vi "CORE PROGRAMMING TLB FRAME V1.vi"() -> ()   [LabVIEW 2018]
uses:
  TLB Type Definitions/Intruction Type Definitions.ctl
  TLB Type Definitions/State Type Definitions, for 0.26g versions and later 3.ctl
  <vilib>/Studica/Studica Toolkit/NavX/TypeDefs/Flags/Z900_navX_Flags_OpStatusTypeDef.ctl
  <vilib>/Studica/Studica Toolkit/NavX/TypeDefs/Flags/Z900_navX_Flags_CalibrationStatusTypeDef.ctl
  TLB Type Definitions/Vision cluster.ctl
  TLB Type Definitions/PING CLUSTER.ctl
  TLB Type Definitions/Encoder cluster.ctl
  TLB Type Definitions/Stepper cluster.ctl
  TLB Type Definitions/Yaw Cluster.ctl
  TLB Type Definitions/IR Sensor Type Def.ctl
  TLB Type Definitions/Line Sensor Cluster.ctl
  TLB Type Definitions/Time cluster.ctl
  TLB Type Definitions/Box Colour Detection Cluster (0.26d and above).ctl
  Underlying VI's/FGV's/Box FGV/Box Colour FGV Colours.ctl
  <vilib>/Studica/Studica Toolkit/Background/DIO Channel.ctl
  TLB Type Definitions/Y Stepper cluster.ctl
  TLB Type Definitions/Motor Speed Cluster.ctl
  <vilib>/Studica/Studica Toolkit/Background/PWM Channel.ctl
  Underlying VI's/NavX VI/navX type def.ctl
  <vilib>/Studica/Studica Toolkit/Background/I2C Channel.ctl
  Underlying VI's/I2C Master VI/Arduino_Interfacing.ctl
  Labview Training Phase 2/Enum Controls/States for Action Engine.ctl
  Underlying VI's/Motor Control VI with PID/MOTOR CONTROL WITH PID AE DATA MODE TYPE DEF.ctl
  Underlying VI's/Motor Control VI with PID/MOTOR CONTROL WITH PID AE DIRECTION TYPE DEF.ctl
  Experimental VI's/Archived VI's/MOTOR CONTROL NO PID Type Def.ctl
  <vilib>/myRIO/Common/Instrument Driver Framework/myRIO v1.0/AI/typedefs/AI Channels List.ctl
  <vilib>/myRIO/Common/Instrument Driver Framework/myRIO v1.0/AI/typedefs/AI Channels Enum.ctl
  Underlying VI's/Line Sensor AE/Line Sensor AE Type Def.ctl
  Underlying VI's/I2C Master VI/I2C MASTER Type Def.ctl
  Underlying VI's/Elasped Timer/Elapsed timer control.ctl
  Underlying VI's/IMAQ Create Reference AE/IMAQ Reference AE.ctl
  Underlying VI's/FGV's/Box FGV/Box Colour FGV States.ctl
  Underlying VI's/I2C Master VI/I2C_MASTER_WRITE_NEW Type Def.ctl
  Underlying VI's/FGV's/Servo State FGV/Servo States FGV Enum.ctl
  Underlying VI's/Modified webcam FGV/Webcam AE.ctl
  <vilib>/userdefined/High Color/IMAQdx.ctl
  <vilib>/Studica/Studica Toolkit/NavX/NavX.lvlib
panel:
  out "Same colour?":bool
  out "Distance to move":dbl
  out "Box Colour Detection":T1
  out "Errors detected":bool
  out "Robot ready":bool
  out "Time cluster":T3
  out "Table IR obstruct":bool
  out "Front IR obstruct":bool
  out "Line sensors":T4
  out "IR Sensors":T5
  out "NAVX Values":T6
  out "Stepper position values":T7
  out "Encoder values":T8
  out "Ultrasonic sensors":T9
  out "Selected Task":T10=enum."Start Task 9"
  out "Object recognition mode":enum16{"Ball", "Soap", "Gel", "Pipe", "None"}(ring)
  out "Image Processing Error":errorcluster
  out "Object Detection":T11
  out "Status":T14 {"OP Status" items=["INITIALIZING", "SELFTEST_IN_PROGRESS", "ERROR", "IMU_AUTOCAL_IN_PROGRESS", "NORMAL"]; "Calibration Status" items=["IMU_CAL_STATE_MASK"=3, "IMU_CAL_STATE_INPROGRESS"=0, "IMU_CAL_STATE_ACCUMULATE"=1, "IMU_CAL_STATE_COMPLETE"=2]}
  out "General Errors":errorcluster
  in  "Red LED":bool
  out "Front Ultrasonic obstruct":bool
  out "Speed & distance":T15
  out "Task selection":u8
  out "NavX Readings":T16
  out "Arduino Data":T17
  out "TASK ENABLE":bool
  out "Rising Edge":bool
  in  "Green LED":bool
  out "State Logic":T18=enum."Startup"
  out "elements":T10[](array[typedef])
  in  "STOP TASK":bool
  in  "OK Button":bool
  in  "STOP":bool
  out "Queue Errors":errorcluster
  out "Action Queue Items":i32
  out "State Logic Queue Items":i32
  out "Action Queues items":string[](array[string])=["Hardware reset", "Software reset", ""]
  out "Action State":string
  # "TLB FRAMEWORK STATUS"
  # "System Health Status Update"
  # "Test Programme written by Calvin Loke    Dated: 28 Aug 2019\nTest Programme revised by Dr Alex See   Dated 30 Aug 2019\n\nRevision date: 20/03/2020\nProgramme version:   TLB Native Dynamic Events ver 0.19a"
  # "0: Task 1\n1: Task 2\n2: Task 3\n3: Task 4\n4: Task 5\n5: Task 6\n6: Task 7\n7: Task 8 Ball\n8: Task 8 Soap\n9: Task 8 Gel\n10: Task 8 Pipe\n11: Task 9 Blue\n12: Task 9 Black\n13: Task 9 Green\n14: Task 9 Red\n15: Task 9 Yellow"
  # "Ball: Right\nSoap: Left\nGel: Reverse\nPipe: Forward"
  # "VISION"
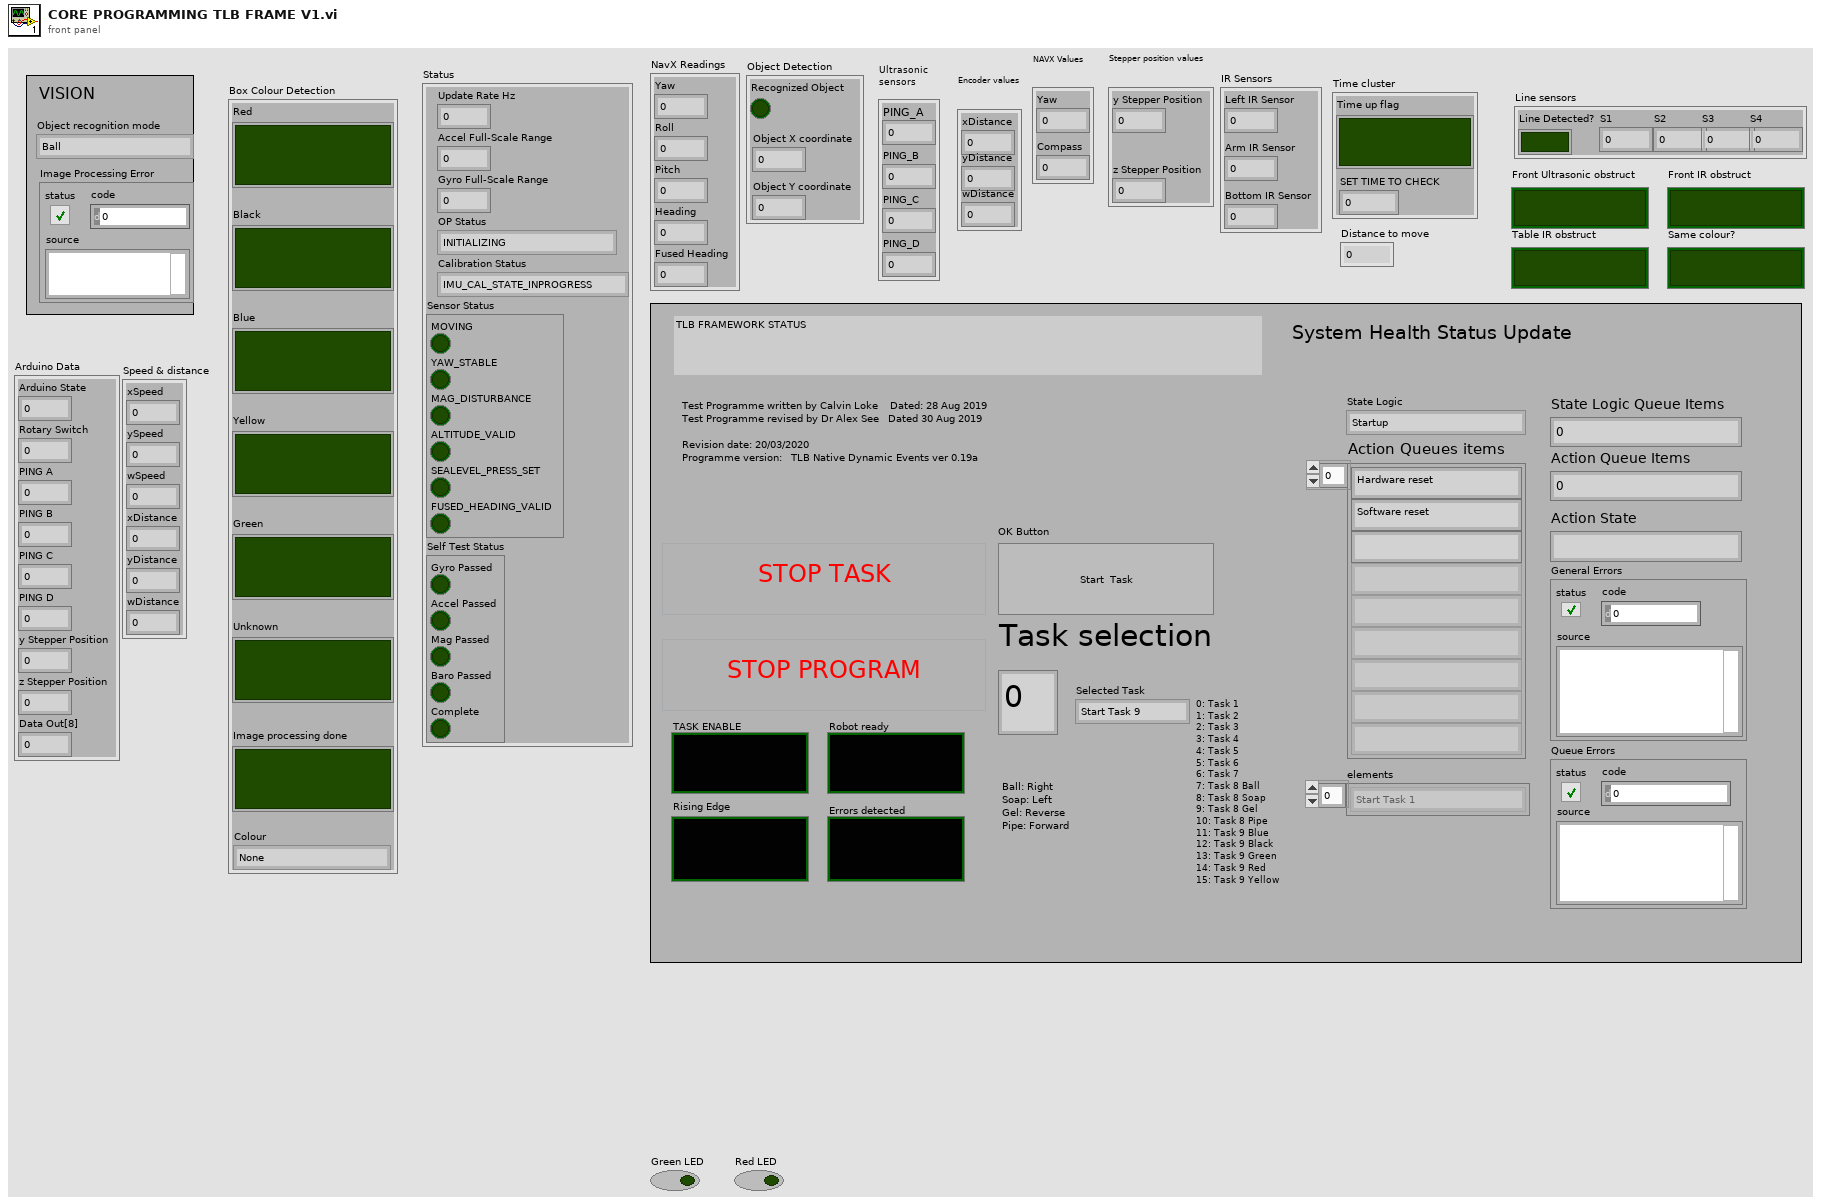
[diagram p1: front panel]
types:
  T1 = typedef "Box Colour Detection Cluster (0.26d and above).ctl" = cluster{"Red":bool, "Black":bool, "Blue":bool, "Yellow":bool, "Green":bool, "Unknown":bool, "Image processing done":bool, "Colour":T2}
  T2 = typedef "Box Colour FGV Colours.ctl" = enum16{"None", "Black", "Blue", "Green", "Red", "Yellow"}
  T3 = typedef "Time cluster.ctl" = cluster{"Time up flag":bool, "SET TIME TO CHECK":dbl}
  T4 = typedef "Line Sensor Cluster.ctl" = cluster{"Line Detected?":bool, "S1":dbl, "S2":dbl, "S3":dbl, "S4":dbl}
  T5 = typedef "IR Sensor Type Def.ctl" = cluster{"Left IR Sensor":dbl, "Arm IR Sensor":dbl, "Bottom IR Sensor":dbl}
  T6 = typedef "Yaw Cluster.ctl" = cluster{"Yaw":dbl, "Compass":dbl}
  T7 = typedef "Stepper cluster.ctl" = cluster{"y Stepper Position":u8, "z Stepper Position":u8}
  T8 = typedef "Encoder cluster.ctl" = cluster{"xDistance":dbl, "yDistance":dbl, "wDistance":dbl}
  T9 = typedef "PING CLUSTER.ctl" = cluster{"PING_A":u8, "PING_B":u8, "PING_C":u8, "PING_D":u8}
  T10 = typedef "Intruction Type Definitions.ctl" = enum16{"None", "Start Task 1", "Start Task 2", "Start Task 3", "Start Task 4", "Start Task 5", "Start Task 6", "Start Task 7", "Start Task 8 - BALL", "Start Task 8 - Gel", "Start Task 8 - Pipe", "Start Task 8 - Soap", "Start Task 9", "Start Task A", "Start Task B", "Exit"}
  T11 = typedef "Vision cluster.ctl" = cluster{"Recognized Object":bool, "Object X coordinate":dbl, "Object Y coordinate":dbl}
  T12 = typedef "NavX.lvlib/Z900_navX_Flags_OpStatusTypeDef.ctl" = u8
  T13 = typedef "NavX.lvlib/Z900_navX_Flags_CalibrationStatusTypeDef.ctl" = u8
  T14 = cluster{"Update Rate Hz":u8, "Accel Full-Scale Range":u8, "Gyro Full-Scale Range":u16, "OP Status":T12, "Calibration Status":T13, "Sensor Status":cluster{"MOVING":bool, "YAW_STABLE":bool, "MAG_DISTURBANCE":bool, "ALTITUDE_VALID":bool, "SEALEVEL_PRESS_SET":bool, "FUSED_HEADING_VALID":bool}, "Self Test Status":cluster{"Gyro Passed":bool, "Accel Passed":bool, "Mag Passed":bool, "Baro Passed":bool, "Complete":bool}}
  T15 = cluster{"xSpeed":dbl, "ySpeed":dbl, "wSpeed":dbl, "xDistance":dbl, "yDistance":dbl, "wDistance":dbl}
  T16 = cluster{"Yaw":dbl, "Roll":dbl, "Pitch":dbl, "Heading":dbl, "Fused Heading":dbl}
  T17 = cluster{"Arduino State":u8, "Rotary Switch":u8, "PING A":u8, "PING B":u8, "PING C":u8, "PING D":u8, "y Stepper Position":u8, "z Stepper Position":u8, "Data Out[8]":u8}
  T18 = typedef "State Type Definitions, for 0.26g versions and later 3.ctl" = enum16{"None", "Startup", "Move to Angle", "True Stop", "Idle", "Shutdown", "Task 1A", "Task 1B", "Task 2:Raise Arm", "Task 2:Sensor Mode", "Task 2:Reverse Mode", "Task 3: Rotate 360", "Task 4_A", "Task 4_B", "Task 4_C", "Task 4_D", "Task 5A: RAISING ARM", "Task 5B: STILL WAITING", "Task 5C: GOING DOWN", "Task 5D: GRAB", "Task 5E: GOING UP", "Task 5F: ARM GRAB HEIGHT", "Task 5G: CLOSE CLAW", "Task 5H: RAISE ARM", "Task 6A: RAISE ARM", "Task 6B: CAM BURST", "Task 6C: PROCESS IMAGE", "Task 6D: BALL BUSTER", "Task 6E: STILL WAITING", "Task 6F: CAM BURST 2", "Task 6G: PROCESS IMAGE 2", "Task 6H: SKADI SOAPS", "Task 6I: STILL WAITING 2", "Task 6J: CAM BURST 3", "Task 6K: PROCESS IMAGE 3", "Task 6L: JAM IT IN", "Task 6M: STILL WAITING 3", "Task 6N: CAM BURST 4", "Task 6O: PROCESS IMAGE 4", "Task 6P: PIPE BOMB", "Task 7", "Task 8A: RAISE ARM", "Task 8B: MOVE TO BOX", "Task 8C: CAM BURST", "Task 8D: PROCESS IMAGE", "Task 8E: ROBOT ADJUST", "Task 8F: CAM BURST 2", "Task 8G: PROCESS IMAGE 2", "Task 8H: ARM ADJUST", "Task 8I: ARM GRAB HEIGHT", "Task 8J: CLOSE CLAW", "Task 8K: RAISE MY SWORD", "Task 8I: STILL WAITING", "Task 8L: Return to position", "Task 9A: Raise Arm", "Task 9B: Rotate to Angle", "Task 9C: Detect Box", "Task 9D: MOVE FORWARD", "Task 9D2: ANGLE CORRECTION", "Task 9E: MOVE LEFT", "Task 9E2: MOVE RIGHT", "Task 9F: SCAN BOX", "Task 9G: MOVE RIGHT", "Task 9H: SCAN BOX 2", "Task 9I: ROTATE 90 CW", "Task 9J: FORWARD", "Task 9J2: ANGLE CORRECTION", "Task 9K: RAM WALL", "Task 9L: MOVE RIGHT", "Task 9M: SCAN BOX 3", "Task 9N: MOVE RIGHT", "Task 9O: SCAN BOX 4", "Task A1: RAISE ARM", "Task A2: ROTATE TO ANGLE", "Task A3: MOVE TO BL BOX", "Task A4: MOVE FORWARD", "Task A5: Stop", "Task A6: ROTATE CW 90", "Task A7: FORWARD", "Task A8: LEFT UNTIL LINE", "Task A9: REVERSE", "Task A10: ROTATE TO ANGLE"}
  T19 = typedef "PWM Channel.ctl" = enum16{"Not Connected", "A/PWM0", "A/PWM1", "A/PWM2", "A/PWM3", "A/PWM4", "B/PWM0", "B/PWM1", "B/PWM2", "B/PWM3", "B/PWM4", "C/PWM0", "C/PWM1"}
  T20 = typedef "Motor Speed Cluster.ctl" = cluster{"ySpeed":dbl, "xSpeed":dbl, "wSpeed":dbl}
  T21 = typedef "Y Stepper cluster.ctl" = cluster{"yStepper desired":u8}
  T22 = typedef "DIO Channel.ctl" = enum16{"Not Connected", "A/DIO1", "A/DIO2", "A/DIO3", "A/DIO4", "A/DIO5", "A/DIO6", "A/DIO7", "A/DIO13", "B/DIO1", "B/DIO2", "B/DIO3", "B/DIO4", "B/DIO5", "B/DIO6", "B/DIO7", "B/DIO13", "C/DIO0", "C/DIO1", "C/DIO2", "C/DIO3", "C/DIO4", "C/DIO5", "C/DIO6", "C/DIO7"}
  T23 = cluster{"PWM Channel":T19, "FPGA VI Reference Out":refnum<k20>}
  T24 = cluster{"DIO Channel":T22, "FPGA VI Reference Out":refnum<k20>}
  T25 = typedef "States for Action Engine.ctl" = enum16{"Initialize", "Write", "Read"}
  T26 = typedef "MOTOR CONTROL WITH PID AE DATA MODE TYPE DEF.ctl" = enum16{"Init AE", "Write to AE", "Read from AE"}
  T27 = typedef "navX type def.ctl" = enum16{"Get i2C reference", "Read Values", "Zero Yaw"}
  T28 = typedef "Arduino_Interfacing.ctl" = enum16{"Initialize", "Write to Arduino", "Read From Arduino"}
  T29 = typedef "I2C Channel.ctl" = enum16{"Not Connected", "A", "B"}
  T30 = cluster{"I2C Ref Out":cluster{"I2C Channel":T29, "FPGA VI Reference Out":refnum<k20>}, "Connected":bool, "Slave Address (7-bit)":u8, "Registry":u8[]}
  T31 = typedef "Box Colour FGV States.ctl" = enum16{"Initialize", "Read", "Write"}
  T32 = typedef "MOTOR CONTROL WITH PID AE DIRECTION TYPE DEF.ctl" = enum16{"y-axis movement", "x-axis movement", "rotation", "stop", "reset encoders"}
  T33 = typedef "Line Sensor AE Type Def.ctl" = enum16{"INIT AE", "READ FROM LINE SENSORS"}
  T34 = typedef "IMAQ Reference AE.ctl" = enum16{"Initialize AE", "Get IMAQ Reference", "Dispose Processing Buffer"}
  T35 = typedef "Elapsed timer control.ctl" = enum16{"Start", "Pause", "Initialize"}
  T36 = typedef "I2C_MASTER_WRITE_NEW Type Def.ctl" = enum16{"Ultrasonic sensors", "Stepper origin", "zStepper 13.3k", "zStepper 13k", "zStepper 12k", "zStepper 11k", "zStepper 10k", "zStepper 9k", "zStepper 8k", "zStepper 7k", "zStepper 6k", "zStepper 5k", "zStepper 4k", "zStepper 3k", "zStepper 2k", "zStepper 1k", "zStepper 900", "zStepper 800", "zStepper 700", "zStepper 600", "zStepper 500", "zStepper 400", "zStepper 300", "zStepper 200", "zStepper 100", "zStepper 0", "yStepper control", "Open Claw", "Close Claw", "Soft Reset"}
  T37 = typedef "Servo States FGV Enum.ctl" = enum16{"Open Claw", "Close claw"}
  T38 = typedef "Webcam AE.ctl" = enum16{"Initialize Camera", "Open Camera", "Continuous Acquisition", "Close Camera", "Retrieve Image", "Dispose Camera Image Buffer"}
  T39 = typedef "IMAQdx.ctl" = refnum<k21>
  T40 = typedef "MOTOR CONTROL NO PID Type Def.ctl" = enum16{"Init", "Front Back", "Left Right", "Rotate", "Stop", "Latch"}
  T41 = typedef "AI Channels List.ctl" = T42[]
  T42 = typedef "AI Channels Enum.ctl" = enum16{"Not Connected", "AudioIn/Left", "AudioIn/Right", "C/AI0", "C/AI1", "A/AI0", "A/AI1", "A/AI2", "A/AI3", "A/AI4", "A/AI5", "A/AI6", "A/AI7", "B/AI0", "B/AI1", "B/AI2", "B/AI3", "B/AI4", "B/AI5", "B/AI6", "B/AI7", "AI/AI0", "AI/AI1", "AI/AI2", "AI/AI3", "A/AI0 (DIFF)", "A/AI1 (DIFF)", "A/AI2 (DIFF)", "A/AI3 (DIFF)", "B/AI0 (DIFF)", "B/AI1 (DIFF)", "B/AI2 (DIFF)", "B/AI3 (DIFF)"}
  T43 = cluster{"S1":dbl, "S2":dbl, "S3":dbl, "S4":dbl, "Array[4]":dbl, "Array[5]":dbl, "Array[6]":dbl, "Array[7]":dbl, "Array[8]":dbl}
  T44 = typedef "I2C MASTER Type Def.ctl" = enum16{"Last State", "Mode 0", "Mode 1", "Mode 2", "Mode 3", "Mode 4", "Mode 5", "Mode 6", "Mode 7", "Mode 8", "Mode 9", "Mode 10"}
  T45 = typedef "IMAQ Image.ctl" = refnum<image>
  T46 = cluster{"Number of Matches":i32, "Object detected?":bool}
  T47 = cluster{"Red":bool, "Black":bool, "Blue":bool, "Yellow":bool, "Green":bool, "No recognizable coolour":bool}
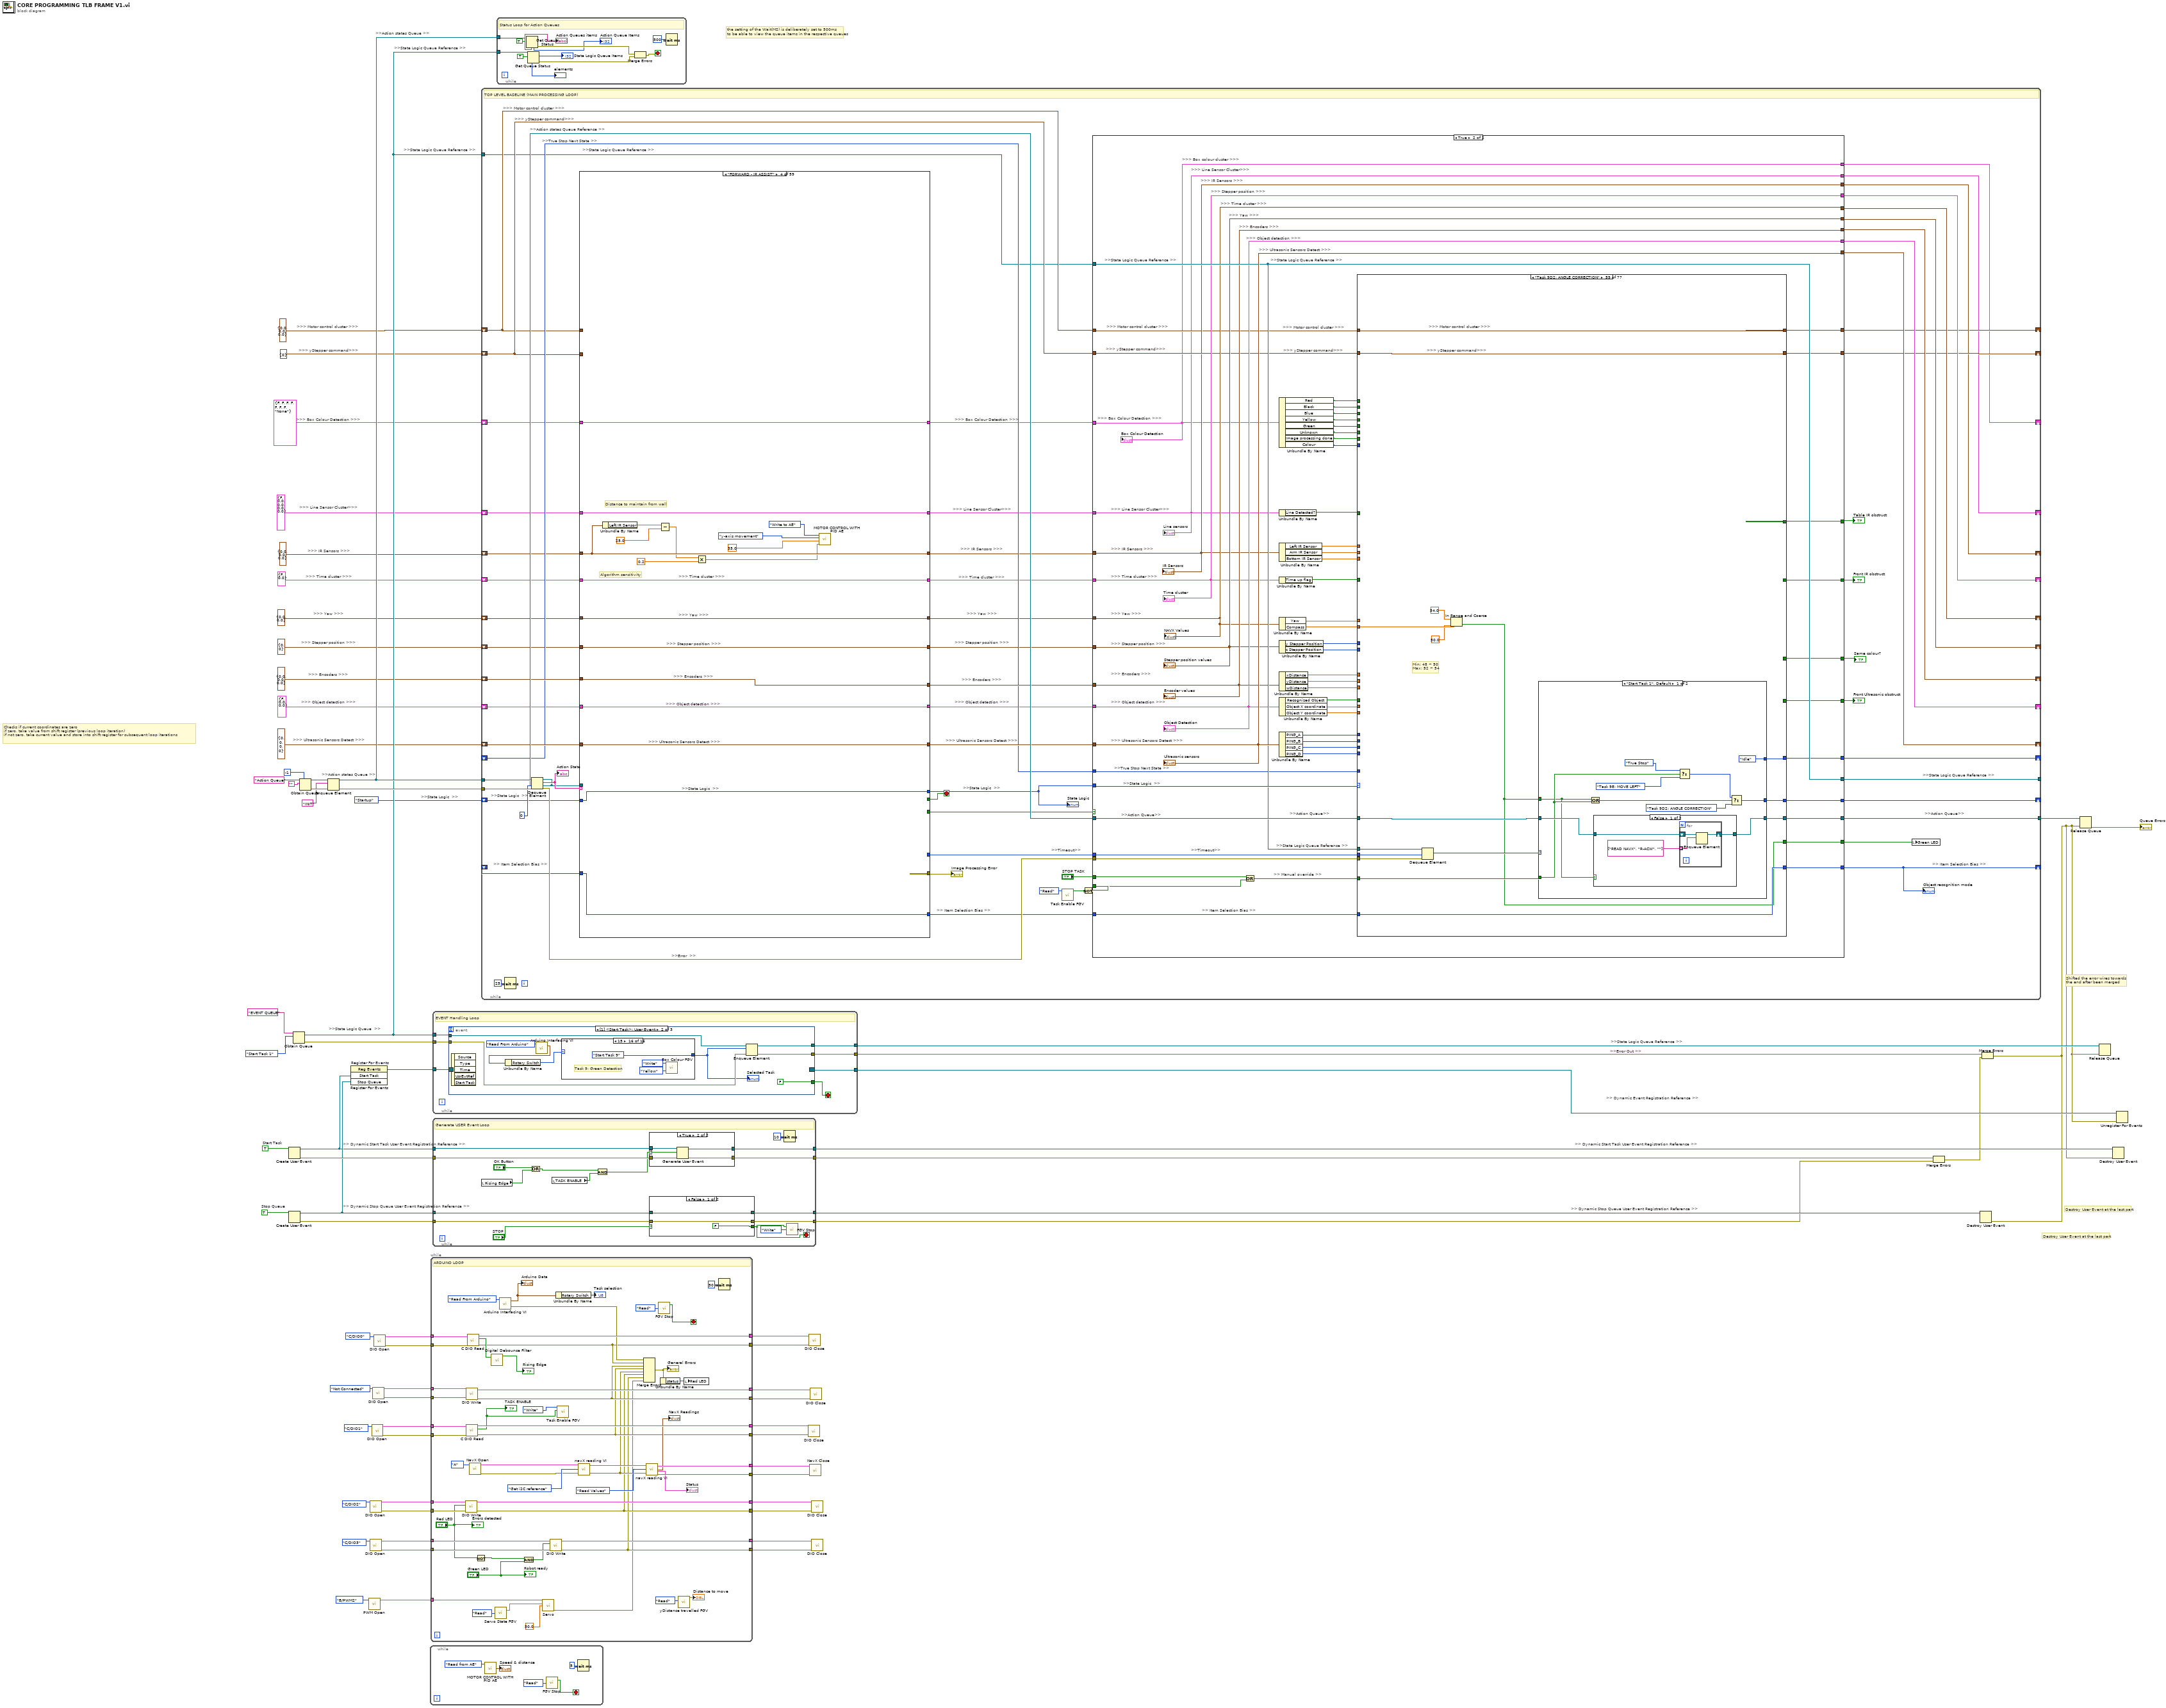
[diagram p0: block diagram]
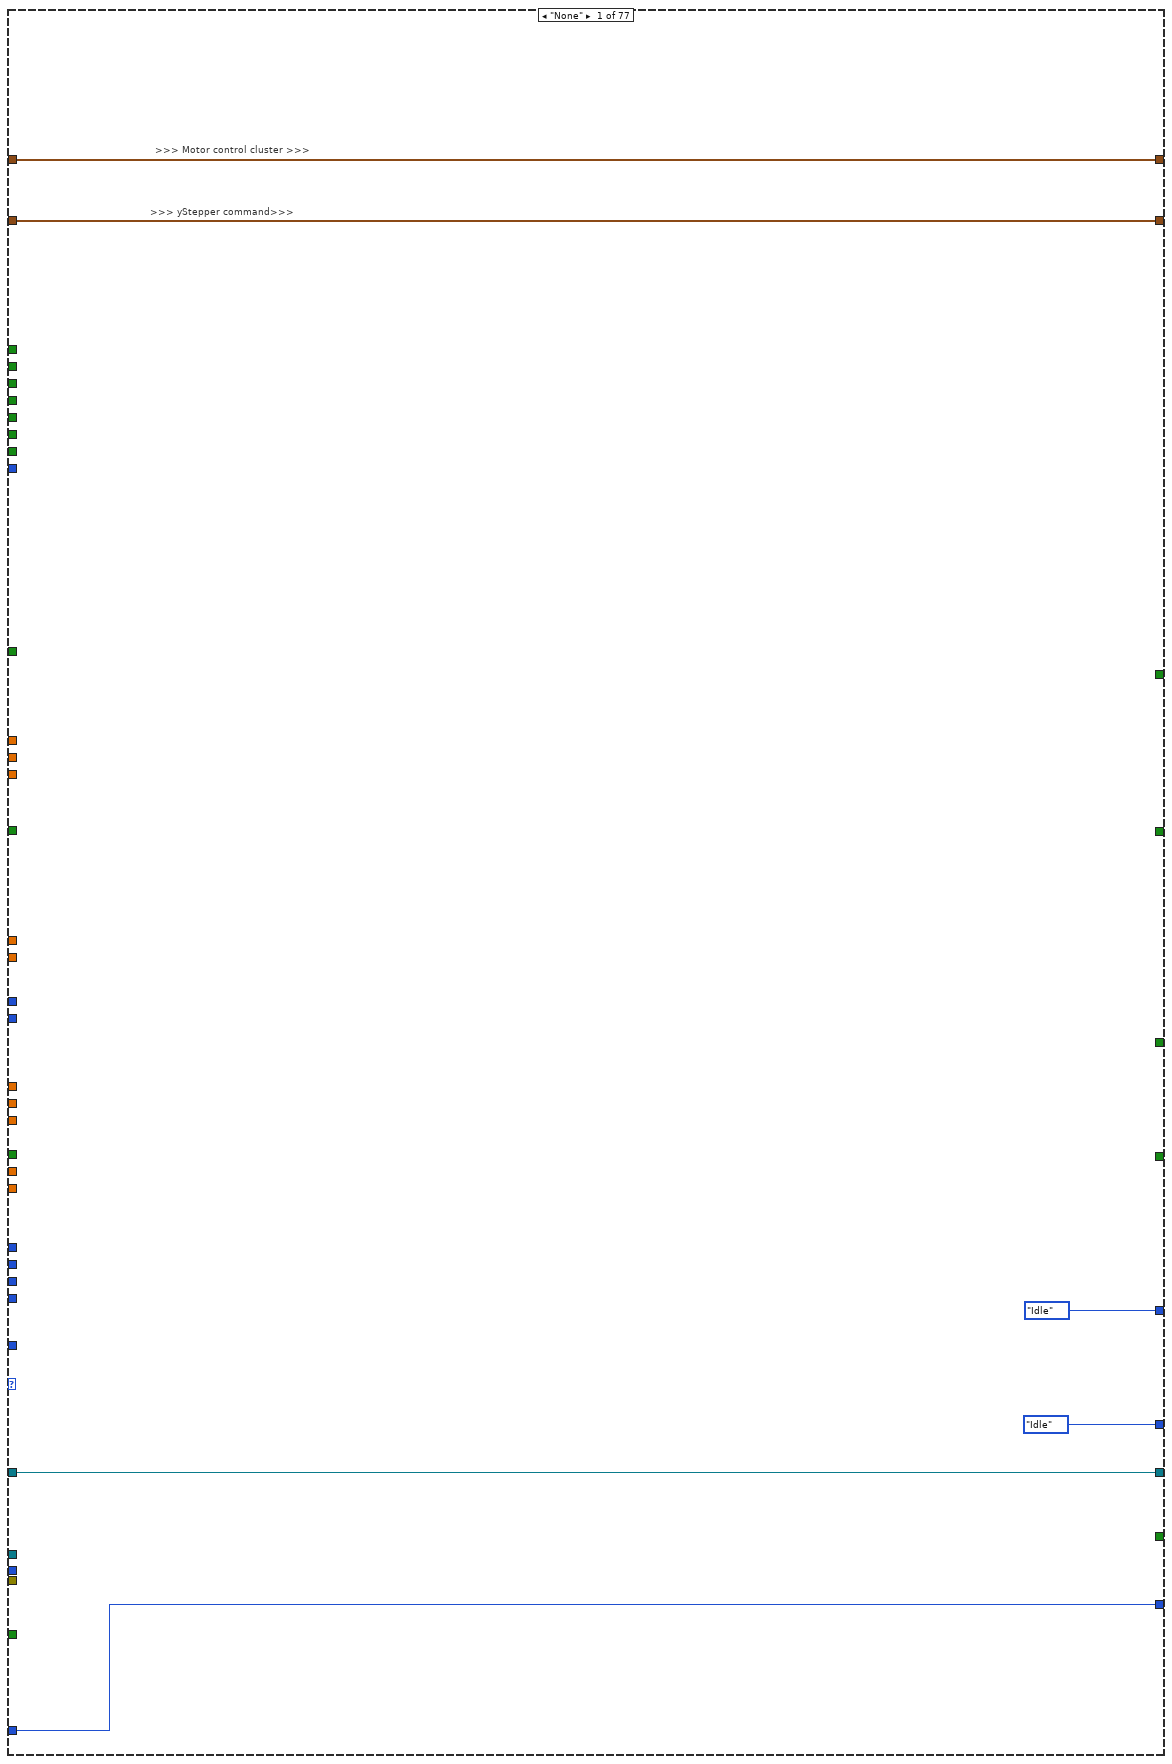
[diagram p3: hidden frame]
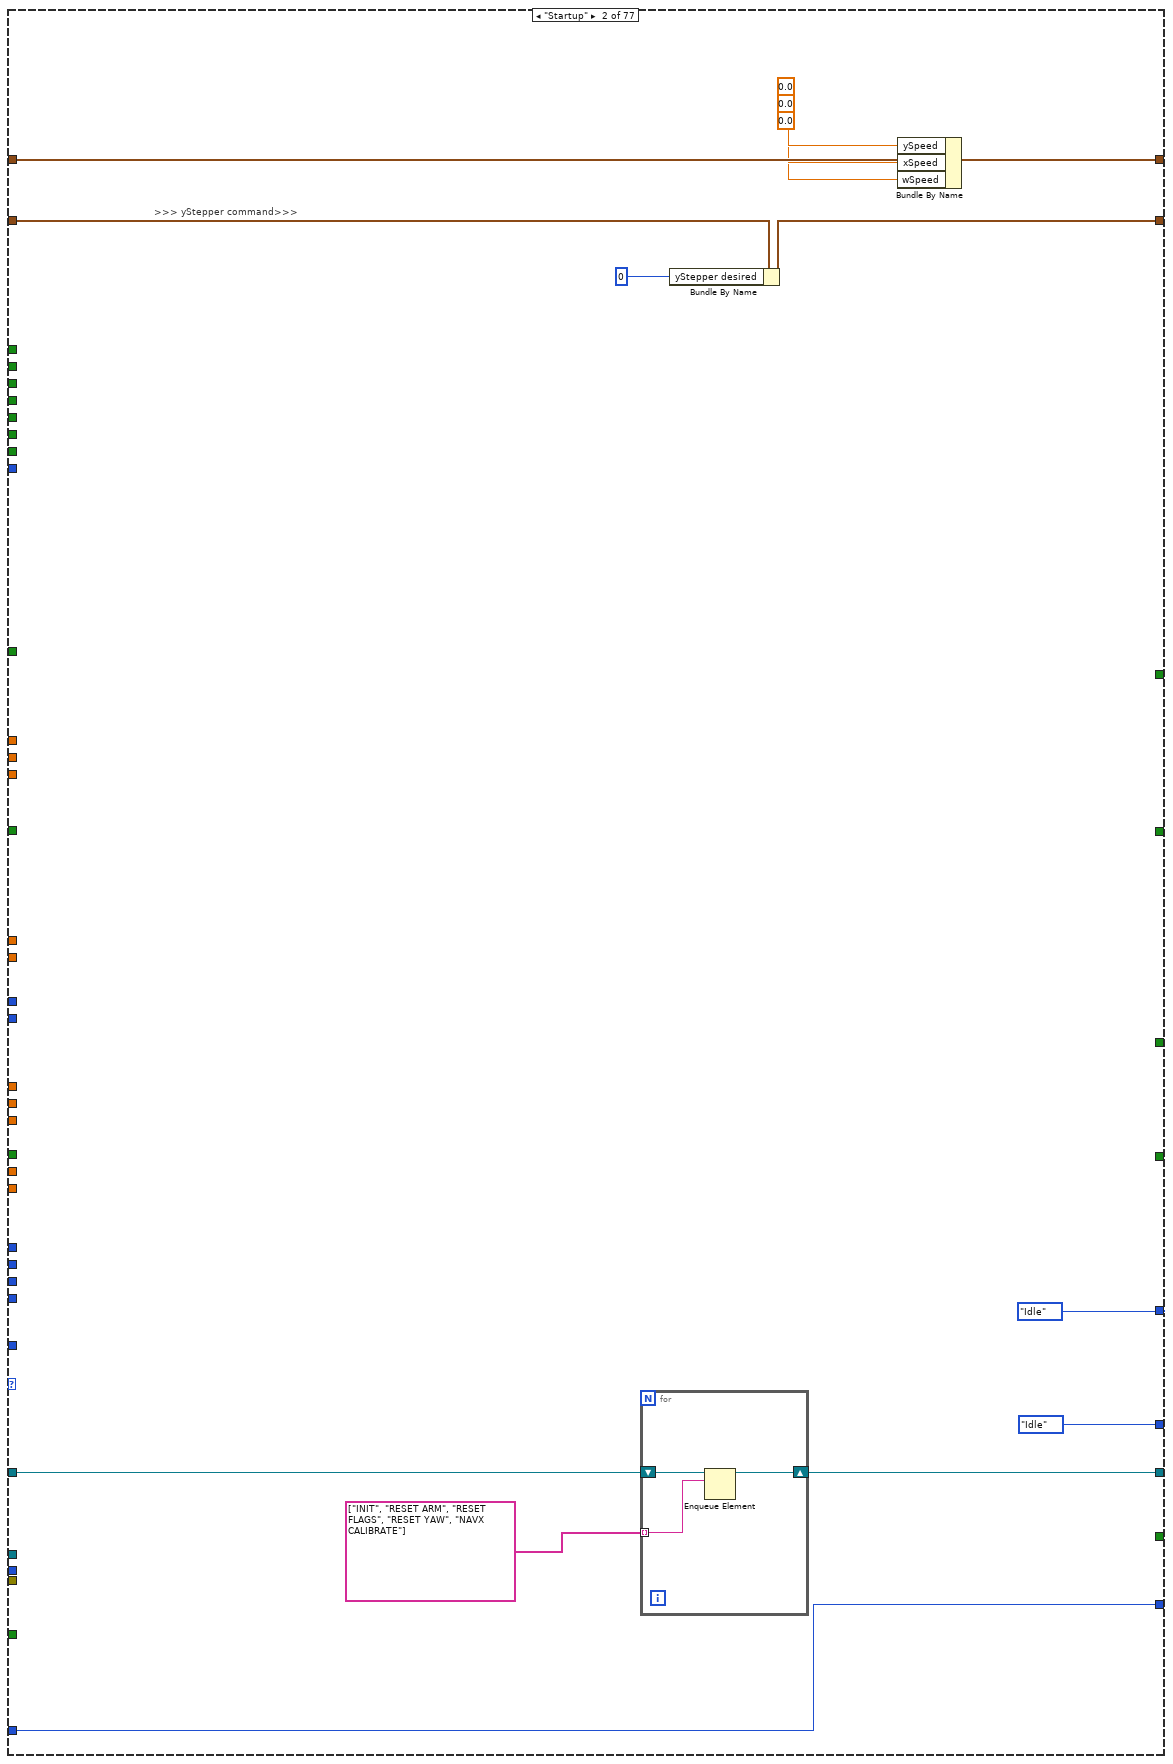
[diagram p4: hidden frame]
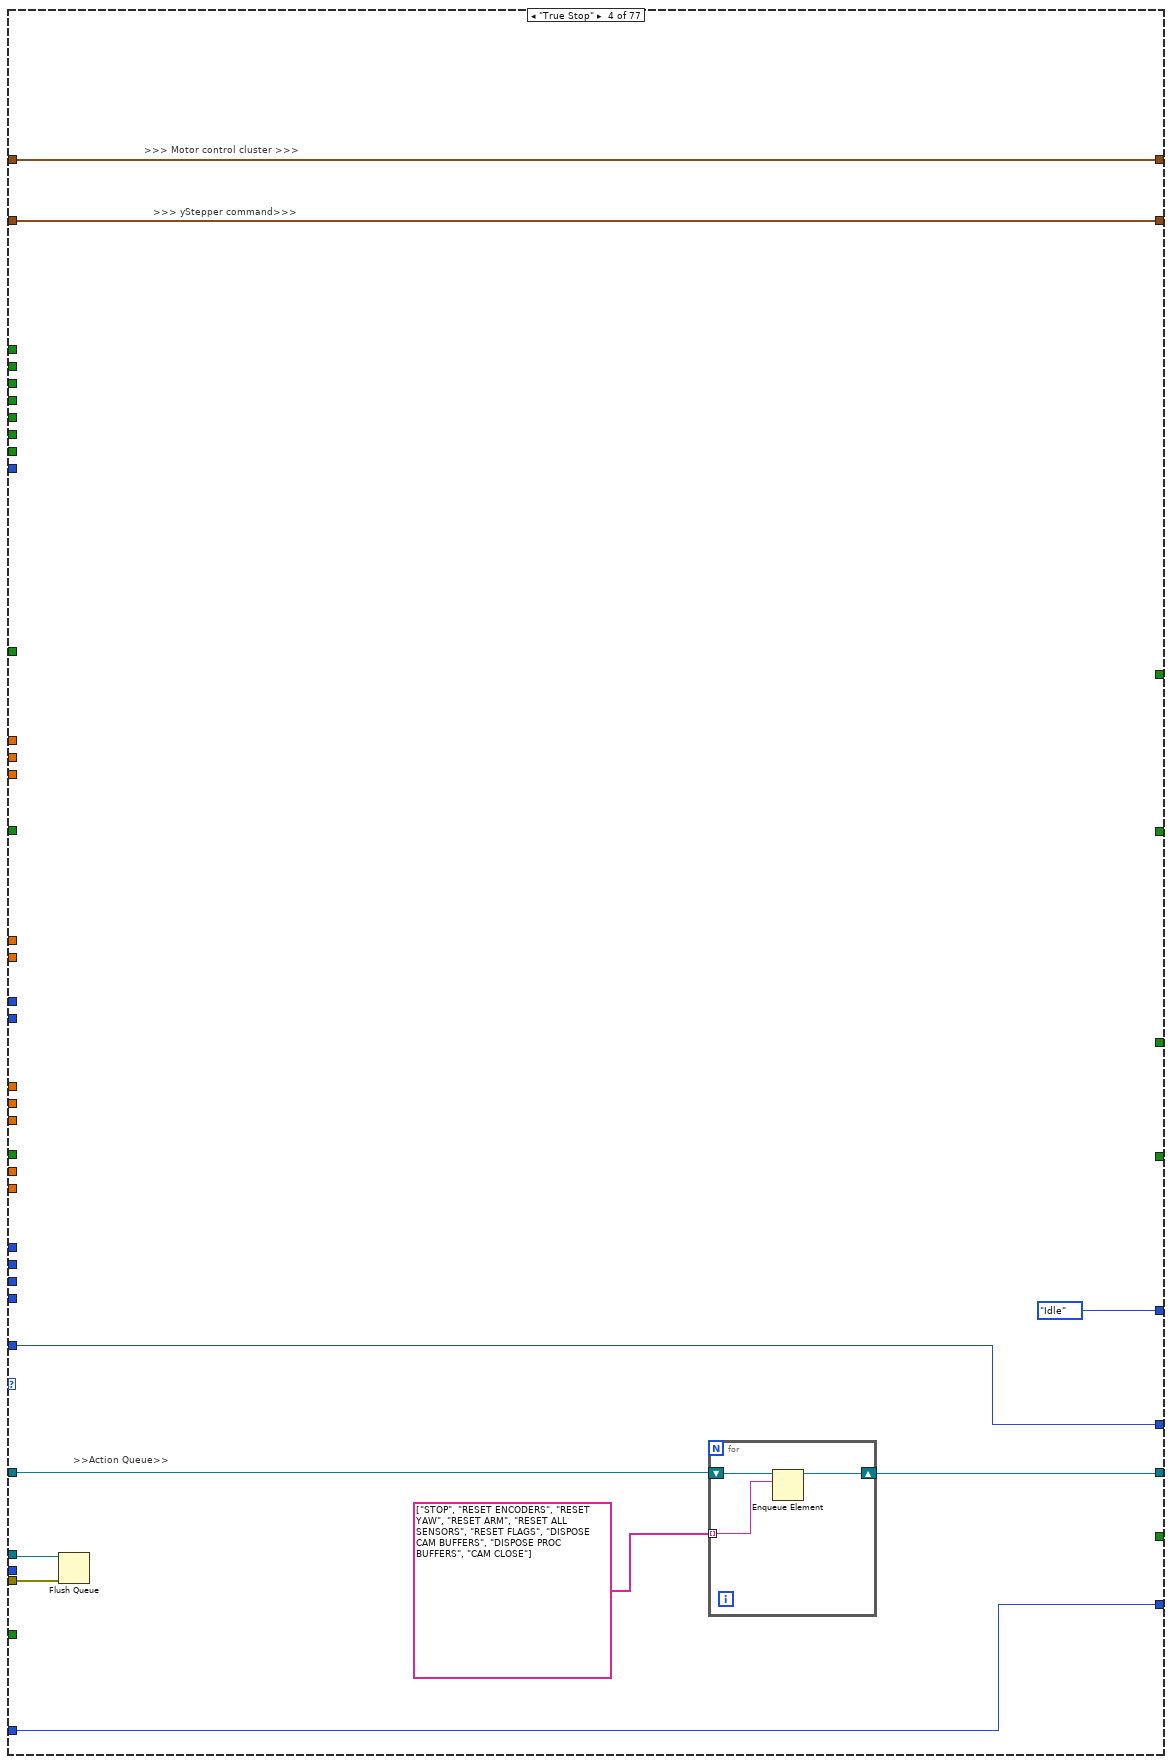
[diagram p6: hidden frame]
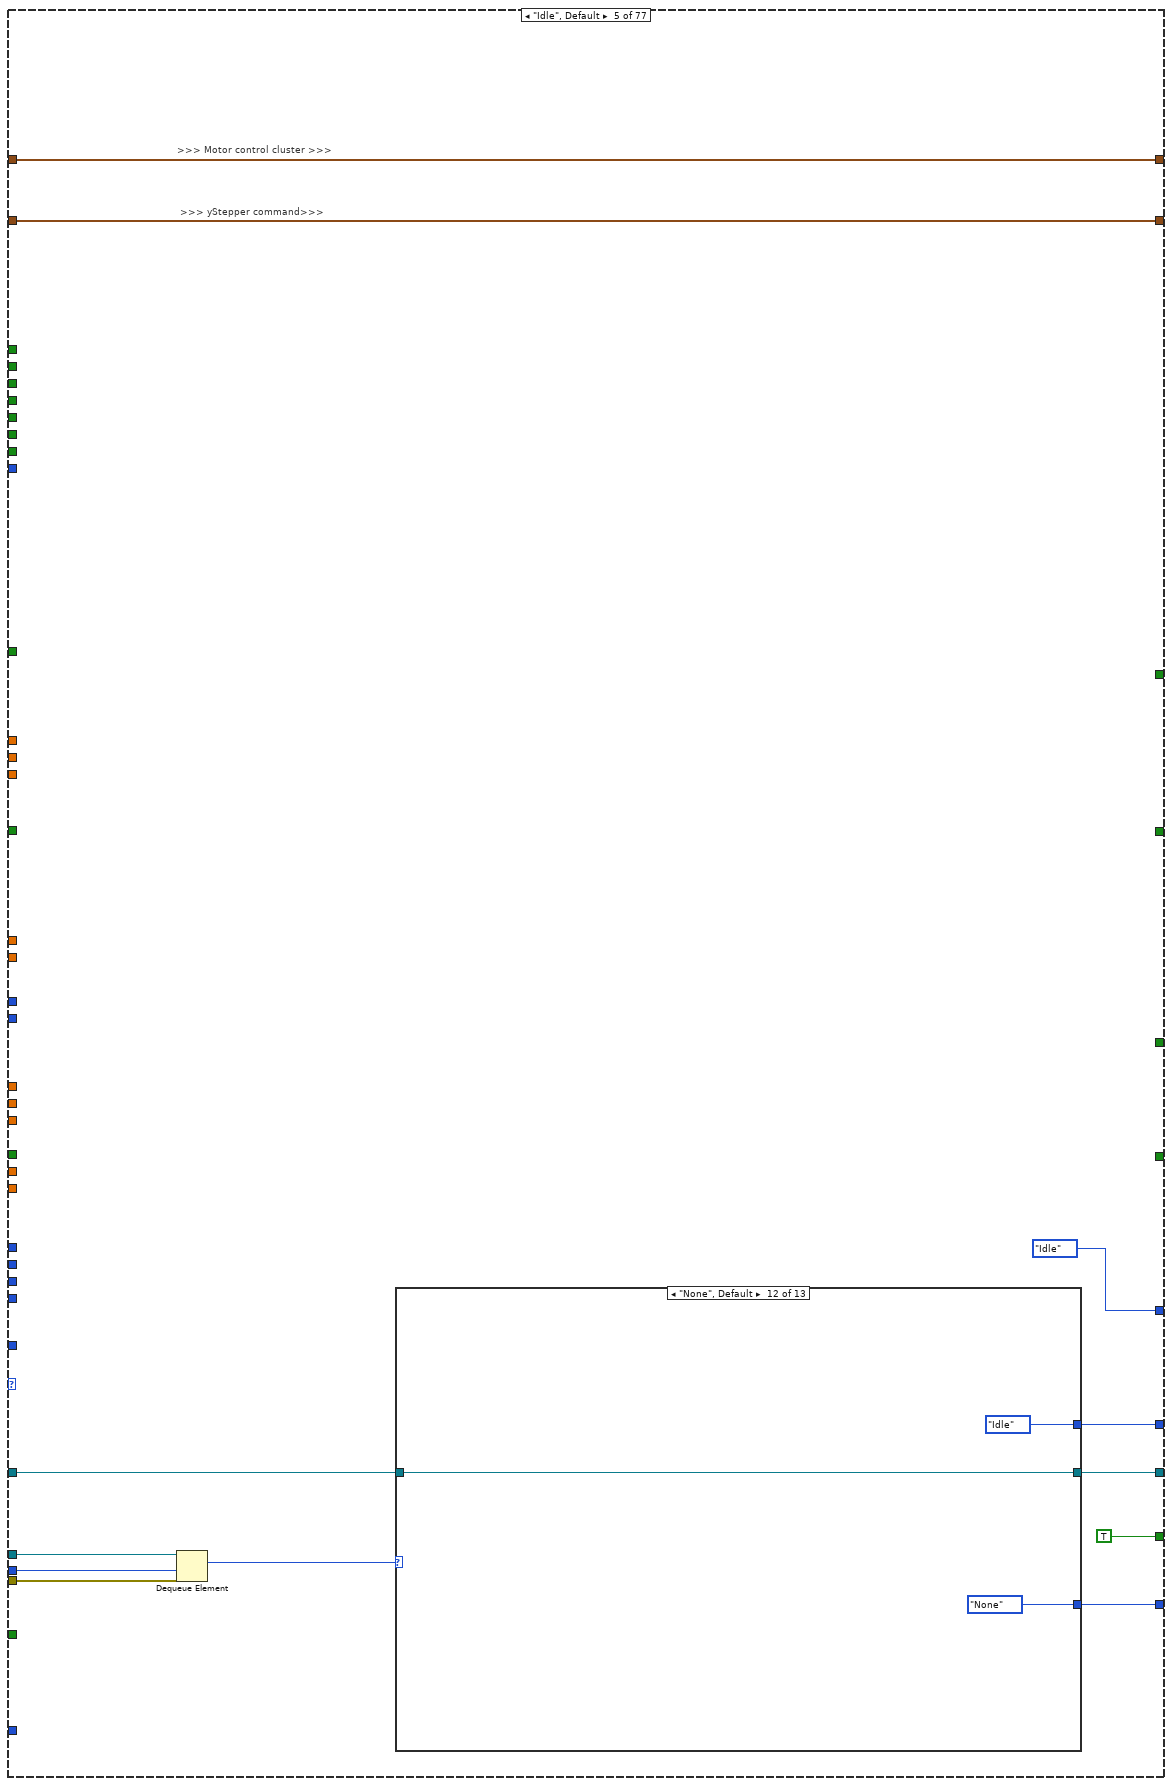
[diagram p7: hidden frame]
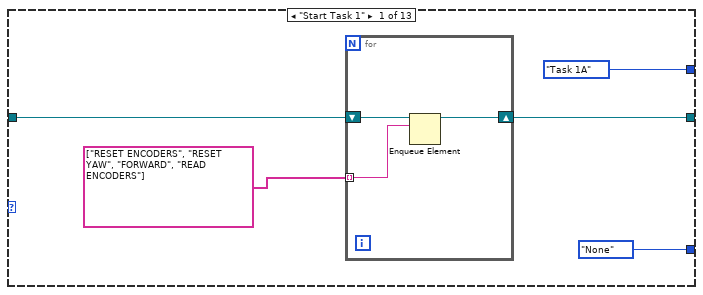
[diagram p8: hidden frame]
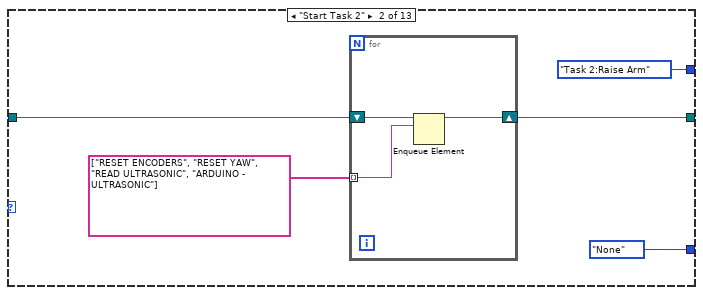
[diagram p9: hidden frame]
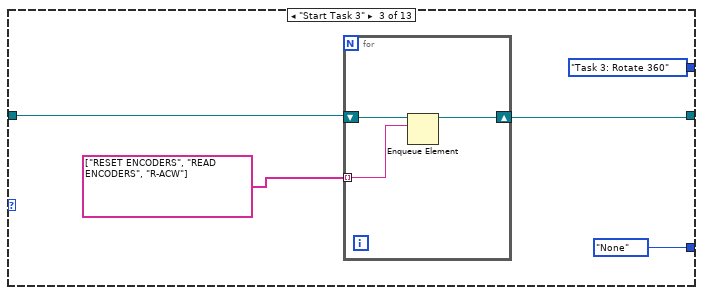
[diagram p10: hidden frame]
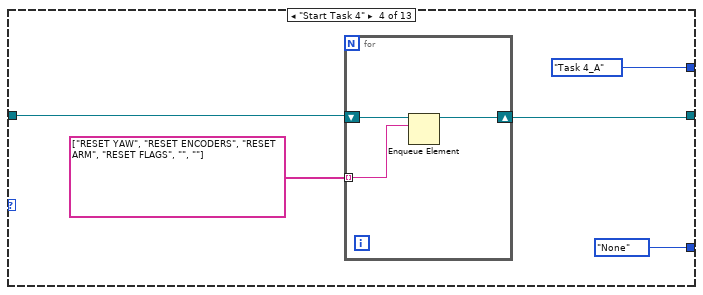
[diagram p11: hidden frame]
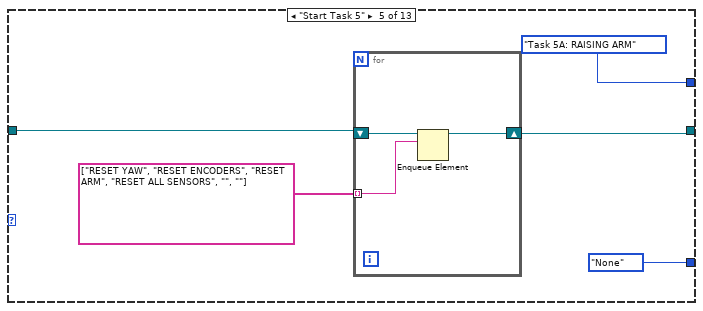
[diagram p12: hidden frame]
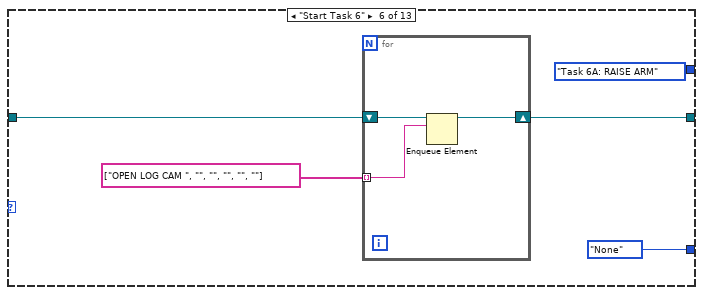
[diagram p13: hidden frame]
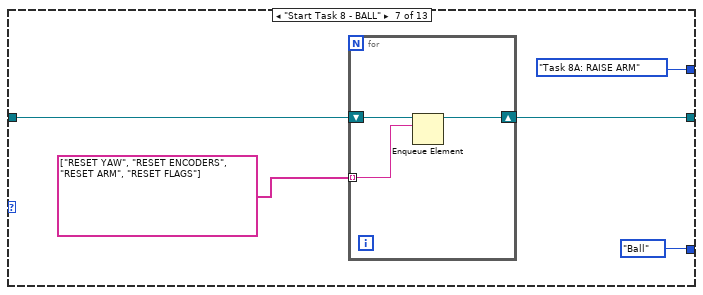
[diagram p14: hidden frame]
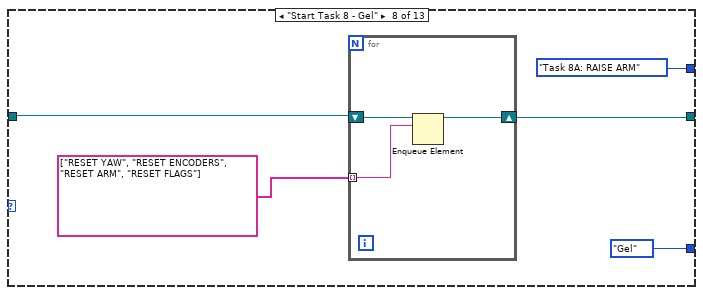
[diagram p15: hidden frame]
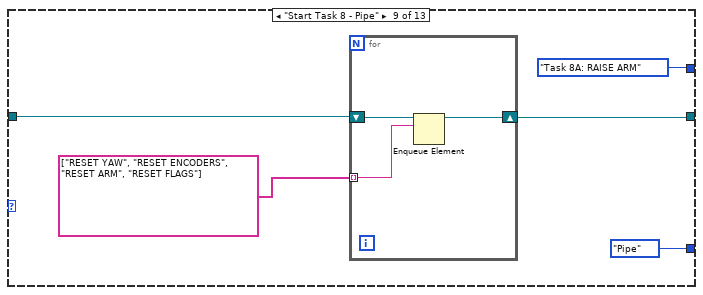
[diagram p16: hidden frame]
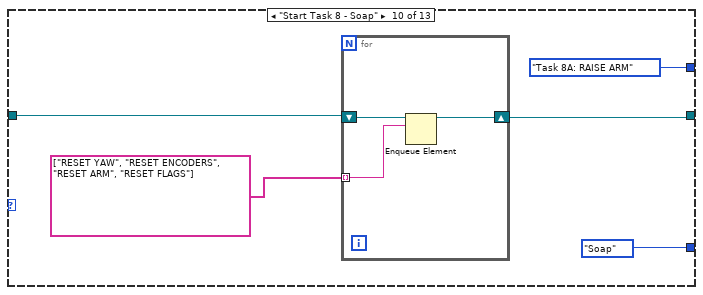
[diagram p17: hidden frame]
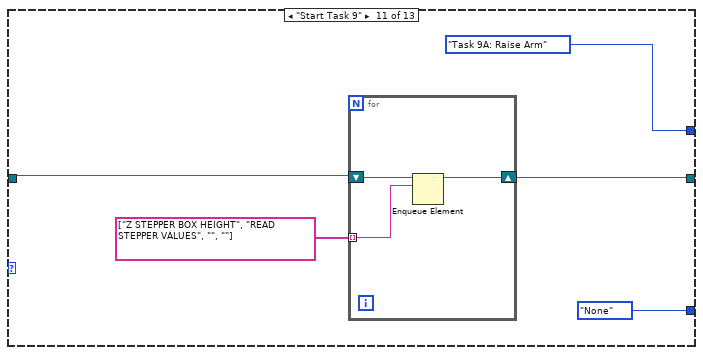
[diagram p18: hidden frame]
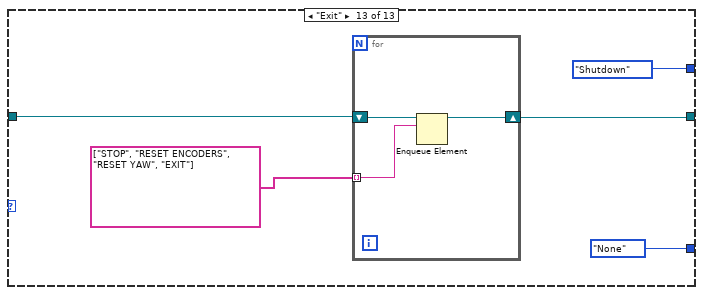
[diagram p19: hidden frame]
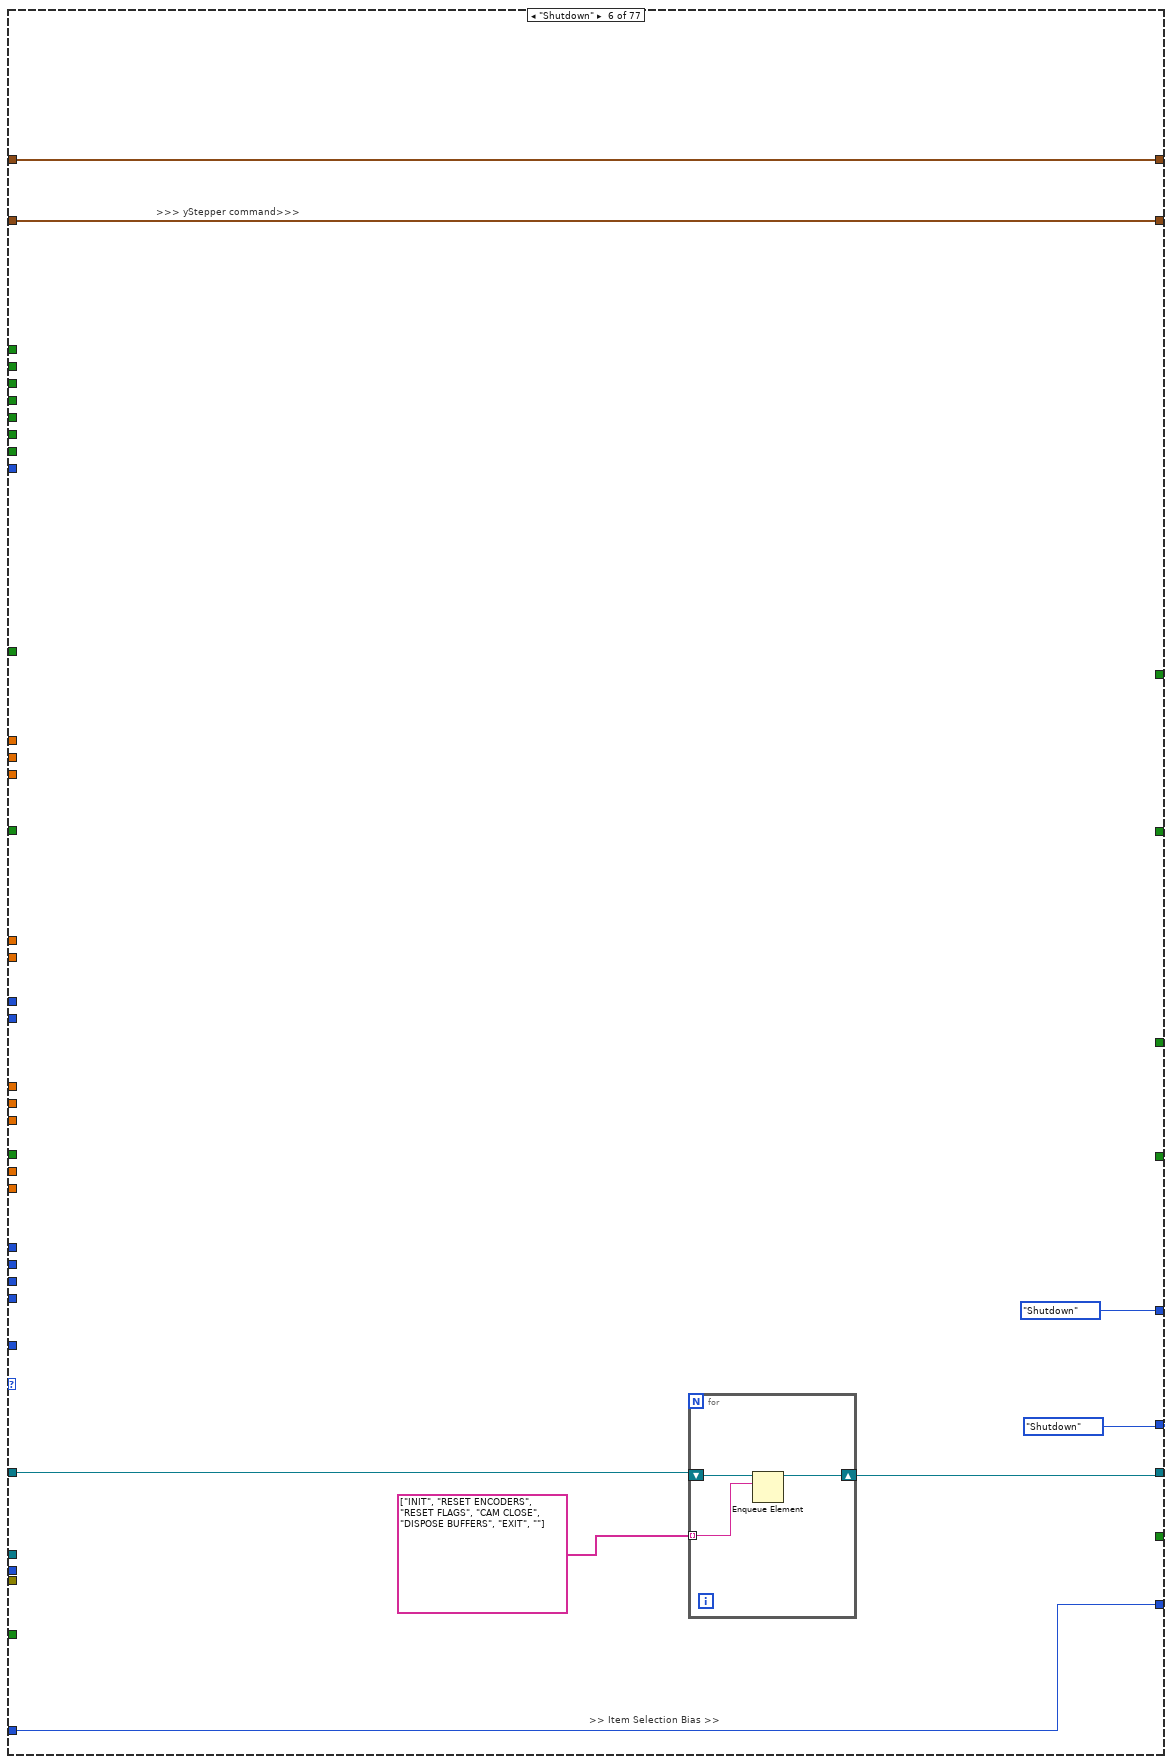
[diagram p20: hidden frame]
diagram:
  w71 = TRUE  # Stop Queue
  w70 = TRUE  # Start Task
  # ">>State Logic Queue Reference >>"
  # ">>Action states Queue >>"
  # ">>> Box Colour Detection >>>"
  # ">>State Logic Queue Reference >>"
  # ">>State Logic  >>"
  # ">>> Line Sensor Cluster>>>"
  # ">>> Motor control cluster >>>"
  # ">>> IR Sensors >>>"
  # "Checks if current coordinates are zero\nif zero, take value from shift register (previous loop iteration)\nif not zero, take current value and store into shift register for subsequent loop iterations"
  # ">>> yStepper command>>>"
  # ">>> Time cluster >>>"
  # ">>> Yaw >>>"
  # ">>> Stepper position >>>"
  # ">>> Encoders >>>"
  # ">>> Object detection >>>"
  # ">>> Ultrasonic Sensors Detect >>>"
  # "the setting of the Wait(MS) is deliberately set to 500ms\nto be able to view the queue items in the respective queues"
  # ">>Error Out >>"
  # ">> Dynamic Stop Queue User Event Registration Reference >>"
  # ">> Dynamic Start Task User Event Registration Reference >>"
  # ">> Dynamic Stop Queue User Event Registration Reference >>"
  # ">> Dynamic Start Task User Event Registration Reference >>"
  # ">> Dynamic Event Registration Reference >>"
  # ">>Action states Queue >>"
  # ">>State Logic Queue  >>"
  # ">>State Logic Queue Reference >>"
  # "Destroy User Event at the last part"
  # "Destroy User Event at the last part"
  # "Shifted the error wires towards\nthe end after been merged"
  n1 = Create User Event(user event datatype=w70) -> (user event=w62:refnum<user-event>, error out=w67:errorcluster)  [unwired: 1 in]
  n2 = Create User Event(user event datatype=w71) -> (user event=w63:refnum<user-event>, error out=w66:errorcluster)  [unwired: 1 in]
  n3 = Obtain Queue(name (unnamed)="EVENT QUEUE", element data type=Intruction_Type_Definitions."Start Task 1" ("Enum")) -> (queue out=w48:refnum<queue>, error out=w54:errorcluster)  [unwired: 3 in, 1 out]
  n4 = Obtain Queue(max queue size (-1, unlimited)=-1, name (unnamed)="Action Queue", element data type="") -> (queue out=w57:refnum<queue>, error out=w53:errorcluster)  [unwired: 2 in, 1 out]
  n5 = Enqueue Element(queue=w57, element="INIT", error in (no error)=w53) -> (queue out=w49:refnum<queue>, error out=w52:errorcluster)  [unwired: 1 in, 1 out]
  n6 = register-events "Register For Events"(w62, w63) -> (reference out=w61:refnum<event-registration>)  [unwired: 2 in, 1 out]
  n7 = call <vilib>:"PWM Open.vi"("PWM Channel"=PWM_Channel."B/PWM2") -> ("PWM Info Out"=w1:T23)  [unwired: 9 in, 1 out]
  n8 = call <vilib>:"DIO Open.vi"("DIO Channel"=DIO_Channel."C/DIO2") -> ("error out"=w21:errorcluster, "DIO Info Out"=w22:T24)  [unwired: 9 in]
  n9 = call <vilib>:"DIO Open.vi"("DIO Channel"=DIO_Channel."C/DIO3") -> ("error out"=w16:errorcluster, "DIO Info Out"=w17:T24)  [unwired: 9 in]
  n10 = call <vilib>:"DIO Open.vi"("DIO Channel"=DIO_Channel."C/DIO1") -> ("error out"=w26:errorcluster, "DIO Info Out"=w27:T24)  [unwired: 9 in]
  n11 = call <vilib>:"DIO Open.vi"("DIO Channel"=DIO_Channel."Not Connected") -> ("error out"=w31:errorcluster, "DIO Info Out"=w33:T24)  [unwired: 9 in]
  n12 = call <vilib>:"DIO Open.vi"("DIO Channel"=DIO_Channel."C/DIO0") -> ("error out"=w36:errorcluster, "DIO Info Out"=w39:T24)  [unwired: 9 in]
  n13 = while {
    stop <- w73 stop-if-true
    n14 = call "MOTOR CONTROL WITH PID AE.vi"("AE Mode"=MOTOR_CONTROL_WITH_PID_AE_DATA_MODE_TYPE_DEF."Read from AE") -> ("Speed & distance"=→"Speed & distance":T15)  [unwired: 3 in]
    n15 = call "FGV Stop.vi"("Init/Read/Write State"=States_for_Action_Engine."Read") -> ("Output node"=w73:bool)  [unwired: 2 in, 1 out]
    n16 = Wait (ms)(milliseconds to wait=u32 5) -> ()  [unwired: 1 out]
  }
  n17 = while {
    tunnel: w39 -> [w128]
    tunnel: [w127] -> w37
    tunnel: w36 -> [w126]
    tunnel: [w98] -> w35
    tunnel: w33 -> [w123]
    tunnel: [w122] -> w32
    tunnel: w31 -> [w121]
    tunnel: [w97] -> w30
    tunnel: [w120] -> w28
    tunnel: w27 -> [w119]
    tunnel: w26 -> [w118]
    tunnel: [w96] -> w25
    tunnel: w22 -> [w113]
    tunnel: w21 -> [w112]
    tunnel: [w111] -> w20
    tunnel: [w94] -> w19
    tunnel: w17 -> [w110]
    tunnel: w16 -> [w109]
    tunnel: [w108] -> w15
    tunnel: [w93] -> w14
    tunnel: [w105] -> w11
    tunnel: [w104] -> w12
    tunnel: w1 -> [w85]
    stop <- w130 stop-if-true
    # "ARDUINO LOOP"
    n18 = call <vilib>:"DIO Write.vi"("error in (no error)"=w112, "Input"="Red LED", "DIO Info In"=w113) -> ("error out"=w94:errorcluster, "DIO Info Out"=w111:T24)  [unwired: 7 in]
    n19 = call <vilib>:"DIO Write.vi"("error in (no error)"=w121, "DIO Info In"=w123) -> ("error out"=w97:errorcluster, "DIO Info Out"=w122:T24)  [unwired: 8 in]
    n20 = call <vilib>:"C DIO Read.vi"("error in (no error)"=w118, "DIO Info In in"=w119) -> ("error out"=w96:errorcluster, "IN"=w77:bool, "DIO Info In out"=w120:T24)  [unwired: 7 in]
    "TASK ENABLE" <- w77
    n21 = call <vilib>:"C DIO Read.vi"("error in (no error)"=w126, "DIO Info In in"=w128) -> ("error out"=w98:errorcluster, "IN"=w125:bool, "DIO Info In out"=w127:T24)  [unwired: 7 in]
    n22 = call <vilib>:"NavX Open.vi"("I2C Channel"=I2C_Channel."A") -> ("error out"=w115:errorcluster, "NavX Info"=w117:T30)  [unwired: 9 in]
    n23 = Not(x="Red LED") -> (.not. x?=w88:bool)
    n24 = call "Digital Debounce Filter.vi"("Boolean input"=w125) -> ("Rising Edge"=→"Rising Edge":bool)  [unwired: 1 in, 2 out]
    n25 = call "Servo State FGV.vi"("Init/Read/Write State"=States_for_Action_Engine."Read") -> ("Output"=w81:dbl)  [unwired: 2 in, 1 out]
    n26 = call "Arduino Interfacing VI.vi"("AE Mode"=Arduino_Interfacing."Read From Arduino") -> ("error out"=w99:errorcluster, "Arduino Data"=w101:T17)  [unwired: 3 in]
    "Arduino Data" <- w101
    n27 = And(x=w88, y="Green LED") -> (x .and. y?=w90:bool)
    n28 = call <vilib>:"Servo.vi"("PWM Info In"=w85, "Position"=w81, "Frequency [Hz]"=50.0) -> ("error out"=w84:errorcluster)  [unwired: 11 in, 1 out]
    n29 = call <vilib>:"DIO Write.vi"("error in (no error)"=w109, "Input"=w90, "DIO Info In"=w110) -> ("error out"=w93:errorcluster, "DIO Info Out"=w108:T24)  [unwired: 7 in]
    n30 = Unbundle By Name(w101) -> ("Rotary Switch"=→"Task selection":u8)
    n31 = call "Task Enable FGV.vi"("Task Enable Input"=w77, "Init/Read/Write State"=States_for_Action_Engine."Write") -> ()  [unwired: 8 in, 2 out]
    n32 = call "navX reading VI.vi"("NavX Info In"=w117, "Mode"=navX_type_def."Get i2C reference", "error in (no error)"=w115) -> ("NavX Info Out"=w106:T30, "Error Out"=w95:errorcluster)  [unwired: 2 out]
    n33 = Merge Errors(w99, w98, w97, w96, w95, w94, w93, w84) -> (w91:errorcluster)
    "General Errors" <- w91
    n34 = call "navX reading VI.vi"("NavX Info In"=w106, "Mode"=navX_type_def."Read Values", "error in (no error)"=w95) -> ("NavX Info Out"=w105:T30, "NavX Readings"=→"NavX Readings":T16, "Status"=→"Status":T14, "Error Out"=w104:errorcluster)
    n35 = call "FGV Stop.vi"("Init/Read/Write State"=States_for_Action_Engine."Read") -> ("Output node"=w130:bool)  [unwired: 2 in, 1 out]
    n36 = Unbundle By Name(w91) -> ("status"=w89:bool)
    n37 = call "yDistance travelled FGV.vi"("Init/Read/Write State"=States_for_Action_Engine."Read") -> ("Output"=→"Distance to move":dbl)  [unwired: 9 in, 1 out]
    n38 = local write "Red LED"(w89) -> ()
    n39 = Wait (ms)(milliseconds to wait=u32 50) -> ()  [unwired: 1 out]
    "Robot ready" <- "Green LED"
    "Errors detected" <- "Red LED"
  }
  n40 = while {
    tunnel: w62 -> [w148]
    tunnel: w63 -> [w147]
    tunnel: [w146] -> w69
    tunnel: [w145] -> w68
    tunnel: w67 -> [w144]
    tunnel: [w143] -> w65
    tunnel: w66 -> [w142]
    tunnel: [w141] -> w64
    stop <- w139 stop-if-true
    # "Generate USER Event Loop"
    n41 = local read "Rising Edge"() -> (w136:bool)
    n42 = Or(x="OK Button", y=w136) -> (x .or. y?=w135:bool)
    n43 = local read "TASK ENABLE"() -> (w134:bool)
    n44 = And(x=w135, y=w134) -> (x .and. y?=w133:bool)
    n45 = case shown="True" w133 {
      selector: w133 -> [_ w159]
      tunnel: w148 -> [w158 w163]
      tunnel: [w158 w162] -> w145
      tunnel: w144 -> [w157 w161]
      tunnel: [w157 w160] -> w143
      frame False {
      }
      frame True {
        n46 = Generate User Event(user event=w163, event data cluster=w159, error in=w161) -> (user event out=w162:refnum<user-event>, error out=w160:errorcluster)  [unwired: 1 in]
      }
    }
    n47 = case shown="False" "STOP" {
      selector: "STOP" -> [_ w152]
      tunnel: w147 -> [w151 w156]
      tunnel: [w151 w155] -> w146
      tunnel: w142 -> [w150 w154]
      tunnel: [w150 w153] -> w141
      tunnel: [FALSE w152] -> w139
      frame False {
      }
      frame True {
        n48 = Generate User Event(user event=w156, event data cluster=w152, error in=w154) -> (user event out=w155:refnum<user-event>, error out=w153:errorcluster)  [unwired: 1 in]
      }
    }
    n49 = Wait (ms)(milliseconds to wait=u32 10) -> ()  [unwired: 1 out]
    n50 = call "FGV Stop.vi"("Init/Read/Write State"=States_for_Action_Engine."Write", "Input Node"=w139) -> ()  [unwired: 1 in, 2 out]
  }
  n51 = while {
    tunnel: w61 -> [w170]
    tunnel: [w169] -> w60
    tunnel: w48 -> [w167]
    tunnel: [w166] -> w59
    tunnel: w54 -> [w165]
    tunnel: [w164] -> w51
    stop <- w168 stop-if-true
    # "EVENT Handling Loop"
    n52 = event shown="[1] <Start Task>: User Event" {
      selector: w170 -> [_ _ _]
      dyn-events: [_ _ _] -> w169
      timeout: _ -> [_ _ _]
      tunnel: [FALSE FALSE w217] -> w168
      tunnel: w167 -> [w175 w184 w215]
      tunnel: [w174 w183 w216] -> w166
      tunnel: w165 -> [w173 w182 w214]
      tunnel: [w172 w181 w213] -> w164
      event Timeout {
        n53 = event-data() -> ()  [unwired: 1 in, 3 out]
        n54 = Enqueue Element(queue=w175, element=Intruction_Type_Definitions."Start Task 1" ("Enum"), error in (no error)=w173) -> (queue out=w174:refnum<queue>, error out=w172:errorcluster)  [unwired: 1 in, 1 out]
      }
      event User Event {
        n55 = event-data() -> ()  [unwired: 1 in, 5 out]
        n56 = call "Arduino Interfacing VI.vi"("AE Mode"=Arduino_Interfacing."Read From Arduino") -> ("Arduino Data"=w178:T17)  [unwired: 3 in, 1 out]
        n57 = Unbundle By Name(w178) -> ("Rotary Switch"=w177:u8)
        n58 = case shown="15" w177 {
          tunnel: [Intruction_Type_Definitions."Start Task 1" ("Enum") Intruction_Type_Definitions."Start Task 2" ("Enum") Intruction_Type_Definitions."Start Task 3" ("Enum") Intruction_Type_Definitions."Start Task 4" ("Enum") Intruction_Type_Definitions."Start Task 5" ("Enum") Intruction_Type_Definitions."Start Task 6" ("Enum") Intruction_Type_Definitions."Start Task 7" ("Enum") Intruction_Type_Definitions."Start Task 8 - BALL" ("Enum") Intruction_Type_Definitions."Start Task 8 - Soap" ("Enum") Intruction_Type_Definitions."Start Task 8 - Gel" ("Enum") Intruction_Type_Definitions."Start Task 8 - Pipe" ("Enum") Intruction_Type_Definitions."Start Task 9" ("Enum") Intruction_Type_Definitions."Start Task 9" ("Enum") Intruction_Type_Definitions."Start Task 9" ("Enum") Intruction_Type_Definitions."Start Task 9" ("Enum") Intruction_Type_Definitions."Start Task 9" ("Enum")] -> w180
          frame 0, Default {
          }
          frame 1 {
          }
          frame 2 {
          }
          frame 3 {
          }
          frame 4 {
          }
          frame 5 {
          }
          frame 6 {
          }
          frame 7 {
          }
          frame 8 {
          }
          frame 9 {
          }
          frame 10 {
          }
          frame 11 {
            # "Task 9: Red Detection"
            n59 = call "Box Colour FGV.vi"("Colour to detect"=Box_Colour_FGV_Colours."Blue", "Init/R/W State"=Box_Colour_FGV_States."Write") -> ()  [unwired: 8 in, 2 out]
          }
          frame 12 {
            # "Task 9: Black Detection"
            n60 = call "Box Colour FGV.vi"("Colour to detect"=Box_Colour_FGV_Colours."Black", "Init/R/W State"=Box_Colour_FGV_States."Write") -> ()  [unwired: 8 in, 2 out]
          }
          frame 13 {
            # "Task 9: Blue Detection"
            n61 = call "Box Colour FGV.vi"("Colour to detect"=Box_Colour_FGV_Colours."Green", "Init/R/W State"=Box_Colour_FGV_States."Write") -> ()  [unwired: 8 in, 2 out]
          }
          frame 14 {
            # "Task 9: Yellow Detection"
            n62 = call "Box Colour FGV.vi"("Colour to detect"=Box_Colour_FGV_Colours."Red", "Init/R/W State"=Box_Colour_FGV_States."Write") -> ()  [unwired: 8 in, 2 out]
          }
          frame 15 {
            # "Task 9: Green Detection"
            n63 = call "Box Colour FGV.vi"("Colour to detect"=Box_Colour_FGV_Colours."Yellow", "Init/R/W State"=Box_Colour_FGV_States."Write") -> ()  [unwired: 8 in, 2 out]
          }
        }
        "Selected Task" <- w180
        n64 = Enqueue Element(queue=w184, element=w180, error in (no error)=w182) -> (queue out=w183:refnum<queue>, error out=w181:errorcluster)  [unwired: 1 in, 1 out]
      }
      event User Event {
        n65 = event-data() -> ("Stop Queue"=w217:bool)  [unwired: 1 in, 4 out]
        n66 = Enqueue Element At Opposite End(queue=w215, element=Intruction_Type_Definitions."Exit" ("Enum"), error in (no error)=w214) -> (queue out=w216:refnum<queue>, error out=w213:errorcluster)  [unwired: 1 in, 1 out]
      }
    }
  }
  n67 = while {
    tunnel: w48 -> [w222]
    tunnel: w49 -> [w279]
    tunnel: w52 -> [w277]
    tunnel: [w276] -> _
    tunnel: [w275] -> w42
    shift-right: [w268] -> _
    shift-left: T9 {"PING_A"=0, "PING_B"=0, "PING_C"=0, "PING_D"=0} -> [w270]
    shift-right: [w262] -> _
    shift-left: State_Type_Definitions,_for_0.26g_versions_and_later_3."Startup" ("Enum") -> [w265]
    shift-right: [w258] -> _
    shift-left: T8 {"xDistance"=0.0, "yDistance"=0.0, "wDistance"=0.0} -> [w260]
    shift-right: [w256] -> _
    shift-left: _ -> [w255]
    shift-right: [w252] -> _
    shift-left: T11 {"Recognized Object"=FALSE, "Object X coordinate"=0.0, "Object Y coordinate"=0.0} -> [w254]
    shift-right: [w249] -> _
    shift-left: T7 {"y Stepper Position"=0, "z Stepper Position"=0} -> [w251]
    shift-right: [w246] -> _
    shift-left: T6 {"Yaw"=0.0, "Compass"=0.0} -> [w248]
    shift-right: [w243] -> _
    shift-left: T3 {"Time up flag"=FALSE, "SET TIME TO CHECK"=0.0} -> [w245]
    shift-right: [w241] -> _
    shift-left: T21 {"yStepper desired"=0} -> [w242]
    shift-right: [w237] -> _
    shift-left: T5 {"Left IR Sensor"=0.0, "Arm IR Sensor"=0.0, "Bottom IR Sensor"=0.0} -> [w239]
    shift-right: [w235] -> _
    shift-left: T20 {"ySpeed"=0.0, "xSpeed"=0.0, "wSpeed"=0.0} -> [w236]
    shift-right: [w232] -> _
    shift-left: T4 {"Line Detected?"=FALSE, "S1"=0.0, "S2"=0.0, "S3"=0.0, "S4"=0.0} -> [w234]
    shift-right: [w230] -> _
    shift-left: _ -> [w229]
    shift-right: [w221] -> _
    shift-left: T1 {"Red"=FALSE, "Black"=FALSE, "Blue"=FALSE, "Yellow"=FALSE, "Green"=FALSE, "Unknown"=FALSE, "Image processing done"=FALSE, "Colour"=enum."None"} -> [w224]
    stop <- w267 stop-if-true
    # ">>> Box Colour Detection >>>"
    # ">>State Logic Queue Reference >>"
    # ">>Action Queue>>"
    # ">>State Logic Queue Reference >>"
    # ">>> Line Sensor Cluster>>>"
    # ">>> IR Sensors >>>"
    # ">>> Time cluster >>>"
    # ">>> Object detection >>>"
    # ">>> Yaw >>>"
    # ">>> Ultrasonic Sensors Detect >>>"
    # ">>> Encoders >>>"
    # ">>> Stepper position >>>"
    # ">>State Logic  >>"
    # ">> Item Selection Bias >>"
    # ">> Item Selection Bias >>"
    # ">> Item Selection Bias >>"
    # ">>State Logic  >>"
    # ">>> Motor control cluster >>>"
    # ">>> yStepper command>>>"
    # ">>True Stop Next State >>"
    # ">>Error  >>"
    # ">>Timeout>>"
    # ">>Action states Queue Reference >>"
    # "TOP LEVEL BASELINE (MAIN PROCESSING LOOP)"
    n68 = Wait (ms)(milliseconds to wait=u32 25) -> ()  [unwired: 1 out]
    n69 = Dequeue Element(queue=w279, timeout in ms (-1)=0, error in (no error)=w277) -> (queue out=w271:refnum<queue>, element=w278:string, error out=w272:errorcluster)  [unwired: 1 out]
    "Action State" <- w278
    n70 = case shown="\"FORWARD - IR ASSIST\"" w278 {
      tunnel: [_ _ _ _ _ _ _ _ _ _ _ _ _ _ _ _ _ _ _ _ _ _ 0 w3975 _ _ _ _ _ _ _ _ _ _ _ _ _ _ _ _ _ _ _ _ _ _ _ _ _ _ _ _ _ _ _ _ _ _ _] -> w274
      tunnel: w271 -> [_ _ _ _ _ _ _ _ _ _ _ _ _ _ _ _ _ _ _ _ _ _ _ _ _ _ _ _ _ _ _ _ _ _ _ _ _ _ _ _ _ _ _ _ _ _ _ _ _ _ _ _ _ _ _ _ _ _ _]
      tunnel: w270 -> [w3616 w3628 w3643 w3657 w3677 w3692 w3706 w3720 w3734 w3748 w3764 w3779 w3793 w3803 w3821 w3838 w3853 w3868 w3892 w3902 w3936 w3949 w3963 w3976 w3988 w4001 w4021 w4056 w4093 w4107 w4120 w4132 w4145 w4160 w4176 w4188 w4200 w4220 w4243 w4254 w4270 w4301 w4311 w4324 w4337 w4350 w4360 w4378 w4388 w4407 w4416 w4432 w4448 w4464 w4480 w4496 w4510 w4525 w4545]
      tunnel: [w3616 w3628 w3643 w3657 w3677 w3692 w3706 w3720 w3734 w3748 w3764 w3779 w3793 w3803 w3821 w3839 w3853 w3868 w3892 w3902 w3937 w3949 w3963 w3976 w3988 w4001 w4021 w4055 w4092 w4107 w4120 w4132 w4145 w4160 w4176 w4188 w4200 w4220 w4243 w4254 w4270 w4301 w4311 w4324 w4337 w4350 w4360 w4378 w4388 w4407 w4416 w4432 w4448 w4464 w4480 w4496 w4510 w4525 w4545] -> w269
      tunnel: [TRUE TRUE _ _ _ _ _ _ _ _ _ _ _ _ _ _ _ _ _ _ _ _ _ _ _ _ _ _ _ _ _ _ _ _ _ _ _ _ _ _ _ _ _ _ _ _ _ _ _ _ _ _ _ _ _ _ _ _ _] -> w267
      tunnel: w265 -> [w3614 w3626 w3642 w3656 w3676 w3691 w3705 w3719 w3733 w3747 w3763 w3778 w3792 w3802 w3820 w3837 w3852 w3866 w3885 w3901 w3935 w3948 w3960 w3973 w3987 w4000 w4020 w4054 w4091 w4106 w4119 w4131 w4137 w4159 w4175 w4187 w4199 w4219 w4242 w4253 w4264 w4295 w4310 w4323 w4336 w4349 w4359 w4369 w4387 w4406 w4415 w4431 w4447 w4463 w4479 w4495 w4509 w4515 w4533]
      tunnel: [_ _ _ _ _ _ _ _ _ _ _ _ _ _ _ _ _ _ _ _ _ _ _ TRUE _ _ _ _ _ _ _ _ _ _ _ _ _ _ _ _ _ _ _ _ _ _ _ _ _ _ _ _ _ _ _ _ _ _ _] -> w264
      tunnel: [w3614 w3626 w3642 w3656 w3676 w3691 w3705 w3719 w3733 w3747 w3763 w3778 w3792 w3802 w3820 w3837 w3852 w3866 w3885 w3901 w3935 w3948 w3960 w3973 w3987 w4000 w4020 w4054 w4091 w4106 w4119 w4131 w4137 w4159 w4175 w4187 w4199 w4219 w4242 w4253 w4264 w4295 w4310 w4323 w4336 w4349 w4359 w4369 w4387 w4406 w4415 w4431 w4447 w4463 w4479 w4495 w4509 w4515 w4533] -> w263
      tunnel: w260 -> [w3613 w3625 w3641 w3659 w3675 w3690 w3704 w3718 w3732 w3746 w3762 w3777 w3791 w3804 w3819 w3836 w3854 w3870 w3887 w3903 w3934 w3950 w3959 w3972 w3989 w4002 w4016 w4045 w4081 w4105 w4122 w4133 w4142 w4161 w4177 w4189 w4201 w4221 w4244 w4256 w4268 w4299 w4313 w4326 w4339 w4352 w4362 w4373 w4390 w4409 w4418 w4434 w4450 w4466 w4482 w4498 w4512 w4517 w4538]
      tunnel: [w3613 w3625 w3641 w3659 w3675 w3690 w3704 w3718 w3732 w3746 w3762 w3777 w3791 w3804 w3818 w3836 w3854 w3870 w3887 w3903 w3933 w3950 w3959 w3972 w3989 w4002 w4016 w4044 w4080 w4105 w4122 w4133 w4142 w4161 w4177 w4189 w4201 w4221 w4244 w4256 w4268 w4299 w4313 w4326 w4339 w4352 w4362 w4373 w4390 w4409 w4418 w4434 w4450 w4466 w4482 w4498 w4512 w4517 w4538] -> w259
      tunnel: w254 -> [w3612 w3624 w3640 w3658 w3674 w3689 w3703 w3717 w3731 w3745 w3761 w3776 w3789 w3801 w3817 w3835 w3847 w3869 w3886 w3900 w3925 w3947 w3958 w3971 w3986 w3999 w4019 w4049 w4086 w4103 w4121 w4130 w4143 w4158 w4174 w4183 w4198 w4217 w4237 w4255 w4269 w4300 w4312 w4325 w4338 w4351 w4361 w4372 w4389 w4408 w4417 w4433 w4449 w4465 w4481 w4497 w4511 w4516 w4537]
      tunnel: [w3612 w3624 w3640 w3658 w3674 w3689 w3703 w3717 w3731 w3745 w3761 w3776 w3789 w3801 w3817 w3835 w3847 w3869 w3886 w3900 w3924 w3947 w3958 w3971 w3986 w3999 w4018 w4048 w4085 w4103 w4121 w4130 w4143 w4158 w4174 w4183 w4198 w4216 w4237 w4255 w4269 w4300 w4312 w4325 w4338 w4351 w4361 w4372 w4389 w4408 w4417 w4433 w4449 w4465 w4481 w4497 w4511 w4516 w4537] -> w253
      tunnel: w251 -> [w3611 w3623 w3639 w3660 w3673 w3688 w3702 w3716 w3730 w3744 w3760 w3775 w3788 w3800 w3816 w3834 w3855 w3871 w3888 w3899 w3930 w3946 w3957 w3970 w3985 w3998 w4015 w4040 w4076 w4102 w4118 w4129 w4141 w4157 w4173 w4186 w4197 w4222 w4245 w4257 w4267 w4298 w4309 w4322 w4335 w4348 w4363 w4374 w4391 w4405 w4419 w4435 w4451 w4467 w4483 w4499 w4513 w4518 w4539]
      tunnel: [w3611 w3623 w3639 w3660 w3673 w3688 w3702 w3716 w3730 w3744 w3760 w3775 w3788 w3800 w3816 w3834 w3855 w3871 w3888 w3899 w3929 w3946 w3957 w3970 w3985 w3998 w4015 w4039 w4075 w4102 w4118 w4129 w4141 w4157 w4173 w4186 w4197 w4222 w4245 w4257 w4267 w4298 w4309 w4322 w4335 w4348 w4363 w4374 w4391 w4404 w4419 w4435 w4451 w4467 w4483 w4499 w4513 w4518 w4539] -> w250
      tunnel: w248 -> [w3610 w3622 w3637 w3661 w3671 w3686 w3700 w3715 w3729 w3743 w3758 w3773 w3787 w3799 w3815 w3827 w3850 w3872 w3889 w3898 w3920 w3945 w3956 w3969 w3984 w3997 w4014 w4036 w4072 w4101 w4115 w4128 w4140 w4156 w4172 w4185 w4196 w4223 w4246 w4258 w4266 w4297 w4308 w4321 w4334 w4345 w4364 w4375 w4392 w4399 w4420 w4436 w4452 w4468 w4484 w4500 w4514 w4519 w4540]
      tunnel: [w3610 w3622 w3637 w3661 w3671 w3686 w3700 w3715 w3729 w3743 w3758 w3773 w3787 w3799 w3815 w3827 w3849 w3872 w3889 w3898 w3919 w3945 w3956 w3969 w3984 w3997 w4014 w4035 w4071 w4101 w4115 w4128 w4140 w4156 w4172 w4185 w4196 w4223 w4246 w4258 w4266 w4297 w4308 w4321 w4334 w4345 w4364 w4375 w4392 w4399 w4420 w4436 w4452 w4468 w4484 w4500 w4514 w4519 w4540] -> w247
      tunnel: w245 -> [w3608 w3621 w3638 w3662 w3672 w3687 w3701 w3714 w3728 w3742 w3759 w3774 w3786 w3798 w3814 w3826 w3846 w3873 w3890 w3897 w3916 w3942 w3955 w3968 w3983 w3996 w4013 w4033 w4069 w4099 w4114 w4127 w4139 w4155 w4171 w4184 w4195 w4224 w4247 w4259 w4265 w4296 w4307 w4320 w4333 w4344 w4365 w4376 w4393 w4398 w4414 w4430 w4446 w4462 w4478 w4494 w4508 w4520 w4541]
      tunnel: [w3608 w3621 w3638 w3662 w3672 w3687 w3701 w3714 w3728 w3742 w3759 w3774 w3786 w3798 w3814 w3826 w3846 w3873 w3890 w3897 w3916 w3942 w3955 w3968 w3983 w3996 w4012 w4032 w4068 w4099 w4114 w4127 w4139 w4155 w4171 w4184 w4195 w4224 w4247 w4259 w4265 w4296 w4307 w4320 w4333 w4344 w4365 w4376 w4393 w4398 w4414 w4428 w4444 w4460 w4476 w4493 w4507 w4520 w4541] -> w244
      tunnel: w242 -> [_ _ _ _ _ _ _ _ _ _ _ _ _ _ _ _ _ _ _ _ _ _ _ _ _ _ _ _ _ _ _ _ _ _ _ _ _ _ _ _ _ _ _ _ _ _ _ _ w4384 _ _ _ _ _ _ _ _ _ _]
      tunnel: [w3607 w3620 w3632 w3652 w3666 w3681 w3696 w3710 w3724 w3738 w3754 w3768 w3783 w3797 w3808 w3825 w3843 w3864 w3891 w3896 w3913 w3941 w3954 w3967 w3982 w3993 w4006 w4026 w4060 w4098 w4113 w4126 w4144 w4149 w4165 w4181 w4193 w4212 w4240 w4251 w4271 w4302 w4306 w4319 w4332 w4343 w4356 w4377 w4382 w4397 w4413 w4426 w4442 w4458 w4474 w4491 w4504 w4524 w4544] -> w238
      tunnel: w239 -> [w3607 w3620 w3632 w3652 w3666 w3681 w3696 w3710 w3724 w3738 w3754 w3768 w3783 w3797 w3808 w3825 w3843 w3865 w3891 w3896 w3913 w3941 w3954 w3967 w3982 w3993 w4006 w4027 w4061 w4098 w4113 w4126 w4144 w4149 w4165 w4181 w4193 w4212 w4240 w4251 w4271 w4302 w4306 w4319 w4332 w4343 w4356 w4377 w4382 w4397 w4413 w4426 w4442 w4458 w4474 w4491 w4504 w4524 w4544]
      tunnel: w236 -> [_ _ _ _ _ _ _ _ _ _ w3753 _ _ _ _ _ _ _ _ _ _ _ _ _ _ _ _ _ _ _ _ _ _ _ _ _ _ _ _ _ _ _ _ _ _ _ _ _ _ _ _ _ _ _ _ _ _ _ _]
      tunnel: w234 -> [w3606 w3619 w3631 w3646 w3665 w3680 w3695 w3709 w3723 w3737 w3751 w3767 w3782 w3796 w3807 w3824 w3842 w3860 w3884 w3895 w3911 w3940 w3953 w3966 w3981 w3992 w4009 w4029 w4064 w4097 w4112 w4125 w4136 w4148 w4164 w4180 w4192 w4210 w4239 w4250 w4262 w4294 w4305 w4318 w4331 w4342 w4355 w4368 w4381 w4396 w4412 w4425 w4441 w4457 w4473 w4490 w4503 w4523 w4543]
      tunnel: [w3606 w3619 w3631 w3646 w3665 w3680 w3695 w3709 w3723 w3737 w3751 w3767 w3782 w3796 w3807 w3824 w3842 w3860 w3883 w3895 w3911 w3940 w3953 w3966 w3981 w3992 w4008 w4028 w4063 w4097 w4112 w4125 w4136 w4148 w4164 w4180 w4192 w4210 w4239 w4250 w4262 w4294 w4305 w4318 w4331 w4342 w4355 w4368 w4381 w4396 w4412 w4425 w4441 w4457 w4473 w4490 w4503 w4523 w4543] -> w233
      tunnel: [_ _ _ _ _ _ _ _ _ _ _ _ _ _ _ _ _ _ _ _ _ _ _ _ _ _ _ _ _ _ _ _ _ _ _ _ _ w4204 w4234 _ _ _ _ _ _ _ _ _ _ _ _ _ _ _ _ _ _ _ _] -> w231
      tunnel: w229 -> [w3605 w3618 w3630 w3645 w3664 w3679 w3694 w3708 w3722 w3736 w3750 w3766 w3781 w3795 w3806 w3823 w3841 w3859 w3875 w3894 w3909 w3939 w3952 w3965 w3980 w3991 w4010 w4030 w4065 w4096 w4111 w4124 w4135 w4147 w4163 w4179 w4191 w4206 w4238 w4249 w4261 w4293 w4304 w4317 w4330 w4341 w4354 w4367 w4380 w4395 w4411 w4424 w4440 w4456 w4472 w4489 w4502 w4522 w4542]
      tunnel: [w3605 w3618 w3630 w3645 w3664 w3679 w3694 w3708 w3722 w3736 w3750 w3766 w3781 w3795 w3806 w3823 w3841 w3859 w3875 w3894 w3909 w3939 w3952 w3965 w3980 w3991 w4010 w4030 w4065 w4096 w4111 w4124 w4135 w4147 w4163 w4179 w4191 w4206 w4238 w4249 w4261 w4293 w4304 w4317 w4330 w4341 w4354 w4367 w4380 w4395 w4411 w4424 w4440 w4456 w4472 w4489 w4502 w4522 w4542] -> w228
      tunnel: w224 -> [w3604 w3617 w3629 w3644 w3663 w3678 w3693 w3707 w3721 w3735 w3749 w3765 w3780 w3794 w3805 w3822 w3840 w3856 w3874 w3893 w3908 w3938 w3951 w3964 w3979 w3990 w4005 w4023 w4059 w4095 w4110 w4123 w4134 w4146 w4162 w4178 w4190 w4209 w4232 w4248 w4260 w4292 w4303 w4316 w4329 w4340 w4353 w4366 w4379 w4394 w4410 w4423 w4439 w4455 w4471 w4488 w4501 w4521 w4536]
      tunnel: [w3604 w3617 w3629 w3644 w3663 w3678 w3693 w3707 w3721 w3735 w3749 w3765 w3780 w3794 w3805 w3822 w3840 w3856 w3874 w3893 w3908 w3938 w3951 w3964 w3979 w3990 w4004 w4023 w4059 w4095 w4110 w4123 w4134 w4146 w4162 w4178 w4190 w4209 w4225 w4248 w4260 w4291 w4303 w4316 w4329 w4340 w4353 w4366 w4379 w4394 w4410 w4423 w4439 w4455 w4471 w4488 w4501 w4521 w4535] -> w223
      frame "Exit" {
        # ">>State Logic  >>"
        # ">>> Time cluster >>>"
        # ">>> Yaw >>>"
        # ">>> Stepper position >>>"
        # ">>> Encoders >>>"
        # ">>> Object detection >>>"
        # ">>> Ultrasonic Sensors Detect >>>"
        n71 = call "Imaq Dispose"("All Images? (No)"=TRUE) -> ()  [unwired: 5 in, 1 out]
      }
      frame "----Movement States----" {
        # ">>State Logic  >>"
        # ">>> Time cluster >>>"
        # ">>> Yaw >>>"
        # ">>> Stepper position >>>"
        # ">>> Encoders >>>"
        # ">>> Object detection >>>"
        # ">>> Ultrasonic Sensors Detect >>>"
      }
      frame "FORWARD" {
        # "High voltage values: 30\nMid voltage values: 40\nLow voltage values: 50"
        # ">>State Logic  >>"
        # ">>> Time cluster >>>"
        # ">>> Yaw >>>"
        # ">>> Stepper position >>>"
        # ">>> Encoders >>>"
        # ">>> Object detection >>>"
        # ">>> Ultrasonic Sensors Detect >>>"
        n72 = Unbundle By Name(w3637) -> ("Yaw"=w3633:dbl)
        n73 = call "MOTOR CONTROL WITH PID AE.vi"("Yaw"=w3633, "Speed"=30.0, "Direction"=MOTOR_CONTROL_WITH_PID_AE_DIRECTION_TYPE_DEF."y-axis movement", "AE Mode"=MOTOR_CONTROL_WITH_PID_AE_DATA_MODE_TYPE_DEF."Write to AE") -> ()  [unwired: 1 out]
      }
      frame "FORWARD - IR ASSIST" {
        # "Algorithm sensitivity"
        # "Distance to maintain from wall"
        # ">>State Logic  >>"
        # ">>> Time cluster >>>"
        # ">>> Yaw >>>"
        # ">>> Stepper position >>>"
        # ">>> Encoders >>>"
        # ">>> Object detection >>>"
        # ">>> Ultrasonic Sensors Detect >>>"
        n74 = Unbundle By Name(w3652) -> ("Left IR Sensor"=w3651:dbl)
        n75 = Subtract(x=w3651, y=25.0) -> (x-y=w3649:dbl)
        n76 = Multiply(x=w3649, y=0.2) -> (x*y=w3647:dbl)
        n77 = call "MOTOR CONTROL WITH PID AE.vi"("Yaw"=w3647, "Speed"=35.0, "Direction"=MOTOR_CONTROL_WITH_PID_AE_DIRECTION_TYPE_DEF."y-axis movement", "AE Mode"=MOTOR_CONTROL_WITH_PID_AE_DATA_MODE_TYPE_DEF."Write to AE") -> ()  [unwired: 1 out]
      }
      frame "LEFT" {
        # ">>State Logic  >>"
        # ">>> Time cluster >>>"
        # ">>> Yaw >>>"
        # ">>> Stepper position >>>"
        # ">>> Encoders >>>"
        # ">>> Object detection >>>"
        # ">>> Ultrasonic Sensors Detect >>>"
        n78 = Unbundle By Name(w3671) -> ("Yaw"=w3668:dbl)
        n79 = call "MOTOR CONTROL WITH PID AE.vi"("Yaw"=w3668, "Speed"=-25.0, "Direction"=MOTOR_CONTROL_WITH_PID_AE_DIRECTION_TYPE_DEF."x-axis movement", "AE Mode"=MOTOR_CONTROL_WITH_PID_AE_DATA_MODE_TYPE_DEF."Write to AE") -> ()  [unwired: 1 out]
      }
      frame "RIGHT" {
        # ">>> Time cluster >>>"
        # ">>> Yaw >>>"
        # ">>> Stepper position >>>"
        # ">>> Encoders >>>"
        # ">>> Object detection >>>"
        # ">>> Ultrasonic Sensors Detect >>>"
        n80 = Unbundle By Name(w3686) -> ("Yaw"=w3682:dbl)
        n81 = call "MOTOR CONTROL WITH PID AE.vi"("Yaw"=w3682, "Speed"=25.0, "Direction"=MOTOR_CONTROL_WITH_PID_AE_DIRECTION_TYPE_DEF."x-axis movement", "AE Mode"=MOTOR_CONTROL_WITH_PID_AE_DATA_MODE_TYPE_DEF."Write to AE") -> ()  [unwired: 1 out]
      }
      frame "R-ACW" {
        # ">>> IR Sensors >>>"
        # ">>> Time cluster >>>"
        # ">>> Yaw >>>"
        # ">>> Stepper position >>>"
        # ">>> Encoders >>>"
        # ">>> Object detection >>>"
        # ">>> Ultrasonic Sensors Detect >>>"
        n82 = call "MOTOR CONTROL WITH PID AE.vi"("Speed"=10.0, "Direction"=MOTOR_CONTROL_WITH_PID_AE_DIRECTION_TYPE_DEF."rotation", "AE Mode"=MOTOR_CONTROL_WITH_PID_AE_DATA_MODE_TYPE_DEF."Write to AE") -> ()  [unwired: 1 in, 1 out]
      }
      frame "R-CW" {
        (unwired) -0.2 ("Speed")
        # ">>> Time cluster >>>"
        # ">>> Yaw >>>"
        # ">>> Stepper position >>>"
        # ">>> Encoders >>>"
        # ">>> Object detection >>>"
        # ">>> Ultrasonic Sensors Detect >>>"
        n83 = call "MOTOR CONTROL WITH PID AE.vi"("Speed"=-8.0, "Direction"=MOTOR_CONTROL_WITH_PID_AE_DIRECTION_TYPE_DEF."rotation", "AE Mode"=MOTOR_CONTROL_WITH_PID_AE_DATA_MODE_TYPE_DEF."Write to AE") -> ()  [unwired: 1 in, 1 out]
      }
      frame "R-ACW SLOW" {
        (unwired) -0.2 ("Speed")
        # ">>> Time cluster >>>"
        # ">>> Yaw >>>"
        # ">>> Stepper position >>>"
        # ">>> Encoders >>>"
        # ">>> Object detection >>>"
        # ">>> Ultrasonic Sensors Detect >>>"
        n84 = call "MOTOR CONTROL WITH PID AE.vi"("Speed"=5.0, "Direction"=MOTOR_CONTROL_WITH_PID_AE_DIRECTION_TYPE_DEF."rotation", "AE Mode"=MOTOR_CONTROL_WITH_PID_AE_DATA_MODE_TYPE_DEF."Write to AE") -> ()  [unwired: 1 in, 1 out]
      }
      frame "R-CW SLOW" {
        (unwired) -0.2 ("Speed")
        # ">>> Time cluster >>>"
        # ">>> Yaw >>>"
        # ">>> Stepper position >>>"
        # ">>> Encoders >>>"
        # ">>> Object detection >>>"
        # ">>> Ultrasonic Sensors Detect >>>"
        n85 = call "MOTOR CONTROL WITH PID AE.vi"("Speed"=-5.0, "Direction"=MOTOR_CONTROL_WITH_PID_AE_DIRECTION_TYPE_DEF."rotation", "AE Mode"=MOTOR_CONTROL_WITH_PID_AE_DATA_MODE_TYPE_DEF."Write to AE") -> ()  [unwired: 1 in, 1 out]
      }
      frame "X AXIS - SLOW" {
        # ">>> Line Sensor Cluster>>>"
        # ">>> IR Sensors >>>"
        # ">>> Time cluster >>>"
        # ">>> Yaw >>>"
        # ">>> Stepper position >>>"
        # ">>> Encoders >>>"
        # ">>> Object detection >>>"
        # ">>> Ultrasonic Sensors Detect >>>"
        n86 = Unbundle By Name(w3753) -> ("xSpeed"=w3752:dbl)
        n87 = Unbundle By Name(w3758) -> ("Yaw"=w3755:dbl)
        n88 = call "MOTOR CONTROL WITH PID AE.vi"("Yaw"=w3755, "Speed"=w3752, "Direction"=MOTOR_CONTROL_WITH_PID_AE_DIRECTION_TYPE_DEF."x-axis movement", "AE Mode"=MOTOR_CONTROL_WITH_PID_AE_DATA_MODE_TYPE_DEF."Write to AE") -> ()  [unwired: 1 out]
      }
      frame "REVERSE" {
        # ">>> Time cluster >>>"
        # ">>> Yaw >>>"
        # ">>> Stepper position >>>"
        # ">>> Encoders >>>"
        # ">>> Object detection >>>"
        # ">>> Ultrasonic Sensors Detect >>>"
        n89 = Unbundle By Name(w3773) -> ("Yaw"=w3769:dbl)
        n90 = call "MOTOR CONTROL WITH PID AE.vi"("Yaw"=w3769, "Speed"=-40.0, "Direction"=MOTOR_CONTROL_WITH_PID_AE_DIRECTION_TYPE_DEF."y-axis movement", "AE Mode"=MOTOR_CONTROL_WITH_PID_AE_DATA_MODE_TYPE_DEF."Write to AE") -> ()  [unwired: 1 out]
      }
      frame "STOP" {
        n91 = Wait (ms)(milliseconds to wait=u32 100) -> ()  [unwired: 1 out]
        n92 = call "MOTOR CONTROL WITH PID AE.vi"("Direction"=MOTOR_CONTROL_WITH_PID_AE_DIRECTION_TYPE_DEF."stop", "AE Mode"=MOTOR_CONTROL_WITH_PID_AE_DATA_MODE_TYPE_DEF."Write to AE") -> ()  [unwired: 2 in, 1 out]
      }
      frame "----SENSOR READING---- " {
      }
      frame "READ ENCODERS" {
        # ">>> Time cluster >>>"
        # ">>> Yaw >>>"
        # ">>> Stepper position >>>"
        # ">>> Object detection >>>"
        # ">>> Current encoder distance >>>"
        # ">>> Ultrasonic Sensors Detect >>>"
        n93 = call "MOTOR CONTROL WITH PID AE.vi"("AE Mode"=MOTOR_CONTROL_WITH_PID_AE_DATA_MODE_TYPE_DEF."Read from AE") -> ("Speed & distance"=w3812:T15)  [unwired: 3 in]
        n94 = Unbundle By Name(w3812) -> ("xDistance"=w3811:dbl, "yDistance"=w3810:dbl, "wDistance"=w3809:dbl)
        n95 = Bundle By Name(cluster=w3819, "xDistance"=w3811, "yDistance"=w3810, "wDistance"=w3809) -> (w3818:T8)
      }
      frame "READ ULTRASONIC" {
        (unwired) navX_type_def."Read Values" ("Mode")
        (unwired) MOTOR_CONTROL_NO_PID_Type_Def."Latch" ("Direction")
        # ">>> Line Sensor Cluster>>>"
        # ">>> IR Sensors >>>"
        # ">>State Logic  >>"
        # ">>> Time cluster >>>"
        # ">>> Ultrasonic Sensors Detect >>>"
        # ">>> Object detection >>>"
        # ">>> Encoders >>>"
        # ">>> Stepper position >>>"
        # ">>> Yaw >>>"
        n96 = call "Arduino Interfacing VI.vi"("AE Mode"=Arduino_Interfacing."Read From Arduino") -> ("Arduino Data"=w3832:T17)  [unwired: 3 in, 1 out]
        n97 = Unbundle By Name(w3832) -> ("PING A"=w3831:u8, "PING B"=w3830:u8, "PING C"=w3829:u8, "PING D"=w3828:u8)
        n98 = Bundle By Name(cluster=w3838, "PING_A"=w3831, "PING_B"=w3830, "PING_C"=w3829, "PING_D"=w3828) -> (w3839:T9)
      }
      frame "READ NAVX" {
        # ">> Item Selection Bias >>"
        # ">>State Logic  >>"
        # ">>> Line Sensor Cluster>>>"
        # ">>> IR Sensors >>>"
        # ">>> Time cluster >>>"
        # ">>> Yaw >>>"
        # ">>> Ultrasonic Sensors Detect >>>"
        # ">>> Object detection >>>"
        # ">>> Encoders >>>"
        # ">>> Stepper position >>>"
        n99 = call "navX reading VI.vi"("Mode"=navX_type_def."Read Values") -> ("NavX Readings"=w3845:T16)  [unwired: 2 in, 3 out]
        n100 = Unbundle By Name(w3845) -> ("Heading"=w3844:dbl)
        n101 = Unbundle By Name(w3845) -> ("Yaw"=w3848:dbl)
        n102 = Bundle By Name(cluster=w3850, "Yaw"=w3848, "Compass"=w3844) -> (w3849:T6)
      }
      frame "READ IR" {
        w3858 = T41 [enum."B/AI2"] items=["Not Connected", "AudioIn/Left", "AudioIn/Right", "C/AI0", "C/AI1", "A/AI0", "A/AI1", "A/AI2", "A/AI3", "A/AI4", "A/AI5", "A/AI6", "A/AI7", "B/AI0", "B/AI1", "B/AI2", "B/AI3", "B/AI4", "B/AI5", "B/AI6", "B/AI7", "AI/AI0", "AI/AI1", "AI/AI2", "AI/AI3", "A/AI0 (DIFF)", "A/AI1 (DIFF)", "A/AI2 (DIFF)", "A/AI3 (DIFF)", "B/AI0 (DIFF)", "B/AI1 (DIFF)", "B/AI2 (DIFF)", "B/AI3 (DIFF)"] ("AI Channel")
        w3862 = T41 [enum."B/AI1"] items=["Not Connected", "AudioIn/Left", "AudioIn/Right", "C/AI0", "C/AI1", "A/AI0", "A/AI1", "A/AI2", "A/AI3", "A/AI4", "A/AI5", "A/AI6", "A/AI7", "B/AI0", "B/AI1", "B/AI2", "B/AI3", "B/AI4", "B/AI5", "B/AI6", "B/AI7", "AI/AI0", "AI/AI1", "AI/AI2", "AI/AI3", "A/AI0 (DIFF)", "A/AI1 (DIFF)", "A/AI2 (DIFF)", "A/AI3 (DIFF)", "B/AI0 (DIFF)", "B/AI1 (DIFF)", "B/AI2 (DIFF)", "B/AI3 (DIFF)"] ("AI Channel")
        w3867 = T41 [enum."B/AI0"] items=["Not Connected", "AudioIn/Left", "AudioIn/Right", "C/AI0", "C/AI1", "A/AI0", "A/AI1", "A/AI2", "A/AI3", "A/AI4", "A/AI5", "A/AI6", "A/AI7", "B/AI0", "B/AI1", "B/AI2", "B/AI3", "B/AI4", "B/AI5", "B/AI6", "B/AI7", "AI/AI0", "AI/AI1", "AI/AI2", "AI/AI3", "A/AI0 (DIFF)", "A/AI1 (DIFF)", "A/AI2 (DIFF)", "A/AI3 (DIFF)", "B/AI0 (DIFF)", "B/AI1 (DIFF)", "B/AI2 (DIFF)", "B/AI3 (DIFF)"] ("AI Channel")
        # ">>> Line Sensor Cluster>>>"
        # ">>> IR Sensors >>>"
        # ">>State Logic  >>"
        # ">>> Time cluster >>>"
        # ">>> Ultrasonic Sensors Detect >>>"
        # ">>> Object detection >>>"
        # ">>> Encoders >>>"
        # ">>> Stepper position >>>"
        # ">>> Yaw >>>"
        n103 = call <vilib>:"Sharp IR.vi"("AI Channel"=w3867) -> ("Sharp IR Distance"=w3863:dbl)  [unwired: 8 in, 2 out]
        n104 = call <vilib>:"Sharp IR.vi"("AI Channel"=w3862) -> ("Sharp IR Distance"=w3861:dbl)  [unwired: 8 in, 2 out]
        n105 = call <vilib>:"Sharp IR.vi"("AI Channel"=w3858) -> ("Sharp IR Distance"=w3857:dbl)  [unwired: 8 in, 2 out]
        n106 = Bundle By Name(cluster=w3865, "Left IR Sensor"=w3863, "Arm IR Sensor"=w3861, "Bottom IR Sensor"=w3857) -> (w3864:T5)
      }
      frame "READ LINE SENSOR" {
        # ">>> IR Sensors >>>"
        # ">>> Line Sensor Cluster>>>"
        # ">>State Logic  >>"
        # ">>> Time cluster >>>"
        # ">>> Object detection >>>"
        # ">>> Yaw >>>"
        # ">>> Ultrasonic Sensors Detect >>>"
        # ">>> Encoders >>>"
        # ">>> Stepper position >>>"
        n107 = call "Line Sensor AE.vi"("AE State"=Line_Sensor_AE_Type_Def."READ FROM LINE SENSORS") -> ("Line Detected?"=w3881:bool, "Line Sensor Raw Values"=w3880:T43)
        n108 = Unbundle By Name(w3880) -> ("S1"=w3879:dbl, "S2"=w3878:dbl, "S3"=w3877:dbl, "S4"=w3876:dbl)
        n109 = Bundle By Name(cluster=w3884, "Line Detected?"=w3881, "S1"=w3879, "S2"=w3878, "S3"=w3877, "S4"=w3876) -> (w3883:T4)
      }
      frame "----SYSTEM MODES----" {
        (unwired) I2C_MASTER_Type_Def."Last State" ("Arduino Mode")
        # ">>> Object detection >>>"
        # ">>> Yaw >>>"
        # ">>> Ultrasonic Sensors Detect >>>"
        # ">>> Encoders >>>"
        # ">>> Stepper position >>>"
      }
      frame "INIT" {
        w3931 = u8 0
        w3932 = 0.0
        # ">>> Box Colour Detection >>>"
        # ">>> IR Sensors >>>"
        # ">>> IR Sensors >>>"
        # ">>> Line Sensor Cluster>>>"
        # ">>> Time cluster >>>"
        # ">>> Object detection >>>"
        # ">>> Yaw >>>"
        # ">>> Ultrasonic Sensors Detect >>>"
        # ">>> Encoders >>>"
        # ">>> Stepper position >>>"
        # ">>State Logic  >>"
        n110 = call "Arduino Interfacing VI.vi"("AE Mode"=Arduino_Interfacing."Initialize") -> ()  [unwired: 3 in, 2 out]
        n111 = call "FGV Stop.vi"("Init/Read/Write State"=States_for_Action_Engine."Initialize") -> ()  [unwired: 2 in, 2 out]
        n112 = call "Elasped Timer.vi"("Action"=Elapsed_timer_control."Initialize") -> ()  [unwired: 7 in, 4 out]
        n113 = call "MOTOR CONTROL WITH PID AE.vi"("AE Mode"=MOTOR_CONTROL_WITH_PID_AE_DATA_MODE_TYPE_DEF."Init AE") -> ()  [unwired: 3 in, 1 out]
        n114 = call "IMAQ Reference AE.vi"("IMAQ AE States"=IMAQ_Reference_AE."Initialize AE") -> ()  [unwired: 1 in, 2 out]
        n115 = call "Line Sensor AE.vi"("AE State"=Line_Sensor_AE_Type_Def."INIT AE") -> ()  [unwired: 2 out]
        n116 = Bundle By Name(cluster=w3925, "Recognized Object"=FALSE, "Object X coordinate"=0.0, "Object Y coordinate"=0.0) -> (w3924:T11)
        n117 = Bundle By Name(cluster=w3930, "y Stepper Position"=u8 0, "z Stepper Position"=u8 0) -> (w3929:T7)
        n118 = Bundle By Name(cluster=w3934, "xDistance"=w3932, "yDistance"=w3932, "wDistance"=w3932) -> (w3933:T8)
        n119 = Bundle By Name(cluster=w3936, "PING_A"=w3931, "PING_B"=w3931, "PING_C"=w3931, "PING_D"=w3931) -> (w3937:T9)
        n120 = invoke class="VI" method="Default Vals.Reinit All"() -> ()  [unwired: 3 in, 3 out]
        n121 = Bundle By Name(cluster=w3920, "Yaw"=0.0) -> (w3919:T6)
        n122 = call "Box Colour FGV.vi"("Init/R/W State"=Box_Colour_FGV_States."Initialize") -> ()  [unwired: 9 in, 2 out]
        n123 = call "Servo State FGV.vi"("Init/Read/Write State"=States_for_Action_Engine."Initialize") -> ()  [unwired: 2 in, 2 out]
        n124 = call "yDistance travelled FGV.vi"("Init/Read/Write State"=States_for_Action_Engine."Initialize") -> ()  [unwired: 9 in, 2 out]
        n125 = call "Task Enable FGV.vi"("Init/Read/Write State"=States_for_Action_Engine."Initialize") -> ()  [unwired: 9 in, 2 out]
      }
      frame "ARDUINO - ULTRASONIC" {
        # ">>> Time cluster >>>"
        # ">>> Line Sensor Cluster>>>"
        # ">>> Object detection >>>"
        # ">>> Yaw >>>"
        # ">>> Ultrasonic Sensors Detect >>>"
        # ">>> Encoders >>>"
        # ">>> Stepper position >>>"
        # ">>State Logic  >>"
        n126 = call "Arduino Interfacing VI.vi"("Data to Write"=I2C_MASTER_WRITE_NEW_Type_Def."Ultrasonic sensors", "AE Mode"=Arduino_Interfacing."Write to Arduino") -> ()  [unwired: 2 in, 2 out]
      }
      frame "NAVX CALIBRATE" {
        # ">>> Object detection >>>"
        # ">>> Yaw >>>"
        # ">>> Ultrasonic Sensors Detect >>>"
        # ">>> Encoders >>>"
        # ">>> Stepper position >>>"
        # ">>State Logic  >>"
        # "Adds a 15 second delay to the startup process \nfor the NavX to calibrate"
        n127 = Wait (ms)(milliseconds to wait=u32 1000) -> ()  [unwired: 1 out]
      }
      frame "NO ACTION", Default {
        (unwired) u8 0 ("y Stepper value")
        (unwired) TRUE ("Latch")
        (unwired) navX_type_def."Read Values" ("Mode")
        (unwired) MOTOR_CONTROL_NO_PID_Type_Def."Latch" ("Direction")
        # ">>> Object detection >>>"
        # ">>> Yaw >>>"
        # ">>> Ultrasonic Sensors Detect >>>"
        # ">>> Encoders >>>"
        # ">>> Stepper position >>>"
        # ">>State Logic  >>"
        n128 = case shown="\"Idle\"" w3973 {
          tunnel: [0 100] -> w3975
          frame "Startup", Default {
          }
          frame "Idle" {
          }
        }
      }
      frame "----RESET CASES----" {
        (unwired) I2C_MASTER_Type_Def."Last State" ("Arduino Mode")
        # ">>> Object detection >>>"
        # ">>> Yaw >>>"
        # ">>> Ultrasonic Sensors Detect >>>"
        # ">>> Encoders >>>"
        # ">>> Stepper position >>>"
        # ">>State Logic  >>"
      }
      frame "RESET ENCODERS" {
        # ">>> Object detection >>>"
        # ">>> Yaw >>>"
        # ">>> Ultrasonic Sensors Detect >>>"
        # ">>> Encoders >>>"
        # ">>> Stepper position >>>"
        # ">>State Logic  >>"
        n129 = call "MOTOR CONTROL WITH PID AE.vi"("Direction"=MOTOR_CONTROL_WITH_PID_AE_DIRECTION_TYPE_DEF."reset encoders", "AE Mode"=MOTOR_CONTROL_WITH_PID_AE_DATA_MODE_TYPE_DEF."Write to AE") -> ()  [unwired: 2 in, 1 out]
      }
      frame "RESET FLAGS" {
        w4003 = FALSE ("Line Detected?")
        # ">>> Line Sensor Cluster>>>"
        # ">>> IR Sensors >>>"
        # ">>> Time cluster >>>"
        # ">>> Object detection >>>"
        # ">>> Yaw >>>"
        # ">>> Ultrasonic Sensors Detect >>>"
        # ">>> Encoders >>>"
        # ">>> Stepper position >>>"
        # ">>> Line Sensor Cluster>>>"
        # ">>> IR Sensors >>>"
        # ">>> Time cluster >>>"
        # ">>> Object detection >>>"
        # ">>> Yaw >>>"
        # ">>> Ultrasonic Sensors Detect >>>"
        # ">>> Encoders >>>"
        # ">>> Stepper position >>>"
        # "Resets BOOLEAN FLAGS only"
        n130 = Wait (ms)(milliseconds to wait=u32 20) -> ()  [unwired: 1 out]
        n131 = Bundle By Name(cluster=w4019, "Recognized Object"=FALSE) -> (w4018:T11)
        n132 = Bundle By Name(cluster=w4009, "Line Detected?"=FALSE) -> (w4008:T4)
        n133 = Bundle By Name(cluster=w4013, "Time up flag"=FALSE) -> (w4012:T3)
        n134 = Bundle By Name(cluster=w4005, "Red"=w4003, "Black"=w4003, "Blue"=w4003, "Yellow"=w4003, "Green"=w4003, "Unknown"=w4003, "Image processing done"=w4003) -> (w4004:T1)
      }
      frame "RESET SENSOR VALUES" {
        w4024 = 0.0 ("S4")
        w4025 = 0.0 ("S4")
        # "Resets SENSOR VALUES only"
        # ">>> Line Sensor Cluster>>>"
        # ">>> IR Sensors >>>"
        # ">>> Time cluster >>>"
        # ">>> Object detection >>>"
        # ">>> Yaw >>>"
        # ">>> Ultrasonic Sensors Detect >>>"
        # ">>> Encoders >>>"
        # ">>> Stepper position >>>"
        # ">>> Line Sensor Cluster>>>"
        # ">>> IR Sensors >>>"
        # ">>> Time cluster >>>"
        # ">>> Object detection >>>"
        # ">>> Yaw >>>"
        # ">>> Ultrasonic Sensors Detect >>>"
        # ">>> Encoders >>>"
        # ">>> Stepper position >>>"
        # "Resets any software variables\nand/or non-critical states"
        n135 = Wait (ms)(milliseconds to wait=u32 20) -> ()  [unwired: 1 out]
        n136 = Bundle By Name(cluster=w4033, "SET TIME TO CHECK"=0.0) -> (w4032:T3)
        n137 = Bundle By Name(cluster=w4049, "Object X coordinate"=0.0, "Object Y coordinate"=0.0) -> (w4048:T11)
        n138 = Bundle By Name(cluster=w4040, "y Stepper Position"=u8 0, "z Stepper Position"=u8 0) -> (w4039:T7)
        n139 = Bundle By Name(cluster=w4027, "Left IR Sensor"=w4024, "Arm IR Sensor"=w4024) -> (w4026:T5)
        n140 = Bundle By Name(cluster=w4045, "xDistance"=0.0, "yDistance"=0.0, "wDistance"=0.0) -> (w4044:T8)
        n141 = Bundle By Name(cluster=w4056, "PING_A"=u8 0, "PING_B"=u8 0, "PING_C"=u8 0, "PING_D"=u8 0) -> (w4055:T9)
        n142 = Bundle By Name(cluster=w4036, "Yaw"=0.0) -> (w4035:T6)
        n143 = Bundle By Name(cluster=w4029, "S1"=w4025, "S2"=w4025, "S3"=w4025, "S4"=w4025) -> (w4028:T4)
      }
      frame "RESET ALL SENSORS" {
        w4058 = 0.0 ("SET TIME TO CHECK")
        # ">>> Line Sensor Cluster>>>"
        # ">>> IR Sensors >>>"
        # ">>> Time cluster >>>"
        # ">>> Object detection >>>"
        # ">>> Yaw >>>"
        # ">>> Ultrasonic Sensors Detect >>>"
        # ">>> Encoders >>>"
        # ">>> Stepper position >>>"
        # ">>> Line Sensor Cluster>>>"
        # ">>> IR Sensors >>>"
        # ">>> Time cluster >>>"
        # ">>> Object detection >>>"
        # ">>> Yaw >>>"
        # ">>> Ultrasonic Sensors Detect >>>"
        # ">>> Encoders >>>"
        # ">>> Stepper position >>>"
        # "Resets ALL SENSOR PARAMTERS"
        n144 = Wait (ms)(milliseconds to wait=u32 20) -> ()  [unwired: 1 out]
        n145 = Bundle By Name(cluster=w4069, "Time up flag"=FALSE, "SET TIME TO CHECK"=0.0) -> (w4068:T3)
        n146 = Bundle By Name(cluster=w4086, "Recognized Object"=FALSE, "Object X coordinate"=0.0, "Object Y coordinate"=0.0) -> (w4085:T11)
        n147 = Bundle By Name(cluster=w4076, "y Stepper Position"=u8 0, "z Stepper Position"=u8 0) -> (w4075:T7)
        n148 = Bundle By Name(cluster=w4061, "Left IR Sensor"=w4058, "Arm IR Sensor"=w4058, "Bottom IR Sensor"=w4058) -> (w4060:T5)
        n149 = Bundle By Name(cluster=w4064, "Line Detected?"=FALSE) -> (w4063:T4)
        n150 = Bundle By Name(cluster=w4081, "xDistance"=0.0, "yDistance"=0.0, "wDistance"=0.0) -> (w4080:T8)
        n151 = Bundle By Name(cluster=w4093, "PING_A"=u8 0, "PING_B"=u8 0, "PING_C"=u8 0, "PING_D"=u8 0) -> (w4092:T9)
        n152 = Bundle By Name(cluster=w4072, "Yaw"=0.0) -> (w4071:T6)
      }
      frame "RESET YAW" {
        n153 = Wait (ms)(milliseconds to wait=u32 100) -> ()  [unwired: 1 out]
        n154 = call "navX reading VI.vi"("Mode"=navX_type_def."Zero Yaw") -> ()  [unwired: 2 in, 4 out]
      }
      frame "RESET ARM" {
        n155 = call "Arduino Interfacing VI.vi"("Data to Write"=I2C_MASTER_WRITE_NEW_Type_Def."Soft Reset", "AE Mode"=Arduino_Interfacing."Write to Arduino") -> ()  [unwired: 2 in, 2 out]
        n156 = call "Servo State FGV.vi"("Init/Read/Write State"=States_for_Action_Engine."Write", "Servo State"=Servo_States_FGV_Enum."Open Claw") -> ()  [unwired: 1 in, 2 out]
      }
      frame "--------CAM STATES-------" {
      }
      frame "OPEN IMAQ REF" {
        # ">>> Line Sensor Cluster>>>"
        # ">>State Logic  >>"
        # ">>> Time cluster >>>"
        # ">>> Object detection >>>"
        # ">>> Yaw >>>"
        # ">>> Ultrasonic Sensors Detect >>>"
        # ">>> Encoders >>>"
        # ">>> Stepper position >>>"
        # ">>> IR Sensors >>>"
        n157 = call "IMAQ Reference AE.vi"("IMAQ AE States"=IMAQ_Reference_AE."Initialize AE") -> ()  [unwired: 1 in, 2 out]
      }
      frame "OPEN LOG CAM" {
        n158 = call "Webcam AE.vi"("Session In"=T39 "cam0", "Camera states"=Webcam_AE."Initialize Camera") -> ("error out"=w4152:errorcluster, "Session Out"=w4151:T39)  [unwired: 1 in, 1 out]
        n159 = call "Webcam AE.vi"("error in (no error)"=w4152, "Session In"=w4151, "Camera states"=Webcam_AE."Open Camera") -> ()  [unwired: 3 out]
      }
      frame "OPEN LIFE CAM" {
        n160 = call "Webcam AE.vi"("Session In"=T39 "cam1", "Camera states"=Webcam_AE."Initialize Camera") -> ("error out"=w4168:errorcluster, "Session Out"=w4167:T39)  [unwired: 1 in, 1 out]
        n161 = call "Webcam AE.vi"("error in (no error)"=w4168, "Session In"=w4167, "Camera states"=Webcam_AE."Open Camera") -> ()  [unwired: 3 out]
      }
      frame "CAM ACQ" {
        # ">>State Logic  >>"
        # ">>> Time cluster >>>"
        # ">>> Yaw >>>"
        # ">>> Stepper position >>>"
        # ">>> Encoders >>>"
        # ">>> Object detection >>>"
        # ">>> Ultrasonic Sensors Detect >>>"
        n162 = call "Webcam AE.vi"("Camera states"=Webcam_AE."Continuous Acquisition") -> ()  [unwired: 2 in, 3 out]
      }
      frame "CAM CLOSE" {
        # ">>> Box Colour Detection >>>"
        # ">>> Line Sensor Cluster>>>"
        # ">>> IR Sensors >>>"
        # ">>State Logic  >>"
        # ">>> Time cluster >>>"
        # ">>> Yaw >>>"
        # ">>> Stepper position >>>"
        # ">>> Encoders >>>"
        # ">>> Object detection >>>"
        # ">>> Ultrasonic Sensors Detect >>>"
        n163 = call "Webcam AE.vi"("Camera states"=Webcam_AE."Close Camera") -> ()  [unwired: 2 in, 3 out]
      }
      frame "PROCESS IMAGE" {
        # ">>> Line Sensor Cluster>>>"
        # ">>> IR Sensors >>>"
        # ">> Item Selection Bias >>"
        # ">> Item Selection Bias >>"
        # ">>State Logic  >>"
        # ">>> Time cluster >>>"
        # ">>> Yaw >>>"
        # ">>> Stepper position >>>"
        # ">>> Encoders >>>"
        # ">>> Object detection >>>"
        # ">>> Ultrasonic Sensors Detect >>>"
        n164 = call "Webcam AE.vi"("Camera states"=Webcam_AE."Retrieve Image") -> ("error out"=w4205:errorcluster, "Image Out"=w4208:T45)  [unwired: 2 in, 1 out]
        n165 = call "IMAQ Reference AE.vi"("IMAQ AE States"=IMAQ_Reference_AE."Get IMAQ Reference") -> ("Image Out"=w4207:T45)  [unwired: 1 in, 1 out]
        n166 = call "Object Detection SubVI v2.vi"("Error In"=w4205, "Mode"=w4206, "Image Dest"=w4207, "Image in"=w4208) -> ("Error out"=w4204:errorcluster, "Object Center Coordinates"=w4203:cluster{"x":sgl, "y":sgl}, "Object detection cluster"=w4202:T46)  [unwired: 1 out]
        n167 = Unbundle By Name(w4202) -> ("Object detected?"=w4213:bool)
        n168 = Unbundle By Name(w4203) -> ("x"=w4215:sgl, "y"=w4214:sgl)
        n169 = Bundle By Name(cluster=w4217, "Recognized Object"=w4213, "Object X coordinate"=w4215, "Object Y coordinate"=w4214) -> (w4216:T11)
      }
      frame "COLOUR PROCESSING" {
        # ">>> Box Colour Detection >>>"
        # ">>> Box Colour Detection >>>"
        # ">>> Line Sensor Cluster>>>"
        # ">>> IR Sensors >>>"
        # ">> Item Selection Bias >>"
        # ">> Item Selection Bias >>"
        # ">>State Logic  >>"
        # ">>> Time cluster >>>"
        # ">>> Yaw >>>"
        # ">>> Stepper position >>>"
        # ">>> Encoders >>>"
        # ">>> Object detection >>>"
        # ">>> Ultrasonic Sensors Detect >>>"
        n170 = call "Webcam AE.vi"("Camera states"=Webcam_AE."Retrieve Image") -> ("error out"=w4235:errorcluster, "Image Out"=w4236:T45)  [unwired: 2 in, 1 out]
        n171 = call "Box Colour Detection SubVI.vi"("Image In"=w4236, "Error In"=w4235) -> ("Colour output boolean cluster"=w4233:T47, "Error out"=w4234:errorcluster)  [unwired: 1 out]
        n172 = Unbundle By Name(w4233) -> ("Red"=w4231:bool, "Black"=w4230:bool, "Blue"=w4229:bool, "Yellow"=w4228:bool, "Green"=w4227:bool, "No recognizable coolour"=w4226:bool)
        n173 = Bundle By Name(cluster=w4232, "Red"=w4231, "Black"=w4230, "Blue"=w4229, "Yellow"=w4228, "Green"=w4227, "Unknown"=w4226) -> (w4225:T1)
      }
      frame "DISPOSE CAM BUFFERS" {
        # ">> Item Selection Bias >>"
        # ">>> Line Sensor Cluster>>>"
        # ">>> IR Sensors >>>"
        # ">>State Logic  >>"
        # ">>> Time cluster >>>"
        # ">>> Yaw >>>"
        # ">>> Stepper position >>>"
        # ">>> Encoders >>>"
        # ">>> Object detection >>>"
        # ">>> Ultrasonic Sensors Detect >>>"
        n174 = call "Webcam AE.vi"("Camera states"=Webcam_AE."Dispose Camera Image Buffer") -> ()  [unwired: 2 in, 3 out]
      }
      frame "DISPOSE PROC BUFFERS" {
        # ">>> Box Colour Detection >>>"
        # ">>> Line Sensor Cluster>>>"
        # ">>State Logic  >>"
        # ">>> IR Sensors >>>"
        # ">>> Time cluster >>>"
        # ">>> Object detection >>>"
        # ">>> Yaw >>>"
        # ">>> Ultrasonic Sensors Detect >>>"
        # ">>> Encoders >>>"
        # ">>> Stepper position >>>"
        n175 = call "IMAQ Reference AE.vi"("IMAQ AE States"=IMAQ_Reference_AE."Dispose Processing Buffer") -> ()  [unwired: 1 in, 2 out]
      }
      frame "BOX COLOUR" {
        # ">>> Box Colour Detection >>>"
        # ">>> Line Sensor Cluster>>>"
        # ">>State Logic  >>"
        # ">>> IR Sensors >>>"
        # ">>> Time cluster >>>"
        # ">>> Object detection >>>"
        # ">>> Yaw >>>"
        # ">>> Ultrasonic Sensors Detect >>>"
        # ">>> Encoders >>>"
        # ">>> Stepper position >>>"
        n176 = call "Box Colour Detection Sequence.vi"() -> ("Colour scan time out?"=w4288:bool, "Colour output boolean cluster"=w4290:T47)  [unwired: 9 in, 1 out]
        n177 = Unbundle By Name(w4290) -> ("Red"=w4287:bool, "Black"=w4283:bool, "Blue"=w4280:bool, "Yellow"=w4279:bool, "Green"=w4276:bool, "No recognizable coolour"=w4289:bool)
        n178 = Select(t=Box_Colour_FGV_Colours."Green" ("Colour"), s=w4276, f=Box_Colour_FGV_Colours."None" ("Colour")) -> (s? t:f=w4274:T2)
        n179 = Select(t=Box_Colour_FGV_Colours."Yellow" ("Colour"), s=w4279, f=w4274) -> (s? t:f=w4273:T2)
        n180 = Select(t=Box_Colour_FGV_Colours."Blue" ("Colour"), s=w4280, f=w4273) -> (s? t:f=w4282:T2)
        n181 = Select(t=Box_Colour_FGV_Colours."Black" ("Colour"), s=w4283, f=w4282) -> (s? t:f=w4285:T2)
        n182 = Select(t=Box_Colour_FGV_Colours."Red" ("Colour"), s=w4287, f=w4285) -> (s? t:f=w4272:T2)
        n183 = Bundle By Name(cluster=w4292, "Red"=w4287, "Black"=w4283, "Blue"=w4280, "Yellow"=w4279, "Green"=w4276, "Unknown"=w4289, "Image processing done"=w4288, "Colour"=w4272) -> (w4291:T1)
      }
      frame "-----ARM ACTIONS-----" {
      }
      frame "CLOSE CLAW" {
        n184 = call "Servo State FGV.vi"("Init/Read/Write State"=States_for_Action_Engine."Write", "Servo State"=Servo_States_FGV_Enum."Close claw") -> ()  [unwired: 1 in, 2 out]
      }
      frame "OPEN CLAW" {
        n185 = call "Servo State FGV.vi"("Init/Read/Write State"=States_for_Action_Engine."Write", "Servo State"=Servo_States_FGV_Enum."Open Claw") -> ()  [unwired: 1 in, 2 out]
      }
      frame "Z STEPPER CAM HEIGHT" {
        n186 = call "Arduino Interfacing VI.vi"("Data to Write"=I2C_MASTER_WRITE_NEW_Type_Def."zStepper 6k", "AE Mode"=Arduino_Interfacing."Write to Arduino") -> ()  [unwired: 2 in, 2 out]
      }
      frame "Z STEPPER GRAB HEIGHT" {
        # ">>State Logic  >>"
        # ">>> Time cluster >>>"
        # ">>> Yaw >>>"
        # ">>> Stepper position >>>"
        # ">>> Encoders >>>"
        # ">>> Object detection >>>"
        # ">>> Ultrasonic Sensors Detect >>>"
        n187 = call "Arduino Interfacing VI.vi"("Data to Write"=I2C_MASTER_WRITE_NEW_Type_Def."zStepper 100", "AE Mode"=Arduino_Interfacing."Write to Arduino") -> ()  [unwired: 2 in, 2 out]
      }
      frame "Z STEPPER BOX HEIGHT" {
        # ">>> IR Sensors >>>"
        # ">>> Time cluster >>>"
        # ">>> Yaw >>>"
        # ">>> Stepper position >>>"
        # ">>> Encoders >>>"
        # ">>> Object detection >>>"
        # ">>> Ultrasonic Sensors Detect >>>"
        n188 = call "Arduino Interfacing VI.vi"("Data to Write"=I2C_MASTER_WRITE_NEW_Type_Def."zStepper 4k", "AE Mode"=Arduino_Interfacing."Write to Arduino") -> ()  [unwired: 2 in, 2 out]
      }
      frame "Y STEPPER CONTROL" {
        # ">>State Logic  >>"
        # ">>> yStepper command>>>"
        # ">>> Time cluster >>>"
        # ">>> Yaw >>>"
        # ">>> Stepper position >>>"
        # ">>> Encoders >>>"
        # ">>> Object detection >>>"
        # ">>> Ultrasonic Sensors Detect >>>"
        n189 = Unbundle By Name(w4384) -> ("yStepper desired"=w4383:u8)
        n190 = call "Arduino Interfacing VI.vi"("y Stepper value"=w4383, "Data to Write"=I2C_MASTER_WRITE_NEW_Type_Def."yStepper control", "AE Mode"=Arduino_Interfacing."Write to Arduino") -> ()  [unwired: 1 in, 2 out]
      }
      frame "READ STEPPER VALUES" {
        # ">>State Logic  >>"
        # ">>> Time cluster >>>"
        # ">>> Yaw >>>"
        # ">>> Stepper position >>>"
        # ">>> Encoders >>>"
        # ">>> Object detection >>>"
        # ">>> Ultrasonic Sensors Detect >>>"
        n191 = call "Arduino Interfacing VI.vi"("AE Mode"=Arduino_Interfacing."Read From Arduino") -> ("Arduino Data"=w4402:T17)  [unwired: 3 in, 1 out]
        n192 = Unbundle By Name(w4402) -> ("y Stepper Position"=w4401:u8, "z Stepper Position"=w4400:u8)
        n193 = Bundle By Name(cluster=w4405, "y Stepper Position"=w4401, "z Stepper Position"=w4400) -> (w4404:T7)
      }
      frame " -----TIMING-----" {
        # ">>State Logic  >>"
        # ">>> Time cluster >>>"
        # ">>> Yaw >>>"
        # ">>> Stepper position >>>"
        # ">>> Encoders >>>"
        # ">>> Object detection >>>"
        # ">>> Ultrasonic Sensors Detect >>>"
      }
      frame "SET TIMER 1" {
        w4421 = 1.0 ("Time Setting")
        # ">>State Logic  >>"
        # ">>> Time cluster >>>"
        # ">>> Yaw >>>"
        # ">>> Stepper position >>>"
        # ">>> Encoders >>>"
        # ">>> Object detection >>>"
        # ">>> Ultrasonic Sensors Detect >>>"
        n194 = Wait (ms)(milliseconds to wait=u32 250) -> ()  [unwired: 1 out]
        n195 = call "Elasped Timer.vi"("Time Setting"=w4421, "Action"=Elapsed_timer_control."Initialize") -> ()  [unwired: 6 in, 4 out]
        n196 = Bundle By Name(cluster=w4430, "Time up flag"=FALSE, "SET TIME TO CHECK"=w4421) -> (w4428:T3)
      }
      frame "SET TIMER 2" {
        w4437 = 2.0 ("Time Setting")
        # ">>State Logic  >>"
        # ">>> Time cluster >>>"
        # ">>> Yaw >>>"
        # ">>> Stepper position >>>"
        # ">>> Encoders >>>"
        # ">>> Object detection >>>"
        # ">>> Ultrasonic Sensors Detect >>>"
        n197 = Wait (ms)(milliseconds to wait=u32 250) -> ()  [unwired: 1 out]
        n198 = call "Elasped Timer.vi"("Time Setting"=w4437, "Action"=Elapsed_timer_control."Initialize") -> ()  [unwired: 6 in, 4 out]
        n199 = Bundle By Name(cluster=w4446, "Time up flag"=FALSE, "SET TIME TO CHECK"=w4437) -> (w4444:T3)
      }
      frame "SET TIMER 3" {
        w4453 = 3.0 ("Time Setting")
        # ">>State Logic  >>"
        # ">>> Time cluster >>>"
        # ">>> Yaw >>>"
        # ">>> Stepper position >>>"
        # ">>> Encoders >>>"
        # ">>> Object detection >>>"
        # ">>> Ultrasonic Sensors Detect >>>"
        n200 = Wait (ms)(milliseconds to wait=u32 250) -> ()  [unwired: 1 out]
        n201 = call "Elasped Timer.vi"("Time Setting"=w4453, "Action"=Elapsed_timer_control."Initialize") -> ()  [unwired: 6 in, 4 out]
        n202 = Bundle By Name(cluster=w4462, "Time up flag"=FALSE, "SET TIME TO CHECK"=w4453) -> (w4460:T3)
      }
      frame "SET TIMER 4" {
        w4469 = 4.0 ("Time Setting")
        # ">>State Logic  >>"
        # ">>> Time cluster >>>"
        # ">>> Yaw >>>"
        # ">>> Stepper position >>>"
        # ">>> Encoders >>>"
        # ">>> Object detection >>>"
        # ">>> Ultrasonic Sensors Detect >>>"
        n203 = call "Elasped Timer.vi"("Time Setting"=w4469, "Action"=Elapsed_timer_control."Initialize") -> ()  [unwired: 6 in, 4 out]
        n204 = Wait (ms)(milliseconds to wait=u32 250) -> ()  [unwired: 1 out]
        n205 = Bundle By Name(cluster=w4478, "Time up flag"=FALSE, "SET TIME TO CHECK"=w4469) -> (w4476:T3)
      }
      frame "SET TIMER 5" {
        w4486 = 5.0 ("Time Setting")
        # ">>State Logic  >>"
        # ">>> Time cluster >>>"
        # ">>> Yaw >>>"
        # ">>> Stepper position >>>"
        # ">>> Encoders >>>"
        # ">>> Object detection >>>"
        # ">>> Ultrasonic Sensors Detect >>>"
        n206 = call "Elasped Timer.vi"("Time Setting"=w4486, "Action"=Elapsed_timer_control."Initialize") -> ("Time Out?!"=w4485:bool)  [unwired: 6 in, 3 out]
        n207 = Wait (ms)(milliseconds to wait=u32 250) -> ()  [unwired: 1 out]
        n208 = Bundle By Name(cluster=w4494, "Time up flag"=w4485, "SET TIME TO CHECK"=w4486) -> (w4493:T3)
      }
      frame "START TIMER" {
        # ">>State Logic  >>"
        # ">>> Time cluster >>>"
        # ">>> Yaw >>>"
        # ">>> Stepper position >>>"
        # ">>> Encoders >>>"
        # ">>> Object detection >>>"
        # ">>> Ultrasonic Sensors Detect >>>"
        n209 = call "Elasped Timer.vi"("Action"=Elapsed_timer_control."Start") -> ("Time Out?!"=w4505:bool)  [unwired: 7 in, 3 out]
        n210 = Bundle By Name(cluster=w4508, "Time up flag"=w4505) -> (w4507:T3)
      }
      frame "-----MISC-----" {
        # ">>> Box Colour Detection >>>"
        # ">>> Line Sensor Cluster>>>"
        # ">>> IR Sensors >>>"
        # ">>> Time cluster >>>"
        # ">>> Object detection >>>"
        # ">>> Yaw >>>"
        # ">>> Ultrasonic Sensors Detect >>>"
        # ">>> Encoders >>>"
        # ">>> Stepper position >>>"
      }
      frame "Task 9" {
        # ">>> Box Colour Detection >>>"
        # ">>> Line Sensor Cluster>>>"
        # ">>> IR Sensors >>>"
        # ">>> Time cluster >>>"
        # ">>> Object detection >>>"
        # ">>> Yaw >>>"
        # ">>> Ultrasonic Sensors Detect >>>"
        # ">>> Encoders >>>"
        # ">>> Stepper position >>>"
        n211 = call "Colour Processing Test Env.vi"() -> ("Colour scan time out?"=w4534:bool, "Colour output boolean cluster"=w4532:T47)  [unwired: 10 in]
        n212 = Unbundle By Name(w4532) -> ("Red"=w4526:bool, "Black"=w4527:bool, "Blue"=w4528:bool, "Yellow"=w4529:bool, "Green"=w4530:bool, "No recognizable coolour"=w4531:bool)
        n213 = Bundle By Name(cluster=w4536, "Red"=w4526, "Black"=w4527, "Blue"=w4528, "Yellow"=w4529, "Green"=w4530, "Unknown"=w4531, "Image processing done"=w4534) -> (w4535:T1)
      }
    }
    "State Logic" <- w263
    "Image Processing Error" <- w231
    n214 = call "Task Enable FGV.vi"("Init/Read/Write State"=States_for_Action_Engine."Read") -> ("Output node"=w219:bool)  [unwired: 9 in, 1 out]
    n215 = Not(x=w219) -> (.not. x?=w257:bool)
    n216 = case shown="True" w264 {
      tunnel: w222 -> [w295 w349]
      tunnel: w271 -> [w291 w351]
      tunnel: [w295 w349] -> w276
      tunnel: [w291 w352] -> w275
      tunnel: w272 -> [_ w347]
      tunnel: w274 -> [_ w348]
      tunnel: w269 -> [w294 w354]
      tunnel: [w294 w354] -> w268
      tunnel: "STOP TASK" -> [_ w337]
      tunnel: w263 -> [w293 w353]
      tunnel: [w293 w350] -> w262
      tunnel: w259 -> [w292 w343]
      tunnel: [w292 w343] -> w258
      tunnel: w257 -> [_ w338]
      tunnel: [w290 w335] -> w256
      tunnel: w255 -> [w290 w334]
      tunnel: w253 -> [w289 w331]
      tunnel: [w289 w331] -> w252
      tunnel: w250 -> [w288 w327]
      tunnel: [w288 w327] -> w249
      tunnel: w247 -> [w287 w325]
      tunnel: [w287 w325] -> w246
      tunnel: w244 -> [w286 w323]
      tunnel: [w286 w323] -> w243
      tunnel: w242 -> [w285 w322]
      tunnel: [w285 w321] -> w241
      tunnel: [_ w319] -> w240
      tunnel: w238 -> [w284 w317]
      tunnel: [w284 w317] -> w237
      tunnel: w236 -> [w283 w316]
      tunnel: [w283 w315] -> w235
      tunnel: w233 -> [w282 w312]
      tunnel: [w282 w312] -> w232
      tunnel: [w281 w311] -> w230
      tunnel: w228 -> [w281 w310]
      tunnel: [_ w308] -> w227
      tunnel: [_ w307] -> w226
      tunnel: [_ w306] -> w225
      tunnel: w223 -> [w280 w305]
      tunnel: [w280 w305] -> w221
      tunnel: [_ w296] -> w218
      frame False {
        # ">>> Box Colour Detection >>>"
        # ">>> Line Sensor Cluster>>>"
        # ">> Item Selection Bias >>"
        # ">>State Logic Queue Reference >>"
        # ">>Action states Queue Reference >>"
        # ">>True Stop Next State >>"
        # ">>State Logic  >>"
        # ">>> IR Sensors >>>"
        # ">>> Line Sensor Cluster>>>"
        # ">>> Line Sensor Cluster>>>"
        # ">>> Motor control cluster >>>"
        # ">>> yStepper command>>>"
        # ">>> Motor control cluster >>>"
        # ">>> yStepper command>>>"
        # ">>> Motor control cluster >>>"
        # ">>> IR Sensors >>>"
        # ">>> IR Sensors >>>"
        # ">>> yStepper command>>>"
        # ">>> Time cluster >>>"
        # ">>> Yaw >>>"
        # ">>> Stepper position >>>"
        # ">>> Encoders >>>"
        # ">>> Object detection >>>"
        # ">>> Ultrasonic Sensors Detect >>>"
        # ">>> Time cluster >>>"
        # ">>> Yaw >>>"
        # ">>> Stepper position >>>"
        # ">>> Encoders >>>"
        # ">>> Object detection >>>"
        # ">>> Ultrasonic Sensors Detect >>>"
      }
      frame True {
        # ">>> Box colour cluster >>>"
        # ">>State Logic Queue Reference >>"
        # ">>> Box Colour Detection >>>"
        # ">> Item Selection Bias >>"
        # ">>> IR Sensors >>>"
        # ">>> Line Sensor Cluster>>>"
        # ">>> Line Sensor Cluster>>>"
        # ">>> Motor control cluster >>>"
        # ">>> yStepper command>>>"
        # ">>> IR Sensors >>>"
        # ">>> Motor control cluster >>>"
        # ">>State Logic Queue Reference >>"
        # ">>Timeout>>"
        # ">>> yStepper command>>>"
        # ">>> Time cluster >>>"
        # ">>> Object detection >>>"
        # ">>> Yaw >>>"
        # ">>> Ultrasonic Sensors Detect >>>"
        # ">>> Encoders >>>"
        # ">>> Stepper position >>>"
        # ">>State Logic  >>"
        # ">>True Stop Next State >>"
        # ">>Action Queue>>"
        # ">> Manual override >>"
        # ">>> Time cluster >>>"
        # ">>> Yaw >>>"
        # ">>> Stepper position >>>"
        # ">>> Encoders >>>"
        # ">>> Object detection >>>"
        # ">>> Ultrasonic Sensors Detect >>>"
        # ">>Action Queue>>"
        # ">>State Logic Queue Reference >>"
        n217 = Or(x=w337, y=w338) -> (x .or. y?=w336:bool)
        n218 = Unbundle By Name(w305) -> ("Red"=w304:bool, "Black"=w303:bool, "Blue"=w302:bool, "Yellow"=w301:bool, "Green"=w300:bool, "Unknown"=w299:bool, "Image processing done"=w298:bool, "Colour"=w297:T2)
        n219 = Unbundle By Name(w312) -> ("Line Detected?"=w313:bool)
        n220 = Unbundle By Name(w317) -> ("Left IR Sensor"=w318:dbl, "Arm IR Sensor"=w314:dbl, "Bottom IR Sensor"=w309:dbl)
        n221 = Unbundle By Name(w323) -> ("Time up flag"=w324:bool)
        n222 = Unbundle By Name(w325) -> ("Yaw"=w326:dbl, "Compass"=w320:dbl)
        n223 = Unbundle By Name(w327) -> ("y Stepper Position"=w329:u8, "z Stepper Position"=w328:u8)
        n224 = Unbundle By Name(w343) -> ("xDistance"=w340:dbl, "yDistance"=w341:dbl, "wDistance"=w342:dbl)
        n225 = Unbundle By Name(w331) -> ("Recognized Object"=w330:bool, "Object X coordinate"=w333:dbl, "Object Y coordinate"=w332:dbl)
        n226 = Unbundle By Name(w354) -> ("PING_A"=w346:u8, "PING_B"=w345:u8, "PING_C"=w344:u8, "PING_D"=w339:u8)
        n227 = case shown="\"Task 9D2: ANGLE CORRECTION\"" w353 {
          tunnel: [w359 w371 w381 w389 w400 w510 w527 w573 w611 w665 w707 w756 w799 w854 w902 w946 w1006 w1047 w1090 w1139 w1179 w1232 w1270 w1322 w1368 w1414 w1455 w1504 w1548 w1594 w1635 w1684 w1728 w1774 w1815 w1864 w1908 w1954 w1995 w2044 w2079 w2097 w2145 w2186 w2236 w2293 w2332 w2381 w2424 w2477 w2515 w2567 w2610 w2655 w2690 w2738 w2781 w2835 w2883 w2926 w2979 w3020 w3076 w3117 w3169 w3217 w3266 w3309 w3353 w3401 w3452 w3495 w3554 w3591 w3595 w3599 w3603] -> w352
          tunnel: w351 -> [w359 w374 w381 w390 w403 w512 w528 w574 w620 w663 w711 w757 w805 w847 w905 w953 w996 w1050 w1096 w1138 w1182 w1222 w1276 w1312 w1363 w1406 w1454 w1503 w1547 w1586 w1634 w1683 w1727 w1766 w1814 w1863 w1907 w1946 w1994 w2043 w2079 w2087 w2148 w2192 w2235 w2292 w2338 w2380 w2427 w2467 w2521 w2557 w2603 w2648 w2694 w2745 w2786 w2840 w2890 w2932 w2977 w3021 w3074 w3118 w3170 w3219 w3273 w3315 w3360 w3406 w3451 w3491 w3552 w3591 w3595 w3599 w3603]
          tunnel: [State_Type_Definitions,_for_0.26g_versions_and_later_3."Idle" ("Enum") State_Type_Definitions,_for_0.26g_versions_and_later_3."Idle" ("Enum") _ w385 w402 State_Type_Definitions,_for_0.26g_versions_and_later_3."Shutdown" ("Enum") w529 w575 w618 w666 w708 w755 w800 w853 w903 w948 w1005 w1048 w1097 w1140 w1181 w1231 w1277 w1321 w1369 w1407 w1456 w1505 w1549 w1587 w1636 w1685 w1729 w1767 w1816 w1865 w1909 w1947 w1996 w2045 State_Type_Definitions,_for_0.26g_versions_and_later_3."Idle" ("Enum") w2096 w2146 w2193 w2237 w2294 w2339 w2382 w2426 w2476 w2522 w2566 w2609 w2654 w2691 w2739 w2782 w2836 w2884 w2925 w2980 w3019 w3077 w3116 w3168 w3218 w3267 w3308 w3355 w3407 w3453 w3494 w3555 _ _ _ _] -> w350
          tunnel: w349 -> [_ _ _ w388 w406 _ w533 w580 w614 w662 w712 w763 w804 w851 w906 w952 w1003 w1045 w1095 w1136 w1183 w1229 w1275 w1319 w1366 w1413 w1452 w1501 w1545 w1593 w1632 w1681 w1725 w1773 w1812 w1861 w1905 w1953 w1992 w2041 _ w2094 w2143 w2191 w2233 w2290 w2337 w2378 w2428 w2474 w2520 w2564 w2607 w2652 w2698 w2744 w2789 w2843 w2889 w2931 w2976 w3029 w3073 w3119 w3163 w3220 w3272 w3314 w3359 w3405 w3450 w3500 w3551 _ _ _ _]
          tunnel: w348 -> [_ _ _ _ w405 _ w532 w579 w613 w661 w713 w762 w803 w850 w899 w951 w1002 w1044 w1094 w1135 w1184 w1228 w1274 w1318 w1365 w1411 w1451 w1500 w1544 w1591 w1631 w1680 w1724 w1771 w1811 w1860 w1904 w1951 w1991 w2040 _ w2093 w2142 w2190 w2232 w2289 w2336 w2377 w2429 w2473 w2519 w2563 w2606 w2651 w2693 w2743 w2788 w2842 w2888 w2930 w2975 w3027 w3072 w3120 w3164 w3221 w3271 w3313 w3358 w3404 w3449 w3499 w3550 _ _ _ _]
          tunnel: w347 -> [_ _ _ w387 w401 _ w531 w578 w612 w660 w714 w761 w802 w849 w898 w950 w1004 w1046 w1093 w1134 w1185 w1230 w1273 w1320 w1364 w1412 w1450 w1499 w1543 w1592 w1630 w1679 w1723 w1772 w1810 w1859 w1903 w1952 w1990 w2039 _ w2095 w2144 w2189 w2231 w2288 w2335 w2376 w2430 w2475 w2518 w2565 w2608 w2653 w2697 w2742 w2787 w2841 w2887 w2929 w2974 w3028 w3071 w3121 w3165 w3222 w3270 w3312 w3357 w3403 w3448 w3498 w3549 _ _ _ _]
          tunnel: w336 -> [_ _ _ _ _ _ w518 w572 w619 w659 w715 w758 w798 w852 w904 w954 w997 w1051 w1091 w1137 w1186 w1223 w1271 w1313 w1367 w1409 w1453 w1502 w1546 w1589 w1633 w1682 w1726 w1769 w1813 w1862 w1906 w1949 w1993 w2042 _ w2088 w2149 w2187 w2234 w2291 w2333 w2379 w2431 w2468 w2516 w2558 w2604 w2649 w2696 w2737 w2785 w2839 w2882 w2928 w2973 w3023 w3070 w3122 w3166 w3223 w3265 w3311 w3356 w3402 w3447 w3497 w3548 _ _ _ _]
          tunnel: w346 -> [_ _ _ _ _ _ _ _ _ _ _ _ _ _ _ _ _ _ _ _ _ _ _ _ _ _ _ _ _ _ _ _ _ _ _ _ _ _ _ _ _ _ _ _ _ _ _ _ _ _ _ _ _ _ _ _ _ _ _ _ _ _ _ _ _ _ _ _ _ _ _ _ _ _ _ _ _]
          tunnel: w345 -> [_ _ _ _ _ _ _ _ _ w658 _ _ _ w843 w887 w944 _ _ _ _ _ _ _ _ _ _ _ _ _ _ _ _ _ _ _ _ _ _ _ _ _ _ w2135 _ _ _ _ _ _ _ _ _ _ _ _ _ _ _ _ _ _ _ _ _ _ _ _ _ _ _ _ _ _ _ _ _ _]
          tunnel: w344 -> [_ _ _ _ _ _ _ _ _ w657 _ _ _ w844 w888 w945 _ _ _ _ _ _ _ _ _ _ _ _ _ _ _ _ _ _ _ _ _ _ _ _ _ _ w2136 _ _ _ _ _ _ _ _ _ _ _ _ _ _ _ _ _ _ _ _ _ _ _ _ _ _ _ _ _ _ _ _ _ _]
          tunnel: w342 -> [_ _ _ _ _ _ _ _ _ _ _ w760 _ _ _ _ _ _ _ _ _ _ _ _ _ _ _ _ _ _ _ _ _ _ _ _ _ _ _ _ _ _ _ _ _ _ _ _ _ _ _ _ _ _ _ _ _ _ _ _ _ _ _ _ w3162 _ _ _ _ _ _ _ _ _ _ _ _]
          tunnel: w341 -> [_ _ _ _ _ _ w526 w571 _ _ w706 _ _ _ _ w949 _ _ _ _ _ _ _ _ _ _ _ _ _ _ _ _ _ _ _ w1852 _ _ _ w2032 _ _ _ _ _ _ _ _ _ _ _ _ _ _ _ _ _ w2826 _ _ _ _ _ _ _ _ _ _ _ _ _ _ _ _ _ _ _]
          tunnel: w340 -> [_ _ _ _ _ _ _ _ _ _ _ _ _ _ w893 _ _ _ _ _ _ _ _ _ _ _ _ w1492 _ _ _ w1672 _ _ _ _ _ _ _ _ _ _ _ _ _ w2279 _ _ _ _ _ _ _ w2641 _ _ _ _ _ _ _ _ w3063 _ _ _ _ _ _ _ _ _ w3541 _ _ _ _]
          tunnel: w339 -> [_ _ _ _ _ _ _ _ _ _ _ _ _ _ _ _ _ _ _ _ _ _ _ _ _ _ _ _ _ _ _ _ _ _ _ _ _ _ _ _ _ _ _ _ _ _ _ _ _ _ _ _ _ _ _ _ _ _ _ _ _ _ _ _ _ _ _ _ _ _ _ _ _ _ _ _ _]
          tunnel: [State_Type_Definitions,_for_0.26g_versions_and_later_3."Idle" ("Enum") State_Type_Definitions,_for_0.26g_versions_and_later_3."Idle" ("Enum") _ State_Type_Definitions,_for_0.26g_versions_and_later_3."Idle" ("Enum") State_Type_Definitions,_for_0.26g_versions_and_later_3."Idle" ("Enum") State_Type_Definitions,_for_0.26g_versions_and_later_3."Shutdown" ("Enum") w524 w569 w617 w664 w709 w752 w797 w846 w901 w947 w1007 w1049 w1089 w1141 w1180 w1233 w1269 w1323 w1370 w1408 w1457 w1506 w1550 w1588 w1637 w1686 w1730 w1768 w1817 w1866 w1910 w1948 w1997 w2046 w2081 w2098 w2147 w2185 w2238 w2295 w2331 w2383 w2425 w2478 w2514 w2568 w2611 w2656 w2692 w2740 w2784 w2838 w2885 w2924 w2978 w3018 w3075 w3115 w3167 w3216 w3268 w3307 w3354 w3408 w3454 w3493 w3553 _ _ _ _] -> w335
          tunnel: w334 -> [_ _ _ w385 _ _ _ _ _ _ _ _ _ _ _ _ _ _ _ _ _ _ _ _ _ _ _ _ _ _ _ _ _ _ _ _ _ _ _ _ w2081 _ _ _ _ _ _ _ _ _ _ _ _ _ _ _ _ _ _ _ _ _ _ _ _ _ _ _ _ _ _ _ _ _ _ _ _]
          tunnel: w330 -> [_ _ _ _ _ _ _ _ _ _ _ _ _ _ _ _ _ _ _ _ _ _ _ _ _ _ w1444 _ _ _ w1624 _ _ _ w1804 _ _ _ w1984 _ _ _ _ _ w2226 _ _ _ _ _ _ _ _ _ _ _ _ _ _ _ _ _ _ _ _ _ _ _ _ _ _ _ _ _ _ _ _]
          tunnel: w333 -> [_ _ _ _ _ _ _ _ _ _ _ _ _ _ _ _ _ _ _ _ _ _ _ _ _ _ _ _ _ _ _ _ _ _ _ _ _ _ _ _ _ _ _ _ _ w2285 _ _ _ _ _ _ _ _ _ _ _ _ _ _ _ _ _ _ _ _ _ _ _ _ _ _ _ _ _ _ _]
          tunnel: w332 -> [_ _ _ _ _ _ _ _ _ _ _ _ _ _ _ _ _ _ _ _ _ _ _ _ _ _ _ _ _ _ _ _ _ _ _ _ _ _ _ _ _ _ _ _ _ _ _ _ w2420 _ _ _ _ _ _ _ _ _ _ _ _ _ _ _ _ _ _ _ _ _ _ _ _ _ _ _ _]
          tunnel: w329 -> [_ _ _ _ _ _ _ _ _ _ _ _ _ _ _ _ _ _ _ _ _ _ _ _ _ _ _ _ _ _ _ _ _ _ _ _ _ _ _ _ _ _ _ _ _ _ _ _ w2419 _ _ _ _ _ _ _ _ _ _ _ _ _ _ _ _ _ _ _ _ _ _ _ _ _ _ _ _]
          tunnel: w328 -> [_ _ _ _ _ _ _ _ w616 _ _ _ w795 _ _ _ w1000 _ w1085 _ w1175 w1226 _ w1316 w1362 _ _ _ _ _ _ _ _ _ _ _ _ _ _ _ _ w2091 _ _ _ _ _ _ _ w2471 _ w2561 _ _ w2695 _ _ _ _ _ _ _ _ _ _ _ _ _ _ _ _ _ _ _ _ _ _]
          tunnel: w326 -> [_ _ _ _ _ _ _ _ _ _ _ _ _ _ _ _ _ _ _ _ _ _ _ _ _ _ _ _ _ _ _ _ _ _ _ _ _ _ _ _ _ _ _ _ _ _ _ _ _ _ _ _ _ _ _ _ _ _ _ _ _ _ _ _ _ _ _ _ _ _ _ _ _ _ _ _ _]
          tunnel: w324 -> [_ _ _ _ _ _ _ _ _ _ _ _ _ _ _ _ _ _ _ w1131 _ _ w1267 _ _ w1402 w1445 _ _ w1582 w1625 _ _ w1762 w1805 _ _ w1942 w1985 _ _ _ _ w2183 w2225 _ w2329 w2373 _ _ w2512 _ _ _ _ _ _ _ _ _ _ _ _ _ _ _ _ _ _ _ _ _ _ _ _ _ _]
          tunnel: w322 -> [w357 w369 w380 w384 w398 w508 w523 w568 w615 w656 w710 w751 w796 w845 w897 w943 w995 w1042 w1088 w1132 w1176 w1221 w1268 w1311 w1360 w1405 w1448 w1497 w1541 w1585 w1628 w1677 w1721 w1765 w1808 w1857 w1901 w1945 w1988 w2037 w2082 w2086 w2140 w2184 w2229 w2286 w2330 w2374 w2422 w2466 w2513 w2556 w2602 w2647 w2689 w2741 w2783 w2837 w2886 w2936 w2972 w3026 w3069 w3124 w3172 w3225 w3269 w3319 w3362 w3410 w3456 w3505 w3547 w3590 w3594 w3598 w3602]
          tunnel: [w357 w368 w380 w384 w398 w508 w523 w568 w615 w656 w710 w751 w796 w845 w897 w943 w995 w1042 w1088 w1132 w1176 w1221 w1268 w1311 w1360 w1405 w1448 w1497 w1541 w1585 w1628 w1677 w1721 w1765 w1808 w1857 w1901 w1945 w1988 w2037 w2082 w2086 w2140 w2184 w2229 w2286 w2330 w2374 w2421 w2466 w2513 w2556 w2602 w2647 w2689 w2741 w2783 w2837 w2886 w2936 w2972 w3026 w3069 w3124 w3172 w3225 w3269 w3319 w3362 w3410 w3456 w3505 w3547 w3590 w3594 w3598 w3602] -> w321
          tunnel: w320 -> [_ _ _ _ _ _ _ _ _ _ _ _ _ _ _ _ _ _ _ _ _ _ _ _ _ _ _ _ _ _ _ _ _ _ _ _ _ _ _ _ _ _ _ _ _ _ _ _ _ _ _ _ _ _ _ w2736 _ _ w2881 _ _ _ _ _ _ _ w3264 _ _ _ _ _ _ _ _ _ _]
          tunnel: [_ _ _ _ TRUE _ w517 w565 w608 w653 w702 w748 w791 _ _ _ _ _ _ _ _ _ _ _ w1356 _ w1445 _ _ _ w1625 _ _ _ w1805 _ _ _ w1985 _ _ _ _ _ w2225 w2275 _ _ _ _ _ _ _ _ w2686 w2731 w2778 w2827 w2876 _ w2969 w3013 w3062 w3110 w3160 w3207 w3259 _ _ _ w3446 w3490 w3540 _ _ _ _] -> w319
          tunnel: w318 -> [_ _ _ _ _ _ _ _ _ _ _ _ _ _ _ _ _ _ _ _ _ _ _ _ _ _ _ _ _ _ _ _ _ _ _ _ _ _ _ _ _ _ _ _ _ _ _ _ _ _ _ _ _ _ _ _ _ _ _ w2923 _ _ _ _ _ _ _ w3306 _ _ _ _ _ _ _ _ _]
          tunnel: w316 -> [w356 w366 w379 w383 w396 w507 w522 w567 w610 w655 w704 w750 w793 w838 w886 w942 w994 w1041 w1087 w1130 w1178 w1220 w1266 w1310 w1359 w1404 w1447 w1496 w1540 w1584 w1627 w1676 w1720 w1764 w1807 w1856 w1900 w1944 w1987 w2036 w2083 w2085 w2134 w2182 w2228 w2282 w2328 w2372 w2416 w2465 w2511 w2555 w2601 w2646 w2688 w2733 w2780 w2834 w2878 w2937 w2971 w3025 w3068 w3126 w3174 w3227 w3261 w3320 w3364 w3412 w3458 w3506 w3546 w3589 w3593 w3597 w3601]
          tunnel: [w356 w365 w379 w383 w396 w507 w522 w567 w610 w655 w704 w750 w793 w838 w886 w942 w994 w1041 w1087 w1130 w1178 w1220 w1266 w1310 w1359 w1404 w1447 w1496 w1540 w1584 w1627 w1676 w1720 w1764 w1807 w1856 w1900 w1944 w1987 w2036 w2083 w2085 w2134 w2182 w2228 w2281 w2328 w2372 w2416 w2465 w2511 w2555 w2601 w2646 w2688 w2733 w2780 w2834 w2878 w2937 w2971 w3025 w3068 w3126 w3174 w3227 w3261 w3320 w3364 w3412 w3458 w3506 w3546 w3589 w3593 w3597 w3601] -> w315
          tunnel: w314 -> [_ _ _ _ _ _ _ _ _ _ _ _ _ _ _ _ _ _ _ _ _ _ _ _ _ _ _ _ _ _ _ _ _ _ _ _ _ _ _ _ _ _ _ _ _ _ _ _ _ _ _ _ _ _ _ _ _ w2832 _ _ _ _ _ _ _ w3214 _ _ _ _ _ _ _ _ _ _ _]
          tunnel: w313 -> [_ _ _ _ _ _ w519 _ _ _ _ _ _ _ _ w940 _ _ _ _ _ _ _ _ _ _ _ _ _ _ _ _ _ _ _ _ _ _ _ _ _ _ _ _ _ _ _ _ _ _ _ _ _ _ _ _ w2778 _ _ _ w2969 _ w3064 _ _ _ _ _ w3352 _ w3446 _ w3542 _ _ _ _]
          tunnel: [w355 w361 w378 w382 w395 w506 w521 w566 w609 w654 w703 w749 w792 w837 w885 w941 w993 w1040 w1086 w1129 w1177 w1219 w1265 w1309 w1358 enum16{"Ball", "Soap", "Gel", "Pipe", "None"}."Ball" ("Object recognition mode") w1446 w1495 enum16{"Ball", "Soap", "Gel", "Pipe", "None"}."Soap" ("Object recognition mode") enum16{"Ball", "Soap", "Gel", "Pipe", "None"}."Soap" ("Object recognition mode") w1626 w1675 enum16{"Ball", "Soap", "Gel", "Pipe", "None"}."Gel" ("Object recognition mode") enum16{"Ball", "Soap", "Gel", "Pipe", "None"}."Gel" ("Object recognition mode") w1806 w1855 enum16{"Ball", "Soap", "Gel", "Pipe", "None"}."Pipe" ("Object recognition mode") enum16{"Ball", "Soap", "Gel", "Pipe", "None"}."Pipe" ("Object recognition mode") w1986 w2035 w2078 w2084 w2133 w2181 w2227 w2276 w2327 w2371 w2415 w2464 w2510 w2554 w2600 w2645 w2687 w2732 w2779 w2831 w2877 w2927 w2970 w3024 w3067 w3125 w3173 w3226 w3260 w3310 w3363 w3411 w3457 w3496 w3545 w3588 w3592 w3596 w3600] -> w311
          tunnel: w310 -> [w355 w361 w378 w382 _ w506 w521 w566 w609 w654 w703 w749 w792 w837 w885 w941 w993 w1040 w1086 w1129 w1177 w1219 w1265 w1309 w1358 _ w1446 w1495 _ _ w1626 w1675 _ _ w1806 w1855 _ _ w1986 w2035 w2078 w2084 w2133 w2181 w2227 w2276 w2327 w2371 w2415 w2464 w2510 w2554 w2600 w2645 w2687 w2732 w2779 w2831 w2877 w2927 w2970 w3024 w3067 w3125 w3173 w3226 w3260 w3310 w3363 w3411 w3457 w3496 w3545 w3588 w3592 w3596 w3600]
          tunnel: w309 -> [_ _ _ _ _ _ _ _ _ _ _ _ _ _ _ _ _ _ _ _ _ _ _ _ _ _ _ _ _ _ _ _ _ _ _ _ _ _ _ _ _ _ w2132 _ _ _ _ _ _ _ _ _ _ _ _ _ _ w2830 _ _ _ _ _ _ _ w3208 _ _ _ _ _ _ _ _ _ _ _]
          tunnel: [_ _ _ _ _ _ _ _ _ w653 _ _ _ _ _ _ _ _ _ _ _ _ _ _ _ _ _ _ _ _ _ _ _ _ _ _ _ _ _ _ _ _ _ _ _ _ _ _ _ _ _ _ _ _ _ _ _ w2827 _ _ _ _ _ _ _ _ _ _ _ _ _ _ _ _ _ _ _] -> w308
          tunnel: [_ _ _ _ _ _ _ _ _ _ _ _ _ _ _ _ _ _ _ _ _ _ _ _ _ _ _ _ _ _ _ _ _ _ _ _ _ _ _ _ _ _ _ _ _ _ _ _ _ _ _ _ _ _ _ _ _ w2824 _ _ _ _ _ _ _ w3206 _ _ _ _ _ _ _ _ _ _ _] -> w307
          tunnel: [_ _ _ _ _ _ _ _ _ _ _ _ _ _ _ _ _ _ _ _ _ _ _ _ _ _ _ _ _ _ _ _ _ _ _ _ _ _ _ _ _ _ _ _ _ _ _ _ _ _ _ _ _ _ _ _ _ w2828 _ _ _ _ _ _ _ w3206 _ _ _ _ _ _ _ _ _ _ _] -> w306
          tunnel: w304 -> [_ _ _ _ _ _ _ _ _ _ _ _ _ _ _ _ _ _ _ _ _ _ _ _ _ _ _ _ _ _ _ _ _ _ _ _ _ _ _ _ _ _ _ _ _ _ _ _ _ _ _ _ _ _ _ _ _ _ _ _ _ _ _ _ _ _ _ _ _ _ _ _ _ _ _ _ _]
          tunnel: w303 -> [_ _ _ _ _ _ _ _ _ _ _ _ _ _ _ _ _ _ _ _ _ _ _ _ _ _ _ _ _ _ _ _ _ _ _ _ _ _ _ _ _ _ _ _ _ _ _ _ _ _ _ _ _ _ _ _ _ _ _ _ _ _ _ _ _ _ _ _ _ _ _ _ _ _ _ _ _]
          tunnel: w302 -> [_ _ _ _ _ _ _ _ _ _ _ _ _ _ _ _ _ _ _ _ _ _ _ _ _ _ _ _ _ _ _ _ _ _ _ _ _ _ _ _ _ _ _ _ _ _ _ _ _ _ _ _ _ _ _ _ _ _ _ _ _ _ _ _ _ _ _ _ _ _ _ _ _ _ _ _ _]
          tunnel: w301 -> [_ _ _ _ _ _ _ _ _ _ _ _ _ _ _ _ _ _ _ _ _ _ _ _ _ _ _ _ _ _ _ _ _ _ _ _ _ _ _ _ _ _ _ _ _ _ _ _ _ _ _ _ _ _ _ _ _ _ _ _ _ _ _ _ _ _ _ _ _ _ _ _ _ _ _ _ _]
          tunnel: w300 -> [_ _ _ _ _ _ _ _ _ _ _ _ _ _ _ _ _ _ _ _ _ _ _ _ _ _ _ _ _ _ _ _ _ _ _ _ _ _ _ _ _ _ _ _ _ _ _ _ _ _ _ _ _ _ _ _ _ _ _ _ _ _ _ _ _ _ _ _ _ _ _ _ _ _ _ _ _]
          tunnel: w299 -> [_ _ _ _ _ _ _ _ _ _ _ _ _ _ _ _ _ _ _ _ _ _ _ _ _ _ _ _ _ _ _ _ _ _ _ _ _ _ _ _ _ _ _ _ _ _ _ _ _ _ _ _ _ _ _ _ _ _ _ _ _ _ _ _ _ _ _ _ _ _ _ _ _ _ _ _ _]
          tunnel: w298 -> [_ _ _ _ _ _ _ _ _ _ _ _ _ _ _ _ _ _ _ _ _ _ _ _ _ _ _ _ _ _ _ _ _ _ _ _ _ _ _ _ _ _ _ _ _ _ _ _ _ _ _ _ _ _ _ _ _ _ _ _ _ w3013 _ w3110 _ _ _ _ _ w3396 _ w3490 _ _ _ _ _]
          tunnel: w297 -> [_ _ _ _ _ _ _ _ _ _ _ _ _ _ _ _ _ _ _ _ _ _ _ _ _ _ _ _ _ _ _ _ _ _ _ _ _ _ _ _ _ _ _ _ _ _ _ _ _ _ _ _ _ _ _ _ _ _ _ _ _ w3016 _ w3112 _ _ _ _ _ w3398 _ w3492 _ _ _ _ _]
          tunnel: [_ _ _ _ _ _ _ _ _ _ _ _ _ _ _ _ _ _ _ _ _ _ _ _ _ _ _ _ _ _ _ _ _ _ _ _ _ _ _ _ _ _ _ _ _ _ _ _ _ _ _ _ _ _ _ _ _ _ _ _ _ w3014 _ w3111 _ _ _ _ _ _ _ _ _ _ _ _ _] -> w296
          frame "None" {
            # ">>> Motor control cluster >>>"
            # ">>> yStepper command>>>"
          }
          frame "Startup" {
            # ">>> yStepper command>>>"
            n228 = for {
              shift-right: [w377] -> w371
              shift-left: w374 -> [w376]
              tunnel: string[] ["INIT", "RESET ARM", "RESET FLAGS", "RESET YAW", "NAVX CALIBRATE"] -> [w375] mode=indexing
              n229 = Enqueue Element(queue=w376, element=w375) -> (queue out=w377:refnum<queue>)  [unwired: 2 in, 2 out]
            }
            n230 = Bundle By Name(cluster=w369, "yStepper desired"=u8 0) -> (w368:T21)
            n231 = Bundle By Name(cluster=w366, "ySpeed"=0.0, "xSpeed"=0.0, "wSpeed"=0.0) -> (w365:T20)
          }
          frame "Move to Angle" {
          }
          frame "True Stop" {
            # ">>Action Queue>>"
            # ">>> Motor control cluster >>>"
            # ">>> yStepper command>>>"
            n232 = Flush Queue(queue=w388, error in (no error)=w387) -> ()  [unwired: 3 out]
            n233 = for {
              shift-right: [w394] -> w389
              shift-left: w390 -> [w393]
              tunnel: string[] ["STOP", "RESET ENCODERS", "RESET YAW", "RESET ARM", "RESET ALL SENSORS", "RESET FLAGS", "DISPOSE CAM BUFFERS", "DISPOSE PROC BUFFERS", "CAM CLOSE"] -> [w392] mode=indexing
              n234 = Enqueue Element(queue=w393, element=w392) -> (queue out=w394:refnum<queue>)  [unwired: 2 in, 2 out]
            }
          }
          frame "Idle", Default {
            # ">>> Motor control cluster >>>"
            # ">>> yStepper command>>>"
            n235 = Dequeue Element(queue=w406, timeout in ms (-1)=w405, error in (no error)=w401) -> (element=w404:T10)  [unwired: 3 out]
            n236 = case shown="\"None\", Default" w404 {
              tunnel: [w409 w417 w425 w433 w441 w449 w457 w465 w473 w480 w490 w497 w500] -> w400
              tunnel: w403 -> [w410 w418 w426 w434 w442 w450 w458 w466 w474 w481 w489 w497 w501]
              tunnel: [State_Type_Definitions,_for_0.26g_versions_and_later_3."Task 1A" ("Enum") State_Type_Definitions,_for_0.26g_versions_and_later_3."Task 2:Raise Arm" ("Enum") State_Type_Definitions,_for_0.26g_versions_and_later_3."Task 3: Rotate 360" ("Enum") State_Type_Definitions,_for_0.26g_versions_and_later_3."Task 4_A" ("Enum") State_Type_Definitions,_for_0.26g_versions_and_later_3."Task 5A: RAISING ARM" ("Enum") State_Type_Definitions,_for_0.26g_versions_and_later_3."Task 6A: RAISE ARM" ("Enum") State_Type_Definitions,_for_0.26g_versions_and_later_3."Task 8A: RAISE ARM" ("Enum") State_Type_Definitions,_for_0.26g_versions_and_later_3."Task 8A: RAISE ARM" ("Enum") State_Type_Definitions,_for_0.26g_versions_and_later_3."Task 8A: RAISE ARM" ("Enum") State_Type_Definitions,_for_0.26g_versions_and_later_3."Task 8A: RAISE ARM" ("Enum") State_Type_Definitions,_for_0.26g_versions_and_later_3."Task 9A: Raise Arm" ("Enum") State_Type_Definitions,_for_0.26g_versions_and_later_3."Idle" ("Enum") State_Type_Definitions,_for_0.26g_versions_and_later_3."Shutdown" ("Enum")] -> w402
              tunnel: [enum16{"Ball", "Soap", "Gel", "Pipe", "None"}."None" ("Object recognition mode") enum16{"Ball", "Soap", "Gel", "Pipe", "None"}."None" ("Object recognition mode") enum16{"Ball", "Soap", "Gel", "Pipe", "None"}."None" ("Object recognition mode") enum16{"Ball", "Soap", "Gel", "Pipe", "None"}."None" ("Object recognition mode") enum16{"Ball", "Soap", "Gel", "Pipe", "None"}."None" ("Object recognition mode") enum16{"Ball", "Soap", "Gel", "Pipe", "None"}."None" ("Object recognition mode") enum16{"Ball", "Soap", "Gel", "Pipe", "None"}."Ball" ("Object recognition mode") enum16{"Ball", "Soap", "Gel", "Pipe", "None"}."Gel" ("Object recognition mode") enum16{"Ball", "Soap", "Gel", "Pipe", "None"}."Pipe" ("Object recognition mode") enum16{"Ball", "Soap", "Gel", "Pipe", "None"}."Soap" ("Object recognition mode") enum16{"Ball", "Soap", "Gel", "Pipe", "None"}."None" ("Object recognition mode") enum16{"Ball", "Soap", "Gel", "Pipe", "None"}."None" ("Object recognition mode") enum16{"Ball", "Soap", "Gel", "Pipe", "None"}."None" ("Object recognition mode")] -> w395
              frame "Start Task 1" {
                n237 = for {
                  shift-right: [w414] -> w409
                  shift-left: w410 -> [w413]
                  tunnel: string[] ["RESET ENCODERS", "RESET YAW", "FORWARD", "READ ENCODERS"] -> [w412] mode=indexing
                  n238 = Enqueue Element(queue=w413, element=w412) -> (queue out=w414:refnum<queue>)  [unwired: 2 in, 2 out]
                }
              }
              frame "Start Task 2" {
                n239 = for {
                  shift-right: [w422] -> w417
                  shift-left: w418 -> [w421]
                  tunnel: string[] ["RESET ENCODERS", "RESET YAW", "READ ULTRASONIC", "ARDUINO - ULTRASONIC"] -> [w420] mode=indexing
                  n240 = Enqueue Element(queue=w421, element=w420) -> (queue out=w422:refnum<queue>)  [unwired: 2 in, 2 out]
                }
              }
              frame "Start Task 3" {
                n241 = for {
                  shift-right: [w430] -> w425
                  shift-left: w426 -> [w429]
                  tunnel: string[] ["RESET ENCODERS", "READ ENCODERS", "R-ACW"] -> [w428] mode=indexing
                  n242 = Enqueue Element(queue=w429, element=w428) -> (queue out=w430:refnum<queue>)  [unwired: 2 in, 2 out]
                }
              }
              frame "Start Task 4" {
                n243 = for {
                  shift-right: [w438] -> w433
                  shift-left: w434 -> [w437]
                  tunnel: string[] ["RESET YAW", "RESET ENCODERS", "RESET ARM", "RESET FLAGS", "", ""] -> [w436] mode=indexing
                  n244 = Enqueue Element(queue=w437, element=w436) -> (queue out=w438:refnum<queue>)  [unwired: 2 in, 2 out]
                }
              }
              frame "Start Task 5" {
                n245 = for {
                  shift-right: [w446] -> w441
                  shift-left: w442 -> [w445]
                  tunnel: string[] ["RESET YAW", "RESET ENCODERS", "RESET ARM", "RESET ALL SENSORS", "", ""] -> [w444] mode=indexing
                  n246 = Enqueue Element(queue=w445, element=w444) -> (queue out=w446:refnum<queue>)  [unwired: 2 in, 2 out]
                }
              }
              frame "Start Task 6" {
                n247 = for {
                  shift-right: [w454] -> w449
                  shift-left: w450 -> [w453]
                  tunnel: string[] ["OPEN LOG CAM ", "", "", "", "", ""] -> [w452] mode=indexing
                  n248 = Enqueue Element(queue=w453, element=w452) -> (queue out=w454:refnum<queue>)  [unwired: 2 in, 2 out]
                }
              }
              frame "Start Task 8 - BALL" {
                n249 = for {
                  shift-right: [w462] -> w457
                  shift-left: w458 -> [w461]
                  tunnel: string[] ["RESET YAW", "RESET ENCODERS", "RESET ARM", "RESET FLAGS"] -> [w460] mode=indexing
                  n250 = Enqueue Element(queue=w461, element=w460) -> (queue out=w462:refnum<queue>)  [unwired: 2 in, 2 out]
                }
              }
              frame "Start Task 8 - Gel" {
                n251 = for {
                  shift-right: [w470] -> w465
                  shift-left: w466 -> [w469]
                  tunnel: string[] ["RESET YAW", "RESET ENCODERS", "RESET ARM", "RESET FLAGS"] -> [w468] mode=indexing
                  n252 = Enqueue Element(queue=w469, element=w468) -> (queue out=w470:refnum<queue>)  [unwired: 2 in, 2 out]
                }
              }
              frame "Start Task 8 - Pipe" {
                n253 = for {
                  shift-right: [w478] -> w473
                  shift-left: w474 -> [w477]
                  tunnel: string[] ["RESET YAW", "RESET ENCODERS", "RESET ARM", "RESET FLAGS"] -> [w476] mode=indexing
                  n254 = Enqueue Element(queue=w477, element=w476) -> (queue out=w478:refnum<queue>)  [unwired: 2 in, 2 out]
                }
              }
              frame "Start Task 8 - Soap" {
                n255 = for {
                  shift-right: [w486] -> w480
                  shift-left: w481 -> [w485]
                  tunnel: string[] ["RESET YAW", "RESET ENCODERS", "RESET ARM", "RESET FLAGS"] -> [w484] mode=indexing
                  n256 = Enqueue Element(queue=w485, element=w484) -> (queue out=w486:refnum<queue>)  [unwired: 2 in, 2 out]
                }
              }
              frame "Start Task 9" {
                n257 = for {
                  shift-right: [w494] -> w490
                  shift-left: w489 -> [w493]
                  tunnel: string[] ["Z STEPPER BOX HEIGHT", "READ STEPPER VALUES", "", ""] -> [w492] mode=indexing
                  n258 = Enqueue Element(queue=w493, element=w492) -> (queue out=w494:refnum<queue>)  [unwired: 2 in, 2 out]
                }
              }
              frame "None", Default {
              }
              frame "Exit" {
                n259 = for {
                  shift-right: [w505] -> w500
                  shift-left: w501 -> [w504]
                  tunnel: string[] ["STOP", "RESET ENCODERS", "RESET YAW", "EXIT"] -> [w503] mode=indexing
                  n260 = Enqueue Element(queue=w504, element=w503) -> (queue out=w505:refnum<queue>)  [unwired: 2 in, 2 out]
                }
              }
            }
          }
          frame "Shutdown" {
            # ">> Item Selection Bias >>"
            # ">>> yStepper command>>>"
            n261 = for {
              shift-right: [w516] -> w510
              shift-left: w512 -> [w515]
              tunnel: string[] ["INIT", "RESET ENCODERS", "RESET FLAGS", "CAM CLOSE", "DISPOSE BUFFERS", "EXIT", ""] -> [w514] mode=indexing
              n262 = Enqueue Element(queue=w515, element=w514) -> (queue out=w516:refnum<queue>)  [unwired: 2 in, 2 out]
            }
          }
          frame "Task 1A" {
            # ">>> Motor control cluster >>>"
            # ">> Line detection >>"
            # ">> Checks if 1 metre moved >>"
            # ">>> yStepper command>>>"
            # "Use 250"
            n263 = Greater?(x=w526, y=265.0) -> (0:w520:bool)
            n264 = Dequeue Element(queue=w533, timeout in ms (-1)=w532, error in (no error)=w531) -> (element=w530:T10)  [unwired: 3 out]
            n265 = And(x=w519, y=w520) -> (x .and. y?=w517:bool)
            n266 = case shown="\"Start Task 1\", Default" w530 {
              tunnel: w518 -> [w534 _]
              tunnel: [w544 State_Type_Definitions,_for_0.26g_versions_and_later_3."True Stop" ("Enum")] -> w529
              tunnel: w528 -> [w542 w559]
              tunnel: [w541 w558] -> w527
              tunnel: [State_Type_Definitions,_for_0.26g_versions_and_later_3."Idle" ("Enum") State_Type_Definitions,_for_0.26g_versions_and_later_3."Shutdown" ("Enum")] -> w524
              tunnel: w517 -> [w535 _]
              frame "Start Task 1", Default {
                n267 = Or(x=w535, y=w534) -> (x .or. y?=w536:bool)
                n268 = case shown="True" w536 {
                  tunnel: w542 -> [w547 w553]
                  tunnel: [w546 w551] -> w541
                  frame False {
                    n269 = for {
                      shift-right: [w549] -> w546
                      shift-left: w547 -> [w550]
                      tunnel: string[] ["READ ENCODERS", "READ NAVX", "FORWARD", "READ LINE SENSOR"] ("element") -> [w548] mode=indexing
                      n270 = Enqueue Element(queue=w550, element=w548) -> (queue out=w549:refnum<queue>)  [unwired: 2 in, 2 out]
                    }
                  }
                  frame True {
                    n271 = for {
                      shift-right: [w555] -> w551
                      shift-left: w553 -> [w556]
                      tunnel: string[] ["RESET YAW", "RESET ENCODERS", "STOP", ""] -> [w554] mode=indexing
                      n272 = Enqueue Element(queue=w556, element=w554) -> (queue out=w555:refnum<queue>)  [unwired: 2 in, 2 out]
                    }
                  }
                }
                n273 = Select(t=State_Type_Definitions,_for_0.26g_versions_and_later_3."True Stop" ("Enum"), s=w534, f=State_Type_Definitions,_for_0.26g_versions_and_later_3."Task 1B" ("Enum")) -> (s? t:f=w539:T18)
                n274 = Select(t=w539, s=w535, f=State_Type_Definitions,_for_0.26g_versions_and_later_3."Task 1A" ("Enum")) -> (s? t:f=w544:T18)
              }
              frame "Exit" {
                n275 = for {
                  shift-right: [w563] -> w558
                  shift-left: w559 -> [w564]
                  tunnel: string[] ["STOP", "RESET ENCODERS", "RESET YAW", ""] -> [w562] mode=indexing
                  n276 = Enqueue Element(queue=w564, element=w562) -> (queue out=w563:refnum<queue>)  [unwired: 2 in, 2 out]
                }
              }
            }
          }
          frame "Task 1B" {
            # ">>> Motor control cluster >>>"
            # ">> Line detection >>"
            # ">> Adds small distance overhead after 1M >>"
            # ">>> yStepper command>>>"
            n277 = Greater?(x=w571, y=50.0) -> (0:w565:bool)
            n278 = Dequeue Element(queue=w580, timeout in ms (-1)=w579, error in (no error)=w578) -> (element=w577:T10)  [unwired: 3 out]
            n279 = Or(x=w565, y=w572) -> (x .or. y?=w576:bool)
            n280 = case shown="\"Start Task 1\", Default" w577 {
              tunnel: w576 -> [w583 _]
              tunnel: [w587 State_Type_Definitions,_for_0.26g_versions_and_later_3."True Stop" ("Enum")] -> w575
              tunnel: w574 -> [w584 w602]
              tunnel: [w582 w601] -> w573
              tunnel: [State_Type_Definitions,_for_0.26g_versions_and_later_3."Idle" ("Enum") State_Type_Definitions,_for_0.26g_versions_and_later_3."Shutdown" ("Enum")] -> w569
              frame "Start Task 1", Default {
                n281 = case shown="True" w583 {
                  tunnel: w584 -> [w590 w596]
                  tunnel: [w589 w594] -> w582
                  frame False {
                    n282 = for {
                      shift-right: [w592] -> w589
                      shift-left: w590 -> [w593]
                      tunnel: string[] ["READ ENCODERS", "READ NAVX", "FORWARD", "READ LINE SENSOR"] ("element") -> [w591] mode=indexing
                      n283 = Enqueue Element(queue=w593, element=w591) -> (queue out=w592:refnum<queue>)  [unwired: 2 in, 2 out]
                    }
                  }
                  frame True {
                    n284 = for {
                      shift-right: [w598] -> w594
                      shift-left: w596 -> [w599]
                      tunnel: string[] ["RESET YAW", "RESET ENCODERS", "STOP", ""] -> [w597] mode=indexing
                      n285 = Enqueue Element(queue=w599, element=w597) -> (queue out=w598:refnum<queue>)  [unwired: 2 in, 2 out]
                    }
                  }
                }
                n286 = Select(t=State_Type_Definitions,_for_0.26g_versions_and_later_3."True Stop" ("Enum"), s=w583, f=State_Type_Definitions,_for_0.26g_versions_and_later_3."Task 1B" ("Enum")) -> (s? t:f=w587:T18)
              }
              frame "Exit" {
                n287 = for {
                  shift-right: [w606] -> w601
                  shift-left: w602 -> [w607]
                  tunnel: string[] ["STOP", "RESET ENCODERS", "RESET YAW", ""] -> [w605] mode=indexing
                  n288 = Enqueue Element(queue=w607, element=w605) -> (queue out=w606:refnum<queue>)  [unwired: 2 in, 2 out]
                }
              }
            }
          }
          frame "Task 2:Raise Arm" {
            # ">>> Motor control cluster >>>"
            # ">> Stepper height reeached >>"
            # ">>> yStepper command>>>"
            # ">> Manual override >>"
            n289 = Dequeue Element(queue=w614, timeout in ms (-1)=w613, error in (no error)=w612) -> (element=w622:T10)  [unwired: 3 out]
            n290 = Equal?(x=w616, y=u8 60) -> (x = y?=w608:bool)
            n291 = case shown="\"Start Task 1\", Default" w622 {
              tunnel: [w633 State_Type_Definitions,_for_0.26g_versions_and_later_3."True Stop" ("Enum")] -> w618
              tunnel: [w631 w648] -> w611
              tunnel: w620 -> [w630 _]
              tunnel: w619 -> [w624 _]
              tunnel: [State_Type_Definitions,_for_0.26g_versions_and_later_3."Idle" ("Enum") State_Type_Definitions,_for_0.26g_versions_and_later_3."Shutdown" ("Enum")] -> w617
              tunnel: w608 -> [w623 _]
              frame "Start Task 1", Default {
                # ">> WIill proceed to part ii if not manual override >>"
                # ">>If ENABLE or Trigger is set to true>>"
                n292 = Or(x=w623, y=w624) -> (x .or. y?=w625:bool)
                n293 = case shown="True" w623 {
                  tunnel: [w636 w642] -> w631
                  tunnel: w630 -> [w635 w641]
                  frame False {
                    n294 = for {
                      shift-right: [w638] -> w636
                      shift-left: w635 -> [w639]
                      tunnel: string[] ["Z STEPPER CAM HEIGHT", "READ STEPPER VALUES"] ("element") -> [w637] mode=indexing
                      n295 = Enqueue Element(queue=w639, element=w637) -> (queue out=w638:refnum<queue>)  [unwired: 2 in, 2 out]
                    }
                  }
                  frame True {
                    n296 = for {
                      shift-right: [w644] -> w642
                      shift-left: w641 -> [w645]
                      tunnel: string[] ["ARDUINO - ULTRASONIC", "READ ULTRASONIC", "", "", "", ""] -> [w643] mode=indexing
                      n297 = Enqueue Element(queue=w645, element=w643) -> (queue out=w644:refnum<queue>)  [unwired: 2 in, 2 out]
                    }
                  }
                }
                n298 = Select(t=State_Type_Definitions,_for_0.26g_versions_and_later_3."True Stop" ("Enum"), s=w624, f=State_Type_Definitions,_for_0.26g_versions_and_later_3."Task 2:Sensor Mode" ("Enum")) -> (s? t:f=w627:T18)
                n299 = Select(t=w627, s=w625, f=State_Type_Definitions,_for_0.26g_versions_and_later_3."Task 2:Raise Arm" ("Enum")) -> (s? t:f=w633:T18)
              }
              frame "Exit" {
                n300 = for {
                  shift-right: [w651] -> w648
                  shift-left: _ -> [w652]
                  tunnel: string[] ["STOP", "RESET ENCODERS", "RESET YAW", ""] -> [w650] mode=indexing
                  n301 = Enqueue Element(queue=w652, element=w650) -> (queue out=w651:refnum<queue>)  [unwired: 2 in, 2 out]
                }
              }
            }
          }
          frame "Task 2:Sensor Mode" {
            w669 = u8 20 ("y")
            # ">>> Motor control cluster >>>"
            # ">>> yStepper command>>>"
            # ">>Object detected>>"
            n302 = Dequeue Element(queue=w662, timeout in ms (-1)=w661, error in (no error)=w660) -> (element=w670:T10)  [unwired: 3 out]
            n303 = Less?(x=w658, y=w669) -> (x < y?=w668:bool)
            n304 = Less?(x=w657, y=w669) -> (x < y?=w667:bool)
            n305 = Or(x=w668, y=w667) -> (x .or. y?=w653:bool)
            n306 = case shown="\"Start Task 1\", Default" w670 {
              tunnel: w653 -> [w673 _]
              tunnel: [w680 State_Type_Definitions,_for_0.26g_versions_and_later_3."True Stop" ("Enum")] -> w666
              tunnel: w659 -> [w672 _]
              tunnel: w663 -> [w679 w696]
              tunnel: [w678 w697] -> w665
              tunnel: [State_Type_Definitions,_for_0.26g_versions_and_later_3."Idle" ("Enum") State_Type_Definitions,_for_0.26g_versions_and_later_3."Shutdown" ("Enum")] -> w664
              frame "Start Task 1", Default {
                n307 = case shown="True" w673 {
                  tunnel: w679 -> [w683 w690]
                  tunnel: [w684 w689] -> w678
                  frame False {
                    n308 = for {
                      tunnel: string[] ["READ ULTRASONIC", "STOP"] ("element") -> [w685] mode=indexing
                      shift-right: [w687] -> w684
                      shift-left: w683 -> [w686]
                      n309 = Enqueue Element(queue=w686, element=w685) -> (queue out=w687:refnum<queue>)  [unwired: 2 in, 2 out]
                    }
                  }
                  frame True {
                    n310 = for {
                      shift-right: [w692] -> w689
                      shift-left: w690 -> [w693]
                      tunnel: string[] ["RESET ENCODERS", "READ NAVX", "READ ENCODERS"] -> [w691] mode=indexing
                      n311 = Enqueue Element(queue=w693, element=w691) -> (queue out=w692:refnum<queue>)  [unwired: 2 in, 2 out]
                    }
                  }
                }
                n312 = Or(x=w673, y=w672) -> (x .or. y?=w671:bool)
                n313 = Select(t=State_Type_Definitions,_for_0.26g_versions_and_later_3."True Stop" ("Enum"), s=w672, f=State_Type_Definitions,_for_0.26g_versions_and_later_3."Task 2:Reverse Mode" ("Enum")) -> (s? t:f=w674:T18)
                n314 = Select(t=w674, s=w671, f=State_Type_Definitions,_for_0.26g_versions_and_later_3."Task 2:Sensor Mode" ("Enum")) -> (s? t:f=w680:T18)
              }
              frame "Exit" {
                n315 = for {
                  shift-right: [w700] -> w697
                  shift-left: w696 -> [w701]
                  tunnel: string[] ["STOP", "RESET ENCODERS", "RESET YAW", "ARDUINO MODE 0"] -> [w699] mode=indexing
                  n316 = Enqueue Element(queue=w701, element=w699) -> (queue out=w700:refnum<queue>)  [unwired: 2 in, 2 out]
                }
              }
            }
          }
          frame "Task 2:Reverse Mode" {
            # ">>> yStepper command>>>"
            n317 = Dequeue Element(queue=w712, timeout in ms (-1)=w713, error in (no error)=w714) -> (element=w716:T10)  [unwired: 3 out]
            n318 = Less?(x=w706, y=-30.0) -> (x < y?=w702:bool)
            n319 = case shown="\"Start Task 1\", Default" w716 {
              tunnel: [w726 State_Type_Definitions,_for_0.26g_versions_and_later_3."True Stop" ("Enum")] -> w708
              tunnel: w715 -> [w719 _]
              tunnel: w711 -> [w725 w742]
              tunnel: [w724 w743] -> w707
              tunnel: [State_Type_Definitions,_for_0.26g_versions_and_later_3."Idle" ("Enum") State_Type_Definitions,_for_0.26g_versions_and_later_3."Shutdown" ("Enum")] -> w709
              tunnel: w702 -> [w717 _]
              frame "Start Task 1", Default {
                n320 = case shown="True" w717 {
                  tunnel: w725 -> [w729 w736]
                  tunnel: [w730 w735] -> w724
                  frame False {
                    n321 = for {
                      tunnel: string[] ["READ ENCODERS", "REVERSE", "READ NAVX"] ("element") -> [w731] mode=indexing
                      shift-right: [w733] -> w730
                      shift-left: w729 -> [w732]
                      n322 = Enqueue Element(queue=w732, element=w731) -> (queue out=w733:refnum<queue>)  [unwired: 2 in, 2 out]
                    }
                  }
                  frame True {
                    n323 = for {
                      shift-right: [w738] -> w735
                      shift-left: w736 -> [w739]
                      tunnel: string[] ["STOP", "ARDUINO - ULTRASONIC", "READ ULTRASONIC", "RESET ENCODERS"] -> [w737] mode=indexing
                      n324 = Enqueue Element(queue=w739, element=w737) -> (queue out=w738:refnum<queue>)  [unwired: 2 in, 2 out]
                    }
                  }
                }
                n325 = Or(x=w717, y=w719) -> (x .or. y?=w718:bool)
                n326 = Select(t=State_Type_Definitions,_for_0.26g_versions_and_later_3."True Stop" ("Enum"), s=w719, f=State_Type_Definitions,_for_0.26g_versions_and_later_3."Task 2:Sensor Mode" ("Enum")) -> (s? t:f=w720:T18)
                n327 = Select(t=w720, s=w718, f=State_Type_Definitions,_for_0.26g_versions_and_later_3."Task 2:Reverse Mode" ("Enum")) -> (s? t:f=w726:T18)
              }
              frame "Exit" {
                n328 = for {
                  shift-right: [w746] -> w743
                  shift-left: w742 -> [w747]
                  tunnel: string[] ["STOP", "RESET ENCODERS", "RESET YAW", "ARDUINO MODE 0"] -> [w745] mode=indexing
                  n329 = Enqueue Element(queue=w747, element=w745) -> (queue out=w746:refnum<queue>)  [unwired: 2 in, 2 out]
                }
              }
            }
          }
          frame "Task 3: Rotate 360" {
            # ">>> Motor control cluster >>>"
            # ">>> yStepper command>>>"
            n330 = Dequeue Element(queue=w763, timeout in ms (-1)=w762, error in (no error)=w761) -> (element=w753:T10)  [unwired: 3 out]
            n331 = Less?(x=w760, y=-160.0) -> (x < y?=w748:bool)
            n332 = Or(x=w748, y=w758) -> (x .or. y?=w754:bool)
            n333 = case shown="\"Start Task 1\", Default" w753 {
              tunnel: w754 -> [w766 _]
              tunnel: [w770 State_Type_Definitions,_for_0.26g_versions_and_later_3."True Stop" ("Enum")] -> w755
              tunnel: w757 -> [w767 w786]
              tunnel: [w765 w785] -> w756
              tunnel: [State_Type_Definitions,_for_0.26g_versions_and_later_3."Idle" ("Enum") State_Type_Definitions,_for_0.26g_versions_and_later_3."Shutdown" ("Enum")] -> w752
              frame "Start Task 1", Default {
                n334 = case shown="False" w766 {
                  tunnel: w767 -> [w773 w779]
                  tunnel: [w772 w777] -> w765
                  frame False {
                    n335 = for {
                      shift-right: [w775] -> w772
                      shift-left: w773 -> [w776]
                      tunnel: string[] ["READ ENCODERS", "R-CW"] ("element") -> [w774] mode=indexing
                      n336 = Enqueue Element(queue=w776, element=w774) -> (queue out=w775:refnum<queue>)  [unwired: 2 in, 2 out]
                    }
                  }
                  frame True {
                    n337 = for {
                      shift-right: [w781] -> w777
                      shift-left: w779 -> [w782]
                      tunnel: string[] ["RESET YAW", "RESET ENCODERS", "STOP", "ARDUINO MODE 0"] -> [w780] mode=indexing
                      n338 = Enqueue Element(queue=w782, element=w780) -> (queue out=w781:refnum<queue>)  [unwired: 2 in, 2 out]
                    }
                  }
                }
                n339 = Select(t=State_Type_Definitions,_for_0.26g_versions_and_later_3."True Stop" ("Enum"), s=w766, f=State_Type_Definitions,_for_0.26g_versions_and_later_3."Task 3: Rotate 360" ("Enum")) -> (s? t:f=w770:T18)
              }
              frame "Exit" {
                n340 = for {
                  shift-right: [w789] -> w785
                  shift-left: w786 -> [w790]
                  tunnel: string[] ["STOP", "RESET ENCODERS", "RESET YAW", ""] -> [w788] mode=indexing
                  n341 = Enqueue Element(queue=w790, element=w788) -> (queue out=w789:refnum<queue>)  [unwired: 2 in, 2 out]
                }
              }
            }
          }
          frame "Task 4_A" {
            # ">> Stepper height reeached >>"
            # ">>> yStepper command>>>"
            # ">> Manual override >>"
            n342 = Dequeue Element(queue=w804, timeout in ms (-1)=w803, error in (no error)=w802) -> (element=w801:T10)  [unwired: 3 out]
            n343 = Equal?(x=w795, y=u8 60) -> (x = y?=w791:bool)
            n344 = case shown="\"Start Task 1\", Default" w801 {
              tunnel: [w816 State_Type_Definitions,_for_0.26g_versions_and_later_3."True Stop" ("Enum")] -> w800
              tunnel: [w814 w832] -> w799
              tunnel: w805 -> [w813 w829]
              tunnel: w798 -> [w807 _]
              tunnel: [State_Type_Definitions,_for_0.26g_versions_and_later_3."Idle" ("Enum") State_Type_Definitions,_for_0.26g_versions_and_later_3."Shutdown" ("Enum")] -> w797
              tunnel: w791 -> [w806 _]
              frame "Start Task 1", Default {
                # ">> WIill proceed to part ii if not manual override >>"
                # ">>If ENABLE or Trigger is set to true>>"
                n345 = Or(x=w806, y=w807) -> (x .or. y?=w808:bool)
                n346 = case shown="False" w806 {
                  tunnel: [w819 w825] -> w814
                  tunnel: w813 -> [w818 w824]
                  frame False {
                    n347 = for {
                      shift-right: [w821] -> w819
                      shift-left: w818 -> [w822]
                      tunnel: string[] ["Z STEPPER CAM HEIGHT", "READ STEPPER VALUES"] ("element") -> [w820] mode=indexing
                      n348 = Enqueue Element(queue=w822, element=w820) -> (queue out=w821:refnum<queue>)  [unwired: 2 in, 2 out]
                    }
                  }
                  frame True {
                    n349 = for {
                      shift-right: [w827] -> w825
                      shift-left: w824 -> [w828]
                      tunnel: string[] ["ARDUINO - ULTRASONIC", "READ ULTRASONIC", "FORWARD", "", "", ""] -> [w826] mode=indexing
                      n350 = Enqueue Element(queue=w828, element=w826) -> (queue out=w827:refnum<queue>)  [unwired: 2 in, 2 out]
                    }
                  }
                }
                n351 = Select(t=State_Type_Definitions,_for_0.26g_versions_and_later_3."True Stop" ("Enum"), s=w807, f=State_Type_Definitions,_for_0.26g_versions_and_later_3."Task 4_B" ("Enum")) -> (s? t:f=w810:T18)
                n352 = Select(t=w810, s=w808, f=State_Type_Definitions,_for_0.26g_versions_and_later_3."Task 4_A" ("Enum")) -> (s? t:f=w816:T18)
              }
              frame "Exit" {
                n353 = for {
                  shift-right: [w835] -> w832
                  shift-left: w829 -> [w836]
                  tunnel: string[] ["STOP", "RESET ENCODERS", "RESET YAW", ""] -> [w834] mode=indexing
                  n354 = Enqueue Element(queue=w836, element=w834) -> (queue out=w835:refnum<queue>)  [unwired: 2 in, 2 out]
                }
              }
            }
          }
          frame "Task 4_B" {
            w842 = u8 20
            # ">> Path blocked >>"
            # ">>> yStepper command>>>"
            # ">> Manual override >>"
            n355 = Dequeue Element(queue=w851, timeout in ms (-1)=w850, error in (no error)=w849) -> (element=w848:T10)  [unwired: 3 out]
            n356 = Less?(x=w844, y=w842) -> (x < y?=w839:bool)
            n357 = Less?(x=w843, y=w842) -> (x < y?=w840:bool)
            n358 = And(x=w840, y=w839) -> (x .and. y?=w841:bool)
            n359 = case shown="\"Start Task 1\", Default" w848 {
              tunnel: [w865 State_Type_Definitions,_for_0.26g_versions_and_later_3."True Stop" ("Enum")] -> w853
              tunnel: [w863 w880] -> w854
              tunnel: w847 -> [w862 _]
              tunnel: w852 -> [w856 _]
              tunnel: [State_Type_Definitions,_for_0.26g_versions_and_later_3."Idle" ("Enum") State_Type_Definitions,_for_0.26g_versions_and_later_3."Shutdown" ("Enum")] -> w846
              tunnel: w841 -> [w855 _]
              frame "Start Task 1", Default {
                # ">> Manual override forces program to true stop >>"
                # ">>If ENABLE or Trigger is set to true>>"
                n360 = Or(x=w855, y=w856) -> (x .or. y?=w861:bool)
                n361 = case shown="False" w855 {
                  tunnel: [w868 w873] -> w863
                  tunnel: w862 -> [w867 w872]
                  frame False {
                    n362 = for {
                      shift-right: [w870] -> w868
                      shift-left: w867 -> [w871]
                      tunnel: string[] ["FORWARD", "READ ULTRASONIC", "READ NAVX"] ("element") -> [w869] mode=indexing
                      n363 = Enqueue Element(queue=w871, element=w869) -> (queue out=w870:refnum<queue>)  [unwired: 2 in, 2 out]
                    }
                  }
                  frame True {
                    n364 = for {
                      shift-right: [w876] -> w873
                      shift-left: w872 -> [w877]
                      tunnel: string[] ["STOP", "RESET YAW", "RESET ENCODERS", "RESET FLAGS"] -> [w875] mode=indexing
                      n365 = Enqueue Element(queue=w877, element=w875) -> (queue out=w876:refnum<queue>)  [unwired: 2 in, 2 out]
                    }
                  }
                }
                n366 = Select(t=State_Type_Definitions,_for_0.26g_versions_and_later_3."True Stop" ("Enum"), s=w856, f=State_Type_Definitions,_for_0.26g_versions_and_later_3."Task 4_C" ("Enum")) -> (s? t:f=w858:T18)
                n367 = Select(t=w858, s=w861, f=State_Type_Definitions,_for_0.26g_versions_and_later_3."Task 4_B" ("Enum")) -> (s? t:f=w865:T18)
              }
              frame "Exit" {
                n368 = for {
                  shift-right: [w883] -> w880
                  shift-left: _ -> [w884]
                  tunnel: string[] ["STOP", "RESET ENCODERS", "RESET YAW", ""] -> [w882] mode=indexing
                  n369 = Enqueue Element(queue=w884, element=w882) -> (queue out=w883:refnum<queue>)  [unwired: 2 in, 2 out]
                }
              }
            }
          }
          frame "Task 4_C" {
            w896 = u8 20
            # ">> xDistance travelled>>"
            # ">> Path NOT blocked >>"
            # ">>> yStepper command>>>"
            # ">> Manual override >>"
            n370 = Dequeue Element(queue=w906, timeout in ms (-1)=w899, error in (no error)=w898) -> (element=w900:T10)  [unwired: 3 out]
            n371 = Greater?(x=w888, y=w896) -> (0:w894:bool)
            n372 = Greater?(x=w893, y=80.0) -> (0:w891:bool)
            n373 = Greater?(x=w887, y=w896) -> (0:w895:bool)
            n374 = And(x=w895, y=w894) -> (x .and. y?=w890:bool)
            n375 = And(x=w891, y=w890) -> (x .and. y?=w889:bool)
            n376 = case shown="\"Start Task 1\", Default" w900 {
              tunnel: [w917 State_Type_Definitions,_for_0.26g_versions_and_later_3."True Stop" ("Enum")] -> w903
              tunnel: [w915 w933] -> w902
              tunnel: w905 -> [w914 w930]
              tunnel: w904 -> [w908 _]
              tunnel: [State_Type_Definitions,_for_0.26g_versions_and_later_3."Idle" ("t") State_Type_Definitions,_for_0.26g_versions_and_later_3."Shutdown" ("Enum")] -> w901
              tunnel: w889 -> [w907 _]
              frame "Start Task 1", Default {
                # ">> Manual override forces program to true stop >>"
                # ">>If ENABLE or Trigger is set to true>>"
                n377 = Or(x=w907, y=w908) -> (x .or. y?=w913:bool)
                n378 = case shown="False" w907 {
                  tunnel: [w920 w925] -> w915
                  tunnel: w914 -> [w918 w924]
                  frame False {
                    n379 = for {
                      shift-right: [w922] -> w920
                      shift-left: w918 -> [w923]
                      tunnel: string[] ["RIGHT", "READ NAVX", "READ ENCODERS", "READ ULTRASONIC"] ("element") -> [w921] mode=indexing
                      n380 = Enqueue Element(queue=w923, element=w921) -> (queue out=w922:refnum<queue>)  [unwired: 2 in, 2 out]
                    }
                  }
                  frame True {
                    n381 = for {
                      shift-right: [w928] -> w925
                      shift-left: w924 -> [w929]
                      tunnel: string[] ["STOP", "RESET YAW", "RESET ENCODERS", "ARDUINO - ULTRASONIC"] -> [w927] mode=indexing
                      n382 = Enqueue Element(queue=w929, element=w927) -> (queue out=w928:refnum<queue>)  [unwired: 2 in, 2 out]
                    }
                  }
                }
                n383 = Select(t=State_Type_Definitions,_for_0.26g_versions_and_later_3."True Stop" ("Enum"), s=w908, f=State_Type_Definitions,_for_0.26g_versions_and_later_3."Task 4_D" ("Enum")) -> (s? t:f=w909:T18)
                n384 = Select(t=w909, s=w913, f=State_Type_Definitions,_for_0.26g_versions_and_later_3."Task 4_C" ("Enum")) -> (s? t:f=w917:T18)
              }
              frame "Exit" {
                n385 = for {
                  shift-right: [w936] -> w933
                  shift-left: w930 -> [w937]
                  tunnel: string[] ["STOP", "RESET ENCODERS", "RESET YAW", ""] -> [w935] mode=indexing
                  n386 = Enqueue Element(queue=w937, element=w935) -> (queue out=w936:refnum<queue>)  [unwired: 2 in, 2 out]
                }
              }
            }
          }
          frame "Task 4_D" {
            w960 = u8 20
            # ">>> Motor control cluster >>>"
            # ">> Line detected >>"
            # ">> yDistance travelled>>"
            # ">> Path blocked >>"
            # ">>> yStepper command>>>"
            # ">> Manual override >>"
            n387 = Less?(x=w945, y=w960) -> (x < y?=w958:bool)
            n388 = Greater?(x=w949, y=200.0) -> (0:w956:bool)
            n389 = Less?(x=w944, y=w960) -> (x < y?=w959:bool)
            n390 = And(x=w959, y=w958) -> (x .and. y?=w955:bool)
            n391 = Dequeue Element(queue=w952, timeout in ms (-1)=w951, error in (no error)=w950) -> (element=w961:T10)  [unwired: 3 out]
            n392 = Or(x=w956, y=w955) -> (x .or. y?=w939:bool)
            n393 = And(x=w940, y=w939) -> (x .and. y?=w938:bool)
            n394 = case shown="\"Start Task 1\", Default" w961 {
              tunnel: [w972 State_Type_Definitions,_for_0.26g_versions_and_later_3."True Stop" ("Enum")] -> w948
              tunnel: [w970 w988] -> w946
              tunnel: w953 -> [w969 w985]
              tunnel: w954 -> [w963 _]
              tunnel: [State_Type_Definitions,_for_0.26g_versions_and_later_3."Idle" ("t") State_Type_Definitions,_for_0.26g_versions_and_later_3."Shutdown" ("Enum")] -> w947
              tunnel: w938 -> [w962 _]
              frame "Start Task 1", Default {
                # ">> Manual override forces program to true stop >>"
                # ">>If ENABLE or Trigger is set to true>>"
                n395 = Or(x=w962, y=w963) -> (x .or. y?=w968:bool)
                n396 = case shown="False" w962 {
                  tunnel: [w975 w980] -> w970
                  tunnel: w969 -> [w973 w979]
                  frame False {
                    n397 = for {
                      shift-right: [w977] -> w975
                      shift-left: w973 -> [w978]
                      tunnel: string[] ["FORWARD", "READ NAVX", "READ ENCODERS", "READ ULTRASONIC", "READ LINE SENSOR"] ("element") -> [w976] mode=indexing
                      n398 = Enqueue Element(queue=w978, element=w976) -> (queue out=w977:refnum<queue>)  [unwired: 2 in, 2 out]
                    }
                  }
                  frame True {
                    n399 = for {
                      shift-right: [w983] -> w980
                      shift-left: w979 -> [w984]
                      tunnel: string[] ["STOP", "RESET YAW", "RESET ENCODERS", "RESET FLAGS"] -> [w982] mode=indexing
                      n400 = Enqueue Element(queue=w984, element=w982) -> (queue out=w983:refnum<queue>)  [unwired: 2 in, 2 out]
                    }
                  }
                }
                n401 = Select(t=State_Type_Definitions,_for_0.26g_versions_and_later_3."True Stop" ("Enum"), s=w963, f=State_Type_Definitions,_for_0.26g_versions_and_later_3."True Stop" ("Enum")) -> (s? t:f=w964:T18)
                n402 = Select(t=w964, s=w968, f=State_Type_Definitions,_for_0.26g_versions_and_later_3."Task 4_D" ("Enum")) -> (s? t:f=w972:T18)
              }
              frame "Exit" {
                n403 = for {
                  shift-right: [w991] -> w988
                  shift-left: w985 -> [w992]
                  tunnel: string[] ["STOP", "RESET ENCODERS", "RESET YAW", ""] -> [w990] mode=indexing
                  n404 = Enqueue Element(queue=w992, element=w990) -> (queue out=w991:refnum<queue>)  [unwired: 2 in, 2 out]
                }
              }
            }
          }
          frame "Task 5A: RAISING ARM" {
            # "Stays in Task 5_A until stepper reaches desired \nheight"
            # ">>> Motor control cluster >>>"
            # ">>> yStepper command>>>"
            # ">> Manual override >>"
            n405 = Dequeue Element(queue=w1003, timeout in ms (-1)=w1002, error in (no error)=w1004) -> (element=w1001:T10)  [unwired: 3 out]
            n406 = Equal?(x=w1000, y=u8 60) -> (x = y?=w998:bool)
            n407 = case shown="\"Start Task 1\", Default" w1001 {
              tunnel: [w1014 State_Type_Definitions,_for_0.26g_versions_and_later_3."True Stop" ("Enum")] -> w1005
              tunnel: [w1017 w1034] -> w1006
              tunnel: [State_Type_Definitions,_for_0.26g_versions_and_later_3."Idle" ("Enum") State_Type_Definitions,_for_0.26g_versions_and_later_3."Shutdown" ("Enum")] -> w1007
              tunnel: w998 -> [w1013 _]
              tunnel: w997 -> [w1012 _]
              tunnel: w996 -> [w1008 w1031]
              frame "Start Task 1", Default {
                # "T: Go back to idle, F: Continue with task\""
                # ">> Manual override >>"
                n408 = case shown="False" w1013 {
                  tunnel: [w1021 w1027] -> w1017
                  tunnel: w1008 -> [w1019 w1025]
                  frame False {
                    n409 = for {
                      tunnel: string[] ["Z STEPPER CAM HEIGHT", "READ STEPPER VALUES"] ("element") -> [w1022] mode=indexing
                      shift-right: [w1024] -> w1021
                      shift-left: w1019 -> [w1023]
                      n410 = Enqueue Element(queue=w1023, element=w1022) -> (queue out=w1024:refnum<queue>)  [unwired: 2 in, 2 out]
                    }
                  }
                  frame True {
                    n411 = for {
                      shift-right: [w1029] -> w1027
                      shift-left: w1025 -> [w1030]
                      tunnel: string[] ["RESET FLAGS", "RESET YAW", "RESET ENCODERS"] -> [w1028] mode=indexing
                      n412 = Enqueue Element(queue=w1030, element=w1028) -> (queue out=w1029:refnum<queue>)  [unwired: 2 in, 2 out]
                    }
                  }
                }
                n413 = Or(x=w1013, y=w1012) -> (x .or. y?=w1015:bool)
                n414 = Select(t=State_Type_Definitions,_for_0.26g_versions_and_later_3."True Stop" ("Enum"), s=w1012, f=State_Type_Definitions,_for_0.26g_versions_and_later_3."Task 5B: STILL WAITING" ("Enum")) -> (s? t:f=w1009:T18)
                n415 = Select(t=w1009, s=w1015, f=State_Type_Definitions,_for_0.26g_versions_and_later_3."Task 5A: RAISING ARM" ("Enum")) -> (s? t:f=w1014:T18)
              }
              frame "Exit" {
                n416 = for {
                  shift-right: [w1037] -> w1034
                  shift-left: w1031 -> [w1038]
                  tunnel: string[] ["STOP", "RESET ENCODERS", "RESET YAW", "ARDUINO MODE 0"] -> [w1036] mode=indexing
                  n417 = Enqueue Element(queue=w1038, element=w1036) -> (queue out=w1037:refnum<queue>)  [unwired: 2 in, 2 out]
                }
              }
            }
          }
          frame "Task 5B: STILL WAITING" {
            # ">>> yStepper command>>>"
            n418 = Dequeue Element(queue=w1045, timeout in ms (-1)=w1044, error in (no error)=w1046) -> (element=w1043:T10)  [unwired: 3 out]
            n419 = local read "Rising Edge"() -> (w1039:bool)
            n420 = case shown="\"Start Task 1\", Default" w1043 {
              tunnel: [w1058 State_Type_Definitions,_for_0.26g_versions_and_later_3."True Stop" ("Enum")] -> w1048
              tunnel: [w1061 w1078] -> w1047
              tunnel: [State_Type_Definitions,_for_0.26g_versions_and_later_3."Idle" ("Enum") State_Type_Definitions,_for_0.26g_versions_and_later_3."Shutdown" ("Enum")] -> w1049
              tunnel: w1051 -> [w1057 _]
              tunnel: w1050 -> [w1053 w1075]
              tunnel: w1039 -> [w1052 _]
              frame "Start Task 1", Default {
                # "T: Go back to idle, F: Continue with task\""
                # ">> Manual override >>"
                n421 = case shown="False" w1052 {
                  tunnel: [w1065 w1071] -> w1061
                  tunnel: w1053 -> [w1063 w1069]
                  frame False {
                    n422 = for {
                      tunnel: string[] ["READ IR", "READ NAVX", ""] ("element") -> [w1066] mode=indexing
                      shift-right: [w1068] -> w1065
                      shift-left: w1063 -> [w1067]
                      n423 = Enqueue Element(queue=w1067, element=w1066) -> (queue out=w1068:refnum<queue>)  [unwired: 2 in, 2 out]
                    }
                  }
                  frame True {
                    n424 = for {
                      shift-right: [w1073] -> w1071
                      shift-left: w1069 -> [w1074]
                      tunnel: string[] ["Z STEPPER GRAB HEIGHT", "READ STEPPER VALUES", "", ""] -> [w1072] mode=indexing
                      n425 = Enqueue Element(queue=w1074, element=w1072) -> (queue out=w1073:refnum<queue>)  [unwired: 2 in, 2 out]
                    }
                  }
                }
                n426 = Or(x=w1052, y=w1057) -> (x .or. y?=w1059:bool)
                n427 = Select(t=State_Type_Definitions,_for_0.26g_versions_and_later_3."True Stop" ("Enum"), s=w1057, f=State_Type_Definitions,_for_0.26g_versions_and_later_3."Task 5C: GOING DOWN" ("Enum")) -> (s? t:f=w1054:T18)
                n428 = Select(t=w1054, s=w1059, f=State_Type_Definitions,_for_0.26g_versions_and_later_3."Task 5B: STILL WAITING" ("Enum")) -> (s? t:f=w1058:T18)
              }
              frame "Exit" {
                n429 = for {
                  shift-right: [w1081] -> w1078
                  shift-left: w1075 -> [w1082]
                  tunnel: string[] ["STOP", "RESET ENCODERS", "RESET YAW", "ARDUINO MODE 0"] -> [w1080] mode=indexing
                  n430 = Enqueue Element(queue=w1082, element=w1080) -> (queue out=w1081:refnum<queue>)  [unwired: 2 in, 2 out]
                }
              }
            }
          }
          frame "Task 5C: GOING DOWN" {
            # ">>> Motor control cluster >>>"
            # ">>> yStepper command>>>"
            # ">> Manual override >>"
            n431 = Equal?(x=w1085, y=u8 1) -> (x = y?=w1083:bool)
            n432 = Dequeue Element(queue=w1095, timeout in ms (-1)=w1094, error in (no error)=w1093) -> (element=w1092:T10)  [unwired: 3 out]
            n433 = case shown="\"Start Task 1\", Default" w1092 {
              tunnel: [w1104 State_Type_Definitions,_for_0.26g_versions_and_later_3."True Stop" ("Enum")] -> w1097
              tunnel: [w1107 w1124] -> w1090
              tunnel: [State_Type_Definitions,_for_0.26g_versions_and_later_3."Idle" ("Enum") State_Type_Definitions,_for_0.26g_versions_and_later_3."Shutdown" ("Enum")] -> w1089
              tunnel: w1091 -> [w1098 _]
              tunnel: w1096 -> [w1103 w1121]
              tunnel: w1083 -> [w1102 _]
              frame "Start Task 1", Default {
                # ">> Is time up? >>"
                # "Determines if object is in range to pick up"
                # ">> Manual override >>"
                n434 = case shown="False" w1102 {
                  tunnel: [w1111 w1117] -> w1107
                  tunnel: w1103 -> [w1110 w1115]
                  frame False {
                    n435 = for {
                      tunnel: string[] ["READ STEPPER VALUES", "Z STEPPER GRAB HEIGHT", "", ""] -> [w1112] mode=indexing
                      shift-right: [w1114] -> w1111
                      shift-left: w1110 -> [w1113]
                      n436 = Enqueue Element(queue=w1113, element=w1112) -> (queue out=w1114:refnum<queue>)  [unwired: 2 in, 2 out]
                    }
                  }
                  frame True {
                    n437 = for {
                      shift-right: [w1119] -> w1117
                      shift-left: w1115 -> [w1120]
                      tunnel: string[] ["RESET FLAGS", "RESET YAW", "SET TIMER 5"] -> [w1118] mode=indexing
                      n438 = Enqueue Element(queue=w1120, element=w1118) -> (queue out=w1119:refnum<queue>)  [unwired: 2 in, 2 out]
                    }
                  }
                }
                n439 = Or(x=w1102, y=w1098) -> (x .or. y?=w1105:bool)
                n440 = Select(t=State_Type_Definitions,_for_0.26g_versions_and_later_3."True Stop" ("Enum"), s=w1098, f=State_Type_Definitions,_for_0.26g_versions_and_later_3."Task 5D: GRAB" ("Enum")) -> (s? t:f=w1100:T18)
                n441 = Select(t=w1100, s=w1105, f=State_Type_Definitions,_for_0.26g_versions_and_later_3."Task 5C: GOING DOWN" ("Enum")) -> (s? t:f=w1104:T18)
              }
              frame "Exit" {
                n442 = for {
                  shift-right: [w1127] -> w1124
                  shift-left: w1121 -> [w1128]
                  tunnel: string[] ["STOP", "RESET ENCODERS", "RESET YAW", "ARDUINO MODE 0"] -> [w1126] mode=indexing
                  n443 = Enqueue Element(queue=w1128, element=w1126) -> (queue out=w1127:refnum<queue>)  [unwired: 2 in, 2 out]
                }
              }
            }
          }
          frame "Task 5D: GRAB" {
            # ">>> Motor control cluster >>>"
            # ">>> yStepper command>>>"
            n444 = Dequeue Element(queue=w1136, timeout in ms (-1)=w1135, error in (no error)=w1134) -> (element=w1133:T10)  [unwired: 3 out]
            n445 = case shown="\"Start Task 1\", Default" w1133 {
              tunnel: [w1148 State_Type_Definitions,_for_0.26g_versions_and_later_3."True Stop" ("Enum")] -> w1140
              tunnel: [w1151 w1168] -> w1139
              tunnel: [State_Type_Definitions,_for_0.26g_versions_and_later_3."Idle" ("Enum") State_Type_Definitions,_for_0.26g_versions_and_later_3."Shutdown" ("Enum")] -> w1141
              tunnel: w1137 -> [w1147 _]
              tunnel: w1138 -> [w1143 w1165]
              tunnel: w1131 -> [w1142 _]
              frame "Start Task 1", Default {
                # ">> T: Breaks out of state loop; F: Stays in loop>>"
                # ">> Manual override >>"
                # ">> Checks if time is up>>"
                # "Stays in Task 5D until the object is detected"
                # "T: Go back to idle, F: Continue with task\""
                # ">> Manual override >>"
                n446 = case shown="True" w1142 {
                  tunnel: [w1155 w1161] -> w1151
                  tunnel: w1143 -> [w1153 w1159]
                  frame False {
                    n447 = for {
                      tunnel: string[] ["START TIMER", "CLOSE CLAW", ""] ("element") -> [w1156] mode=indexing
                      shift-right: [w1158] -> w1155
                      shift-left: w1153 -> [w1157]
                      n448 = Enqueue Element(queue=w1157, element=w1156) -> (queue out=w1158:refnum<queue>)  [unwired: 2 in, 2 out]
                    }
                  }
                  frame True {
                    n449 = for {
                      shift-right: [w1163] -> w1161
                      shift-left: w1159 -> [w1164]
                      tunnel: string[] ["READ STEPPER VALUES", "ZSTEPPER BOX HEIGHT", ""] -> [w1162] mode=indexing
                      n450 = Enqueue Element(queue=w1164, element=w1162) -> (queue out=w1163:refnum<queue>)  [unwired: 2 in, 2 out]
                    }
                  }
                }
                n451 = Or(x=w1142, y=w1147) -> (x .or. y?=w1149:bool)
                n452 = Select(t=State_Type_Definitions,_for_0.26g_versions_and_later_3."True Stop" ("Enum"), s=w1147, f=State_Type_Definitions,_for_0.26g_versions_and_later_3."Task 5E: GOING UP" ("Enum")) -> (s? t:f=w1144:T18)
                n453 = Select(t=w1144, s=w1149, f=State_Type_Definitions,_for_0.26g_versions_and_later_3."Task 5D: GRAB" ("Enum")) -> (s? t:f=w1148:T18)
              }
              frame "Exit" {
                n454 = for {
                  shift-right: [w1171] -> w1168
                  shift-left: w1165 -> [w1172]
                  tunnel: string[] ["STOP", "RESET ENCODERS", "RESET YAW", "ARDUINO MODE 0"] -> [w1170] mode=indexing
                  n455 = Enqueue Element(queue=w1172, element=w1170) -> (queue out=w1171:refnum<queue>)  [unwired: 2 in, 2 out]
                }
              }
            }
          }
          frame "Task 5E: GOING UP" {
            # ">>> Motor control cluster >>>"
            # ">>> yStepper command>>>"
            n456 = Equal?(x=w1175, y=u8 50) -> (x = y?=w1173:bool)
            n457 = Dequeue Element(queue=w1183, timeout in ms (-1)=w1184, error in (no error)=w1185) -> (element=w1187:T10)  [unwired: 3 out]
            n458 = case shown="\"Start Task 1\", Default" w1187 {
              tunnel: [w1195 State_Type_Definitions,_for_0.26g_versions_and_later_3."True Stop" ("Enum")] -> w1181
              tunnel: [w1197 w1214] -> w1179
              tunnel: [State_Type_Definitions,_for_0.26g_versions_and_later_3."Idle" ("Enum") State_Type_Definitions,_for_0.26g_versions_and_later_3."Shutdown" ("Enum")] -> w1180
              tunnel: w1186 -> [w1194 _]
              tunnel: w1182 -> [w1190 w1211]
              tunnel: w1173 -> [w1189 _]
              frame "Start Task 1", Default {
                # ">> T: Breaks out of state loop; F: Stays in loop>>"
                # ">> Manual override >>"
                # ">> Checks if time is up>>"
                # "Stays in Task 5D until the object is detected"
                # "T: Go back to idle, F: Continue with task\""
                # ">> Manual override >>"
                n459 = Or(x=w1189, y=w1194) -> (x .or. y?=w1188:bool)
                n460 = case shown="False" w1188 {
                  tunnel: [w1201 w1207] -> w1197
                  tunnel: w1190 -> [w1199 w1205]
                  frame False {
                    n461 = for {
                      tunnel: string[] ["READ STEPPER VALUES", "ZSTEPPER BOX HEIGHT", ""] ("element") -> [w1202] mode=indexing
                      shift-right: [w1204] -> w1201
                      shift-left: w1199 -> [w1203]
                      n462 = Enqueue Element(queue=w1203, element=w1202) -> (queue out=w1204:refnum<queue>)  [unwired: 2 in, 2 out]
                    }
                  }
                  frame True {
                    n463 = for {
                      shift-right: [w1209] -> w1207
                      shift-left: w1205 -> [w1210]
                      tunnel: string[] ["CAM CLOSE", "DISPOSE BUFFERS", ""] -> [w1208] mode=indexing
                      n464 = Enqueue Element(queue=w1210, element=w1208) -> (queue out=w1209:refnum<queue>)  [unwired: 2 in, 2 out]
                    }
                  }
                }
                n465 = Select(t=State_Type_Definitions,_for_0.26g_versions_and_later_3."True Stop" ("Enum"), s=w1194, f=State_Type_Definitions,_for_0.26g_versions_and_later_3."True Stop" ("Enum")) -> (s? t:f=w1191:T18)
                n466 = Select(t=w1191, s=w1188, f=State_Type_Definitions,_for_0.26g_versions_and_later_3."Task 5E: GOING UP" ("Enum")) -> (s? t:f=w1195:T18)
              }
              frame "Exit" {
                n467 = for {
                  shift-right: [w1217] -> w1214
                  shift-left: w1211 -> [w1218]
                  tunnel: string[] ["STOP", "RESET ENCODERS", "RESET YAW", "ARDUINO MODE 0"] -> [w1216] mode=indexing
                  n468 = Enqueue Element(queue=w1218, element=w1216) -> (queue out=w1217:refnum<queue>)  [unwired: 2 in, 2 out]
                }
              }
            }
          }
          frame "Task 5F: ARM GRAB HEIGHT" {
            # ">>> Motor control cluster >>>"
            # ">>> yStepper command>>>"
            # ">> Manual override >>"
            n469 = Dequeue Element(queue=w1229, timeout in ms (-1)=w1228, error in (no error)=w1230) -> (element=w1227:T10)  [unwired: 3 out]
            n470 = Equal?(x=w1226, y=u8 1) -> (x = y?=w1224:bool)
            n471 = case shown="\"Start Task 1\", Default" w1227 {
              tunnel: [w1240 State_Type_Definitions,_for_0.26g_versions_and_later_3."True Stop" ("Enum")] -> w1231
              tunnel: [w1243 w1260] -> w1232
              tunnel: [State_Type_Definitions,_for_0.26g_versions_and_later_3."Idle" ("Enum") State_Type_Definitions,_for_0.26g_versions_and_later_3."Shutdown" ("Enum")] -> w1233
              tunnel: w1224 -> [w1239 _]
              tunnel: w1223 -> [w1238 _]
              tunnel: w1222 -> [w1234 w1257]
              frame "Start Task 1", Default {
                # "Stays in Task 5F until stepper reaches desired \nheight"
                # "T: Go back to idle, F: Continue with task\""
                # ">> Manual override >>"
                n472 = case shown="True" w1239 {
                  tunnel: [w1247 w1253] -> w1243
                  tunnel: w1234 -> [w1245 w1251]
                  frame False {
                    n473 = for {
                      tunnel: string[] ["Z STEPPER GRAB HEIGHT", "READ STEPPER VALUES"] ("element") -> [w1248] mode=indexing
                      shift-right: [w1250] -> w1247
                      shift-left: w1245 -> [w1249]
                      n474 = Enqueue Element(queue=w1249, element=w1248) -> (queue out=w1250:refnum<queue>)  [unwired: 2 in, 2 out]
                    }
                  }
                  frame True {
                    n475 = for {
                      shift-right: [w1255] -> w1253
                      shift-left: w1251 -> [w1256]
                      tunnel: string[] ["RESET YAW", "RESET ENCODERS", "RESET FLAGS"] -> [w1254] mode=indexing
                      n476 = Enqueue Element(queue=w1256, element=w1254) -> (queue out=w1255:refnum<queue>)  [unwired: 2 in, 2 out]
                    }
                  }
                }
                n477 = Or(x=w1239, y=w1238) -> (x .or. y?=w1241:bool)
                n478 = Select(t=State_Type_Definitions,_for_0.26g_versions_and_later_3."True Stop" ("Enum"), s=w1238, f=State_Type_Definitions,_for_0.26g_versions_and_later_3."True Stop" ("Enum")) -> (s? t:f=w1235:T18)
                n479 = Select(t=w1235, s=w1241, f=State_Type_Definitions,_for_0.26g_versions_and_later_3."Task 5F: ARM GRAB HEIGHT" ("Enum")) -> (s? t:f=w1240:T18)
              }
              frame "Exit" {
                n480 = for {
                  shift-right: [w1263] -> w1260
                  shift-left: w1257 -> [w1264]
                  tunnel: string[] ["STOP", "RESET ENCODERS", "RESET YAW", "ARDUINO MODE 0"] -> [w1262] mode=indexing
                  n481 = Enqueue Element(queue=w1264, element=w1262) -> (queue out=w1263:refnum<queue>)  [unwired: 2 in, 2 out]
                }
              }
            }
          }
          frame "Task 5G: CLOSE CLAW" {
            # ">>> yStepper command>>>"
            # ">> Manual override >>"
            n482 = Dequeue Element(queue=w1275, timeout in ms (-1)=w1274, error in (no error)=w1273) -> (element=w1272:T10)  [unwired: 3 out]
            n483 = case shown="\"Start Task 1\", Default" w1272 {
              tunnel: [w1284 State_Type_Definitions,_for_0.26g_versions_and_later_3."True Stop" ("Enum")] -> w1277
              tunnel: [w1287 w1304] -> w1270
              tunnel: [State_Type_Definitions,_for_0.26g_versions_and_later_3."Idle" ("Enum") State_Type_Definitions,_for_0.26g_versions_and_later_3."Shutdown" ("Enum")] -> w1269
              tunnel: w1271 -> [w1278 _]
              tunnel: w1276 -> [w1283 w1301]
              tunnel: w1267 -> [w1282 _]
              frame "Start Task 1", Default {
                # ">> Is time up? >>"
                # "Determines if object is in range to pick up"
                # ">> Manual override >>"
                n484 = case shown="True" w1282 {
                  tunnel: [w1291 w1297] -> w1287
                  tunnel: w1283 -> [w1289 w1295]
                  frame False {
                    n485 = for {
                      tunnel: string[] ["CLOSE CLAW", "START TIMER"] ("element") -> [w1292] mode=indexing
                      shift-right: [w1294] -> w1291
                      shift-left: w1289 -> [w1293]
                      n486 = Enqueue Element(queue=w1293, element=w1292) -> (queue out=w1294:refnum<queue>)  [unwired: 2 in, 2 out]
                    }
                  }
                  frame True {
                    n487 = for {
                      shift-right: [w1299] -> w1297
                      shift-left: w1295 -> [w1300]
                      tunnel: string[] ["READ STEPPER VALUES", "", ""] -> [w1298] mode=indexing
                      n488 = Enqueue Element(queue=w1300, element=w1298) -> (queue out=w1299:refnum<queue>)  [unwired: 2 in, 2 out]
                    }
                  }
                }
                n489 = Or(x=w1282, y=w1278) -> (x .or. y?=w1285:bool)
                n490 = Select(t=State_Type_Definitions,_for_0.26g_versions_and_later_3."True Stop" ("Enum"), s=w1278, f=State_Type_Definitions,_for_0.26g_versions_and_later_3."Task 5H: RAISE ARM" ("Enum")) -> (s? t:f=w1280:T18)
                n491 = Select(t=w1280, s=w1285, f=State_Type_Definitions,_for_0.26g_versions_and_later_3."Task 5G: CLOSE CLAW" ("Enum")) -> (s? t:f=w1284:T18)
              }
              frame "Exit" {
                n492 = for {
                  shift-right: [w1307] -> w1304
                  shift-left: w1301 -> [w1308]
                  tunnel: string[] ["STOP", "RESET ENCODERS", "RESET YAW", "ARDUINO MODE 0"] -> [w1306] mode=indexing
                  n493 = Enqueue Element(queue=w1308, element=w1306) -> (queue out=w1307:refnum<queue>)  [unwired: 2 in, 2 out]
                }
              }
            }
          }
          frame "Task 5H: RAISE ARM" {
            # ">>> yStepper command>>>"
            # ">> Manual override >>"
            n494 = Dequeue Element(queue=w1319, timeout in ms (-1)=w1318, error in (no error)=w1320) -> (element=w1317:T10)  [unwired: 3 out]
            n495 = Equal?(x=w1316, y=u8 60) -> (x = y?=w1314:bool)
            n496 = case shown="\"Start Task 1\", Default" w1317 {
              tunnel: [w1330 State_Type_Definitions,_for_0.26g_versions_and_later_3."True Stop" ("Enum")] -> w1321
              tunnel: [w1333 w1350] -> w1322
              tunnel: [State_Type_Definitions,_for_0.26g_versions_and_later_3."Idle" ("Enum") State_Type_Definitions,_for_0.26g_versions_and_later_3."Shutdown" ("Enum")] -> w1323
              tunnel: w1314 -> [w1329 _]
              tunnel: w1313 -> [w1328 _]
              tunnel: w1312 -> [w1324 w1347]
              frame "Start Task 1", Default {
                # "Stays in Task 5_A until stepper reaches desired \nheight"
                # "T: Go back to idle, F: Continue with task\""
                # ">> Manual override >>"
                n497 = case shown="False" w1329 {
                  tunnel: [w1337 w1343] -> w1333
                  tunnel: w1324 -> [w1335 w1341]
                  frame False {
                    n498 = for {
                      tunnel: string[] ["Z STEPPER CAM HEIGHT", "READ STEPPER VALUES"] ("element") -> [w1338] mode=indexing
                      shift-right: [w1340] -> w1337
                      shift-left: w1335 -> [w1339]
                      n499 = Enqueue Element(queue=w1339, element=w1338) -> (queue out=w1340:refnum<queue>)  [unwired: 2 in, 2 out]
                    }
                  }
                  frame True {
                    n500 = for {
                      shift-right: [w1345] -> w1343
                      shift-left: w1341 -> [w1346]
                      tunnel: string[] ["ARDUINO - ULTRASONIC", "READ ULTRASONIC", ""] -> [w1344] mode=indexing
                      n501 = Enqueue Element(queue=w1346, element=w1344) -> (queue out=w1345:refnum<queue>)  [unwired: 2 in, 2 out]
                    }
                  }
                }
                n502 = Or(x=w1329, y=w1328) -> (x .or. y?=w1331:bool)
                n503 = Select(t=State_Type_Definitions,_for_0.26g_versions_and_later_3."True Stop" ("Enum"), s=w1328, f=State_Type_Definitions,_for_0.26g_versions_and_later_3."True Stop" ("Enum")) -> (s? t:f=w1325:T18)
                n504 = Select(t=w1325, s=w1331, f=State_Type_Definitions,_for_0.26g_versions_and_later_3."Task 5H: RAISE ARM" ("Enum")) -> (s? t:f=w1330:T18)
              }
              frame "Exit" {
                n505 = for {
                  shift-right: [w1353] -> w1350
                  shift-left: w1347 -> [w1354]
                  tunnel: string[] ["STOP", "RESET ENCODERS", "RESET YAW", "ARDUINO MODE 0"] -> [w1352] mode=indexing
                  n506 = Enqueue Element(queue=w1354, element=w1352) -> (queue out=w1353:refnum<queue>)  [unwired: 2 in, 2 out]
                }
              }
            }
          }
          frame "Task 6A: RAISE ARM" {
            # ">>> Motor control cluster >>>"
            # ">>> yStepper command>>>"
            n507 = Equal?(x=w1362, y=u8 60) -> (x = y?=w1356:bool)
            n508 = Dequeue Element(queue=w1366, timeout in ms (-1)=w1365, error in (no error)=w1364) -> (element=w1371:T10)  [unwired: 3 out]
            n509 = local read "Rising Edge"() -> (w1357:bool)
            n510 = And(x=w1357, y=w1356) -> (x .and. y?=w1355:bool)
            n511 = case shown="\"Start Task 1\", Default" w1371 {
              tunnel: [w1381 State_Type_Definitions,_for_0.26g_versions_and_later_3."True Stop" ("Enum")] -> w1369
              tunnel: [w1380 w1397] -> w1368
              tunnel: [State_Type_Definitions,_for_0.26g_versions_and_later_3."Idle" ("Enum") State_Type_Definitions,_for_0.26g_versions_and_later_3."Shutdown" ("Enum")] -> w1370
              tunnel: w1367 -> [w1377 _]
              tunnel: w1363 -> [w1378 _]
              tunnel: w1355 -> [w1375 _]
              frame "Start Task 1", Default {
                n512 = Or(x=w1375, y=w1377) -> (x .or. y?=w1372:bool)
                n513 = case shown="False" w1372 {
                  tunnel: [w1385 w1391] -> w1380
                  tunnel: w1378 -> [w1383 w1390]
                  frame False {
                    n514 = for {
                      tunnel: string[] ["Z STEPPER CAM HEIGHT", "READ STEPPER VALUES"] ("element") -> [w1386] mode=indexing
                      shift-right: [w1388] -> w1385
                      shift-left: w1383 -> [w1387]
                      n515 = Enqueue Element(queue=w1387, element=w1386) -> (queue out=w1388:refnum<queue>)  [unwired: 2 in, 2 out]
                    }
                  }
                  frame True {
                    n516 = for {
                      shift-right: [w1393] -> w1391
                      shift-left: w1390 -> [w1394]
                      tunnel: string[] ["OPEN LOG CAM", "SET TIMER 2", "OPEN IMAQ REF", "", ""] -> [w1392] mode=indexing
                      n517 = Enqueue Element(queue=w1394, element=w1392) -> (queue out=w1393:refnum<queue>)  [unwired: 2 in, 2 out]
                    }
                  }
                }
                n518 = Select(t=State_Type_Definitions,_for_0.26g_versions_and_later_3."Task 6B: CAM BURST" ("Enum"), s=w1375, f=State_Type_Definitions,_for_0.26g_versions_and_later_3."True Stop" ("Enum")) -> (s? t:f=w1373:T18)
                n519 = Select(t=w1373, s=w1372, f=State_Type_Definitions,_for_0.26g_versions_and_later_3."Task 6A: RAISE ARM" ("Enum")) -> (s? t:f=w1381:T18)
              }
              frame "Exit" {
                n520 = for {
                  shift-right: [w1400] -> w1397
                  shift-left: _ -> [w1401]
                  tunnel: string[] ["STOP", "RESET ENCODERS", "RESET YAW", "ARDUINO MODE 0"] -> [w1399] mode=indexing
                  n521 = Enqueue Element(queue=w1401, element=w1399) -> (queue out=w1400:refnum<queue>)  [unwired: 2 in, 2 out]
                }
              }
            }
          }
          frame "Task 6B: CAM BURST" {
            # ">> Manual override >>"
            # ">>> Motor control cluster >>>"
            # ">>> yStepper command>>>"
            n522 = Dequeue Element(queue=w1413, timeout in ms (-1)=w1411, error in (no error)=w1412) -> (element=w1410:T10)  [unwired: 3 out]
            n523 = case shown="\"Start Task 1\", Default" w1410 {
              tunnel: [w1421 State_Type_Definitions,_for_0.26g_versions_and_later_3."True Stop" ("Enum")] -> w1407
              tunnel: [w1419 w1439] -> w1414
              tunnel: [State_Type_Definitions,_for_0.26g_versions_and_later_3."Idle" ("Enum") State_Type_Definitions,_for_0.26g_versions_and_later_3."Shutdown" ("Enum")] -> w1408
              tunnel: w1409 -> [w1417 _]
              tunnel: w1406 -> [w1418 w1436]
              tunnel: w1402 -> [w1415 _]
              frame "Start Task 1", Default {
                n524 = Or(x=w1415, y=w1417) -> (x .or. y?=w1416:bool)
                n525 = case shown="True" w1416 {
                  tunnel: [w1426 w1432] -> w1419
                  tunnel: w1418 -> [w1424 w1430]
                  frame False {
                    n526 = for {
                      tunnel: string[] ["CAM ACQ", "START TIMER"] ("element") -> [w1427] mode=indexing
                      shift-right: [w1429] -> w1426
                      shift-left: w1424 -> [w1428]
                      n527 = Enqueue Element(queue=w1428, element=w1427) -> (queue out=w1429:refnum<queue>)  [unwired: 2 in, 2 out]
                    }
                  }
                  frame True {
                    n528 = for {
                      shift-right: [w1434] -> w1432
                      shift-left: w1430 -> [w1435]
                      tunnel: string[] ["CAM CLOSE", "PROCESS IMAGE", "SET TIMER 2", "RESET ENCODERS"] -> [w1433] mode=indexing
                      n529 = Enqueue Element(queue=w1435, element=w1433) -> (queue out=w1434:refnum<queue>)  [unwired: 2 in, 2 out]
                    }
                  }
                }
                n530 = Select(t=State_Type_Definitions,_for_0.26g_versions_and_later_3."Task 6C: PROCESS IMAGE" ("Enum"), s=w1416, f=State_Type_Definitions,_for_0.26g_versions_and_later_3."Task 6B: CAM BURST" ("Enum")) -> (s? t:f=w1421:T18)
              }
              frame "Exit" {
                # ">> State after true stop >>"
                # ">> Goes to true stop >>"
                n531 = for {
                  shift-right: [w1442] -> w1439
                  shift-left: w1436 -> [w1443]
                  tunnel: string[] ["STOP", "RESET ENCODERS", "RESET YAW", ""] -> [w1441] mode=indexing
                  n532 = Enqueue Element(queue=w1443, element=w1441) -> (queue out=w1442:refnum<queue>)  [unwired: 2 in, 2 out]
                }
              }
            }
          }
          frame "Task 6C: PROCESS IMAGE" {
            # "Ball > Soap > Gel > Pipe"
            # ">>> Motor control cluster >>>"
            # ">>> yStepper command>>>"
            n533 = Dequeue Element(queue=w1452, timeout in ms (-1)=w1451, error in (no error)=w1450) -> (element=w1449:T10)  [unwired: 3 out]
            n534 = case shown="\"Start Task 1\", Default" w1449 {
              tunnel: [w1468 State_Type_Definitions,_for_0.26g_versions_and_later_3."True Stop" ("Enum")] -> w1456
              tunnel: [w1470 w1487] -> w1455
              tunnel: [State_Type_Definitions,_for_0.26g_versions_and_later_3."Idle" ("Enum") State_Type_Definitions,_for_0.26g_versions_and_later_3."Shutdown" ("Enum")] -> w1457
              tunnel: w1453 -> [w1459 _]
              tunnel: w1454 -> [w1465 w1484]
              tunnel: w1445 -> [w1463 _]
              tunnel: w1444 -> [w1464 _]
              frame "Start Task 1", Default {
                # "Stays in Task 5D until the object is detected"
                n535 = Or(x=w1463, y=w1459) -> (x .or. y?=w1462:bool)
                n536 = case shown="True" w1462 {
                  tunnel: [w1474 w1480] -> w1470
                  tunnel: w1465 -> [w1472 w1478]
                  frame False {
                    n537 = for {
                      tunnel: string[] ["START TIMER", "PROCESS IMAGE", ""] ("element") -> [w1475] mode=indexing
                      shift-right: [w1477] -> w1474
                      shift-left: w1472 -> [w1476]
                      n538 = Enqueue Element(queue=w1476, element=w1475) -> (queue out=w1477:refnum<queue>)  [unwired: 2 in, 2 out]
                    }
                  }
                  frame True {
                    n539 = for {
                      shift-right: [w1482] -> w1480
                      shift-left: w1478 -> [w1483]
                      tunnel: string[] ["RESET ENCODERS", "RESET YAW", ""] -> [w1481] mode=indexing
                      n540 = Enqueue Element(queue=w1483, element=w1481) -> (queue out=w1482:refnum<queue>)  [unwired: 2 in, 2 out]
                    }
                  }
                }
                n541 = Select(t=State_Type_Definitions,_for_0.26g_versions_and_later_3."Task 6D: BALL BUSTER" ("Enum"), s=w1464, f=State_Type_Definitions,_for_0.26g_versions_and_later_3."Task 6F: CAM BURST 2" ("Enum")) -> (s? t:f=w1460:T18)
                n542 = Select(t=State_Type_Definitions,_for_0.26g_versions_and_later_3."True Stop" ("Enum"), s=w1459, f=w1460) -> (s? t:f=w1466:T18)
                n543 = Select(t=w1466, s=w1462, f=State_Type_Definitions,_for_0.26g_versions_and_later_3."Task 6C: PROCESS IMAGE" ("Enum")) -> (s? t:f=w1468:T18)
              }
              frame "Exit" {
                n544 = for {
                  shift-right: [w1490] -> w1487
                  shift-left: w1484 -> [w1491]
                  tunnel: string[] ["STOP", "RESET ENCODERS", "RESET YAW", "ARDUINO MODE 0"] -> [w1489] mode=indexing
                  n545 = Enqueue Element(queue=w1491, element=w1489) -> (queue out=w1490:refnum<queue>)  [unwired: 2 in, 2 out]
                }
              }
            }
          }
          frame "Task 6D: BALL BUSTER" {
            # "Ball > Soap > Gel > Pipe"
            # ">>> Motor control cluster >>>"
            # ">>> yStepper command>>>"
            n546 = Greater Or Equal?(x=w1492, y=20.0) -> (x >= y?=w1493:bool)
            n547 = Dequeue Element(queue=w1501, timeout in ms (-1)=w1500, error in (no error)=w1499) -> (element=w1498:T10)  [unwired: 3 out]
            n548 = case shown="\"Start Task 1\", Default" w1498 {
              tunnel: [w1514 State_Type_Definitions,_for_0.26g_versions_and_later_3."True Stop" ("Enum")] -> w1505
              tunnel: [w1516 w1533] -> w1504
              tunnel: [State_Type_Definitions,_for_0.26g_versions_and_later_3."Idle" ("Enum") State_Type_Definitions,_for_0.26g_versions_and_later_3."Shutdown" ("Enum")] -> w1506
              tunnel: w1502 -> [w1509 _]
              tunnel: w1503 -> [w1511 w1530]
              tunnel: w1493 -> [w1508 _]
              frame "Start Task 1", Default {
                # "Stays in Task 5D until the object is detected"
                n549 = Or(x=w1508, y=w1509) -> (x .or. y?=w1510:bool)
                n550 = case shown="False" w1510 {
                  tunnel: [w1520 w1526] -> w1516
                  tunnel: w1511 -> [w1518 w1524]
                  frame False {
                    n551 = for {
                      tunnel: string[] ["RIGHT", "READ NAVX", "READ ENCODERS"] ("element") -> [w1521] mode=indexing
                      shift-right: [w1523] -> w1520
                      shift-left: w1518 -> [w1522]
                      n552 = Enqueue Element(queue=w1522, element=w1521) -> (queue out=w1523:refnum<queue>)  [unwired: 2 in, 2 out]
                    }
                  }
                  frame True {
                    n553 = for {
                      shift-right: [w1528] -> w1526
                      shift-left: w1524 -> [w1529]
                      tunnel: string[] ["RESET ENCODERS", "RESET YAW", "RESET FLAGS"] -> [w1527] mode=indexing
                      n554 = Enqueue Element(queue=w1529, element=w1527) -> (queue out=w1528:refnum<queue>)  [unwired: 2 in, 2 out]
                    }
                  }
                }
                n555 = Select(t=State_Type_Definitions,_for_0.26g_versions_and_later_3."True Stop" ("Enum"), s=w1509, f=State_Type_Definitions,_for_0.26g_versions_and_later_3."Task 6E: STILL WAITING" ("Enum")) -> (s? t:f=w1512:T18)
                n556 = Select(t=w1512, s=w1510, f=State_Type_Definitions,_for_0.26g_versions_and_later_3."Task 6D: BALL BUSTER" ("Enum")) -> (s? t:f=w1514:T18)
              }
              frame "Exit" {
                n557 = for {
                  shift-right: [w1536] -> w1533
                  shift-left: w1530 -> [w1537]
                  tunnel: string[] ["STOP", "RESET ENCODERS", "RESET YAW", "ARDUINO MODE 0"] -> [w1535] mode=indexing
                  n558 = Enqueue Element(queue=w1537, element=w1535) -> (queue out=w1536:refnum<queue>)  [unwired: 2 in, 2 out]
                }
              }
            }
          }
          frame "Task 6E: STILL WAITING" {
            # "Ball > Soap > Gel > Pipe"
            # ">>> Motor control cluster >>>"
            # ">>> yStepper command>>>"
            n559 = local read "Rising Edge"() -> (w1539:bool)
            n560 = Dequeue Element(queue=w1545, timeout in ms (-1)=w1544, error in (no error)=w1543) -> (element=w1542:T10)  [unwired: 3 out]
            n561 = case shown="\"Start Task 1\", Default" w1542 {
              tunnel: [w1559 State_Type_Definitions,_for_0.26g_versions_and_later_3."True Stop" ("Enum")] -> w1549
              tunnel: [w1552 w1577] -> w1548
              tunnel: [State_Type_Definitions,_for_0.26g_versions_and_later_3."Idle" ("Enum") State_Type_Definitions,_for_0.26g_versions_and_later_3."Shutdown" ("Enum")] -> w1550
              tunnel: w1546 -> [w1556 _]
              tunnel: w1547 -> [w1553 w1574]
              tunnel: w1539 -> [w1554 _]
              frame "Start Task 1", Default {
                # "Stays in Task 5D until the object is detected"
                n562 = Or(x=w1554, y=w1556) -> (x .or. y?=w1551:bool)
                n563 = case shown="False" w1551 {
                  tunnel: [w1564 w1570] -> w1552
                  tunnel: w1553 -> [w1562 w1569]
                  frame False {
                    n564 = for {
                      tunnel: string[] ["Z STEPPER CAM HEIGHT", "READ STEPPER VALUES"] ("element") -> [w1565] mode=indexing
                      shift-right: [w1567] -> w1564
                      shift-left: w1562 -> [w1566]
                      n565 = Enqueue Element(queue=w1566, element=w1565) -> (queue out=w1567:refnum<queue>)  [unwired: 2 in, 2 out]
                    }
                  }
                  frame True {
                    n566 = for {
                      shift-right: [w1572] -> w1570
                      shift-left: w1569 -> [w1573]
                      tunnel: string[] ["OPEN LOG CAM", "SET TIMER 2", "OPEN IMAQ REF", "", ""] -> [w1571] mode=indexing
                      n567 = Enqueue Element(queue=w1573, element=w1571) -> (queue out=w1572:refnum<queue>)  [unwired: 2 in, 2 out]
                    }
                  }
                }
                n568 = Select(t=State_Type_Definitions,_for_0.26g_versions_and_later_3."True Stop" ("Enum"), s=w1556, f=State_Type_Definitions,_for_0.26g_versions_and_later_3."Task 6F: CAM BURST 2" ("Enum")) -> (s? t:f=w1557:T18)
                n569 = Select(t=w1557, s=w1551, f=State_Type_Definitions,_for_0.26g_versions_and_later_3."Task 6E: STILL WAITING" ("Enum")) -> (s? t:f=w1559:T18)
              }
              frame "Exit" {
                n570 = for {
                  shift-right: [w1580] -> w1577
                  shift-left: w1574 -> [w1581]
                  tunnel: string[] ["STOP", "RESET ENCODERS", "RESET YAW", "ARDUINO MODE 0"] -> [w1579] mode=indexing
                  n571 = Enqueue Element(queue=w1581, element=w1579) -> (queue out=w1580:refnum<queue>)  [unwired: 2 in, 2 out]
                }
              }
            }
          }
          frame "Task 6F: CAM BURST 2" {
            # ">> Manual override >>"
            # ">>> Motor control cluster >>>"
            # ">>> yStepper command>>>"
            n572 = Dequeue Element(queue=w1593, timeout in ms (-1)=w1591, error in (no error)=w1592) -> (element=w1590:T10)  [unwired: 3 out]
            n573 = case shown="\"Start Task 1\", Default" w1590 {
              tunnel: [w1601 State_Type_Definitions,_for_0.26g_versions_and_later_3."True Stop" ("Enum")] -> w1587
              tunnel: [w1599 w1619] -> w1594
              tunnel: [State_Type_Definitions,_for_0.26g_versions_and_later_3."Idle" ("Enum") State_Type_Definitions,_for_0.26g_versions_and_later_3."Shutdown" ("Enum")] -> w1588
              tunnel: w1589 -> [w1597 _]
              tunnel: w1586 -> [w1598 w1616]
              tunnel: w1582 -> [w1595 _]
              frame "Start Task 1", Default {
                n574 = Or(x=w1595, y=w1597) -> (x .or. y?=w1596:bool)
                n575 = case shown="True" w1596 {
                  tunnel: [w1606 w1612] -> w1599
                  tunnel: w1598 -> [w1604 w1610]
                  frame False {
                    n576 = for {
                      tunnel: string[] ["CAM ACQ", "START TIMER"] ("element") -> [w1607] mode=indexing
                      shift-right: [w1609] -> w1606
                      shift-left: w1604 -> [w1608]
                      n577 = Enqueue Element(queue=w1608, element=w1607) -> (queue out=w1609:refnum<queue>)  [unwired: 2 in, 2 out]
                    }
                  }
                  frame True {
                    n578 = for {
                      shift-right: [w1614] -> w1612
                      shift-left: w1610 -> [w1615]
                      tunnel: string[] ["CAM CLOSE", "PROCESS IMAGE", "SET TIMER 2", "RESET ENCODERS"] -> [w1613] mode=indexing
                      n579 = Enqueue Element(queue=w1615, element=w1613) -> (queue out=w1614:refnum<queue>)  [unwired: 2 in, 2 out]
                    }
                  }
                }
                n580 = Select(t=State_Type_Definitions,_for_0.26g_versions_and_later_3."Task 6G: PROCESS IMAGE 2" ("Enum"), s=w1596, f=State_Type_Definitions,_for_0.26g_versions_and_later_3."Task 6F: CAM BURST 2" ("Enum")) -> (s? t:f=w1601:T18)
              }
              frame "Exit" {
                # ">> State after true stop >>"
                # ">> Goes to true stop >>"
                n581 = for {
                  shift-right: [w1622] -> w1619
                  shift-left: w1616 -> [w1623]
                  tunnel: string[] ["STOP", "RESET ENCODERS", "RESET YAW", ""] -> [w1621] mode=indexing
                  n582 = Enqueue Element(queue=w1623, element=w1621) -> (queue out=w1622:refnum<queue>)  [unwired: 2 in, 2 out]
                }
              }
            }
          }
          frame "Task 6G: PROCESS IMAGE 2" {
            # "Ball > Soap > Gel > Pipe"
            # ">>> Motor control cluster >>>"
            # ">>> yStepper command>>>"
            n583 = Dequeue Element(queue=w1632, timeout in ms (-1)=w1631, error in (no error)=w1630) -> (element=w1629:T10)  [unwired: 3 out]
            n584 = case shown="\"Start Task 1\", Default" w1629 {
              tunnel: [w1648 State_Type_Definitions,_for_0.26g_versions_and_later_3."True Stop" ("Enum")] -> w1636
              tunnel: [w1650 w1667] -> w1635
              tunnel: [State_Type_Definitions,_for_0.26g_versions_and_later_3."Idle" ("Enum") State_Type_Definitions,_for_0.26g_versions_and_later_3."Shutdown" ("Enum")] -> w1637
              tunnel: w1633 -> [w1639 _]
              tunnel: w1634 -> [w1645 w1664]
              tunnel: w1625 -> [w1643 _]
              tunnel: w1624 -> [w1644 _]
              frame "Start Task 1", Default {
                # "Stays in Task 5D until the object is detected"
                n585 = Or(x=w1643, y=w1639) -> (x .or. y?=w1642:bool)
                n586 = case shown="True" w1642 {
                  tunnel: [w1654 w1660] -> w1650
                  tunnel: w1645 -> [w1652 w1658]
                  frame False {
                    n587 = for {
                      tunnel: string[] ["START TIMER", "PROCESS IMAGE", ""] ("element") -> [w1655] mode=indexing
                      shift-right: [w1657] -> w1654
                      shift-left: w1652 -> [w1656]
                      n588 = Enqueue Element(queue=w1656, element=w1655) -> (queue out=w1657:refnum<queue>)  [unwired: 2 in, 2 out]
                    }
                  }
                  frame True {
                    n589 = for {
                      shift-right: [w1662] -> w1660
                      shift-left: w1658 -> [w1663]
                      tunnel: string[] ["RESET ENCODERS", "RESET YAW", ""] -> [w1661] mode=indexing
                      n590 = Enqueue Element(queue=w1663, element=w1661) -> (queue out=w1662:refnum<queue>)  [unwired: 2 in, 2 out]
                    }
                  }
                }
                n591 = Select(t=State_Type_Definitions,_for_0.26g_versions_and_later_3."Task 6H: SKADI SOAPS" ("Enum"), s=w1644, f=State_Type_Definitions,_for_0.26g_versions_and_later_3."Task 6J: CAM BURST 3" ("Enum")) -> (s? t:f=w1640:T18)
                n592 = Select(t=State_Type_Definitions,_for_0.26g_versions_and_later_3."True Stop" ("Enum"), s=w1639, f=w1640) -> (s? t:f=w1646:T18)
                n593 = Select(t=w1646, s=w1642, f=State_Type_Definitions,_for_0.26g_versions_and_later_3."Task 6G: PROCESS IMAGE 2" ("Enum")) -> (s? t:f=w1648:T18)
              }
              frame "Exit" {
                n594 = for {
                  shift-right: [w1670] -> w1667
                  shift-left: w1664 -> [w1671]
                  tunnel: string[] ["STOP", "RESET ENCODERS", "RESET YAW", "ARDUINO MODE 0"] -> [w1669] mode=indexing
                  n595 = Enqueue Element(queue=w1671, element=w1669) -> (queue out=w1670:refnum<queue>)  [unwired: 2 in, 2 out]
                }
              }
            }
          }
          frame "Task 6H: SKADI SOAPS" {
            # "Ball > Soap > Gel > Pipe"
            # ">>> Motor control cluster >>>"
            # ">>> yStepper command>>>"
            n596 = Less Or Equal?(x=w1672, y=-20.0) -> (x <= y?=w1673:bool)
            n597 = Dequeue Element(queue=w1681, timeout in ms (-1)=w1680, error in (no error)=w1679) -> (element=w1678:T10)  [unwired: 3 out]
            n598 = case shown="\"Start Task 1\", Default" w1678 {
              tunnel: [w1694 State_Type_Definitions,_for_0.26g_versions_and_later_3."True Stop" ("Enum")] -> w1685
              tunnel: [w1696 w1713] -> w1684
              tunnel: [State_Type_Definitions,_for_0.26g_versions_and_later_3."Idle" ("Enum") State_Type_Definitions,_for_0.26g_versions_and_later_3."Shutdown" ("Enum")] -> w1686
              tunnel: w1682 -> [w1689 _]
              tunnel: w1683 -> [w1691 w1710]
              tunnel: w1673 -> [w1688 _]
              frame "Start Task 1", Default {
                # "Stays in Task 5D until the object is detected"
                n599 = Or(x=w1688, y=w1689) -> (x .or. y?=w1690:bool)
                n600 = case shown="False" w1690 {
                  tunnel: [w1700 w1706] -> w1696
                  tunnel: w1691 -> [w1698 w1704]
                  frame False {
                    n601 = for {
                      tunnel: string[] ["LEFT", "READ NAVX", "READ ENCODERS"] ("element") -> [w1701] mode=indexing
                      shift-right: [w1703] -> w1700
                      shift-left: w1698 -> [w1702]
                      n602 = Enqueue Element(queue=w1702, element=w1701) -> (queue out=w1703:refnum<queue>)  [unwired: 2 in, 2 out]
                    }
                  }
                  frame True {
                    n603 = for {
                      shift-right: [w1708] -> w1706
                      shift-left: w1704 -> [w1709]
                      tunnel: string[] ["RESET ENCODERS", "RESET YAW", "RESET FLAGS"] -> [w1707] mode=indexing
                      n604 = Enqueue Element(queue=w1709, element=w1707) -> (queue out=w1708:refnum<queue>)  [unwired: 2 in, 2 out]
                    }
                  }
                }
                n605 = Select(t=State_Type_Definitions,_for_0.26g_versions_and_later_3."True Stop" ("Enum"), s=w1689, f=State_Type_Definitions,_for_0.26g_versions_and_later_3."Task 6I: STILL WAITING 2" ("Enum")) -> (s? t:f=w1692:T18)
                n606 = Select(t=w1692, s=w1690, f=State_Type_Definitions,_for_0.26g_versions_and_later_3."Task 6H: SKADI SOAPS" ("Enum")) -> (s? t:f=w1694:T18)
              }
              frame "Exit" {
                n607 = for {
                  shift-right: [w1716] -> w1713
                  shift-left: w1710 -> [w1717]
                  tunnel: string[] ["STOP", "RESET ENCODERS", "RESET YAW", "ARDUINO MODE 0"] -> [w1715] mode=indexing
                  n608 = Enqueue Element(queue=w1717, element=w1715) -> (queue out=w1716:refnum<queue>)  [unwired: 2 in, 2 out]
                }
              }
            }
          }
          frame "Task 6I: STILL WAITING 2" {
            # "Ball > Soap > Gel > Pipe"
            # ">>> Motor control cluster >>>"
            # ">>> yStepper command>>>"
            n609 = local read "Rising Edge"() -> (w1719:bool)
            n610 = Dequeue Element(queue=w1725, timeout in ms (-1)=w1724, error in (no error)=w1723) -> (element=w1722:T10)  [unwired: 3 out]
            n611 = case shown="\"Start Task 1\", Default" w1722 {
              tunnel: [w1739 State_Type_Definitions,_for_0.26g_versions_and_later_3."True Stop" ("Enum")] -> w1729
              tunnel: [w1732 w1757] -> w1728
              tunnel: [State_Type_Definitions,_for_0.26g_versions_and_later_3."Idle" ("Enum") State_Type_Definitions,_for_0.26g_versions_and_later_3."Shutdown" ("Enum")] -> w1730
              tunnel: w1726 -> [w1736 _]
              tunnel: w1727 -> [w1733 w1754]
              tunnel: w1719 -> [w1734 _]
              frame "Start Task 1", Default {
                # "Stays in Task 5D until the object is detected"
                n612 = Or(x=w1734, y=w1736) -> (x .or. y?=w1731:bool)
                n613 = case shown="False" w1731 {
                  tunnel: [w1744 w1750] -> w1732
                  tunnel: w1733 -> [w1742 w1749]
                  frame False {
                    n614 = for {
                      tunnel: string[] ["Z STEPPER CAM HEIGHT", "READ STEPPER VALUES"] ("element") -> [w1745] mode=indexing
                      shift-right: [w1747] -> w1744
                      shift-left: w1742 -> [w1746]
                      n615 = Enqueue Element(queue=w1746, element=w1745) -> (queue out=w1747:refnum<queue>)  [unwired: 2 in, 2 out]
                    }
                  }
                  frame True {
                    n616 = for {
                      shift-right: [w1752] -> w1750
                      shift-left: w1749 -> [w1753]
                      tunnel: string[] ["OPEN LOG CAM", "SET TIMER 2", "OPEN IMAQ REF", "", ""] -> [w1751] mode=indexing
                      n617 = Enqueue Element(queue=w1753, element=w1751) -> (queue out=w1752:refnum<queue>)  [unwired: 2 in, 2 out]
                    }
                  }
                }
                n618 = Select(t=State_Type_Definitions,_for_0.26g_versions_and_later_3."True Stop" ("Enum"), s=w1736, f=State_Type_Definitions,_for_0.26g_versions_and_later_3."Task 6J: CAM BURST 3" ("Enum")) -> (s? t:f=w1737:T18)
                n619 = Select(t=w1737, s=w1731, f=State_Type_Definitions,_for_0.26g_versions_and_later_3."Task 6I: STILL WAITING 2" ("Enum")) -> (s? t:f=w1739:T18)
              }
              frame "Exit" {
                n620 = for {
                  shift-right: [w1760] -> w1757
                  shift-left: w1754 -> [w1761]
                  tunnel: string[] ["STOP", "RESET ENCODERS", "RESET YAW", "ARDUINO MODE 0"] -> [w1759] mode=indexing
                  n621 = Enqueue Element(queue=w1761, element=w1759) -> (queue out=w1760:refnum<queue>)  [unwired: 2 in, 2 out]
                }
              }
            }
          }
          frame "Task 6J: CAM BURST 3" {
            # ">> Manual override >>"
            # ">>> Motor control cluster >>>"
            # ">>> yStepper command>>>"
            n622 = Dequeue Element(queue=w1773, timeout in ms (-1)=w1771, error in (no error)=w1772) -> (element=w1770:T10)  [unwired: 3 out]
            n623 = case shown="\"Start Task 1\", Default" w1770 {
              tunnel: [w1781 State_Type_Definitions,_for_0.26g_versions_and_later_3."True Stop" ("Enum")] -> w1767
              tunnel: [w1779 w1799] -> w1774
              tunnel: [State_Type_Definitions,_for_0.26g_versions_and_later_3."Idle" ("Enum") State_Type_Definitions,_for_0.26g_versions_and_later_3."Shutdown" ("Enum")] -> w1768
              tunnel: w1769 -> [w1777 _]
              tunnel: w1766 -> [w1778 w1796]
              tunnel: w1762 -> [w1775 _]
              frame "Start Task 1", Default {
                n624 = Or(x=w1775, y=w1777) -> (x .or. y?=w1776:bool)
                n625 = case shown="True" w1776 {
                  tunnel: [w1786 w1792] -> w1779
                  tunnel: w1778 -> [w1784 w1790]
                  frame False {
                    n626 = for {
                      tunnel: string[] ["CAM ACQ", "START TIMER"] ("element") -> [w1787] mode=indexing
                      shift-right: [w1789] -> w1786
                      shift-left: w1784 -> [w1788]
                      n627 = Enqueue Element(queue=w1788, element=w1787) -> (queue out=w1789:refnum<queue>)  [unwired: 2 in, 2 out]
                    }
                  }
                  frame True {
                    n628 = for {
                      shift-right: [w1794] -> w1792
                      shift-left: w1790 -> [w1795]
                      tunnel: string[] ["CAM CLOSE", "PROCESS IMAGE", "SET TIMER 2", "RESET ENCODERS"] -> [w1793] mode=indexing
                      n629 = Enqueue Element(queue=w1795, element=w1793) -> (queue out=w1794:refnum<queue>)  [unwired: 2 in, 2 out]
                    }
                  }
                }
                n630 = Select(t=State_Type_Definitions,_for_0.26g_versions_and_later_3."Task 6K: PROCESS IMAGE 3" ("Enum"), s=w1776, f=State_Type_Definitions,_for_0.26g_versions_and_later_3."Task 6J: CAM BURST 3" ("Enum")) -> (s? t:f=w1781:T18)
              }
              frame "Exit" {
                # ">> State after true stop >>"
                # ">> Goes to true stop >>"
                n631 = for {
                  shift-right: [w1802] -> w1799
                  shift-left: w1796 -> [w1803]
                  tunnel: string[] ["STOP", "RESET ENCODERS", "RESET YAW", ""] -> [w1801] mode=indexing
                  n632 = Enqueue Element(queue=w1803, element=w1801) -> (queue out=w1802:refnum<queue>)  [unwired: 2 in, 2 out]
                }
              }
            }
          }
          frame "Task 6K: PROCESS IMAGE 3" {
            # "Ball > Soap > Gel > Pipe"
            # ">>> Motor control cluster >>>"
            # ">>> yStepper command>>>"
            n633 = Dequeue Element(queue=w1812, timeout in ms (-1)=w1811, error in (no error)=w1810) -> (element=w1809:T10)  [unwired: 3 out]
            n634 = case shown="\"Start Task 1\", Default" w1809 {
              tunnel: [w1828 State_Type_Definitions,_for_0.26g_versions_and_later_3."True Stop" ("Enum")] -> w1816
              tunnel: [w1830 w1847] -> w1815
              tunnel: [State_Type_Definitions,_for_0.26g_versions_and_later_3."Idle" ("Enum") State_Type_Definitions,_for_0.26g_versions_and_later_3."Shutdown" ("Enum")] -> w1817
              tunnel: w1813 -> [w1819 _]
              tunnel: w1814 -> [w1825 w1844]
              tunnel: w1805 -> [w1823 _]
              tunnel: w1804 -> [w1824 _]
              frame "Start Task 1", Default {
                # "Stays in Task 5D until the object is detected"
                n635 = Or(x=w1823, y=w1819) -> (x .or. y?=w1822:bool)
                n636 = case shown="True" w1822 {
                  tunnel: [w1834 w1840] -> w1830
                  tunnel: w1825 -> [w1832 w1838]
                  frame False {
                    n637 = for {
                      tunnel: string[] ["START TIMER", "PROCESS IMAGE", ""] ("element") -> [w1835] mode=indexing
                      shift-right: [w1837] -> w1834
                      shift-left: w1832 -> [w1836]
                      n638 = Enqueue Element(queue=w1836, element=w1835) -> (queue out=w1837:refnum<queue>)  [unwired: 2 in, 2 out]
                    }
                  }
                  frame True {
                    n639 = for {
                      shift-right: [w1842] -> w1840
                      shift-left: w1838 -> [w1843]
                      tunnel: string[] ["RESET ENCODERS", "RESET YAW", ""] -> [w1841] mode=indexing
                      n640 = Enqueue Element(queue=w1843, element=w1841) -> (queue out=w1842:refnum<queue>)  [unwired: 2 in, 2 out]
                    }
                  }
                }
                n641 = Select(t=State_Type_Definitions,_for_0.26g_versions_and_later_3."Task 6L: JAM IT IN" ("Enum"), s=w1824, f=State_Type_Definitions,_for_0.26g_versions_and_later_3."Task 6N: CAM BURST 4" ("Enum")) -> (s? t:f=w1820:T18)
                n642 = Select(t=State_Type_Definitions,_for_0.26g_versions_and_later_3."True Stop" ("Enum"), s=w1819, f=w1820) -> (s? t:f=w1826:T18)
                n643 = Select(t=w1826, s=w1822, f=State_Type_Definitions,_for_0.26g_versions_and_later_3."Task 6K: PROCESS IMAGE 3" ("Enum")) -> (s? t:f=w1828:T18)
              }
              frame "Exit" {
                n644 = for {
                  shift-right: [w1850] -> w1847
                  shift-left: w1844 -> [w1851]
                  tunnel: string[] ["STOP", "RESET ENCODERS", "RESET YAW", "ARDUINO MODE 0"] -> [w1849] mode=indexing
                  n645 = Enqueue Element(queue=w1851, element=w1849) -> (queue out=w1850:refnum<queue>)  [unwired: 2 in, 2 out]
                }
              }
            }
          }
          frame "Task 6L: JAM IT IN" {
            # "Ball > Soap > Gel > Pipe"
            # ">>> Motor control cluster >>>"
            # ">>> yStepper command>>>"
            n646 = Less Or Equal?(x=w1852, y=-20.0) -> (x <= y?=w1853:bool)
            n647 = Dequeue Element(queue=w1861, timeout in ms (-1)=w1860, error in (no error)=w1859) -> (element=w1858:T10)  [unwired: 3 out]
            n648 = case shown="\"Start Task 1\", Default" w1858 {
              tunnel: [w1874 State_Type_Definitions,_for_0.26g_versions_and_later_3."True Stop" ("Enum")] -> w1865
              tunnel: [w1876 w1893] -> w1864
              tunnel: [State_Type_Definitions,_for_0.26g_versions_and_later_3."Idle" ("Enum") State_Type_Definitions,_for_0.26g_versions_and_later_3."Shutdown" ("Enum")] -> w1866
              tunnel: w1862 -> [w1869 _]
              tunnel: w1863 -> [w1871 w1890]
              tunnel: w1853 -> [w1868 _]
              frame "Start Task 1", Default {
                # "Stays in Task 5D until the object is detected"
                n649 = Or(x=w1868, y=w1869) -> (x .or. y?=w1870:bool)
                n650 = case shown="False" w1870 {
                  tunnel: [w1880 w1886] -> w1876
                  tunnel: w1871 -> [w1878 w1884]
                  frame False {
                    n651 = for {
                      tunnel: string[] ["REVERSE", "READ NAVX", "READ ENCODERS"] ("element") -> [w1881] mode=indexing
                      shift-right: [w1883] -> w1880
                      shift-left: w1878 -> [w1882]
                      n652 = Enqueue Element(queue=w1882, element=w1881) -> (queue out=w1883:refnum<queue>)  [unwired: 2 in, 2 out]
                    }
                  }
                  frame True {
                    n653 = for {
                      shift-right: [w1888] -> w1886
                      shift-left: w1884 -> [w1889]
                      tunnel: string[] ["RESET ENCODERS", "RESET YAW", "RESET FLAGS"] -> [w1887] mode=indexing
                      n654 = Enqueue Element(queue=w1889, element=w1887) -> (queue out=w1888:refnum<queue>)  [unwired: 2 in, 2 out]
                    }
                  }
                }
                n655 = Select(t=State_Type_Definitions,_for_0.26g_versions_and_later_3."True Stop" ("Enum"), s=w1869, f=State_Type_Definitions,_for_0.26g_versions_and_later_3."Task 6M: STILL WAITING 3" ("Enum")) -> (s? t:f=w1872:T18)
                n656 = Select(t=w1872, s=w1870, f=State_Type_Definitions,_for_0.26g_versions_and_later_3."Task 6L: JAM IT IN" ("Enum")) -> (s? t:f=w1874:T18)
              }
              frame "Exit" {
                n657 = for {
                  shift-right: [w1896] -> w1893
                  shift-left: w1890 -> [w1897]
                  tunnel: string[] ["STOP", "RESET ENCODERS", "RESET YAW", "ARDUINO MODE 0"] -> [w1895] mode=indexing
                  n658 = Enqueue Element(queue=w1897, element=w1895) -> (queue out=w1896:refnum<queue>)  [unwired: 2 in, 2 out]
                }
              }
            }
          }
          frame "Task 6M: STILL WAITING 3" {
            # "Ball > Soap > Gel > Pipe"
            # ">>> Motor control cluster >>>"
            # ">>> yStepper command>>>"
            n659 = local read "Rising Edge"() -> (w1899:bool)
            n660 = Dequeue Element(queue=w1905, timeout in ms (-1)=w1904, error in (no error)=w1903) -> (element=w1902:T10)  [unwired: 3 out]
            n661 = case shown="\"Start Task 1\", Default" w1902 {
              tunnel: [w1919 State_Type_Definitions,_for_0.26g_versions_and_later_3."True Stop" ("Enum")] -> w1909
              tunnel: [w1912 w1937] -> w1908
              tunnel: [State_Type_Definitions,_for_0.26g_versions_and_later_3."Idle" ("Enum") State_Type_Definitions,_for_0.26g_versions_and_later_3."Shutdown" ("Enum")] -> w1910
              tunnel: w1906 -> [w1916 _]
              tunnel: w1907 -> [w1913 w1934]
              tunnel: w1899 -> [w1914 _]
              frame "Start Task 1", Default {
                # "Stays in Task 5D until the object is detected"
                n662 = Or(x=w1914, y=w1916) -> (x .or. y?=w1911:bool)
                n663 = case shown="False" w1911 {
                  tunnel: [w1924 w1930] -> w1912
                  tunnel: w1913 -> [w1922 w1929]
                  frame False {
                    n664 = for {
                      tunnel: string[] ["Z STEPPER CAM HEIGHT", "READ STEPPER VALUES"] ("element") -> [w1925] mode=indexing
                      shift-right: [w1927] -> w1924
                      shift-left: w1922 -> [w1926]
                      n665 = Enqueue Element(queue=w1926, element=w1925) -> (queue out=w1927:refnum<queue>)  [unwired: 2 in, 2 out]
                    }
                  }
                  frame True {
                    n666 = for {
                      shift-right: [w1932] -> w1930
                      shift-left: w1929 -> [w1933]
                      tunnel: string[] ["OPEN LOG CAM", "SET TIMER 2", "OPEN IMAQ REF", "", ""] -> [w1931] mode=indexing
                      n667 = Enqueue Element(queue=w1933, element=w1931) -> (queue out=w1932:refnum<queue>)  [unwired: 2 in, 2 out]
                    }
                  }
                }
                n668 = Select(t=State_Type_Definitions,_for_0.26g_versions_and_later_3."True Stop" ("Enum"), s=w1916, f=State_Type_Definitions,_for_0.26g_versions_and_later_3."Task 6N: CAM BURST 4" ("Enum")) -> (s? t:f=w1917:T18)
                n669 = Select(t=w1917, s=w1911, f=State_Type_Definitions,_for_0.26g_versions_and_later_3."Task 6M: STILL WAITING 3" ("Enum")) -> (s? t:f=w1919:T18)
              }
              frame "Exit" {
                n670 = for {
                  shift-right: [w1940] -> w1937
                  shift-left: w1934 -> [w1941]
                  tunnel: string[] ["STOP", "RESET ENCODERS", "RESET YAW", "ARDUINO MODE 0"] -> [w1939] mode=indexing
                  n671 = Enqueue Element(queue=w1941, element=w1939) -> (queue out=w1940:refnum<queue>)  [unwired: 2 in, 2 out]
                }
              }
            }
          }
          frame "Task 6N: CAM BURST 4" {
            # ">> Manual override >>"
            # ">>> Motor control cluster >>>"
            # ">>> yStepper command>>>"
            n672 = Dequeue Element(queue=w1953, timeout in ms (-1)=w1951, error in (no error)=w1952) -> (element=w1950:T10)  [unwired: 3 out]
            n673 = case shown="\"Start Task 1\", Default" w1950 {
              tunnel: [w1961 State_Type_Definitions,_for_0.26g_versions_and_later_3."True Stop" ("Enum")] -> w1947
              tunnel: [w1959 w1979] -> w1954
              tunnel: [State_Type_Definitions,_for_0.26g_versions_and_later_3."Idle" ("Enum") State_Type_Definitions,_for_0.26g_versions_and_later_3."Shutdown" ("Enum")] -> w1948
              tunnel: w1949 -> [w1957 _]
              tunnel: w1946 -> [w1958 w1976]
              tunnel: w1942 -> [w1955 _]
              frame "Start Task 1", Default {
                n674 = Or(x=w1955, y=w1957) -> (x .or. y?=w1956:bool)
                n675 = case shown="True" w1956 {
                  tunnel: [w1966 w1972] -> w1959
                  tunnel: w1958 -> [w1964 w1970]
                  frame False {
                    n676 = for {
                      tunnel: string[] ["CAM ACQ", "START TIMER"] ("element") -> [w1967] mode=indexing
                      shift-right: [w1969] -> w1966
                      shift-left: w1964 -> [w1968]
                      n677 = Enqueue Element(queue=w1968, element=w1967) -> (queue out=w1969:refnum<queue>)  [unwired: 2 in, 2 out]
                    }
                  }
                  frame True {
                    n678 = for {
                      shift-right: [w1974] -> w1972
                      shift-left: w1970 -> [w1975]
                      tunnel: string[] ["CAM CLOSE", "PROCESS IMAGE", "SET TIMER 2", "RESET ENCODERS"] -> [w1973] mode=indexing
                      n679 = Enqueue Element(queue=w1975, element=w1973) -> (queue out=w1974:refnum<queue>)  [unwired: 2 in, 2 out]
                    }
                  }
                }
                n680 = Select(t=State_Type_Definitions,_for_0.26g_versions_and_later_3."Task 6O: PROCESS IMAGE 4" ("Enum"), s=w1956, f=State_Type_Definitions,_for_0.26g_versions_and_later_3."Task 6N: CAM BURST 4" ("Enum")) -> (s? t:f=w1961:T18)
              }
              frame "Exit" {
                # ">> State after true stop >>"
                # ">> Goes to true stop >>"
                n681 = for {
                  shift-right: [w1982] -> w1979
                  shift-left: w1976 -> [w1983]
                  tunnel: string[] ["STOP", "RESET ENCODERS", "RESET YAW", ""] -> [w1981] mode=indexing
                  n682 = Enqueue Element(queue=w1983, element=w1981) -> (queue out=w1982:refnum<queue>)  [unwired: 2 in, 2 out]
                }
              }
            }
          }
          frame "Task 6O: PROCESS IMAGE 4" {
            # "Ball > Soap > Gel > Pipe"
            # ">>> Motor control cluster >>>"
            # ">>> yStepper command>>>"
            n683 = Dequeue Element(queue=w1992, timeout in ms (-1)=w1991, error in (no error)=w1990) -> (element=w1989:T10)  [unwired: 3 out]
            n684 = case shown="\"Start Task 1\", Default" w1989 {
              tunnel: [w2008 State_Type_Definitions,_for_0.26g_versions_and_later_3."True Stop" ("Enum")] -> w1996
              tunnel: [w2010 w2027] -> w1995
              tunnel: [State_Type_Definitions,_for_0.26g_versions_and_later_3."Idle" ("Enum") State_Type_Definitions,_for_0.26g_versions_and_later_3."Shutdown" ("Enum")] -> w1997
              tunnel: w1993 -> [w1999 _]
              tunnel: w1994 -> [w2005 w2024]
              tunnel: w1985 -> [w2003 _]
              tunnel: w1984 -> [w2004 _]
              frame "Start Task 1", Default {
                # "Stays in Task 5D until the object is detected"
                n685 = Or(x=w2003, y=w1999) -> (x .or. y?=w2002:bool)
                n686 = case shown="True" w2002 {
                  tunnel: [w2014 w2020] -> w2010
                  tunnel: w2005 -> [w2012 w2018]
                  frame False {
                    n687 = for {
                      tunnel: string[] ["START TIMER", "PROCESS IMAGE", ""] ("element") -> [w2015] mode=indexing
                      shift-right: [w2017] -> w2014
                      shift-left: w2012 -> [w2016]
                      n688 = Enqueue Element(queue=w2016, element=w2015) -> (queue out=w2017:refnum<queue>)  [unwired: 2 in, 2 out]
                    }
                  }
                  frame True {
                    n689 = for {
                      shift-right: [w2022] -> w2020
                      shift-left: w2018 -> [w2023]
                      tunnel: string[] ["RESET ENCODERS", "RESET YAW", ""] -> [w2021] mode=indexing
                      n690 = Enqueue Element(queue=w2023, element=w2021) -> (queue out=w2022:refnum<queue>)  [unwired: 2 in, 2 out]
                    }
                  }
                }
                n691 = Select(t=State_Type_Definitions,_for_0.26g_versions_and_later_3."Task 6P: PIPE BOMB" ("Enum"), s=w2004, f=State_Type_Definitions,_for_0.26g_versions_and_later_3."Task 6B: CAM BURST" ("Enum")) -> (s? t:f=w2000:T18)
                n692 = Select(t=State_Type_Definitions,_for_0.26g_versions_and_later_3."True Stop" ("Enum"), s=w1999, f=w2000) -> (s? t:f=w2006:T18)
                n693 = Select(t=w2006, s=w2002, f=State_Type_Definitions,_for_0.26g_versions_and_later_3."Task 6O: PROCESS IMAGE 4" ("Enum")) -> (s? t:f=w2008:T18)
              }
              frame "Exit" {
                n694 = for {
                  shift-right: [w2030] -> w2027
                  shift-left: w2024 -> [w2031]
                  tunnel: string[] ["STOP", "RESET ENCODERS", "RESET YAW", "ARDUINO MODE 0"] -> [w2029] mode=indexing
                  n695 = Enqueue Element(queue=w2031, element=w2029) -> (queue out=w2030:refnum<queue>)  [unwired: 2 in, 2 out]
                }
              }
            }
          }
          frame "Task 6P: PIPE BOMB" {
            # "Ball > Soap > Gel > Pipe"
            # ">>> Motor control cluster >>>"
            # ">>> yStepper command>>>"
            n696 = Greater Or Equal?(x=w2032, y=20.0) -> (x >= y?=w2033:bool)
            n697 = Dequeue Element(queue=w2041, timeout in ms (-1)=w2040, error in (no error)=w2039) -> (element=w2038:T10)  [unwired: 3 out]
            n698 = case shown="\"Start Task 1\", Default" w2038 {
              tunnel: [w2054 State_Type_Definitions,_for_0.26g_versions_and_later_3."True Stop" ("Enum")] -> w2045
              tunnel: [w2056 w2073] -> w2044
              tunnel: [State_Type_Definitions,_for_0.26g_versions_and_later_3."Idle" ("Enum") State_Type_Definitions,_for_0.26g_versions_and_later_3."Shutdown" ("Enum")] -> w2046
              tunnel: w2042 -> [w2049 _]
              tunnel: w2043 -> [w2051 w2070]
              tunnel: w2033 -> [w2048 _]
              frame "Start Task 1", Default {
                # "Stays in Task 5D until the object is detected"
                n699 = Or(x=w2048, y=w2049) -> (x .or. y?=w2050:bool)
                n700 = case shown="False" w2050 {
                  tunnel: [w2060 w2066] -> w2056
                  tunnel: w2051 -> [w2058 w2064]
                  frame False {
                    n701 = for {
                      tunnel: string[] ["FORWARD", "READ NAVX", "READ ENCODERS"] ("element") -> [w2061] mode=indexing
                      shift-right: [w2063] -> w2060
                      shift-left: w2058 -> [w2062]
                      n702 = Enqueue Element(queue=w2062, element=w2061) -> (queue out=w2063:refnum<queue>)  [unwired: 2 in, 2 out]
                    }
                  }
                  frame True {
                    n703 = for {
                      shift-right: [w2068] -> w2066
                      shift-left: w2064 -> [w2069]
                      tunnel: string[] ["RESET ENCODERS", "RESET YAW", "RESET FLAGS"] -> [w2067] mode=indexing
                      n704 = Enqueue Element(queue=w2069, element=w2067) -> (queue out=w2068:refnum<queue>)  [unwired: 2 in, 2 out]
                    }
                  }
                }
                n705 = Select(t=State_Type_Definitions,_for_0.26g_versions_and_later_3."True Stop" ("Enum"), s=w2049, f=State_Type_Definitions,_for_0.26g_versions_and_later_3."Task 5F: ARM GRAB HEIGHT" ("Enum")) -> (s? t:f=w2052:T18)
                n706 = Select(t=w2052, s=w2050, f=State_Type_Definitions,_for_0.26g_versions_and_later_3."Task 6P: PIPE BOMB" ("Enum")) -> (s? t:f=w2054:T18)
              }
              frame "Exit" {
                n707 = for {
                  shift-right: [w2076] -> w2073
                  shift-left: w2070 -> [w2077]
                  tunnel: string[] ["STOP", "RESET ENCODERS", "RESET YAW", "ARDUINO MODE 0"] -> [w2075] mode=indexing
                  n708 = Enqueue Element(queue=w2077, element=w2075) -> (queue out=w2076:refnum<queue>)  [unwired: 2 in, 2 out]
                }
              }
            }
          }
          frame "Task 7" {
          }
          frame "Task 8A: RAISE ARM" {
            # ">>> Motor control cluster >>>"
            # ">>> yStepper command>>>"
            # ">> Manual override >>"
            n709 = Dequeue Element(queue=w2094, timeout in ms (-1)=w2093, error in (no error)=w2095) -> (element=w2092:T10)  [unwired: 3 out]
            n710 = Equal?(x=w2091, y=u8 60) -> (x = y?=w2089:bool)
            n711 = case shown="\"Start Task 1\", Default" w2092 {
              tunnel: [w2105 State_Type_Definitions,_for_0.26g_versions_and_later_3."True Stop" ("Enum")] -> w2096
              tunnel: [w2108 w2125] -> w2097
              tunnel: [State_Type_Definitions,_for_0.26g_versions_and_later_3."Idle" ("Enum") State_Type_Definitions,_for_0.26g_versions_and_later_3."Shutdown" ("Enum")] -> w2098
              tunnel: w2089 -> [w2104 _]
              tunnel: w2088 -> [w2103 _]
              tunnel: w2087 -> [w2099 w2122]
              frame "Start Task 1", Default {
                # "Stays in Task 5_A until stepper reaches desired \nheight"
                # "T: Go back to idle, F: Continue with task\""
                # ">> Manual override >>"
                n712 = case shown="False" w2104 {
                  tunnel: [w2112 w2118] -> w2108
                  tunnel: w2099 -> [w2110 w2116]
                  frame False {
                    n713 = for {
                      tunnel: string[] ["Z STEPPER CAM HEIGHT", "READ STEPPER VALUES", "READ IR"] ("element") -> [w2113] mode=indexing
                      shift-right: [w2115] -> w2112
                      shift-left: w2110 -> [w2114]
                      n714 = Enqueue Element(queue=w2114, element=w2113) -> (queue out=w2115:refnum<queue>)  [unwired: 2 in, 2 out]
                    }
                  }
                  frame True {
                    n715 = for {
                      shift-right: [w2120] -> w2118
                      shift-left: w2116 -> [w2121]
                      tunnel: string[] ["RESET YAW", "RESET ENCODERS", "READ IR"] -> [w2119] mode=indexing
                      n716 = Enqueue Element(queue=w2121, element=w2119) -> (queue out=w2120:refnum<queue>)  [unwired: 2 in, 2 out]
                    }
                  }
                }
                n717 = Or(x=w2104, y=w2103) -> (x .or. y?=w2106:bool)
                n718 = Select(t=State_Type_Definitions,_for_0.26g_versions_and_later_3."True Stop" ("Enum"), s=w2103, f=State_Type_Definitions,_for_0.26g_versions_and_later_3."Task 8B: MOVE TO BOX" ("Enum")) -> (s? t:f=w2100:T18)
                n719 = Select(t=w2100, s=w2106, f=State_Type_Definitions,_for_0.26g_versions_and_later_3."Task 8A: RAISE ARM" ("Enum")) -> (s? t:f=w2105:T18)
              }
              frame "Exit" {
                n720 = for {
                  shift-right: [w2128] -> w2125
                  shift-left: w2122 -> [w2129]
                  tunnel: string[] ["STOP", "RESET ENCODERS", "RESET YAW", "ARDUINO MODE 0"] -> [w2127] mode=indexing
                  n721 = Enqueue Element(queue=w2129, element=w2127) -> (queue out=w2128:refnum<queue>)  [unwired: 2 in, 2 out]
                }
              }
            }
          }
          frame "Task 8B: MOVE TO BOX" {
            w2139 = u8 15 ("y")
            # "High voltage: 70"
            # ">>> yStepper command>>>"
            n722 = Less?(x=w2136, y=w2139) -> (x < y?=w2137:bool)
            n723 = Less?(x=w2135, y=w2139) -> (x < y?=w2138:bool)
            n724 = And(x=w2138, y=w2137) -> ()  [unwired: 1 out]
            n725 = Dequeue Element(queue=w2143, timeout in ms (-1)=w2142, error in (no error)=w2144) -> (element=w2141:T10)  [unwired: 3 out]
            n726 = Less?(x=w2132, y=40.0) -> (x < y?=w2130:bool)
            n727 = case shown="\"Start Task 1\", Default" w2141 {
              tunnel: [w2156 State_Type_Definitions,_for_0.26g_versions_and_later_3."True Stop" ("Enum")] -> w2146
              tunnel: [w2159 w2176] -> w2145
              tunnel: [State_Type_Definitions,_for_0.26g_versions_and_later_3."Idle" ("Enum") State_Type_Definitions,_for_0.26g_versions_and_later_3."Shutdown" ("Enum")] -> w2147
              tunnel: w2149 -> [w2155 _]
              tunnel: w2148 -> [w2151 w2173]
              tunnel: w2130 -> [w2150 _]
              frame "Start Task 1", Default {
                # "Stays in Task 5_B to capture image over 5 seconds"
                # "T: Go back to idle, F: Continue with task\""
                # ">> Manual override >>"
                n728 = case shown="True" w2150 {
                  tunnel: [w2163 w2169] -> w2159
                  tunnel: w2151 -> [w2161 w2167]
                  frame False {
                    n729 = for {
                      tunnel: string[] ["FORWARD", "READ IR", "READ NAVX"] ("element") -> [w2164] mode=indexing
                      shift-right: [w2166] -> w2163
                      shift-left: w2161 -> [w2165]
                      n730 = Enqueue Element(queue=w2165, element=w2164) -> (queue out=w2166:refnum<queue>)  [unwired: 2 in, 2 out]
                    }
                  }
                  frame True {
                    n731 = for {
                      shift-right: [w2171] -> w2169
                      shift-left: w2167 -> [w2172]
                      tunnel: string[] ["STOP", "RESET ENCODERS", "OPEN LOG CAM", "SET TIMER 2", "OPEN IMAQ REF"] -> [w2170] mode=indexing
                      n732 = Enqueue Element(queue=w2172, element=w2170) -> (queue out=w2171:refnum<queue>)  [unwired: 2 in, 2 out]
                    }
                  }
                }
                n733 = Or(x=w2150, y=w2155) -> (x .or. y?=w2157:bool)
                n734 = Select(t=State_Type_Definitions,_for_0.26g_versions_and_later_3."True Stop" ("Enum"), s=w2155, f=State_Type_Definitions,_for_0.26g_versions_and_later_3."Task 8C: CAM BURST" ("Enum")) -> (s? t:f=w2152:T18)
                n735 = Select(t=w2152, s=w2157, f=State_Type_Definitions,_for_0.26g_versions_and_later_3."Task 8B: MOVE TO BOX" ("Enum")) -> (s? t:f=w2156:T18)
              }
              frame "Exit" {
                n736 = for {
                  shift-right: [w2179] -> w2176
                  shift-left: w2173 -> [w2180]
                  tunnel: string[] ["STOP", "RESET ENCODERS", "RESET YAW", "ARDUINO MODE 0"] -> [w2178] mode=indexing
                  n737 = Enqueue Element(queue=w2180, element=w2178) -> (queue out=w2179:refnum<queue>)  [unwired: 2 in, 2 out]
                }
              }
            }
          }
          frame "Task 8C: CAM BURST" {
            # ">>> Motor control cluster >>>"
            # ">>> yStepper command>>>"
            # ">> Manual override >>"
            n738 = Dequeue Element(queue=w2191, timeout in ms (-1)=w2190, error in (no error)=w2189) -> (element=w2188:T10)  [unwired: 3 out]
            n739 = case shown="\"Start Task 1\", Default" w2188 {
              tunnel: [w2200 State_Type_Definitions,_for_0.26g_versions_and_later_3."True Stop" ("Enum")] -> w2193
              tunnel: [w2203 w2220] -> w2186
              tunnel: [State_Type_Definitions,_for_0.26g_versions_and_later_3."Idle" ("Enum") State_Type_Definitions,_for_0.26g_versions_and_later_3."Shutdown" ("Enum")] -> w2185
              tunnel: w2187 -> [w2194 _]
              tunnel: w2192 -> [w2199 w2217]
              tunnel: w2183 -> [w2198 _]
              frame "Start Task 1", Default {
                # ">> Is time up? >>"
                # "Determines if object is in range to pick up"
                # ">> Manual override >>"
                n740 = case shown="True" w2198 {
                  tunnel: [w2207 w2213] -> w2203
                  tunnel: w2199 -> [w2205 w2211]
                  frame False {
                    n741 = for {
                      tunnel: string[] ["CAM ACQ", "START TIMER"] ("element") -> [w2208] mode=indexing
                      shift-right: [w2210] -> w2207
                      shift-left: w2205 -> [w2209]
                      n742 = Enqueue Element(queue=w2209, element=w2208) -> (queue out=w2210:refnum<queue>)  [unwired: 2 in, 2 out]
                    }
                  }
                  frame True {
                    n743 = for {
                      shift-right: [w2215] -> w2213
                      shift-left: w2211 -> [w2216]
                      tunnel: string[] ["CAM CLOSE", "PROCESS IMAGE", "SET TIMER 2"] -> [w2214] mode=indexing
                      n744 = Enqueue Element(queue=w2216, element=w2214) -> (queue out=w2215:refnum<queue>)  [unwired: 2 in, 2 out]
                    }
                  }
                }
                n745 = Or(x=w2198, y=w2194) -> (x .or. y?=w2201:bool)
                n746 = Select(t=State_Type_Definitions,_for_0.26g_versions_and_later_3."True Stop" ("Enum"), s=w2194, f=State_Type_Definitions,_for_0.26g_versions_and_later_3."Task 8D: PROCESS IMAGE" ("Enum")) -> (s? t:f=w2196:T18)
                n747 = Select(t=w2196, s=w2201, f=State_Type_Definitions,_for_0.26g_versions_and_later_3."Task 8C: CAM BURST" ("Enum")) -> (s? t:f=w2200:T18)
              }
              frame "Exit" {
                n748 = for {
                  shift-right: [w2223] -> w2220
                  shift-left: w2217 -> [w2224]
                  tunnel: string[] ["STOP", "RESET ENCODERS", "RESET YAW", "ARDUINO MODE 0"] -> [w2222] mode=indexing
                  n749 = Enqueue Element(queue=w2224, element=w2222) -> (queue out=w2223:refnum<queue>)  [unwired: 2 in, 2 out]
                }
              }
            }
          }
          frame "Task 8D: PROCESS IMAGE" {
            # ">>> Motor control cluster >>>"
            # ">>> yStepper command>>>"
            n750 = Dequeue Element(queue=w2233, timeout in ms (-1)=w2232, error in (no error)=w2231) -> (element=w2230:T10)  [unwired: 3 out]
            n751 = case shown="\"Start Task 1\", Default" w2230 {
              tunnel: [w2248 State_Type_Definitions,_for_0.26g_versions_and_later_3."True Stop" ("Enum")] -> w2237
              tunnel: [w2251 w2268] -> w2236
              tunnel: [State_Type_Definitions,_for_0.26g_versions_and_later_3."Idle" ("Enum") State_Type_Definitions,_for_0.26g_versions_and_later_3."Shutdown" ("Enum")] -> w2238
              tunnel: w2234 -> [w2247 _]
              tunnel: w2235 -> [w2244 w2265]
              tunnel: w2225 -> [w2243 _]
              tunnel: w2226 -> [w2242 _]
              frame "Start Task 1", Default {
                # ">> T: Breaks out of state loop; F: Stays in loop>>"
                # ">> Manual override >>"
                # ">> Checks if time is up>>"
                # "Stays in Task 5D until the object is detected"
                # "T: Go back to idle, F: Continue with task\""
                # ">> Manual override >>"
                n752 = case shown="False" w2243 {
                  tunnel: [w2255 w2261] -> w2251
                  tunnel: w2244 -> [w2253 w2259]
                  frame False {
                    n753 = for {
                      tunnel: string[] ["START TIMER", "PROCESS IMAGE", ""] ("element") -> [w2256] mode=indexing
                      shift-right: [w2258] -> w2255
                      shift-left: w2253 -> [w2257]
                      n754 = Enqueue Element(queue=w2257, element=w2256) -> (queue out=w2258:refnum<queue>)  [unwired: 2 in, 2 out]
                    }
                  }
                  frame True {
                    n755 = for {
                      shift-right: [w2263] -> w2261
                      shift-left: w2259 -> [w2264]
                      tunnel: string[] ["RESET ENCODERS", "", ""] -> [w2262] mode=indexing
                      n756 = Enqueue Element(queue=w2264, element=w2262) -> (queue out=w2263:refnum<queue>)  [unwired: 2 in, 2 out]
                    }
                  }
                }
                n757 = Or(x=w2243, y=w2247) -> (x .or. y?=w2249:bool)
                n758 = Select(t=State_Type_Definitions,_for_0.26g_versions_and_later_3."Task 8E: ROBOT ADJUST" ("Enum"), s=w2242, f=State_Type_Definitions,_for_0.26g_versions_and_later_3."True Stop" ("Enum")) -> (s? t:f=w2239:T18)
                n759 = Select(t=State_Type_Definitions,_for_0.26g_versions_and_later_3."True Stop" ("Enum"), s=w2247, f=w2239) -> (s? t:f=w2245:T18)
                n760 = Select(t=w2245, s=w2249, f=State_Type_Definitions,_for_0.26g_versions_and_later_3."Task 8D: PROCESS IMAGE" ("Enum")) -> (s? t:f=w2248:T18)
              }
              frame "Exit" {
                n761 = for {
                  shift-right: [w2271] -> w2268
                  shift-left: w2265 -> [w2272]
                  tunnel: string[] ["STOP", "RESET ENCODERS", "RESET YAW", "ARDUINO MODE 0"] -> [w2270] mode=indexing
                  n762 = Enqueue Element(queue=w2272, element=w2270) -> (queue out=w2271:refnum<queue>)  [unwired: 2 in, 2 out]
                }
              }
            }
          }
          frame "Task 8E: ROBOT ADJUST" {
            # ">>> Motor control cluster >>>"
            # ">>> yStepper command>>>"
            n763 = Dequeue Element(queue=w2290, timeout in ms (-1)=w2289, error in (no error)=w2288) -> (element=w2287:T10)  [unwired: 3 out]
            n764 = Subtract(x=w2285, y=150.0) -> (x-y=w2283:dbl)
            n765 = formula code="if (error <= -100 && error < -80){\n    distance = -20;\n    xSpeed = -30;\n}\n\nelse if (error <= -80 && error < -60){\n    distance = -18;\n    xSpeed = -30;\n}\n\nelse if (error <= -60 && error < -40){\n    distance = -15;\n    xSpeed = -30;\n}\n\nelse if (error <= -40 && error < -20){\n    distance = -10;\n    xSpeed = -30;\n}\n\nelse if (error <= -20 && error < -10){\n    distance = 5;\n    xSpeed = -30;\n}\n\nelse if (error <= -10 && error <= 10){\n    distance = 0;\n    xSpeed = 0;\n}\n\nelse if (error <= 20 && error < 40){\n    distance = 5;\n    xSpeed = 30;\n}\n\nelse if (error <= 40 && error < 60){\n    distance = 10;\n    xSpeed = 30;\n}\n\nelse if (error <= 60 && error < 80){\n    distance = 15;\n    xSpeed = 30;\n}\n\nelse if (error <= 80 && error < 100){\n    distance = 18;\n    xSpeed = 30;\n}\n\nelse if (error <= 100){\n    distance = 20;\n    xSpeed = 30;\n}\n\nelse {\n    distance = 0;\n    xSpeed = 0;\n}"("error"=w2283) -> ("distance"=w2273:dbl, "xSpeed"=w2280:dbl)
            n766 = formula code="if (target > 0){\nif (current  >= target)\noutput = 1;\n\nelse if (current != target)\noutput = 0;\n}\n\nelse if (target == 0){\nif (current == target)\noutput = 1;\n\nelse if (current != target)\noutput = 0;\n}\n\nelse if (target < 0){\nif (current <= target)\noutput = 1;\n\nelse if (current != target)\noutput = 0;\n}\n\nelse if (current != target)\noutput = 0;"("target"=w2273, "current"=w2279) -> ("output"=w2278:dbl)
            n767 = call "yDistance travelled FGV.vi"("Init/Read/Write State"=States_for_Action_Engine."Write", "yDistance travelled"=w2273) -> ()  [unwired: 8 in, 2 out]
            n768 = Bundle By Name(cluster=w2282, "xSpeed"=w2280) -> (w2281:T20)
            n769 = Equal?(x=w2278, y=1.0) -> (x = y?=w2275:bool)
            n770 = case shown="\"Start Task 1\", Default" w2287 {
              tunnel: [w2302 State_Type_Definitions,_for_0.26g_versions_and_later_3."True Stop" ("Enum")] -> w2294
              tunnel: [w2305 w2322] -> w2293
              tunnel: [State_Type_Definitions,_for_0.26g_versions_and_later_3."Idle" ("Enum") State_Type_Definitions,_for_0.26g_versions_and_later_3."Shutdown" ("Enum")] -> w2295
              tunnel: w2291 -> [w2301 _]
              tunnel: w2292 -> [w2297 w2319]
              tunnel: w2275 -> [w2296 _]
              frame "Start Task 1", Default {
                # ">> T: Breaks out of state loop; F: Stays in loop>>"
                # ">> Manual override >>"
                # ">> Checks if time is up>>"
                # "Stays in Task 5D until the object is detected"
                # "T: Go back to idle, F: Continue with task\""
                # ">> Manual override >>"
                n771 = case shown="True" w2296 {
                  tunnel: [w2309 w2315] -> w2305
                  tunnel: w2297 -> [w2307 w2313]
                  frame False {
                    n772 = for {
                      tunnel: string[] ["X AXIS - SLOW", "READ ENCODERS", "READ NAVX"] ("element") -> [w2310] mode=indexing
                      shift-right: [w2312] -> w2309
                      shift-left: w2307 -> [w2311]
                      n773 = Enqueue Element(queue=w2311, element=w2310) -> (queue out=w2312:refnum<queue>)  [unwired: 2 in, 2 out]
                    }
                  }
                  frame True {
                    n774 = for {
                      shift-right: [w2317] -> w2315
                      shift-left: w2313 -> [w2318]
                      tunnel: string[] ["SET TIMER 2", "STOP", "READ STEPPER VALUES", ""] -> [w2316] mode=indexing
                      n775 = Enqueue Element(queue=w2318, element=w2316) -> (queue out=w2317:refnum<queue>)  [unwired: 2 in, 2 out]
                    }
                  }
                }
                n776 = Or(x=w2296, y=w2301) -> (x .or. y?=w2303:bool)
                n777 = Select(t=State_Type_Definitions,_for_0.26g_versions_and_later_3."True Stop" ("Enum"), s=w2301, f=State_Type_Definitions,_for_0.26g_versions_and_later_3."Task 8H: ARM ADJUST" ("Enum")) -> (s? t:f=w2298:T18)
                n778 = Select(t=w2298, s=w2303, f=State_Type_Definitions,_for_0.26g_versions_and_later_3."Task 8E: ROBOT ADJUST" ("Enum")) -> (s? t:f=w2302:T18)
              }
              frame "Exit" {
                n779 = for {
                  shift-right: [w2325] -> w2322
                  shift-left: w2319 -> [w2326]
                  tunnel: string[] ["STOP", "RESET ENCODERS", "RESET YAW", "ARDUINO MODE 0"] -> [w2324] mode=indexing
                  n780 = Enqueue Element(queue=w2326, element=w2324) -> (queue out=w2325:refnum<queue>)  [unwired: 2 in, 2 out]
                }
              }
            }
          }
          frame "Task 8F: CAM BURST 2" {
            # ">>> Motor control cluster >>>"
            # ">>> yStepper command>>>"
            # ">> Manual override >>"
            n781 = Dequeue Element(queue=w2337, timeout in ms (-1)=w2336, error in (no error)=w2335) -> (element=w2334:T10)  [unwired: 3 out]
            n782 = case shown="\"Start Task 1\", Default" w2334 {
              tunnel: [w2346 State_Type_Definitions,_for_0.26g_versions_and_later_3."True Stop" ("Enum")] -> w2339
              tunnel: [w2349 w2366] -> w2332
              tunnel: [State_Type_Definitions,_for_0.26g_versions_and_later_3."Idle" ("Enum") State_Type_Definitions,_for_0.26g_versions_and_later_3."Shutdown" ("Enum")] -> w2331
              tunnel: w2333 -> [w2340 _]
              tunnel: w2338 -> [w2345 w2363]
              tunnel: w2329 -> [w2344 _]
              frame "Start Task 1", Default {
                # ">> Is time up? >>"
                # "Determines if object is in range to pick up"
                # ">> Manual override >>"
                n783 = case shown="False" w2344 {
                  tunnel: [w2353 w2359] -> w2349
                  tunnel: w2345 -> [w2351 w2357]
                  frame False {
                    n784 = for {
                      tunnel: string[] ["CAM ACQ", "START TIMER"] ("element") -> [w2354] mode=indexing
                      shift-right: [w2356] -> w2353
                      shift-left: w2351 -> [w2355]
                      n785 = Enqueue Element(queue=w2355, element=w2354) -> (queue out=w2356:refnum<queue>)  [unwired: 2 in, 2 out]
                    }
                  }
                  frame True {
                    n786 = for {
                      shift-right: [w2361] -> w2359
                      shift-left: w2357 -> [w2362]
                      tunnel: string[] ["CAM CLOSE", "PROCESS IMAGE", "SET TIMER 3"] -> [w2360] mode=indexing
                      n787 = Enqueue Element(queue=w2362, element=w2360) -> (queue out=w2361:refnum<queue>)  [unwired: 2 in, 2 out]
                    }
                  }
                }
                n788 = Or(x=w2344, y=w2340) -> (x .or. y?=w2347:bool)
                n789 = Select(t=State_Type_Definitions,_for_0.26g_versions_and_later_3."True Stop" ("Enum"), s=w2340, f=State_Type_Definitions,_for_0.26g_versions_and_later_3."Task 8G: PROCESS IMAGE 2" ("Enum")) -> (s? t:f=w2342:T18)
                n790 = Select(t=w2342, s=w2347, f=State_Type_Definitions,_for_0.26g_versions_and_later_3."Task 8F: CAM BURST 2" ("Enum")) -> (s? t:f=w2346:T18)
              }
              frame "Exit" {
                n791 = for {
                  shift-right: [w2369] -> w2366
                  shift-left: w2363 -> [w2370]
                  tunnel: string[] ["STOP", "RESET ENCODERS", "RESET YAW", "ARDUINO MODE 0"] -> [w2368] mode=indexing
                  n792 = Enqueue Element(queue=w2370, element=w2368) -> (queue out=w2369:refnum<queue>)  [unwired: 2 in, 2 out]
                }
              }
            }
          }
          frame "Task 8G: PROCESS IMAGE 2" {
            # ">>> yStepper command>>>"
            n793 = Dequeue Element(queue=w2378, timeout in ms (-1)=w2377, error in (no error)=w2376) -> (element=w2375:T10)  [unwired: 3 out]
            n794 = case shown="\"Start Task 1\", Default" w2375 {
              tunnel: [w2390 State_Type_Definitions,_for_0.26g_versions_and_later_3."True Stop" ("Enum")] -> w2382
              tunnel: [w2393 w2410] -> w2381
              tunnel: [State_Type_Definitions,_for_0.26g_versions_and_later_3."Idle" ("Enum") State_Type_Definitions,_for_0.26g_versions_and_later_3."Shutdown" ("Enum")] -> w2383
              tunnel: w2379 -> [w2389 _]
              tunnel: w2380 -> [w2385 w2407]
              tunnel: w2373 -> [w2384 _]
              frame "Start Task 1", Default {
                # ">> T: Breaks out of state loop; F: Stays in loop>>"
                # ">> Manual override >>"
                # ">> Checks if time is up>>"
                # "Stays in Task 5D until the object is detected"
                # "T: Go back to idle, F: Continue with task\""
                # ">> Manual override >>"
                n795 = case shown="False" w2384 {
                  tunnel: [w2397 w2403] -> w2393
                  tunnel: w2385 -> [w2395 w2401]
                  frame False {
                    n796 = for {
                      tunnel: string[] ["START TIMER", "PROCESS IMAGE", ""] ("element") -> [w2398] mode=indexing
                      shift-right: [w2400] -> w2397
                      shift-left: w2395 -> [w2399]
                      n797 = Enqueue Element(queue=w2399, element=w2398) -> (queue out=w2400:refnum<queue>)  [unwired: 2 in, 2 out]
                    }
                  }
                  frame True {
                    n798 = for {
                      shift-right: [w2405] -> w2403
                      shift-left: w2401 -> [w2406]
                      tunnel: string[] ["READ STEPPER VALUES", "Y STEPPER CONTROL", ""] -> [w2404] mode=indexing
                      n799 = Enqueue Element(queue=w2406, element=w2404) -> (queue out=w2405:refnum<queue>)  [unwired: 2 in, 2 out]
                    }
                  }
                }
                n800 = Or(x=w2384, y=w2389) -> (x .or. y?=w2391:bool)
                n801 = Select(t=State_Type_Definitions,_for_0.26g_versions_and_later_3."True Stop" ("Enum"), s=w2389, f=State_Type_Definitions,_for_0.26g_versions_and_later_3."Task 8H: ARM ADJUST" ("Enum")) -> (s? t:f=w2386:T18)
                n802 = Select(t=w2386, s=w2391, f=State_Type_Definitions,_for_0.26g_versions_and_later_3."Task 8G: PROCESS IMAGE 2" ("Enum")) -> (s? t:f=w2390:T18)
              }
              frame "Exit" {
                n803 = for {
                  shift-right: [w2413] -> w2410
                  shift-left: w2407 -> [w2414]
                  tunnel: string[] ["STOP", "RESET ENCODERS", "RESET YAW", "ARDUINO MODE 0"] -> [w2412] mode=indexing
                  n804 = Enqueue Element(queue=w2414, element=w2412) -> (queue out=w2413:refnum<queue>)  [unwired: 2 in, 2 out]
                }
              }
            }
          }
          frame "Task 8H: ARM ADJUST" {
            # ">>> yStepper command>>>"
            n805 = Dequeue Element(queue=w2428, timeout in ms (-1)=w2429, error in (no error)=w2430) -> (element=w2432:T10)  [unwired: 3 out]
            n806 = formula code="if (pos >= 40 && pos < 80)\ny = 40;\n\nelse if (pos >= 80 && pos < 100)\ny = 35;\n\nelse if (pos >= 100 && pos < 120)\ny = 20;\n\nelse if (pos >= 120 && pos < 140)\ny = 15;\n\nelse if (pos >= 140 && pos < 150)\ny = 10;\n\nelse if (pos >= 150 && 170)\ny = 5;\n\nelse \ny = 0;"("pos"=w2420) -> ("y"=w2423:dbl)
            n807 = To Unsigned Byte Integer(number=w2423) -> (unsigned 8bit integer=w2418:u8)
            n808 = Equal?(x=w2419, y=w2418) -> (x = y?=w2417:bool)
            n809 = case shown="\"Start Task 1\", Default" w2432 {
              tunnel: [w2439 State_Type_Definitions,_for_0.26g_versions_and_later_3."True Stop" ("Enum")] -> w2426
              tunnel: [w2442 w2459] -> w2424
              tunnel: [State_Type_Definitions,_for_0.26g_versions_and_later_3."Idle" ("Enum") State_Type_Definitions,_for_0.26g_versions_and_later_3."Shutdown" ("Enum")] -> w2425
              tunnel: w2431 -> [w2433 _]
              tunnel: w2427 -> [w2435 w2456]
              tunnel: w2417 -> [w2434 _]
              frame "Start Task 1", Default {
                # ">> T: Breaks out of state loop; F: Stays in loop>>"
                # ">> Manual override >>"
                # ">> Checks if time is up>>"
                # "Stays in Task 5D until the object is detected"
                # "T: Go back to idle, F: Continue with task\""
                # ">> Manual override >>"
                n810 = case shown="False" w2434 {
                  tunnel: [w2446 w2452] -> w2442
                  tunnel: w2435 -> [w2444 w2450]
                  frame False {
                    n811 = for {
                      tunnel: string[] ["READ STEPPER VALUES", "Y STEPPER CONTROL", ""] ("element") -> [w2447] mode=indexing
                      shift-right: [w2449] -> w2446
                      shift-left: w2444 -> [w2448]
                      n812 = Enqueue Element(queue=w2448, element=w2447) -> (queue out=w2449:refnum<queue>)  [unwired: 2 in, 2 out]
                    }
                  }
                  frame True {
                    n813 = for {
                      shift-right: [w2454] -> w2452
                      shift-left: w2450 -> [w2455]
                      tunnel: string[] ["DISPOSE BUFFERS", "READ STEPPER VALUES", ""] -> [w2453] mode=indexing
                      n814 = Enqueue Element(queue=w2455, element=w2453) -> (queue out=w2454:refnum<queue>)  [unwired: 2 in, 2 out]
                    }
                  }
                }
                n815 = Or(x=w2434, y=w2433) -> (x .or. y?=w2440:bool)
                n816 = Select(t=State_Type_Definitions,_for_0.26g_versions_and_later_3."True Stop" ("Enum"), s=w2433, f=State_Type_Definitions,_for_0.26g_versions_and_later_3."Task 8I: ARM GRAB HEIGHT" ("Enum")) -> (s? t:f=w2436:T18)
                n817 = Select(t=w2436, s=w2440, f=State_Type_Definitions,_for_0.26g_versions_and_later_3."Task 8H: ARM ADJUST" ("Enum")) -> (s? t:f=w2439:T18)
              }
              frame "Exit" {
                n818 = for {
                  shift-right: [w2462] -> w2459
                  shift-left: w2456 -> [w2463]
                  tunnel: string[] ["STOP", "RESET ENCODERS", "RESET YAW", "ARDUINO MODE 0"] -> [w2461] mode=indexing
                  n819 = Enqueue Element(queue=w2463, element=w2461) -> (queue out=w2462:refnum<queue>)  [unwired: 2 in, 2 out]
                }
              }
            }
            n820 = Bundle By Name(cluster=w2422, "yStepper desired"=w2418) -> (w2421:T21)
          }
          frame "Task 8I: ARM GRAB HEIGHT" {
            # ">>> Motor control cluster >>>"
            # ">>> yStepper command>>>"
            # ">> Manual override >>"
            n821 = Dequeue Element(queue=w2474, timeout in ms (-1)=w2473, error in (no error)=w2475) -> (element=w2472:T10)  [unwired: 3 out]
            n822 = Equal?(x=w2471, y=u8 1) -> (x = y?=w2469:bool)
            n823 = case shown="\"Start Task 1\", Default" w2472 {
              tunnel: [w2485 State_Type_Definitions,_for_0.26g_versions_and_later_3."True Stop" ("Enum")] -> w2476
              tunnel: [w2488 w2505] -> w2477
              tunnel: [State_Type_Definitions,_for_0.26g_versions_and_later_3."Idle" ("Enum") State_Type_Definitions,_for_0.26g_versions_and_later_3."Shutdown" ("Enum")] -> w2478
              tunnel: w2469 -> [w2484 _]
              tunnel: w2468 -> [w2483 _]
              tunnel: w2467 -> [w2479 w2502]
              frame "Start Task 1", Default {
                # "Stays in Task 5F until stepper reaches desired \nheight"
                # "T: Go back to idle, F: Continue with task\""
                # ">> Manual override >>"
                n824 = case shown="True" w2484 {
                  tunnel: [w2492 w2498] -> w2488
                  tunnel: w2479 -> [w2490 w2496]
                  frame False {
                    n825 = for {
                      tunnel: string[] ["Z STEPPER GRAB HEIGHT", "READ STEPPER VALUES"] ("element") -> [w2493] mode=indexing
                      shift-right: [w2495] -> w2492
                      shift-left: w2490 -> [w2494]
                      n826 = Enqueue Element(queue=w2494, element=w2493) -> (queue out=w2495:refnum<queue>)  [unwired: 2 in, 2 out]
                    }
                  }
                  frame True {
                    n827 = for {
                      shift-right: [w2500] -> w2498
                      shift-left: w2496 -> [w2501]
                      tunnel: string[] ["SET TIMER 2", "CLOSE CLAW", ""] -> [w2499] mode=indexing
                      n828 = Enqueue Element(queue=w2501, element=w2499) -> (queue out=w2500:refnum<queue>)  [unwired: 2 in, 2 out]
                    }
                  }
                }
                n829 = Or(x=w2484, y=w2483) -> (x .or. y?=w2486:bool)
                n830 = Select(t=State_Type_Definitions,_for_0.26g_versions_and_later_3."True Stop" ("Enum"), s=w2483, f=State_Type_Definitions,_for_0.26g_versions_and_later_3."Task 8J: CLOSE CLAW" ("Enum")) -> (s? t:f=w2480:T18)
                n831 = Select(t=w2480, s=w2486, f=State_Type_Definitions,_for_0.26g_versions_and_later_3."Task 8I: ARM GRAB HEIGHT" ("Enum")) -> (s? t:f=w2485:T18)
              }
              frame "Exit" {
                n832 = for {
                  shift-right: [w2508] -> w2505
                  shift-left: w2502 -> [w2509]
                  tunnel: string[] ["STOP", "RESET ENCODERS", "RESET YAW", "ARDUINO MODE 0"] -> [w2507] mode=indexing
                  n833 = Enqueue Element(queue=w2509, element=w2507) -> (queue out=w2508:refnum<queue>)  [unwired: 2 in, 2 out]
                }
              }
            }
          }
          frame "Task 8J: CLOSE CLAW" {
            # ">>> yStepper command>>>"
            # ">> Manual override >>"
            n834 = Dequeue Element(queue=w2520, timeout in ms (-1)=w2519, error in (no error)=w2518) -> (element=w2517:T10)  [unwired: 3 out]
            n835 = case shown="\"Start Task 1\", Default" w2517 {
              tunnel: [w2529 State_Type_Definitions,_for_0.26g_versions_and_later_3."True Stop" ("Enum")] -> w2522
              tunnel: [w2532 w2549] -> w2515
              tunnel: [State_Type_Definitions,_for_0.26g_versions_and_later_3."Idle" ("Enum") State_Type_Definitions,_for_0.26g_versions_and_later_3."Shutdown" ("Enum")] -> w2514
              tunnel: w2516 -> [w2523 _]
              tunnel: w2521 -> [w2528 w2546]
              tunnel: w2512 -> [w2527 _]
              frame "Start Task 1", Default {
                # ">> Is time up? >>"
                # "Determines if object is in range to pick up"
                # ">> Manual override >>"
                n836 = case shown="True" w2527 {
                  tunnel: [w2536 w2542] -> w2532
                  tunnel: w2528 -> [w2534 w2540]
                  frame False {
                    n837 = for {
                      tunnel: string[] ["CLOSE CLAW", "START TIMER"] ("element") -> [w2537] mode=indexing
                      shift-right: [w2539] -> w2536
                      shift-left: w2534 -> [w2538]
                      n838 = Enqueue Element(queue=w2538, element=w2537) -> (queue out=w2539:refnum<queue>)  [unwired: 2 in, 2 out]
                    }
                  }
                  frame True {
                    n839 = for {
                      shift-right: [w2544] -> w2542
                      shift-left: w2540 -> [w2545]
                      tunnel: string[] ["READ STEPPER VALUES", "", ""] -> [w2543] mode=indexing
                      n840 = Enqueue Element(queue=w2545, element=w2543) -> (queue out=w2544:refnum<queue>)  [unwired: 2 in, 2 out]
                    }
                  }
                }
                n841 = Or(x=w2527, y=w2523) -> (x .or. y?=w2530:bool)
                n842 = Select(t=State_Type_Definitions,_for_0.26g_versions_and_later_3."True Stop" ("Enum"), s=w2523, f=State_Type_Definitions,_for_0.26g_versions_and_later_3."Task 8K: RAISE MY SWORD" ("Enum")) -> (s? t:f=w2525:T18)
                n843 = Select(t=w2525, s=w2530, f=State_Type_Definitions,_for_0.26g_versions_and_later_3."Task 8J: CLOSE CLAW" ("Enum")) -> (s? t:f=w2529:T18)
              }
              frame "Exit" {
                n844 = for {
                  shift-right: [w2552] -> w2549
                  shift-left: w2546 -> [w2553]
                  tunnel: string[] ["STOP", "RESET ENCODERS", "RESET YAW", "ARDUINO MODE 0"] -> [w2551] mode=indexing
                  n845 = Enqueue Element(queue=w2553, element=w2551) -> (queue out=w2552:refnum<queue>)  [unwired: 2 in, 2 out]
                }
              }
            }
          }
          frame "Task 8K: RAISE MY SWORD" {
            # ">>> Motor control cluster >>>"
            # ">>> yStepper command>>>"
            # ">> Manual override >>"
            n846 = Dequeue Element(queue=w2564, timeout in ms (-1)=w2563, error in (no error)=w2565) -> (element=w2562:T10)  [unwired: 3 out]
            n847 = Equal?(x=w2561, y=u8 60) -> (x = y?=w2559:bool)
            n848 = case shown="\"Start Task 1\", Default" w2562 {
              tunnel: [w2575 State_Type_Definitions,_for_0.26g_versions_and_later_3."True Stop" ("Enum")] -> w2566
              tunnel: [w2578 w2595] -> w2567
              tunnel: [State_Type_Definitions,_for_0.26g_versions_and_later_3."Idle" ("Enum") State_Type_Definitions,_for_0.26g_versions_and_later_3."Shutdown" ("Enum")] -> w2568
              tunnel: w2559 -> [w2574 _]
              tunnel: w2558 -> [w2573 _]
              tunnel: w2557 -> [w2569 w2592]
              frame "Start Task 1", Default {
                # "Stays in Task 5_A until stepper reaches desired \nheight"
                # "T: Go back to idle, F: Continue with task\""
                # ">> Manual override >>"
                n849 = case shown="True" w2574 {
                  tunnel: [w2582 w2588] -> w2578
                  tunnel: w2569 -> [w2580 w2586]
                  frame False {
                    n850 = for {
                      tunnel: string[] ["Z STEPPER CAM HEIGHT", "READ STEPPER VALUES"] ("element") -> [w2583] mode=indexing
                      shift-right: [w2585] -> w2582
                      shift-left: w2580 -> [w2584]
                      n851 = Enqueue Element(queue=w2584, element=w2583) -> (queue out=w2585:refnum<queue>)  [unwired: 2 in, 2 out]
                    }
                  }
                  frame True {
                    n852 = for {
                      shift-right: [w2590] -> w2588
                      shift-left: w2586 -> [w2591]
                      tunnel: string[] ["CAM CLOSE", "DISPOSE CAM BUFFERS", "DISPOSE PROC BUFFERS", "RESET FLAGS"] -> [w2589] mode=indexing
                      n853 = Enqueue Element(queue=w2591, element=w2589) -> (queue out=w2590:refnum<queue>)  [unwired: 2 in, 2 out]
                    }
                  }
                }
                n854 = Or(x=w2574, y=w2573) -> (x .or. y?=w2576:bool)
                n855 = Select(t=State_Type_Definitions,_for_0.26g_versions_and_later_3."True Stop" ("Enum"), s=w2573, f=State_Type_Definitions,_for_0.26g_versions_and_later_3."Task 8I: STILL WAITING" ("Enum")) -> (s? t:f=w2570:T18)
                n856 = Select(t=w2570, s=w2576, f=State_Type_Definitions,_for_0.26g_versions_and_later_3."Task 8K: RAISE MY SWORD" ("Enum")) -> (s? t:f=w2575:T18)
              }
              frame "Exit" {
                n857 = for {
                  shift-right: [w2598] -> w2595
                  shift-left: w2592 -> [w2599]
                  tunnel: string[] ["STOP", "RESET ENCODERS", "RESET YAW", "ARDUINO MODE 0"] -> [w2597] mode=indexing
                  n858 = Enqueue Element(queue=w2599, element=w2597) -> (queue out=w2598:refnum<queue>)  [unwired: 2 in, 2 out]
                }
              }
            }
          }
          frame "Task 8I: STILL WAITING" {
            # ">>> Motor control cluster >>>"
            # ">>> yStepper command>>>"
            # ">> Manual override >>"
            n859 = Dequeue Element(queue=w2607, timeout in ms (-1)=w2606, error in (no error)=w2608) -> (element=w2605:T10)  [unwired: 3 out]
            n860 = case shown="\"Start Task 1\", Default" w2605 {
              tunnel: [w2615 State_Type_Definitions,_for_0.26g_versions_and_later_3."True Stop" ("Enum")] -> w2609
              tunnel: [w2617 w2634] -> w2610
              tunnel: [State_Type_Definitions,_for_0.26g_versions_and_later_3."Idle" ("Enum") State_Type_Definitions,_for_0.26g_versions_and_later_3."Shutdown" ("Enum")] -> w2611
              tunnel: w2604 -> [w2612 _]
              tunnel: w2603 -> [w2613 w2631]
              frame "Start Task 1", Default {
                # "Stays in Task 5_A until stepper reaches desired \nheight"
                # "T: Go back to idle, F: Continue with task\""
                # ">> Manual override >>"
                n861 = case shown="True" w2612 {
                  tunnel: [w2621 w2627] -> w2617
                  tunnel: w2613 -> [w2619 w2625]
                  frame False {
                    n862 = for {
                      tunnel: string[] ["READ NAVX", "READ IR"] ("element") -> [w2622] mode=indexing
                      shift-right: [w2624] -> w2621
                      shift-left: w2619 -> [w2623]
                      n863 = Enqueue Element(queue=w2623, element=w2622) -> (queue out=w2624:refnum<queue>)  [unwired: 2 in, 2 out]
                    }
                  }
                  frame True {
                    n864 = for {
                      shift-right: [w2629] -> w2627
                      shift-left: w2625 -> [w2630]
                      tunnel: string[] ["RESET ENCODERS", "RESET YAW", "RESET FLAGS", ""] -> [w2628] mode=indexing
                      n865 = Enqueue Element(queue=w2630, element=w2628) -> (queue out=w2629:refnum<queue>)  [unwired: 2 in, 2 out]
                    }
                  }
                }
                n866 = Select(t=State_Type_Definitions,_for_0.26g_versions_and_later_3."True Stop" ("Enum"), s=w2612, f=State_Type_Definitions,_for_0.26g_versions_and_later_3."Task 8I: STILL WAITING" ("Enum")) -> (s? t:f=w2615:T18)
              }
              frame "Exit" {
                n867 = for {
                  shift-right: [w2637] -> w2634
                  shift-left: w2631 -> [w2638]
                  tunnel: string[] ["STOP", "RESET ENCODERS", "RESET YAW", "ARDUINO MODE 0"] -> [w2636] mode=indexing
                  n868 = Enqueue Element(queue=w2638, element=w2636) -> (queue out=w2637:refnum<queue>)  [unwired: 2 in, 2 out]
                }
              }
            }
          }
          frame "Task 8L: Return to position" {
            # ">>> Motor control cluster >>>"
            # ">>> yStepper command>>>"
            # ">> Manual override >>"
            n869 = call "yDistance travelled FGV.vi"("Init/Read/Write State"=States_for_Action_Engine."Read") -> ("Output"=w2643:dbl)  [unwired: 9 in, 1 out]
            n870 = Dequeue Element(queue=w2652, timeout in ms (-1)=w2651, error in (no error)=w2653) -> (element=w2650:T10)  [unwired: 3 out]
            n871 = Multiply(x=w2643, y=-1.0) -> (x*y=w2640:dbl)
            n872 = Less Or Equal?(x=w2641, y=w2640) -> (x <= y?=w2639:bool)
            n873 = case shown="\"Start Task 1\", Default" w2650 {
              tunnel: [w2662 State_Type_Definitions,_for_0.26g_versions_and_later_3."True Stop" ("Enum")] -> w2654
              tunnel: [w2664 w2681] -> w2655
              tunnel: [State_Type_Definitions,_for_0.26g_versions_and_later_3."Idle" ("Enum") State_Type_Definitions,_for_0.26g_versions_and_later_3."Shutdown" ("Enum")] -> w2656
              tunnel: w2649 -> [w2658 _]
              tunnel: w2648 -> [w2660 w2678]
              tunnel: w2639 -> [w2659 _]
              frame "Start Task 1", Default {
                # "Stays in Task 5_A until stepper reaches desired \nheight"
                # "T: Go back to idle, F: Continue with task\""
                # ">> Manual override >>"
                n874 = Or(x=w2659, y=w2658) -> (x .or. y?=w2657:bool)
                n875 = case shown="False" w2657 {
                  tunnel: [w2668 w2674] -> w2664
                  tunnel: w2660 -> [w2666 w2672]
                  frame False {
                    n876 = for {
                      tunnel: string[] ["READ NAVX", "LEFT"] ("element") -> [w2669] mode=indexing
                      shift-right: [w2671] -> w2668
                      shift-left: w2666 -> [w2670]
                      n877 = Enqueue Element(queue=w2670, element=w2669) -> (queue out=w2671:refnum<queue>)  [unwired: 2 in, 2 out]
                    }
                  }
                  frame True {
                    n878 = for {
                      shift-right: [w2676] -> w2674
                      shift-left: w2672 -> [w2677]
                      tunnel: string[] ["RESET ENCODERS", "RESET YAW", "RESET FLAGS", ""] -> [w2675] mode=indexing
                      n879 = Enqueue Element(queue=w2677, element=w2675) -> (queue out=w2676:refnum<queue>)  [unwired: 2 in, 2 out]
                    }
                  }
                }
                n880 = Select(t=State_Type_Definitions,_for_0.26g_versions_and_later_3."True Stop" ("Enum"), s=w2657, f=State_Type_Definitions,_for_0.26g_versions_and_later_3."Task 8L: Return to position" ("Enum")) -> (s? t:f=w2662:T18)
              }
              frame "Exit" {
                n881 = for {
                  shift-right: [w2684] -> w2681
                  shift-left: w2678 -> [w2685]
                  tunnel: string[] ["STOP", "RESET ENCODERS", "RESET YAW", "ARDUINO MODE 0"] -> [w2683] mode=indexing
                  n882 = Enqueue Element(queue=w2685, element=w2683) -> (queue out=w2684:refnum<queue>)  [unwired: 2 in, 2 out]
                }
              }
            }
          }
          frame "Task 9A: Raise Arm" {
            # ">>> Motor control cluster >>>"
            # ">> Stepper height reeached >>"
            # ">>> yStepper command>>>"
            # ">> Manual override >>"
            n883 = Dequeue Element(queue=w2698, timeout in ms (-1)=w2693, error in (no error)=w2697) -> (element=w2700:T10)  [unwired: 3 out]
            n884 = Equal?(x=w2695, y=u8 40) -> (x = y?=w2686:bool)
            n885 = case shown="\"Start Task 1\", Default" w2700 {
              tunnel: [w2711 State_Type_Definitions,_for_0.26g_versions_and_later_3."True Stop" ("Enum")] -> w2691
              tunnel: [w2709 w2726] -> w2690
              tunnel: w2694 -> [w2708 _]
              tunnel: w2696 -> [w2702 _]
              tunnel: [State_Type_Definitions,_for_0.26g_versions_and_later_3."Idle" ("Enum") State_Type_Definitions,_for_0.26g_versions_and_later_3."Shutdown" ("Enum")] -> w2692
              tunnel: w2686 -> [w2701 _]
              frame "Start Task 1", Default {
                # ">> WIill proceed to part ii if not manual override >>"
                # ">>If ENABLE or Trigger is set to true>>"
                n886 = Or(x=w2701, y=w2702) -> (x .or. y?=w2703:bool)
                n887 = case shown="False" w2701 {
                  tunnel: [w2714 w2720] -> w2709
                  tunnel: w2708 -> [w2713 w2719]
                  frame False {
                    n888 = for {
                      shift-right: [w2716] -> w2714
                      shift-left: w2713 -> [w2717]
                      tunnel: string[] ["Z STEPPER BOX HEIGHT", "READ STEPPER VALUES"] ("element") -> [w2715] mode=indexing
                      n889 = Enqueue Element(queue=w2717, element=w2715) -> (queue out=w2716:refnum<queue>)  [unwired: 2 in, 2 out]
                    }
                  }
                  frame True {
                    n890 = for {
                      shift-right: [w2722] -> w2720
                      shift-left: w2719 -> [w2723]
                      tunnel: string[] ["READ NAVX", "RESET FLAGS", "RESET YAW", "", "", ""] -> [w2721] mode=indexing
                      n891 = Enqueue Element(queue=w2723, element=w2721) -> (queue out=w2722:refnum<queue>)  [unwired: 2 in, 2 out]
                    }
                  }
                }
                n892 = Select(t=State_Type_Definitions,_for_0.26g_versions_and_later_3."True Stop" ("Enum"), s=w2702, f=State_Type_Definitions,_for_0.26g_versions_and_later_3."Task 9B: Rotate to Angle" ("Enum")) -> (s? t:f=w2705:T18)
                n893 = Select(t=w2705, s=w2703, f=State_Type_Definitions,_for_0.26g_versions_and_later_3."Task 9A: Raise Arm" ("Enum")) -> (s? t:f=w2711:T18)
              }
              frame "Exit" {
                n894 = for {
                  shift-right: [w2729] -> w2726
                  shift-left: _ -> [w2730]
                  tunnel: string[] ["STOP", "RESET ENCODERS", "RESET YAW", ""] -> [w2728] mode=indexing
                  n895 = Enqueue Element(queue=w2730, element=w2728) -> (queue out=w2729:refnum<queue>)  [unwired: 2 in, 2 out]
                }
              }
            }
          }
          frame "Task 9B: Rotate to Angle" {
            # ">>> Motor control cluster >>>"
            # ">>> yStepper command>>>"
            n896 = Dequeue Element(queue=w2744, timeout in ms (-1)=w2743, error in (no error)=w2742) -> (element=w2746:T10)  [unwired: 3 out]
            n897 = In Range and Coerce(upper limit=65.0, x=w2736, lower limit=60.0) -> (In Range?=w2731:bool)  [unwired: 1 out]
            n898 = case shown="\"Start Task 1\", Default" w2746 {
              tunnel: w2737 -> [w2749 _]
              tunnel: [w2757 State_Type_Definitions,_for_0.26g_versions_and_later_3."True Stop" ("Enum")] -> w2739
              tunnel: w2745 -> [w2755 w2773]
              tunnel: [w2754 w2772] -> w2738
              tunnel: [State_Type_Definitions,_for_0.26g_versions_and_later_3."Idle" ("Enum") State_Type_Definitions,_for_0.26g_versions_and_later_3."Shutdown" ("Enum")] -> w2740
              tunnel: w2731 -> [w2747 _]
              frame "Start Task 1", Default {
                n899 = Or(x=w2747, y=w2749) -> (x .or. y?=w2748:bool)
                n900 = case shown="False" w2747 {
                  tunnel: w2755 -> [w2760 w2766]
                  tunnel: [w2759 w2764] -> w2754
                  frame False {
                    n901 = for {
                      shift-right: [w2762] -> w2759
                      shift-left: w2760 -> [w2763]
                      tunnel: string[] ["READ NAVX", "R-CW", ""] ("element") -> [w2761] mode=indexing
                      n902 = Enqueue Element(queue=w2763, element=w2761) -> (queue out=w2762:refnum<queue>)  [unwired: 2 in, 2 out]
                    }
                  }
                  frame True {
                    n903 = for {
                      shift-right: [w2768] -> w2764
                      shift-left: w2766 -> [w2769]
                      tunnel: string[] ["STOP", "RESET ENCODERS", "RESET YAW", "RESET FLAGS", ""] -> [w2767] mode=indexing
                      n904 = Enqueue Element(queue=w2769, element=w2767) -> (queue out=w2768:refnum<queue>)  [unwired: 2 in, 2 out]
                    }
                  }
                }
                n905 = Select(t=State_Type_Definitions,_for_0.26g_versions_and_later_3."True Stop" ("Enum"), s=w2749, f=State_Type_Definitions,_for_0.26g_versions_and_later_3."Task 9C: Detect Box") -> (s? t:f=w2751:T18)
                n906 = Select(t=w2751, s=w2748, f=State_Type_Definitions,_for_0.26g_versions_and_later_3."Task 9B: Rotate to Angle" ("Enum")) -> (s? t:f=w2757:T18)
              }
              frame "Exit" {
                n907 = for {
                  shift-right: [w2776] -> w2772
                  shift-left: w2773 -> [w2777]
                  tunnel: string[] ["STOP", "RESET ENCODERS", "RESET YAW", ""] -> [w2775] mode=indexing
                  n908 = Enqueue Element(queue=w2777, element=w2775) -> (queue out=w2776:refnum<queue>)  [unwired: 2 in, 2 out]
                }
              }
            }
          }
          frame "Task 9C: Detect Box" {
            # ">>> Motor control cluster >>>"
            # ">>Line Detected>>"
            # ">>Action Queue>>"
            # ">>> yStepper command>>>"
            n909 = Dequeue Element(queue=w2789, timeout in ms (-1)=w2788, error in (no error)=w2787) -> (element=w2790:T10)  [unwired: 3 out]
            n910 = case shown="\"Start Task 1\", Default" w2790 {
              tunnel: w2785 -> [w2791 _]
              tunnel: [w2801 State_Type_Definitions,_for_0.26g_versions_and_later_3."True Stop" ("Enum")] -> w2782
              tunnel: w2786 -> [w2799 w2817]
              tunnel: [w2798 w2816] -> w2781
              tunnel: [State_Type_Definitions,_for_0.26g_versions_and_later_3."Idle" ("Enum") State_Type_Definitions,_for_0.26g_versions_and_later_3."Shutdown" ("Enum")] -> w2784
              tunnel: w2778 -> [w2792 _]
              frame "Start Task 1", Default {
                n911 = Or(x=w2791, y=w2792) -> (x .or. y?=w2793:bool)
                n912 = case shown="False" w2792 {
                  tunnel: w2799 -> [w2804 w2810]
                  tunnel: [w2803 w2808] -> w2798
                  frame False {
                    n913 = for {
                      shift-right: [w2806] -> w2803
                      shift-left: w2804 -> [w2807]
                      tunnel: string[] ["READ IR", "READ LINE SENSOR", "FORWARD - IR ASSIST", "READ NAVX"] ("element") -> [w2805] mode=indexing
                      n914 = Enqueue Element(queue=w2807, element=w2805) -> (queue out=w2806:refnum<queue>)  [unwired: 2 in, 2 out]
                    }
                  }
                  frame True {
                    n915 = for {
                      shift-right: [w2812] -> w2808
                      shift-left: w2810 -> [w2813]
                      tunnel: string[] ["STOP", "RESET ENCODERS", "RESET YAW", "RESET FLAGS", "ARDUINO - ULTRASONIC"] -> [w2811] mode=indexing
                      n916 = Enqueue Element(queue=w2813, element=w2811) -> (queue out=w2812:refnum<queue>)  [unwired: 2 in, 2 out]
                    }
                  }
                }
                n917 = Select(t=State_Type_Definitions,_for_0.26g_versions_and_later_3."True Stop" ("Enum"), s=w2791, f=State_Type_Definitions,_for_0.26g_versions_and_later_3."Task 9D: MOVE FORWARD") -> (s? t:f=w2795:T18)
                n918 = Select(t=w2795, s=w2793, f=State_Type_Definitions,_for_0.26g_versions_and_later_3."Task 9C: Detect Box" ("Enum")) -> (s? t:f=w2801:T18)
              }
              frame "Exit" {
                n919 = for {
                  shift-right: [w2820] -> w2816
                  shift-left: w2817 -> [w2821]
                  tunnel: string[] ["STOP", "RESET ENCODERS", "RESET YAW", ""] -> [w2819] mode=indexing
                  n920 = Enqueue Element(queue=w2821, element=w2819) -> (queue out=w2820:refnum<queue>)  [unwired: 2 in, 2 out]
                }
              }
            }
          }
          frame "Task 9D: MOVE FORWARD" {
            (unwired) u8 50 ("y")
            # "Use 20 low voltage\nUse 25 high voltage"
            # ">> Item Selection Bias >>"
            # ">> Wall detected >>"
            # ">> Manual override >>"
            # ">>Table Detected>>"
            # ">>> Motor control cluster >>>"
            # ">>Table or wall detectected>>"
            # ">>Action Queue>>"
            # ">>> yStepper command>>>"
            n921 = Dequeue Element(queue=w2843, timeout in ms (-1)=w2842, error in (no error)=w2841) -> (element=w2844:T10)  [unwired: 3 out]
            n922 = Less Or Equal?(x=w2832, y=25.0) -> (x <= y?=w2828:bool)
            n923 = Less?(x=w2830, y=625.0) -> (x < y?=w2824:bool)
            n924 = Greater Or Equal?(x=w2826, y=620.0) -> (x >= y?=w2825:bool)
            n925 = And(x=w2824, y=w2825) -> (x .and. y?=w2823:bool)
            n926 = Or(x=w2828, y=w2823) -> (x .or. y?=w2827:bool)
            n927 = case shown="\"Start Task 1\", Default" w2844 {
              tunnel: w2839 -> [w2845 _]
              tunnel: [w2855 State_Type_Definitions,_for_0.26g_versions_and_later_3."True Stop" ("Enum")] -> w2836
              tunnel: w2840 -> [w2853 w2871]
              tunnel: [w2852 w2870] -> w2835
              tunnel: [State_Type_Definitions,_for_0.26g_versions_and_later_3."Idle" ("Enum") State_Type_Definitions,_for_0.26g_versions_and_later_3."Shutdown" ("Enum")] -> w2838
              tunnel: w2827 -> [w2846 _]
              frame "Start Task 1", Default {
                n928 = Or(x=w2845, y=w2846) -> (x .or. y?=w2847:bool)
                n929 = case shown="True" w2846 {
                  tunnel: w2853 -> [w2858 w2864]
                  tunnel: [w2857 w2862] -> w2852
                  frame False {
                    n930 = for {
                      shift-right: [w2860] -> w2857
                      shift-left: w2858 -> [w2861]
                      tunnel: string[] ["READ IR", "FORWARD - IR ASSIST", "READ ENCODERS", "READ NAVX"] ("element") -> [w2859] mode=indexing
                      n931 = Enqueue Element(queue=w2861, element=w2859) -> (queue out=w2860:refnum<queue>)  [unwired: 2 in, 2 out]
                    }
                  }
                  frame True {
                    n932 = for {
                      shift-right: [w2866] -> w2862
                      shift-left: w2864 -> [w2867]
                      tunnel: string[] ["STOP", "RESET ENCODERS", "RESET YAW", "RESET FLAGS"] -> [w2865] mode=indexing
                      n933 = Enqueue Element(queue=w2867, element=w2865) -> (queue out=w2866:refnum<queue>)  [unwired: 2 in, 2 out]
                    }
                  }
                }
                n934 = Select(t=State_Type_Definitions,_for_0.26g_versions_and_later_3."True Stop" ("Enum"), s=w2845, f=State_Type_Definitions,_for_0.26g_versions_and_later_3."Task 9D2: ANGLE CORRECTION") -> (s? t:f=w2849:T18)
                n935 = Select(t=w2849, s=w2847, f=State_Type_Definitions,_for_0.26g_versions_and_later_3."Task 9D: MOVE FORWARD" ("Enum")) -> (s? t:f=w2855:T18)
              }
              frame "Exit" {
                n936 = for {
                  shift-right: [w2874] -> w2870
                  shift-left: w2871 -> [w2875]
                  tunnel: string[] ["STOP", "RESET ENCODERS", "RESET YAW", ""] -> [w2873] mode=indexing
                  n937 = Enqueue Element(queue=w2875, element=w2873) -> (queue out=w2874:refnum<queue>)  [unwired: 2 in, 2 out]
                }
              }
            }
          }
          frame "Task 9D2: ANGLE CORRECTION" {
            # "Min: 48 ~ 50\nMax: 52 ~ 54"
            # ">>> Motor control cluster >>>"
            # ">>> yStepper command>>>"
            n938 = Dequeue Element(queue=w2889, timeout in ms (-1)=w2888, error in (no error)=w2887) -> (element=w2891:T10)  [unwired: 3 out]
            n939 = In Range and Coerce(upper limit=54.0, x=w2881, lower limit=50.0) -> (In Range?=w2876:bool)  [unwired: 1 out]
            n940 = case shown="\"Start Task 1\", Default" w2891 {
              tunnel: w2882 -> [w2894 _]
              tunnel: [w2902 State_Type_Definitions,_for_0.26g_versions_and_later_3."True Stop" ("Enum")] -> w2884
              tunnel: w2890 -> [w2900 w2918]
              tunnel: [w2899 w2917] -> w2883
              tunnel: [State_Type_Definitions,_for_0.26g_versions_and_later_3."Idle" ("Enum") State_Type_Definitions,_for_0.26g_versions_and_later_3."Shutdown" ("Enum")] -> w2885
              tunnel: w2876 -> [w2892 _]
              frame "Start Task 1", Default {
                n941 = Or(x=w2892, y=w2894) -> (x .or. y?=w2893:bool)
                n942 = case shown="False" w2892 {
                  tunnel: w2900 -> [w2905 w2911]
                  tunnel: [w2904 w2909] -> w2899
                  frame False {
                    n943 = for {
                      shift-right: [w2907] -> w2904
                      shift-left: w2905 -> [w2908]
                      tunnel: string[] ["READ NAVX", "R-ACW", ""] ("element") -> [w2906] mode=indexing
                      n944 = Enqueue Element(queue=w2908, element=w2906) -> (queue out=w2907:refnum<queue>)  [unwired: 2 in, 2 out]
                    }
                  }
                  frame True {
                    n945 = for {
                      shift-right: [w2913] -> w2909
                      shift-left: w2911 -> [w2914]
                      tunnel: string[] ["STOP", "RESET ENCODERS", "RESET YAW", "", ""] -> [w2912] mode=indexing
                      n946 = Enqueue Element(queue=w2914, element=w2912) -> (queue out=w2913:refnum<queue>)  [unwired: 2 in, 2 out]
                    }
                  }
                }
                n947 = Select(t=State_Type_Definitions,_for_0.26g_versions_and_later_3."True Stop" ("Enum"), s=w2894, f=State_Type_Definitions,_for_0.26g_versions_and_later_3."Task 9E: MOVE LEFT") -> (s? t:f=w2896:T18)
                n948 = Select(t=w2896, s=w2893, f=State_Type_Definitions,_for_0.26g_versions_and_later_3."Task 9D2: ANGLE CORRECTION" ("Enum")) -> (s? t:f=w2902:T18)
              }
              frame "Exit" {
                n949 = for {
                  shift-right: [w2921] -> w2917
                  shift-left: w2918 -> [w2922]
                  tunnel: string[] ["STOP", "RESET ENCODERS", "RESET YAW", ""] -> [w2920] mode=indexing
                  n950 = Enqueue Element(queue=w2922, element=w2920) -> (queue out=w2921:refnum<queue>)  [unwired: 2 in, 2 out]
                }
              }
            }
          }
          frame "Task 9E: MOVE LEFT" {
            # "High battery voltage: 15"
            # ">> Item Selection Bias >>"
            # ">>Stops if either table or wall is obstructing >>"
            n951 = Less?(x=w2923, y=15.0) -> (x < y?=w2933:bool)
            n952 = Dequeue Element(queue=w2931, timeout in ms (-1)=w2930, error in (no error)=w2929) -> (element=w2935:T10)  [unwired: 3 out]
            n953 = case shown="\"Start Task 1\", Default" w2935 {
              tunnel: w2933 -> [w2940 _]
              tunnel: [w2947 State_Type_Definitions,_for_0.26g_versions_and_later_3."True Stop" ("Enum")] -> w2925
              tunnel: w2928 -> [w2939 _]
              tunnel: w2932 -> [w2946 w2963]
              tunnel: [w2945 w2964] -> w2926
              tunnel: [State_Type_Definitions,_for_0.26g_versions_and_later_3."Idle" ("Enum") State_Type_Definitions,_for_0.26g_versions_and_later_3."Shutdown" ("Enum")] -> w2924
              frame "Start Task 1", Default {
                n954 = case shown="False" w2940 {
                  tunnel: w2946 -> [w2950 w2957]
                  tunnel: [w2951 w2956] -> w2945
                  frame False {
                    n955 = for {
                      tunnel: string[] ["LEFT", "READ NAVX", "READ IR", ""] ("element") -> [w2952] mode=indexing
                      shift-right: [w2954] -> w2951
                      shift-left: w2950 -> [w2953]
                      n956 = Enqueue Element(queue=w2953, element=w2952) -> (queue out=w2954:refnum<queue>)  [unwired: 2 in, 2 out]
                    }
                  }
                  frame True {
                    n957 = for {
                      shift-right: [w2959] -> w2956
                      shift-left: w2957 -> [w2960]
                      tunnel: string[] ["STOP", "RESET ENCODERS", "RESET FLAGS", "RESET YAW", "READ IR", ""] -> [w2958] mode=indexing
                      n958 = Enqueue Element(queue=w2960, element=w2958) -> (queue out=w2959:refnum<queue>)  [unwired: 2 in, 2 out]
                    }
                  }
                }
                n959 = Or(x=w2940, y=w2939) -> (x .or. y?=w2938:bool)
                n960 = Select(t=State_Type_Definitions,_for_0.26g_versions_and_later_3."True Stop" ("Enum"), s=w2939, f=State_Type_Definitions,_for_0.26g_versions_and_later_3."Task 9E2: MOVE RIGHT" ("Enum")) -> (s? t:f=w2941:T18)
                n961 = Select(t=w2941, s=w2938, f=State_Type_Definitions,_for_0.26g_versions_and_later_3."Task 9E: MOVE LEFT" ("Enum")) -> (s? t:f=w2947:T18)
              }
              frame "Exit" {
                n962 = for {
                  shift-right: [w2967] -> w2964
                  shift-left: w2963 -> [w2968]
                  tunnel: string[] ["STOP", "RESET ENCODERS", "RESET YAW", "ARDUINO MODE 0"] -> [w2966] mode=indexing
                  n963 = Enqueue Element(queue=w2968, element=w2966) -> (queue out=w2967:refnum<queue>)  [unwired: 2 in, 2 out]
                }
              }
            }
          }
          frame "Task 9E2: MOVE RIGHT" {
            # ">>> Motor control cluster >>>"
            # ">>> yStepper command>>>"
            n964 = Dequeue Element(queue=w2976, timeout in ms (-1)=w2975, error in (no error)=w2974) -> (element=w2981:T10)  [unwired: 3 out]
            n965 = case shown="\"Start Task 1\", Default" w2981 {
              tunnel: w2969 -> [w2984 _]
              tunnel: [w2991 State_Type_Definitions,_for_0.26g_versions_and_later_3."True Stop" ("Enum")] -> w2980
              tunnel: w2973 -> [w2983 _]
              tunnel: w2977 -> [w2990 w3007]
              tunnel: [w2989 w3008] -> w2979
              tunnel: [State_Type_Definitions,_for_0.26g_versions_and_later_3."Idle" ("Enum") State_Type_Definitions,_for_0.26g_versions_and_later_3."Shutdown" ("Enum")] -> w2978
              frame "Start Task 1", Default {
                n966 = case shown="True" w2984 {
                  tunnel: w2990 -> [w2994 w3001]
                  tunnel: [w2995 w3000] -> w2989
                  frame False {
                    n967 = for {
                      tunnel: string[] ["READ LINE SENSOR", "READ NAVX", "RIGHT", "READ ENCODERS"] ("element") -> [w2996] mode=indexing
                      shift-right: [w2998] -> w2995
                      shift-left: w2994 -> [w2997]
                      n968 = Enqueue Element(queue=w2997, element=w2996) -> (queue out=w2998:refnum<queue>)  [unwired: 2 in, 2 out]
                    }
                  }
                  frame True {
                    n969 = for {
                      shift-right: [w3003] -> w3000
                      shift-left: w3001 -> [w3004]
                      tunnel: string[] ["RESET ENCODERS", "RESET YAW", "RESET FLAGS", "STOP", "BOX COLOUR"] -> [w3002] mode=indexing
                      n970 = Enqueue Element(queue=w3004, element=w3002) -> (queue out=w3003:refnum<queue>)  [unwired: 2 in, 2 out]
                    }
                  }
                }
                n971 = Or(x=w2984, y=w2983) -> (x .or. y?=w2982:bool)
                n972 = Select(t=State_Type_Definitions,_for_0.26g_versions_and_later_3."True Stop" ("Enum"), s=w2983, f=State_Type_Definitions,_for_0.26g_versions_and_later_3."Task 9F: SCAN BOX" ("Enum")) -> (s? t:f=w2985:T18)
                n973 = Select(t=w2985, s=w2982, f=State_Type_Definitions,_for_0.26g_versions_and_later_3."Task 9E2: MOVE RIGHT" ("Enum")) -> (s? t:f=w2991:T18)
              }
              frame "Exit" {
                n974 = for {
                  shift-right: [w3011] -> w3008
                  shift-left: w3007 -> [w3012]
                  tunnel: string[] ["STOP", "RESET ENCODERS", "RESET YAW", "ARDUINO MODE 0"] -> [w3010] mode=indexing
                  n975 = Enqueue Element(queue=w3012, element=w3010) -> (queue out=w3011:refnum<queue>)  [unwired: 2 in, 2 out]
                }
              }
            }
          }
          frame "Task 9F: SCAN BOX" {
            # ">>> Motor control cluster >>>"
            # ">>Colour detection >>"
            # ">>> yStepper command>>>"
            # ">> Manual override >>"
            n976 = Dequeue Element(queue=w3029, timeout in ms (-1)=w3027, error in (no error)=w3028) -> (element=w3022:T10)  [unwired: 3 out]
            n977 = call "Box Colour FGV.vi"("Init/R/W State"=Box_Colour_FGV_States."Read") -> ("Colour to detect (output)"=w3015:T2)  [unwired: 9 in, 1 out]
            n978 = Equal?(x=w3016, y=w3015) -> (x = y?=w3014:bool)
            n979 = case shown="\"Start Task 1\", Default" w3022 {
              tunnel: [w3042 State_Type_Definitions,_for_0.26g_versions_and_later_3."True Stop" ("Enum")] -> w3019
              tunnel: [w3040 w3057] -> w3020
              tunnel: w3021 -> [w3039 _]
              tunnel: w3023 -> [w3032 _]
              tunnel: [State_Type_Definitions,_for_0.26g_versions_and_later_3."Idle" ("Enum") State_Type_Definitions,_for_0.26g_versions_and_later_3."Shutdown" ("Enum")] -> w3018
              tunnel: w3013 -> [w3033 _]
              tunnel: w3014 -> [w3031 _]
              frame "Start Task 1", Default {
                # ">> Will stop either due to manual override or is same box colour >>"
                # ">> WIill proceed to part ii if not manual override >>"
                # ">>If ENABLE or Trigger is set to true>>"
                n980 = Or(x=w3033, y=w3032) -> (x .or. y?=w3034:bool)
                n981 = case shown="True" w3033 {
                  tunnel: [w3045 w3051] -> w3040
                  tunnel: w3039 -> [w3044 w3050]
                  frame False {
                    n982 = for {
                      shift-right: [w3047] -> w3045
                      shift-left: w3044 -> [w3048]
                      tunnel: string[] ["", ""] ("element") -> [w3046] mode=indexing
                      n983 = Enqueue Element(queue=w3048, element=w3046) -> (queue out=w3047:refnum<queue>)  [unwired: 2 in, 2 out]
                    }
                  }
                  frame True {
                    n984 = for {
                      shift-right: [w3053] -> w3051
                      shift-left: w3050 -> [w3054]
                      tunnel: string[] ["RESET ENCODER", "RESET FLAGS", "RESET YAW", "", "", ""] -> [w3052] mode=indexing
                      n985 = Enqueue Element(queue=w3054, element=w3052) -> (queue out=w3053:refnum<queue>)  [unwired: 2 in, 2 out]
                    }
                  }
                }
                n986 = Or(x=w3032, y=w3031) -> (x .or. y?=w3030:bool)
                n987 = Select(t=State_Type_Definitions,_for_0.26g_versions_and_later_3."True Stop" ("Enum"), s=w3030, f=State_Type_Definitions,_for_0.26g_versions_and_later_3."Task 9G: MOVE RIGHT" ("Enum")) -> (s? t:f=w3036:T18)
                n988 = Select(t=w3036, s=w3034, f=State_Type_Definitions,_for_0.26g_versions_and_later_3."Task 9F: SCAN BOX" ("Enum")) -> (s? t:f=w3042:T18)
              }
              frame "Exit" {
                n989 = for {
                  shift-right: [w3060] -> w3057
                  shift-left: _ -> [w3061]
                  tunnel: string[] ["STOP", "RESET ENCODERS", "RESET YAW", ""] -> [w3059] mode=indexing
                  n990 = Enqueue Element(queue=w3061, element=w3059) -> (queue out=w3060:refnum<queue>)  [unwired: 2 in, 2 out]
                }
              }
            }
          }
          frame "Task 9G: MOVE RIGHT" {
            # ">>> Motor control cluster >>>"
            # ">>> yStepper command>>>"
            n991 = Dequeue Element(queue=w3073, timeout in ms (-1)=w3072, error in (no error)=w3071) -> (element=w3078:T10)  [unwired: 3 out]
            n992 = Greater?(x=w3063, y=50.0) -> (0:w3066:bool)
            n993 = And(x=w3064, y=w3066) -> (x .and. y?=w3062:bool)
            n994 = case shown="\"Start Task 1\", Default" w3078 {
              tunnel: w3062 -> [w3081 _]
              tunnel: [w3088 State_Type_Definitions,_for_0.26g_versions_and_later_3."True Stop" ("Enum")] -> w3077
              tunnel: w3070 -> [w3080 _]
              tunnel: w3074 -> [w3087 w3104]
              tunnel: [w3086 w3105] -> w3076
              tunnel: [State_Type_Definitions,_for_0.26g_versions_and_later_3."Idle" ("Enum") State_Type_Definitions,_for_0.26g_versions_and_later_3."Shutdown" ("Enum")] -> w3075
              frame "Start Task 1", Default {
                n995 = case shown="True" w3081 {
                  tunnel: w3087 -> [w3091 w3098]
                  tunnel: [w3092 w3097] -> w3086
                  frame False {
                    n996 = for {
                      tunnel: string[] ["READ LINE SENSOR", "READ NAVX", "RIGHT", "READ ENCODERS"] ("element") -> [w3093] mode=indexing
                      shift-right: [w3095] -> w3092
                      shift-left: w3091 -> [w3094]
                      n997 = Enqueue Element(queue=w3094, element=w3093) -> (queue out=w3095:refnum<queue>)  [unwired: 2 in, 2 out]
                    }
                  }
                  frame True {
                    n998 = for {
                      shift-right: [w3100] -> w3097
                      shift-left: w3098 -> [w3101]
                      tunnel: string[] ["RESET ENCODERS", "RESET YAW", "RESET FLAGS", "STOP", "BOX COLOUR"] -> [w3099] mode=indexing
                      n999 = Enqueue Element(queue=w3101, element=w3099) -> (queue out=w3100:refnum<queue>)  [unwired: 2 in, 2 out]
                    }
                  }
                }
                n1000 = Or(x=w3081, y=w3080) -> (x .or. y?=w3079:bool)
                n1001 = Select(t=State_Type_Definitions,_for_0.26g_versions_and_later_3."True Stop" ("Enum"), s=w3080, f=State_Type_Definitions,_for_0.26g_versions_and_later_3."Task 9H: SCAN BOX 2" ("Enum")) -> (s? t:f=w3082:T18)
                n1002 = Select(t=w3082, s=w3079, f=State_Type_Definitions,_for_0.26g_versions_and_later_3."Task 9G: MOVE RIGHT" ("Enum")) -> (s? t:f=w3088:T18)
              }
              frame "Exit" {
                n1003 = for {
                  shift-right: [w3108] -> w3105
                  shift-left: w3104 -> [w3109]
                  tunnel: string[] ["STOP", "RESET ENCODERS", "RESET YAW", "ARDUINO MODE 0"] -> [w3107] mode=indexing
                  n1004 = Enqueue Element(queue=w3109, element=w3107) -> (queue out=w3108:refnum<queue>)  [unwired: 2 in, 2 out]
                }
              }
            }
          }
          frame "Task 9H: SCAN BOX 2" {
            # ">> Item Selection Bias >>"
            # ">>> Motor control cluster >>>"
            # ">>> yStepper command>>>"
            n1005 = Dequeue Element(queue=w3119, timeout in ms (-1)=w3120, error in (no error)=w3121) -> (element=w3123:T10)  [unwired: 3 out]
            n1006 = call "Box Colour FGV.vi"("Init/R/W State"=Box_Colour_FGV_States."Read") -> ("Colour to detect (output)"=w3113:T2)  [unwired: 9 in, 1 out]
            n1007 = Equal?(x=w3112, y=w3113) -> (x = y?=w3111:bool)
            n1008 = case shown="\"Start Task 1\", Default" w3123 {
              tunnel: w3110 -> [w3131 _]
              tunnel: [w3138 State_Type_Definitions,_for_0.26g_versions_and_later_3."True Stop" ("Enum")] -> w3116
              tunnel: w3122 -> [w3128 _]
              tunnel: w3118 -> [w3137 w3154]
              tunnel: [w3136 w3155] -> w3117
              tunnel: [State_Type_Definitions,_for_0.26g_versions_and_later_3."Idle" ("Enum") State_Type_Definitions,_for_0.26g_versions_and_later_3."Shutdown" ("Enum")] -> w3115
              tunnel: w3111 -> [w3129 _]
              frame "Start Task 1", Default {
                n1009 = Or(x=w3131, y=w3128) -> (x .or. y?=w3130:bool)
                n1010 = Or(x=w3129, y=w3128) -> (x .or. y?=w3127:bool)
                n1011 = case shown="True" w3131 {
                  tunnel: w3137 -> [w3141 w3148]
                  tunnel: [w3142 w3147] -> w3136
                  frame False {
                    n1012 = for {
                      tunnel: string[] ["", "", "", ""] ("element") -> [w3143] mode=indexing
                      shift-right: [w3145] -> w3142
                      shift-left: w3141 -> [w3144]
                      n1013 = Enqueue Element(queue=w3144, element=w3143) -> (queue out=w3145:refnum<queue>)  [unwired: 2 in, 2 out]
                    }
                  }
                  frame True {
                    n1014 = for {
                      shift-right: [w3150] -> w3147
                      shift-left: w3148 -> [w3151]
                      tunnel: string[] ["READ NAVX", "RESET FLAGS", "RESET ENCODERS", "", "", ""] -> [w3149] mode=indexing
                      n1015 = Enqueue Element(queue=w3151, element=w3149) -> (queue out=w3150:refnum<queue>)  [unwired: 2 in, 2 out]
                    }
                  }
                }
                n1016 = Select(t=State_Type_Definitions,_for_0.26g_versions_and_later_3."True Stop" ("Enum"), s=w3127, f=State_Type_Definitions,_for_0.26g_versions_and_later_3."Task 9I: ROTATE 90 CW" ("Enum")) -> (s? t:f=w3132:T18)
                n1017 = Select(t=w3132, s=w3130, f=State_Type_Definitions,_for_0.26g_versions_and_later_3."Task 9H: SCAN BOX 2" ("Enum")) -> (s? t:f=w3138:T18)
              }
              frame "Exit" {
                n1018 = for {
                  shift-right: [w3158] -> w3155
                  shift-left: w3154 -> [w3159]
                  tunnel: string[] ["STOP", "RESET ENCODERS", "RESET YAW", "ARDUINO MODE 0"] -> [w3157] mode=indexing
                  n1019 = Enqueue Element(queue=w3159, element=w3157) -> (queue out=w3158:refnum<queue>)  [unwired: 2 in, 2 out]
                }
              }
            }
          }
          frame "Task 9I: ROTATE 90 CW" {
            # "High battery voltage: -36\nMid voltage: -38 \nLow voltage: -40"
            # ">> Item Selection Bias >>"
            n1020 = Less Or Equal?(x=w3162, y=-38.0) -> (x <= y?=w3160:bool)
            n1021 = Dequeue Element(queue=w3163, timeout in ms (-1)=w3164, error in (no error)=w3165) -> (element=w3171:T10)  [unwired: 3 out]
            n1022 = case shown="\"Start Task 1\", Default" w3171 {
              tunnel: w3160 -> [w3177 _]
              tunnel: [w3184 State_Type_Definitions,_for_0.26g_versions_and_later_3."True Stop" ("Enum")] -> w3168
              tunnel: w3166 -> [w3176 _]
              tunnel: w3170 -> [w3183 w3200]
              tunnel: [w3182 w3201] -> w3169
              tunnel: [State_Type_Definitions,_for_0.26g_versions_and_later_3."Idle" ("Enum") State_Type_Definitions,_for_0.26g_versions_and_later_3."Shutdown" ("Enum")] -> w3167
              frame "Start Task 1", Default {
                n1023 = case shown="False" w3177 {
                  tunnel: w3183 -> [w3187 w3194]
                  tunnel: [w3188 w3193] -> w3182
                  frame False {
                    n1024 = for {
                      tunnel: string[] ["R-CW", "READ ENCODERS", "READ IR", "READ NAVX"] ("element") -> [w3189] mode=indexing
                      shift-right: [w3191] -> w3188
                      shift-left: w3187 -> [w3190]
                      n1025 = Enqueue Element(queue=w3190, element=w3189) -> (queue out=w3191:refnum<queue>)  [unwired: 2 in, 2 out]
                    }
                  }
                  frame True {
                    n1026 = for {
                      shift-right: [w3196] -> w3193
                      shift-left: w3194 -> [w3197]
                      tunnel: string[] ["STOP", "RESET ENCODERS", "RESET YAW", "RESET FLAGS", "READ IR", ""] -> [w3195] mode=indexing
                      n1027 = Enqueue Element(queue=w3197, element=w3195) -> (queue out=w3196:refnum<queue>)  [unwired: 2 in, 2 out]
                    }
                  }
                }
                n1028 = Or(x=w3177, y=w3176) -> (x .or. y?=w3175:bool)
                n1029 = Select(t=State_Type_Definitions,_for_0.26g_versions_and_later_3."True Stop" ("Enum"), s=w3176, f=State_Type_Definitions,_for_0.26g_versions_and_later_3."Task 9J: FORWARD" ("Enum")) -> (s? t:f=w3178:T18)
                n1030 = Select(t=w3178, s=w3175, f=State_Type_Definitions,_for_0.26g_versions_and_later_3."Task 9I: ROTATE 90 CW" ("Enum")) -> (s? t:f=w3184:T18)
              }
              frame "Exit" {
                n1031 = for {
                  shift-right: [w3204] -> w3201
                  shift-left: w3200 -> [w3205]
                  tunnel: string[] ["STOP", "RESET ENCODERS", "RESET YAW", "ARDUINO MODE 0"] -> [w3203] mode=indexing
                  n1032 = Enqueue Element(queue=w3205, element=w3203) -> (queue out=w3204:refnum<queue>)  [unwired: 2 in, 2 out]
                }
              }
            }
          }
          frame "Task 9J: FORWARD" {
            # "Max: 25\nMin: 18"
            # "Tried values: 70, 150"
            # ">>Stops if either table or wall is obstructing >>"
            # ">> Item Selection Bias >>"
            n1033 = Less?(x=w3208, y=150.0) -> (x < y?=w3211:bool)
            n1034 = Greater Than 0?(x=w3208) -> (x > 0?=w3210:bool)
            n1035 = Less Or Equal?(x=w3214, y=25.0) -> (x <= y?=w3212:bool)
            n1036 = Greater Than 0?(x=w3214) -> (x > 0?=w3213:bool)
            n1037 = And(x=w3210, y=w3211) -> ()  [unwired: 1 out]
            n1038 = Dequeue Element(queue=w3220, timeout in ms (-1)=w3221, error in (no error)=w3222) -> (element=w3224:T10)  [unwired: 3 out]
            n1039 = And(x=w3213, y=w3212) -> (x .and. y?=w3206:bool)
            n1040 = Or(x=w3206, y=w3206) -> (x .or. y?=w3207:bool)
            n1041 = case shown="\"Start Task 1\", Default" w3224 {
              tunnel: w3207 -> [w3230 _]
              tunnel: [w3237 State_Type_Definitions,_for_0.26g_versions_and_later_3."True Stop" ("Enum")] -> w3218
              tunnel: w3223 -> [w3229 _]
              tunnel: w3219 -> [w3236 w3253]
              tunnel: [w3235 w3254] -> w3217
              tunnel: [State_Type_Definitions,_for_0.26g_versions_and_later_3."Idle" ("Enum") State_Type_Definitions,_for_0.26g_versions_and_later_3."Shutdown" ("Enum")] -> w3216
              frame "Start Task 1", Default {
                n1042 = case shown="True" w3230 {
                  tunnel: w3236 -> [w3240 w3247]
                  tunnel: [w3241 w3246] -> w3235
                  frame False {
                    n1043 = for {
                      tunnel: string[] ["READ IR", "READ NAVX", "FORWARD"] ("element") -> [w3242] mode=indexing
                      shift-right: [w3244] -> w3241
                      shift-left: w3240 -> [w3243]
                      n1044 = Enqueue Element(queue=w3243, element=w3242) -> (queue out=w3244:refnum<queue>)  [unwired: 2 in, 2 out]
                    }
                  }
                  frame True {
                    n1045 = for {
                      shift-right: [w3249] -> w3246
                      shift-left: w3247 -> [w3250]
                      tunnel: string[] ["STOP", "RESET ENCODERS", "RESET YAW", "RESET FLAGS", "READ IR", ""] -> [w3248] mode=indexing
                      n1046 = Enqueue Element(queue=w3250, element=w3248) -> (queue out=w3249:refnum<queue>)  [unwired: 2 in, 2 out]
                    }
                  }
                }
                n1047 = Or(x=w3230, y=w3229) -> (x .or. y?=w3228:bool)
                n1048 = Select(t=State_Type_Definitions,_for_0.26g_versions_and_later_3."True Stop" ("Enum"), s=w3229, f=State_Type_Definitions,_for_0.26g_versions_and_later_3."Task 9J2: ANGLE CORRECTION" ("Enum")) -> (s? t:f=w3231:T18)
                n1049 = Select(t=w3231, s=w3228, f=State_Type_Definitions,_for_0.26g_versions_and_later_3."Task 9J: FORWARD" ("Enum")) -> (s? t:f=w3237:T18)
              }
              frame "Exit" {
                n1050 = for {
                  shift-right: [w3257] -> w3254
                  shift-left: w3253 -> [w3258]
                  tunnel: string[] ["STOP", "RESET ENCODERS", "RESET YAW", "ARDUINO MODE 0"] -> [w3256] mode=indexing
                  n1051 = Enqueue Element(queue=w3258, element=w3256) -> (queue out=w3257:refnum<queue>)  [unwired: 2 in, 2 out]
                }
              }
            }
          }
          frame "Task 9J2: ANGLE CORRECTION" {
            # "Ngee Ann Values: Min 100, Max 110"
            # ">>> Motor control cluster >>>"
            # ">>> yStepper command>>>"
            n1052 = Dequeue Element(queue=w3272, timeout in ms (-1)=w3271, error in (no error)=w3270) -> (element=w3274:T10)  [unwired: 3 out]
            n1053 = In Range and Coerce(upper limit=110.0, x=w3264, lower limit=100.0) -> (In Range?=w3259:bool)  [unwired: 1 out]
            n1054 = case shown="\"Start Task 1\", Default" w3274 {
              tunnel: w3265 -> [w3277 _]
              tunnel: [w3285 State_Type_Definitions,_for_0.26g_versions_and_later_3."True Stop" ("Enum")] -> w3267
              tunnel: w3273 -> [w3283 w3301]
              tunnel: [w3282 w3300] -> w3266
              tunnel: [State_Type_Definitions,_for_0.26g_versions_and_later_3."Idle" ("Enum") State_Type_Definitions,_for_0.26g_versions_and_later_3."Shutdown" ("Enum")] -> w3268
              tunnel: w3259 -> [w3275 _]
              frame "Start Task 1", Default {
                n1055 = Or(x=w3275, y=w3277) -> (x .or. y?=w3276:bool)
                n1056 = case shown="False" w3275 {
                  tunnel: w3283 -> [w3288 w3294]
                  tunnel: [w3287 w3292] -> w3282
                  frame False {
                    n1057 = for {
                      shift-right: [w3290] -> w3287
                      shift-left: w3288 -> [w3291]
                      tunnel: string[] ["READ NAVX", "R-ACW", ""] ("element") -> [w3289] mode=indexing
                      n1058 = Enqueue Element(queue=w3291, element=w3289) -> (queue out=w3290:refnum<queue>)  [unwired: 2 in, 2 out]
                    }
                  }
                  frame True {
                    n1059 = for {
                      shift-right: [w3296] -> w3292
                      shift-left: w3294 -> [w3297]
                      tunnel: string[] ["STOP", "RESET ENCODERS", "RESET YAW", "", ""] -> [w3295] mode=indexing
                      n1060 = Enqueue Element(queue=w3297, element=w3295) -> (queue out=w3296:refnum<queue>)  [unwired: 2 in, 2 out]
                    }
                  }
                }
                n1061 = Select(t=State_Type_Definitions,_for_0.26g_versions_and_later_3."True Stop" ("Enum"), s=w3277, f=State_Type_Definitions,_for_0.26g_versions_and_later_3."Task 9K: RAM WALL") -> (s? t:f=w3279:T18)
                n1062 = Select(t=w3279, s=w3276, f=State_Type_Definitions,_for_0.26g_versions_and_later_3."Task 9J2: ANGLE CORRECTION" ("Enum")) -> (s? t:f=w3285:T18)
              }
              frame "Exit" {
                n1063 = for {
                  shift-right: [w3304] -> w3300
                  shift-left: w3301 -> [w3305]
                  tunnel: string[] ["STOP", "RESET ENCODERS", "RESET YAW", ""] -> [w3303] mode=indexing
                  n1064 = Enqueue Element(queue=w3305, element=w3303) -> (queue out=w3304:refnum<queue>)  [unwired: 2 in, 2 out]
                }
              }
            }
          }
          frame "Task 9K: RAM WALL" {
            # "High battery voltage: 15"
            # ">> Item Selection Bias >>"
            # ">>Stops if either table or wall is obstructing >>"
            n1065 = Less?(x=w3306, y=15.0) -> (x < y?=w3316:bool)
            n1066 = Dequeue Element(queue=w3314, timeout in ms (-1)=w3313, error in (no error)=w3312) -> (element=w3318:T10)  [unwired: 3 out]
            n1067 = case shown="\"Start Task 1\", Default" w3318 {
              tunnel: w3316 -> [w3323 _]
              tunnel: [w3330 State_Type_Definitions,_for_0.26g_versions_and_later_3."True Stop" ("Enum")] -> w3308
              tunnel: w3311 -> [w3322 _]
              tunnel: w3315 -> [w3329 w3346]
              tunnel: [w3328 w3347] -> w3309
              tunnel: [State_Type_Definitions,_for_0.26g_versions_and_later_3."Idle" ("Enum") State_Type_Definitions,_for_0.26g_versions_and_later_3."Shutdown" ("Enum")] -> w3307
              frame "Start Task 1", Default {
                n1068 = case shown="True" w3323 {
                  tunnel: w3329 -> [w3333 w3340]
                  tunnel: [w3334 w3339] -> w3328
                  frame False {
                    n1069 = for {
                      tunnel: string[] ["LEFT", "READ NAVX", "READ IR", ""] ("element") -> [w3335] mode=indexing
                      shift-right: [w3337] -> w3334
                      shift-left: w3333 -> [w3336]
                      n1070 = Enqueue Element(queue=w3336, element=w3335) -> (queue out=w3337:refnum<queue>)  [unwired: 2 in, 2 out]
                    }
                  }
                  frame True {
                    n1071 = for {
                      shift-right: [w3342] -> w3339
                      shift-left: w3340 -> [w3343]
                      tunnel: string[] ["STOP", "RESET ENCODERS", "RESET FLAGS", "RESET YAW", "READ IR", ""] -> [w3341] mode=indexing
                      n1072 = Enqueue Element(queue=w3343, element=w3341) -> (queue out=w3342:refnum<queue>)  [unwired: 2 in, 2 out]
                    }
                  }
                }
                n1073 = Or(x=w3323, y=w3322) -> (x .or. y?=w3321:bool)
                n1074 = Select(t=State_Type_Definitions,_for_0.26g_versions_and_later_3."True Stop" ("Enum"), s=w3322, f=State_Type_Definitions,_for_0.26g_versions_and_later_3."Task 9L: MOVE RIGHT" ("Enum")) -> (s? t:f=w3324:T18)
                n1075 = Select(t=w3324, s=w3321, f=State_Type_Definitions,_for_0.26g_versions_and_later_3."Task 9K: RAM WALL" ("Enum")) -> (s? t:f=w3330:T18)
              }
              frame "Exit" {
                n1076 = for {
                  shift-right: [w3350] -> w3347
                  shift-left: w3346 -> [w3351]
                  tunnel: string[] ["STOP", "RESET ENCODERS", "RESET YAW", "ARDUINO MODE 0"] -> [w3349] mode=indexing
                  n1077 = Enqueue Element(queue=w3351, element=w3349) -> (queue out=w3350:refnum<queue>)  [unwired: 2 in, 2 out]
                }
              }
            }
          }
          frame "Task 9L: MOVE RIGHT" {
            # "High battery voltage: 15"
            # ">>> Motor control cluster >>>"
            # ">>> yStepper command>>>"
            # ">> Item Selection Bias >>"
            n1078 = Dequeue Element(queue=w3359, timeout in ms (-1)=w3358, error in (no error)=w3357) -> (element=w3361:T10)  [unwired: 3 out]
            n1079 = case shown="\"Start Task 1\", Default" w3361 {
              tunnel: w3352 -> [w3367 _]
              tunnel: [w3374 State_Type_Definitions,_for_0.26g_versions_and_later_3."True Stop" ("Enum")] -> w3355
              tunnel: w3356 -> [w3366 _]
              tunnel: w3360 -> [w3373 w3390]
              tunnel: [w3372 w3391] -> w3353
              tunnel: [State_Type_Definitions,_for_0.26g_versions_and_later_3."Idle" ("Enum") State_Type_Definitions,_for_0.26g_versions_and_later_3."Shutdown" ("Enum")] -> w3354
              frame "Start Task 1", Default {
                n1080 = case shown="True" w3367 {
                  tunnel: w3373 -> [w3377 w3384]
                  tunnel: [w3378 w3383] -> w3372
                  frame False {
                    n1081 = for {
                      tunnel: string[] ["RIGHT", "READ NAVX", "READ LINE SENSOR", ""] ("element") -> [w3379] mode=indexing
                      shift-right: [w3381] -> w3378
                      shift-left: w3377 -> [w3380]
                      n1082 = Enqueue Element(queue=w3380, element=w3379) -> (queue out=w3381:refnum<queue>)  [unwired: 2 in, 2 out]
                    }
                  }
                  frame True {
                    n1083 = for {
                      shift-right: [w3386] -> w3383
                      shift-left: w3384 -> [w3387]
                      tunnel: string[] ["STOP", "RESET ENCODERS", "RESET FLAGS", "RESET YAW", "BOX COLOUR", ""] -> [w3385] mode=indexing
                      n1084 = Enqueue Element(queue=w3387, element=w3385) -> (queue out=w3386:refnum<queue>)  [unwired: 2 in, 2 out]
                    }
                  }
                }
                n1085 = Or(x=w3367, y=w3366) -> (x .or. y?=w3365:bool)
                n1086 = Select(t=State_Type_Definitions,_for_0.26g_versions_and_later_3."True Stop" ("Enum"), s=w3366, f=State_Type_Definitions,_for_0.26g_versions_and_later_3."Task 9M: SCAN BOX 3" ("Enum")) -> (s? t:f=w3368:T18)
                n1087 = Select(t=w3368, s=w3365, f=State_Type_Definitions,_for_0.26g_versions_and_later_3."Task 9L: MOVE RIGHT" ("Enum")) -> (s? t:f=w3374:T18)
              }
              frame "Exit" {
                n1088 = for {
                  shift-right: [w3394] -> w3391
                  shift-left: w3390 -> [w3395]
                  tunnel: string[] ["STOP", "RESET ENCODERS", "RESET YAW", "ARDUINO MODE 0"] -> [w3393] mode=indexing
                  n1089 = Enqueue Element(queue=w3395, element=w3393) -> (queue out=w3394:refnum<queue>)  [unwired: 2 in, 2 out]
                }
              }
            }
          }
          frame "Task 9M: SCAN BOX 3" {
            # ">>> Motor control cluster >>>"
            # ">>> yStepper command>>>"
            # ">> Item Selection Bias >>"
            n1090 = Dequeue Element(queue=w3405, timeout in ms (-1)=w3404, error in (no error)=w3403) -> (element=w3409:T10)  [unwired: 3 out]
            n1091 = call "Box Colour FGV.vi"("Init/R/W State"=Box_Colour_FGV_States."Read") -> ("Colour to detect (output)"=w3399:T2)  [unwired: 9 in, 1 out]
            n1092 = Equal?(x=w3398, y=w3399) -> (x = y?=w3397:bool)
            n1093 = case shown="\"Start Task 1\", Default" w3409 {
              tunnel: w3396 -> [w3417 _]
              tunnel: [w3424 State_Type_Definitions,_for_0.26g_versions_and_later_3."True Stop" ("Enum")] -> w3407
              tunnel: w3402 -> [w3413 _]
              tunnel: w3406 -> [w3423 w3440]
              tunnel: [w3422 w3441] -> w3401
              tunnel: [State_Type_Definitions,_for_0.26g_versions_and_later_3."Idle" ("Enum") State_Type_Definitions,_for_0.26g_versions_and_later_3."Shutdown" ("Enum")] -> w3408
              tunnel: w3397 -> [w3415 _]
              frame "Start Task 1", Default {
                n1094 = case shown="True" w3417 {
                  tunnel: w3423 -> [w3427 w3434]
                  tunnel: [w3428 w3433] -> w3422
                  frame False {
                    n1095 = for {
                      tunnel: string[] ["", "", "", ""] ("element") -> [w3429] mode=indexing
                      shift-right: [w3431] -> w3428
                      shift-left: w3427 -> [w3430]
                      n1096 = Enqueue Element(queue=w3430, element=w3429) -> (queue out=w3431:refnum<queue>)  [unwired: 2 in, 2 out]
                    }
                  }
                  frame True {
                    n1097 = for {
                      shift-right: [w3436] -> w3433
                      shift-left: w3434 -> [w3437]
                      tunnel: string[] ["STOP", "RESET ENCODERS", "RESET FLAGS", "RESET YAW", "", ""] -> [w3435] mode=indexing
                      n1098 = Enqueue Element(queue=w3437, element=w3435) -> (queue out=w3436:refnum<queue>)  [unwired: 2 in, 2 out]
                    }
                  }
                }
                n1099 = Or(x=w3417, y=w3413) -> (x .or. y?=w3416:bool)
                n1100 = Or(x=w3415, y=w3413) -> (x .or. y?=w3414:bool)
                n1101 = Select(t=State_Type_Definitions,_for_0.26g_versions_and_later_3."True Stop" ("Enum"), s=w3414, f=State_Type_Definitions,_for_0.26g_versions_and_later_3."Task 9N: MOVE RIGHT" ("Enum")) -> (s? t:f=w3418:T18)
                n1102 = Select(t=w3418, s=w3416, f=State_Type_Definitions,_for_0.26g_versions_and_later_3."Task 9M: SCAN BOX 3" ("Enum")) -> (s? t:f=w3424:T18)
              }
              frame "Exit" {
                n1103 = for {
                  shift-right: [w3444] -> w3441
                  shift-left: w3440 -> [w3445]
                  tunnel: string[] ["STOP", "RESET ENCODERS", "RESET YAW", "ARDUINO MODE 0"] -> [w3443] mode=indexing
                  n1104 = Enqueue Element(queue=w3445, element=w3443) -> (queue out=w3444:refnum<queue>)  [unwired: 2 in, 2 out]
                }
              }
            }
          }
          frame "Task 9N: MOVE RIGHT" {
            # ">> Item Selection Bias >>"
            n1105 = Dequeue Element(queue=w3450, timeout in ms (-1)=w3449, error in (no error)=w3448) -> (element=w3455:T10)  [unwired: 3 out]
            n1106 = case shown="\"Start Task 1\", Default" w3455 {
              tunnel: w3446 -> [w3461 _]
              tunnel: [w3468 State_Type_Definitions,_for_0.26g_versions_and_later_3."True Stop" ("Enum")] -> w3453
              tunnel: w3447 -> [w3460 _]
              tunnel: w3451 -> [w3467 w3484]
              tunnel: [w3466 w3485] -> w3452
              tunnel: [State_Type_Definitions,_for_0.26g_versions_and_later_3."Idle" ("Enum") State_Type_Definitions,_for_0.26g_versions_and_later_3."Shutdown" ("Enum")] -> w3454
              frame "Start Task 1", Default {
                n1107 = case shown="True" w3461 {
                  tunnel: w3467 -> [w3471 w3478]
                  tunnel: [w3472 w3477] -> w3466
                  frame False {
                    n1108 = for {
                      tunnel: string[] ["READ LINE SENSOR", "READ NAVX", "RIGHT", "READ ENCODERS"] ("element") -> [w3473] mode=indexing
                      shift-right: [w3475] -> w3472
                      shift-left: w3471 -> [w3474]
                      n1109 = Enqueue Element(queue=w3474, element=w3473) -> (queue out=w3475:refnum<queue>)  [unwired: 2 in, 2 out]
                    }
                  }
                  frame True {
                    n1110 = for {
                      shift-right: [w3480] -> w3477
                      shift-left: w3478 -> [w3481]
                      tunnel: string[] ["STOP", "RESET ENCODERS", "RESET YAW", "RESET FLAGS", "BOX COLOUR", ""] -> [w3479] mode=indexing
                      n1111 = Enqueue Element(queue=w3481, element=w3479) -> (queue out=w3480:refnum<queue>)  [unwired: 2 in, 2 out]
                    }
                  }
                }
                n1112 = Or(x=w3461, y=w3460) -> (x .or. y?=w3459:bool)
                n1113 = Select(t=State_Type_Definitions,_for_0.26g_versions_and_later_3."True Stop" ("Enum"), s=w3460, f=State_Type_Definitions,_for_0.26g_versions_and_later_3."Task 9O: SCAN BOX 4" ("Enum")) -> (s? t:f=w3462:T18)
                n1114 = Select(t=w3462, s=w3459, f=State_Type_Definitions,_for_0.26g_versions_and_later_3."Task 9N: MOVE RIGHT" ("Enum")) -> (s? t:f=w3468:T18)
              }
              frame "Exit" {
                n1115 = for {
                  shift-right: [w3488] -> w3485
                  shift-left: w3484 -> [w3489]
                  tunnel: string[] ["STOP", "RESET ENCODERS", "RESET YAW", "ARDUINO MODE 0"] -> [w3487] mode=indexing
                  n1116 = Enqueue Element(queue=w3489, element=w3487) -> (queue out=w3488:refnum<queue>)  [unwired: 2 in, 2 out]
                }
              }
            }
          }
          frame "Task 9O: SCAN BOX 4" {
            # ">>> Motor control cluster >>>"
            # ">>> yStepper command>>>"
            # ">> Item Selection Bias >>"
            n1117 = Dequeue Element(queue=w3500, timeout in ms (-1)=w3499, error in (no error)=w3498) -> (element=w3504:T10)  [unwired: 3 out]
            n1118 = call "Box Colour FGV.vi"("Init/R/W State"=Box_Colour_FGV_States."Read") -> ("Colour to detect (output)"=w3502:T2)  [unwired: 9 in, 1 out]
            n1119 = Equal?(x=w3492, y=w3502) -> (x = y?=w3501:bool)
            n1120 = case shown="\"Start Task 1\", Default" w3504 {
              tunnel: w3490 -> [w3511 _]
              tunnel: [w3518 State_Type_Definitions,_for_0.26g_versions_and_later_3."True Stop" ("Enum")] -> w3494
              tunnel: w3497 -> [w3507 _]
              tunnel: w3491 -> [w3517 w3534]
              tunnel: [w3516 w3535] -> w3495
              tunnel: [State_Type_Definitions,_for_0.26g_versions_and_later_3."Idle" ("Enum") State_Type_Definitions,_for_0.26g_versions_and_later_3."Shutdown" ("Enum")] -> w3493
              tunnel: w3501 -> [w3509 _]
              frame "Start Task 1", Default {
                n1121 = case shown="True" w3511 {
                  tunnel: w3517 -> [w3521 w3528]
                  tunnel: [w3522 w3527] -> w3516
                  frame False {
                    n1122 = for {
                      tunnel: string[] ["", "", "", ""] ("element") -> [w3523] mode=indexing
                      shift-right: [w3525] -> w3522
                      shift-left: w3521 -> [w3524]
                      n1123 = Enqueue Element(queue=w3524, element=w3523) -> (queue out=w3525:refnum<queue>)  [unwired: 2 in, 2 out]
                    }
                  }
                  frame True {
                    n1124 = for {
                      shift-right: [w3530] -> w3527
                      shift-left: w3528 -> [w3531]
                      tunnel: string[] ["STOP", "RESET ENCODERS", "RESET FLAGS", "RESET YAW", "", ""] -> [w3529] mode=indexing
                      n1125 = Enqueue Element(queue=w3531, element=w3529) -> (queue out=w3530:refnum<queue>)  [unwired: 2 in, 2 out]
                    }
                  }
                }
                n1126 = Or(x=w3511, y=w3507) -> (x .or. y?=w3510:bool)
                n1127 = Or(x=w3509, y=w3507) -> (x .or. y?=w3508:bool)
                n1128 = Select(t=State_Type_Definitions,_for_0.26g_versions_and_later_3."True Stop" ("Enum"), s=w3508, f=State_Type_Definitions,_for_0.26g_versions_and_later_3."True Stop" ("Enum")) -> (s? t:f=w3512:T18)
                n1129 = Select(t=w3512, s=w3510, f=State_Type_Definitions,_for_0.26g_versions_and_later_3."Task 9O: SCAN BOX 4" ("Enum")) -> (s? t:f=w3518:T18)
              }
              frame "Exit" {
                n1130 = for {
                  shift-right: [w3538] -> w3535
                  shift-left: w3534 -> [w3539]
                  tunnel: string[] ["STOP", "RESET ENCODERS", "RESET YAW", "ARDUINO MODE 0"] -> [w3537] mode=indexing
                  n1131 = Enqueue Element(queue=w3539, element=w3537) -> (queue out=w3538:refnum<queue>)  [unwired: 2 in, 2 out]
                }
              }
            }
          }
          frame "Task A1: RAISE ARM" {
            # ">>> Motor control cluster >>>"
            # ">>> yStepper command>>>"
            n1132 = Dequeue Element(queue=w3551, timeout in ms (-1)=w3550, error in (no error)=w3549) -> (element=w3556:T10)  [unwired: 3 out]
            n1133 = Greater?(x=w3541, y=50.0) -> (0:w3544:bool)
            n1134 = And(x=w3542, y=w3544) -> (x .and. y?=w3540:bool)
            n1135 = case shown="\"Start Task 1\", Default" w3556 {
              tunnel: w3540 -> [w3559 _]
              tunnel: [w3566 State_Type_Definitions,_for_0.26g_versions_and_later_3."True Stop" ("Enum")] -> w3555
              tunnel: w3548 -> [w3558 _]
              tunnel: w3552 -> [w3565 w3582]
              tunnel: [w3564 w3583] -> w3554
              tunnel: [State_Type_Definitions,_for_0.26g_versions_and_later_3."Idle" ("Enum") State_Type_Definitions,_for_0.26g_versions_and_later_3."Shutdown" ("Enum")] -> w3553
              frame "Start Task 1", Default {
                n1136 = case shown="True" w3559 {
                  tunnel: w3565 -> [w3569 w3576]
                  tunnel: [w3570 w3575] -> w3564
                  frame False {
                    n1137 = for {
                      tunnel: string[] ["READ LINE SENSOR", "READ NAVX", "RIGHT", "READ ENCODERS"] ("element") -> [w3571] mode=indexing
                      shift-right: [w3573] -> w3570
                      shift-left: w3569 -> [w3572]
                      n1138 = Enqueue Element(queue=w3572, element=w3571) -> (queue out=w3573:refnum<queue>)  [unwired: 2 in, 2 out]
                    }
                  }
                  frame True {
                    n1139 = for {
                      shift-right: [w3578] -> w3575
                      shift-left: w3576 -> [w3579]
                      tunnel: string[] ["RESET ENCODERS", "RESET YAW", "RESET FLAGS", "STOP", "BOX COLOUR"] -> [w3577] mode=indexing
                      n1140 = Enqueue Element(queue=w3579, element=w3577) -> (queue out=w3578:refnum<queue>)  [unwired: 2 in, 2 out]
                    }
                  }
                }
                n1141 = Or(x=w3559, y=w3558) -> (x .or. y?=w3557:bool)
                n1142 = Select(t=State_Type_Definitions,_for_0.26g_versions_and_later_3."True Stop" ("Enum"), s=w3558, f=State_Type_Definitions,_for_0.26g_versions_and_later_3."Task 9H: SCAN BOX 2" ("Enum")) -> (s? t:f=w3560:T18)
                n1143 = Select(t=w3560, s=w3557, f=State_Type_Definitions,_for_0.26g_versions_and_later_3."Task 9G: MOVE RIGHT" ("Enum")) -> (s? t:f=w3566:T18)
              }
              frame "Exit" {
                n1144 = for {
                  shift-right: [w3586] -> w3583
                  shift-left: w3582 -> [w3587]
                  tunnel: string[] ["STOP", "RESET ENCODERS", "RESET YAW", "ARDUINO MODE 0"] -> [w3585] mode=indexing
                  n1145 = Enqueue Element(queue=w3587, element=w3585) -> (queue out=w3586:refnum<queue>)  [unwired: 2 in, 2 out]
                }
              }
            }
          }
          frame "Task A2: ROTATE TO ANGLE" {
          }
          frame "Task A3: MOVE TO BL BOX" {
          }
          frame "Task A4: MOVE FORWARD" {
          }
          frame "Task A5: Stop" {
          }
        }
        "Object Detection" <- w331
        "Ultrasonic sensors" <- w354
        "Encoder values" <- w343
        "Stepper position values" <- w327
        "NAVX Values" <- w325
        "IR Sensors" <- w317
        "Line sensors" <- w312
        "Time cluster" <- w323
        "Box Colour Detection" <- w305
      }
    }
    "Object recognition mode" <- w230
    "Front Ultrasonic obstruct" <- w227
    "Front IR obstruct" <- w226
    "Table IR obstruct" <- w225
    "Same colour?" <- w218
    n1146 = local write "Green LED"(w240) -> ()
  }
  n1147 = while {
    tunnel: w49 -> [w4555]
    tunnel: w48 -> [w4552]
    stop <- w4549 stop-if-true
    # "Status Loop for Action Queues"
    n1148 = Get Queue Status(queue=w4555, return elements? (F)=TRUE) -> (error out=w4551:errorcluster, # elements in queue=→"Action Queue Items":i32, elements=→"Action Queues items":string[])  [unwired: 1 in, 5 out]
    n1149 = Get Queue Status(queue=w4552, return elements? (F)=TRUE) -> (# pending remove=→"State Logic Queue Items":i32, error out=w4550:errorcluster, elements=→"elements":T10[])  [unwired: 1 in, 5 out]
    n1150 = Merge Errors(w4551, w4550) -> (w4549:errorcluster)
    n1151 = Wait (ms)(milliseconds to wait=u32 500) -> ()  [unwired: 1 out]
  }
  n1152 = call <vilib>:"DIO Close.vi"("error in (no error)"=w25, "DIO Info In"=w28) -> ()  [unwired: 9 in, 1 out]
  n1153 = call <vilib>:"DIO Close.vi"("error in (no error)"=w35, "DIO Info In"=w37) -> ()  [unwired: 9 in, 1 out]
  n1154 = call <vilib>:"NavX Close.vi"("error in (no error)"=w12, "NavX Info In"=w11) -> ()  [unwired: 9 in, 1 out]
  n1155 = call <vilib>:"DIO Close.vi"("error in (no error)"=w30, "DIO Info In"=w32) -> ()  [unwired: 9 in, 1 out]
  n1156 = call <vilib>:"DIO Close.vi"("error in (no error)"=w19, "DIO Info In"=w20) -> ()  [unwired: 9 in, 1 out]
  n1157 = call <vilib>:"DIO Close.vi"("error in (no error)"=w14, "DIO Info In"=w15) -> ()  [unwired: 9 in, 1 out]
  n1158 = Merge Errors "Merge Errors"(w65, w64) -> (w47:errorcluster)
  n1159 = Merge Errors(w51, w47) -> (w46:errorcluster)
  n1160 = Destroy User Event(user event=w69, error in=w46) -> ()  [unwired: 1 out]
  n1161 = Release Queue(queue=w42, error in (no error)=w46) -> (error out=→"Queue Errors":errorcluster)  [unwired: 1 in, 2 out]
  n1162 = Release Queue(queue=w59, error in (no error)=w46) -> ()  [unwired: 1 in, 3 out]
  n1163 = Destroy User Event(user event=w68, error in=w46) -> ()  [unwired: 1 out]
  n1164 = Unregister For Events(event registration refnum=w60, error in=w46) -> ()  [unwired: 1 out]
